vi "dotNET Compress String.vi"(8 "error in (no error)":errorcluster, 11 "String":string="<Cluster>\r\n<Name>TDC Data Cluster (XML)</Name>\r\n<NumElts>4</NumElts>\r\n<Array>\r\n<Name>Adapter Data</Name>\r\n<Dimsize>10</Dimsize>\r\n<String>\r\n<Name> </Name>\r\n<Val>SigmaQuest</Val>\r\n</String>\r\n<String>\r\n<Name> </Name>\r\n<Val>C:\\Program Files\\TMS\\TDC</Val>\r\n</String>\r\n<String>\r\n<Name> </Name>\r\n<Val>TDC Adapter XML Archive.vi</Val>\r\n</String>\r\n<String>\r\n<Name> </Name>\r\n<Val>C:\\Test Reports\\TDC XML</Val>\r\n</String>\r\n<String>\r\n<Name> </Name>\r\n<Val>ET</Val>\r\n</String>\r\n<String>\r\n<Name> </Name>\r\n<Val>OTDA</Val>\r\n</String>\r\n<String>\r\n<Name> </Name>\r\n<Val>TRUE</Val>\r\n</String>\r\n<String>\r\n<Name> </Name>\r\n<Val>D98FE819-833D-54CF-2F12-8500A4D4E1C3</Val>\r\n</String>\r\n<String>\r\n<Name> </Name>\r\n<Val></Val>\r\n</String>\r\n<String>\r\n<Name> </Name>\r\n<Val></Val>\r\n</String>\r\n</Array>\r\n<Cluster>\r\n<Name>Station Common Data</Name>\r\n<NumElts>10</NumElts>\r\n<String>\r\n<Name>Customer</Name>\r\n<Val></Val>\r\n</String>\r\n<String>\r\n<Name>Manufacturer</Name>\r\n<Val></Val>\r\n</String>\r\n<String>\r\n<Name>Process</Name>\r\n<Val></Val>\r\n</String>\r\n<String>\r\n<Name>Line</Name>\r\n<Val></Val>\r\n</String>\r\n<String>\r\n<Name>Site</Name>\r\n<Val>Sycamore-Chelmsford</Val>\r\n</String>\r\n<String>\r\n<Name>Station</Name>\r\n<Val>ATE0000003</Val>\r\n</String>\r\n<String>\r\n<Name>Operator</Name>\r\n<Val>jdaoust</Val>\r\n</String>\r\n<String>\r\n<Name>Privilege</Name>\r\n<Val>technician</Val>\r\n</String>\r\n<String>\r\n<Name>Exp1</Name>\r\n<Val></Val>\r\n</String>\r\n<String>\r\n<Name>Exp2</Name>\r\n<Val></Val>\r\n</String>\r\n</Cluster>\r\n<Cluster>\r\n<Name>Header Data</Name>\r\n<NumElts>19</NumElts>\r\n<String>\r\n<Name>SerialNumber</Name>\r\n<Val>N635017050</Val>\r\n</String>\r\n<String>\r\n<Name>ProductName</Name>\r\n<Val></Val>\r\n</String>\r\n<String>\r\n<Name>ProductNumber</Name>\r\n<Val>910244</Val>\r\n</String>\r\n<String>\r\n<Name>ProductRev</Name>\r\n<Val>AB</Val>\r\n</String>\r\n<String>\r\n<Name>FirmwareRev</Name>\r\n<Val></Val>\r\n</String>\r\n<String>\r\n<Name>CMProductName</Name>\r\n<Val></Val>\r\n</String>\r\n<String>\r\n<Name>CMProductNumber</Name>\r\n<Val>8500052410E</Val>\r\n</String>\r\n<String>\r\n<Name>CMProductRev</Name>\r\n<Val>0L1</Val>\r\n</String>\r\n<String>\r\n<Name>EventType</Name>\r\n<Val></Val>\r\n</String>\r\n<String>\r\n<Name>TPSName</Name>\r\n<Val>SN16K GSC-MC Full (Fixed Pad)</Val>\r\n</String>\r\n<String>\r\n<Name>TPSRev</Name>\r\n<Val>D</Val>\r\n</String>\r\n<String>\r\n<Name>TestStatus</Name>\r\n<Val>PASSED</Val>\r\n</String>\r\n<String>\r\n<Name>StartTime</Name>\r\n<Val>07/07/09 12:07:49</Val>\r\n</String>\r\n<String>\r\n<Name>StopTime</Name>\r\n<Val>07/07/09 12:53:15</Val>\r\n</String>\r\n<String>\r\n<Name>Duration</Name>\r\n<Val>2727</Val>\r\n</String>\r\n<String>\r\n<Name>FixtureID</Name>\r\n<Val></Val>\r\n</String>\r\n<String>\r\n<Name>LotCode</Name>\r\n<Val>HIPDB1</Val>\r\n</String>\r\n<String>\r\n<Name>Expansion1</Name>\r\n<Val></Val>\r\n</String>\r\n<String>\r\n<Name>Expansion2</Name>\r\n<Val></Val>\r\n</String>\r\n</Cluster>\r\n<Array>\r\n<Name>Data</Name>\r\n<Dimsize>11</Dimsize>\r\n<Dimsize>493</Dimsize>\r\n<String>\r\n<Name> </Name>\r\n<Val>UUT &amp; TPS Verify</Val>\r\n</String>\r\n<String>\r\n<Name> </Name>\r\n<Val>Fetch Matrix Details</Val>\r\n</String>\r\n<String>\r\n<Name> </Name>\r\n<Val>Get UUT Information</Val>\r\n</String>\r\n<String>\r\n<Name> </Name>\r\n<Val>Get UUT Information</Val>\r\n</String>\r\n<String>\r\n<Name> </Name>\r\n<Val>Log TPS P/N and Rev</Val>\r\n</String>\r\n<String>\r\n<Name> </Name>\r\n<Val>Check for Genealogy</Val>\r\n</String>\r\n<String>\r\n<Name> </Name>\r\n<Val>Skip if UUTInfoSubSequenceFile = \"Null\"</Val>\r\n</String>\r\n<String>\r\n<Name> </Name>\r\n<Val>Get UUT Genealogy Information</Val>\r\n</String>\r\n<String>\r\n<Name> </Name>\r\n<Val>TMS Common Genealogy Dialog</Val>\r\n</String>\r\n<String>\r\n<Name> </Name>\r\n<Val>Get Genealogy Information</Val>\r\n</String>\r\n<String>\r\n<Name> </Name>\r\n<Val>Power Supplies OFF</Val>\r\n</String>\r\n<String>\r\n<Name> </Name>\r\n<Val>Open VISA Sessions</Val>\r\n</String>\r\n<String>\r\n<Name> </Name>\r\n<Val>Save VXI CFG Path</Val>\r\n</String>\r\n<String>\r\n<Name> </Name>\r\n<Val>Store Paths to Directories</Val>\r\n</String>\r\n<String>\r\n<Name> </Name>\r\n<Val>Reset Arb</Val>\r\n</String>\r\n<String>\r\n<Name> </Name>\r\n<Val>Reset Mux Switching</Val>\r\n</String>\r\n<String>\r\n<Name> </Name>\r\n<Val>Store ITA Slot ID mask</Val>\r\n</String>\r\n<String>\r\n<Name> </Name>\r\n<Val>Store ITA Chassis ID mask</Val>\r\n</String>\r\n<String>\r\n<Name> </Name>\r\n<Val>Install and Connect UUT</Val>\r\n</String>\r\n<String>\r\n<Name> </Name>\r\n<Val>Insert UUT (PC Com)</Val>\r\n</String>\r\n<String>\r\n<Name> </Name>\r\n<Val>Verify Card Present</Val>\r\n</String>\r\n<String>\r\n<Name> </Name>\r\n<Val>Power UP</Val>\r\n</String>\r\n<String>\r\n<Name> </Name>\r\n<Val>Turn on 48VDC</Val>\r\n</String>\r\n<String>\r\n<Name> </Name>\r\n<Val>Turn on 3VDC</Val>\r\n</String>\r\n<String>\r\n<Name> </Name>\r\n<Val>Select 48VDC VXI Switches</Val>\r\n</String>\r\n<String>\r\n<Name> </Name>\r\n<Val>Check 48VDC Voltage</Val>\r\n</String>\r\n<String>\r\n<Name> </Name>\r\n<Val>Check 48VDC Current</Val>\r\n</String>\r\n<String>\r\n<Name> </Name>\r\n<Val>Select 3VDC VXI Switches</Val>\r\n</String>\r\n<String>\r\n<Name> </Name>\r\n<Val>Check 3VDC Voltage</Val>\r\n</String>\r\n<String>\r\n<Name> </Name>\r\n<Val>Verify UUT Bootup and Firmware</Val>\r\n</String>\r\n<String>\r\n<Name> </Name>\r\n<Val>Fetch Matrix Information if required</Val>\r\n</String>\r\n<String>\r\n<Name> </Name>\r\n<Val>Establish Communication</Val>\r\n</String>\r\n<String>\r\n<Name> </Name>\r\n<Val>Check Cable and DIP Switches</Val>\r\n</String>\r\n<String>\r\n<Name> </Name>\r\n<Val>Cycle Power if unable to Establish Communication</Val>\r\n</String>\r\n<String>\r\n<Name> </Name>\r\n<Val>Re-Establish Communication</Val>\r\n</String>\r\n<String>\r\n<Name> </Name>\r\n<Val>Fetch Versions - Flash Files</Val>\r\n</String>\r\n<String>\r\n<Name> </Name>\r\n<Val>Verify Flash Files = Required</Val>\r\n</String>\r\n<String>\r\n<Name> </Name>\r\n<Val>Get Loaded Versions using Command</Val>\r\n</String>\r\n<String>\r\n<Name> </Name>\r\n<Val>Verify Loaded = Required</Val>\r\n</String>\r\n<String>\r\n<Name> </Name>\r\n<Val>Change DIP Switches to RMM Mode</Val>\r\n</String>\r\n<String>\r\n<Name> </Name>\r\n<Val>Cycle Power 1</Val>\r\n</String>\r\n<String>\r\n<Name> </Name>\r\n<Val>Establish Communication 1</Val>\r\n</String>\r\n<String>\r\n<Name> </Name>\r\n<Val>Program BaseROM</Val>\r\n</String>\r\n<String>\r\n<Name> </Name>\r\n<Val>Cycle Power 2</Val>\r\n</String>\r\n<String>\r\n<Name> </Name>\r\n<Val>Establish Communication 2</Val>\r\n</String>\r\n<String>\r\n<Name> </Name>\r\n<Val>Program BootROM</Val>\r\n</String>\r\n<String>\r\n<Name> </Name>\r\n<Val>Program DiagROM</Val>\r\n</String>\r\n<String>\r\n<Name> </Name>\r\n<Val>Program FpgaROM</Val>\r\n</String>\r\n<String>\r\n<Name> </Name>\r\n<Val>Change DIP Switches to Diag Mode</Val>\r\n</String>\r\n<String>\r\n<Name> </Name>\r\n<Val>Cycle Power 3</Val>\r\n</String>\r\n<String>\r\n<Name> </Name>\r\n<Val>Establish Communication 3</Val>\r\n</String>\r\n<String>\r\n<Name> </Name>\r\n<Val>Verify UUT in Diag Mode</Val>\r\n</String>\r\n<String>\r\n<Name> </Name>\r\n<Val>Get Loaded Versions using Command 2</Val>\r\n</String>\r\n<String>\r\n<Name> </Name>\r\n<Val>Verify Loaded = Required 2</Val>\r\n</String>\r\n<String>\r\n<Name> </Name>\r\n<Val>Program IDPROM</Val>\r\n</String>\r\n<String>\r\n<Name> </Name>\r\n<Val>Electrical Diags</Val>\r\n</String>\r\n<String>\r\n<Name> </Name>\r\n<Val>MII Tests</Val>\r\n</String>\r\n<String>\r\n<Name> </Name>\r\n<Val>LED Test</Val>\r\n</String>\r\n<String>\r\n<Name> </Name>\r\n<Val>LED Test Retry Message</Val>\r\n</String>\r\n<String>\r\n<Name> </Name>\r\n<Val>MII0 Access Test</Val>\r\n</String>\r\n<String>\r\n<Name> </Name>\r\n<Val>MII1 Access Test</Val>\r\n</String>\r\n<String>\r\n<Name> </Name>\r\n<Val>SDRAM Tests</Val>\r\n</String>\r\n<String>\r\n<Name> </Name>\r\n<Val>FCC1 Setup for PHY Loopback</Val>\r\n</String>\r\n<String>\r\n<Name> </Name>\r\n<Val>FCC1 PHY Loopback Test</Val>\r\n</String>\r\n<String>\r\n<Name> </Name>\r\n<Val>FCC2 Setup for PHY Loopback</Val>\r\n</String>\r\n<String>\r\n<Name> </Name>\r\n<Val>FCC2 PHY Loopback Test</Val>\r\n</String>\r\n<String>\r\n<Name> </Name>\r\n<Val>Reinitialize card</Val>\r\n</String>\r\n<String>\r\n<Name> </Name>\r\n<Val>FCC1 Setup for no Loopback</Val>\r\n</String>\r\n<String>\r\n<Name> </Name>\r\n<Val>FCC2 Setup for no Loopback</Val>\r\n</String>\r\n<String>\r\n<Name> </Name>\r\n<Val>FCC1 to FCC2 Test</Val>\r\n</String>\r\n<String>\r\n<Name> </Name>\r\n<Val>FCC2 to FCC1 Test</Val>\r\n</String>\r\n<String>\r\n<Name> </Name>\r\n<Val>Cycle Reset Latch , FCC retest</Val>\r\n</String>\r\n<String>\r\n<Name> </Name>\r\n<Val>Establish Diagnostics Communication, FCC retest</Val>\r\n</String>\r\n<String>\r\n<Name> </Name>\r\n<Val>Get Temperature</Val>\r\n</String>\r\n<String>\r\n<Name> </Name>\r\n<Val>Temp Test Retry Message</Val>\r\n</String>\r\n<String>\r\n<Name> </Name>\r\n<Val>SDRAM Data Bus Test</Val>\r\n</String>\r\n<String>\r\n<Name> </Name>\r\n<Val>SDRAM Address Bus Test</Val>\r\n</String>\r\n<String>\r\n<Name> </Name>\r\n<Val>SDRAM Size Test</Val>\r\n</String>\r\n<String>\r\n<Name> </Name>\r\n<Val>FPGA Tests</Val>\r\n</String>\r\n<String>\r\n<Name> </Name>\r\n<Val>PRBS FPGA Access Test</Val>\r\n</String>\r\n<String>\r\n<Name> </Name>\r\n<Val>PRBS FPGA Interrupt Test</Val>\r\n</String>\r\n<String>\r\n<Name> </Name>\r\n<Val>EEPROM Tests</Val>\r\n</String>\r\n<String>\r\n<Name> </Name>\r\n<Val>EEPROM Single Byte Test</Val>\r\n</String>\r\n<String>\r\n<Name> </Name>\r\n<Val>GXC B EEPROM Access Test</Val>\r\n</String>\r\n<String>\r\n<Name> </Name>\r\n<Val>GXC A EEPROM Access Test</Val>\r\n</String>\r\n<String>\r\n<Name> </Name>\r\n<Val>Verify GXC B Status at Addr f303800c</Val>\r\n</String>\r\n<String>\r\n<Name> </Name>\r\n<Val>Verify GXC A Status at Addr f301800c</Val>\r\n</String>\r\n<String>\r\n<Name> </Name>\r\n<Val>CPLD Tests</Val>\r\n</String>\r\n<String>\r\n<Name> </Name>\r\n<Val>Control CPLD Version</Val>\r\n</String>\r\n<String>\r\n<Name> </Name>\r\n<Val>Control CPLD Access Test</Val>\r\n</String>\r\n<String>\r\n<Name> </Name>\r\n<Val>Timing CPLD Access Test</Val>\r\n</String>\r\n<String>\r\n<Name> </Name>\r\n<Val>Timing CPLD Interrupt Test</Val>\r\n</String>\r\n<String>\r\n<Name> </Name>\r\n<Val>GXC Tests</Val>\r\n</String>\r\n<String>\r\n<Name> </Name>\r\n<Val>GXC B Access Test</Val>\r\n</String>\r\n<String>\r\n<Name> </Name>\r\n<Val>GXC B Interrupt Test</Val>\r\n</String>\r\n<String>\r\n<Name> </Name>\r\n<Val>GXC A Access Test</Val>\r\n</String>\r\n<String>\r\n<Name> </Name>\r\n<Val>GXC A Interrupt Test</Val>\r\n</String>\r\n<String>\r\n<Name> </Name>\r\n<Val>Local Timing Tests</Val>\r\n</String>\r\n<String>\r\n<Name> </Name>\r\n<Val>Set Timing Select to Local</Val>\r\n</String>\r\n<String>\r\n<Name> </Name>\r\n<Val>Test VCXO Status</Val>\r\n</String>\r\n<String>\r\n<Name> </Name>\r\n<Val>Test SYSCLK Status</Val>\r\n</String>\r\n<String>\r\n<Name> </Name>\r\n<Val>Test PLL Status</Val>\r\n</String>\r\n<String>\r\n<Name> </Name>\r\n<Val>PLL Re-Lock Test</Val>\r\n</String>\r\n<String>\r\n<Name> </Name>\r\n<Val>PRBS Path Thru Switch</Val>\r\n</String>\r\n<String>\r\n<Name> </Name>\r\n<Val>PRBS Path Thru Switch B</Val>\r\n</String>\r\n<String>\r\n<Name> </Name>\r\n<Val>Reset Switch B, PRBS Path Test</Val>\r\n</String>\r\n<String>\r\n<Name> </Name>\r\n<Val>Setup PRBS Test Thru Switch B</Val>\r\n</String>\r\n<String>\r\n<Name> </Name>\r\n<Val>Verify PRBS Status, in Sync, SW B</Val>\r\n</String>\r\n<String>\r\n<Name> </Name>\r\n<Val>Verify PRBS Status, Zero B1 Errors, SW B</Val>\r\n</String>\r\n<String>\r\n<Name> </Name>\r\n<Val>Turn Off PRBS Generator</Val>\r\n</String>\r\n<String>\r\n<Name> </Name>\r\n<Val>Verify PRBS Status, Lost Sync, SW B</Val>\r\n</String>\r\n<String>\r\n<Name> </Name>\r\n<Val>Verify PRBS Status, Max B1 Errors, SW B</Val>\r\n</String>\r\n<String>\r\n<Name> </Name>\r\n<Val>PRBS Path Thru Switch A</Val>\r\n</String>\r\n<String>\r\n<Name> </Name>\r\n<Val>Reset Switch A, PRBS Path Test</Val>\r\n</String>\r\n<String>\r\n<Name> </Name>\r\n<Val>Setup PRBS Test Thru Switch A</Val>\r\n</String>\r\n<String>\r\n<Name> </Name>\r\n<Val>Verify PRBS Status, in Sync, SW A</Val>\r\n</String>\r\n<String>\r\n<Name> </Name>\r\n<Val>Verify PRBS Status, Zero B1 Errors, SW A</Val>\r\n</String>\r\n<String>\r\n<Name> </Name>\r\n<Val>Turn Off PRBS Generator</Val>\r\n</String>\r\n<String>\r\n<Name> </Name>\r\n<Val>Verify PRBS Status, Lost Sync, SW A</Val>\r\n</String>\r\n<String>\r\n<Name> </Name>\r\n<Val>Verify PRBS Status, Max B1 Errors, SW A</Val>\r\n</String>\r\n<String>\r\n<Name> </Name>\r\n<Val>Electrical Backplane Tests</Val>\r\n</String>\r\n<String>\r\n<Name> </Name>\r\n<Val>SMC Tests</Val>\r\n</String>\r\n<String>\r\n<Name> </Name>\r\n<Val>Enable SMC Digital IO</Val>\r\n</String>\r\n<String>\r\n<Name> </Name>\r\n<Val>Set SMC Act Inputs, 110</Val>\r\n</String>\r\n<String>\r\n<Name> </Name>\r\n<Val>Test Soft Reset A</Val>\r\n</String>\r\n<String>\r\n<Name> </Name>\r\n<Val>Test Hard Reset A</Val>\r\n</String>\r\n<String>\r\n<Name> </Name>\r\n<Val>SMC A Active Test 1</Val>\r\n</String>\r\n<String>\r\n<Name> </Name>\r\n<Val>Set SMC Act Inputs, 101</Val>\r\n</String>\r\n<String>\r\n<Name> </Name>\r\n<Val>SMC A Active Test 2</Val>\r\n</String>\r\n<String>\r\n<Name> </Name>\r\n<Val>Set SMC Act Inputs, 011</Val>\r\n</String>\r\n<String>\r\n<Name> </Name>\r\n<Val>SMC A Active Test 3</Val>\r\n</String>\r\n<String>\r\n<Name> </Name>\r\n<Val>Set SMC Act Inputs, 100</Val>\r\n</String>\r\n<String>\r\n<Name> </Name>\r\n<Val>Test Soft Reset B</Val>\r\n</String>\r\n<String>\r\n<Name> </Name>\r\n<Val>Test Hard Reset B</Val>\r\n</String>\r\n<String>\r\n<Name> </Name>\r\n<Val>SMC B Active Test 1</Val>\r\n</String>\r\n<String>\r\n<Name> </Name>\r\n<Val>Set SMC Act Inputs, 010</Val>\r\n</String>\r\n<String>\r\n<Name> </Name>\r\n<Val>SMC B Active Test 2</Val>\r\n</String>\r\n<String>\r\n<Name> </Name>\r\n<Val>Set SMC Act Inputs, 001</Val>\r\n</String>\r\n<String>\r\n<Name> </Name>\r\n<Val>SMC B Active Test 3</Val>\r\n</String>\r\n<String>\r\n<Name> </Name>\r\n<Val>Disable SMC Digital IO</Val>\r\n</String>\r\n<String>\r\n<Name> </Name>\r\n<Val>TRC Timing Tests</Val>\r\n</String>\r\n<String>\r\n<Name> </Name>\r\n<Val>Set Timing Select to Auto</Val>\r\n</String>\r\n<String>\r\n<Name> </Name>\r\n<Val>Enable TRC Digital IO</Val>\r\n</String>\r\n<String>\r\n<Name> </Name>\r\n<Val>TRC A Tests</Val>\r\n</String>\r\n<String>\r\n<Name> </Name>\r\n<Val>Set Arb to 19MHz Sys Clock A</Val>\r\n</String>\r\n<String>\r\n<Name> </Name>\r\n<Val>Test Prim Ref Clock Status Valid</Val>\r\n</String>\r\n<String>\r\n<Name> </Name>\r\n<Val>Test Sec Ref Clock Status Invalid</Val>\r\n</String>\r\n<String>\r\n<Name> </Name>\r\n<Val>Set TRC Act Inputs, 110</Val>\r\n</String>\r\n<String>\r\n<Name> </Name>\r\n<Val>TRC A Active Test 1</Val>\r\n</String>\r\n<String>\r\n<Name> </Name>\r\n<Val>Set TRC Act Inputs, 101</Val>\r\n</String>\r\n<String>\r\n<Name> </Name>\r\n<Val>TRC A Active Test 2</Val>\r\n</String>\r\n<String>\r\n<Name> </Name>\r\n<Val>Set TRC Act Inputs, 011</Val>\r\n</String>\r\n<String>\r\n<Name> </Name>\r\n<Val>TRC A Active Test 3</Val>\r\n</String>\r\n<String>\r\n<Name> </Name>\r\n<Val>TRC B Tests</Val>\r\n</String>\r\n<String>\r\n<Name> </Name>\r\n<Val>Set Arb to 19Mhz Sys Clock B</Val>\r\n</String>\r\n<String>\r\n<Name> </Name>\r\n<Val>Test Sec Ref Clock Status Valid</Val>\r\n</String>\r\n<String>\r\n<Name> </Name>\r\n<Val>Test Prim Ref Clock Status Invalid</Val>\r\n</String>\r\n<String>\r\n<Name> </Name>\r\n<Val>Set TRC Act Inputs, 100</Val>\r\n</String>\r\n<String>\r\n<Name> </Name>\r\n<Val>TRC B Active Test 1</Val>\r\n</String>\r\n<String>\r\n<Name> </Name>\r\n<Val>Set TRC Act Inputs, 010</Val>\r\n</String>\r\n<String>\r\n<Name> </Name>\r\n<Val>TRC B Active Test 2</Val>\r\n</String>\r\n<String>\r\n<Name> </Name>\r\n<Val>Set TRC Act Inputs, 001</Val>\r\n</String>\r\n<String>\r\n<Name> </Name>\r\n<Val>TRC B Active Test 3</Val>\r\n</String>\r\n<String>\r\n<Name> </Name>\r\n<Val>Fsync Tests</Val>\r\n</String>\r\n<String>\r\n<Name> </Name>\r\n<Val>Enable TRC Fsync Status Reporting</Val>\r\n</String>\r\n<String>\r\n<Name> </Name>\r\n<Val>Set TRC Act Inputs, 110</Val>\r\n</String>\r\n<String>\r\n<Name> </Name>\r\n<Val>Set Arb to 8KHz Fsync A</Val>\r\n</String>\r\n<String>\r\n<Name> </Name>\r\n<Val>Test Fsync A Status Valid</Val>\r\n</String>\r\n<String>\r\n<Name> </Name>\r\n<Val>Test Fsync B Status Invalid</Val>\r\n</String>\r\n<String>\r\n<Name> </Name>\r\n<Val>Set TRC Act Inputs, 100</Val>\r\n</String>\r\n<String>\r\n<Name> </Name>\r\n<Val>Set Arb to 8KHz Fsync B</Val>\r\n</String>\r\n<String>\r\n<Name> </Name>\r\n<Val>Test Fsync B Status Valid</Val>\r\n</String>\r\n<String>\r\n<Name> </Name>\r\n<Val>Test Fsync A Status Invalid</Val>\r\n</String>\r\n<String>\r\n<Name> </Name>\r\n<Val>Disable TRC Digital IO</Val>\r\n</String>\r\n<String>\r\n<Name> </Name>\r\n<Val>Reset Arb</Val>\r\n</String>\r\n<String>\r\n<Name> </Name>\r\n<Val>Verify TRC Active is Local</Val>\r\n</String>\r\n<String>\r\n<Name> </Name>\r\n<Val>Set Timing Select back to Local</Val>\r\n</String>\r\n<String>\r\n<Name> </Name>\r\n<Val>Chassis and Slot ID Tests</Val>\r\n</String>\r\n<String>\r\n<Name> </Name>\r\n<Val>Enable Chassis ID Digital IO</Val>\r\n</String>\r\n<String>\r\n<Name> </Name>\r\n<Val>Set Chassis ID to '55'</Val>\r\n</String>\r\n<String>\r\n<Name> </Name>\r\n<Val>Verify '55' at f100000c</Val>\r\n</String>\r\n<String>\r\n<Name> </Name>\r\n<Val>Set Chassis ID to 'AA'</Val>\r\n</String>\r\n<String>\r\n<Name> </Name>\r\n<Val>Verify 'AA' at f100000c</Val>\r\n</String>\r\n<String>\r\n<Name> </Name>\r\n<Val>Chassis ID Test from Diag Port</Val>\r\n</String>\r\n<String>\r\n<Name> </Name>\r\n<Val>Disable Chassis ID Digital IO</Val>\r\n</String>\r\n<String>\r\n<Name> </Name>\r\n<Val>Enable Slot ID Digital IO</Val>\r\n</String>\r\n<String>\r\n<Name> </Name>\r\n<Val>Slot ID Test</Val>\r\n</String>\r\n<String>\r\n<Name> </Name>\r\n<Val>Disable Slot ID Digital IO</Val>\r\n</String>\r\n<String>\r\n<Name> </Name>\r\n<Val>Card Pending Removal Test</Val>\r\n</String>\r\n<String>\r\n<Name> </Name>\r\n<Val>BP LED Test</Val>\r\n</String>\r\n<String>\r\n<Name> </Name>\r\n<Val>BP LED Test Retry Message</Val>\r\n</String>\r\n<String>\r\n<Name> </Name>\r\n<Val>Disable Digital IO</Val>\r\n</String>\r\n<String>\r\n<Name> </Name>\r\n<Val>Pull Reset Latch Down</Val>\r\n</String>\r\n<String>\r\n<Name> </Name>\r\n<Val>Verify Pending Removal BP Signal</Val>\r\n</String>\r\n<String>\r\n<Name> </Name>\r\n<Val>Return Reset Latch to Up Position</Val>\r\n</String>\r\n<String>\r\n<Name> </Name>\r\n<Val>Verify No Pending Removal BP Signal</Val>\r\n</String>\r\n<String>\r\n<Name> </Name>\r\n<Val>Disable Digital IO</Val>\r\n</String>\r\n<String>\r\n<Name> </Name>\r\n<Val>Verify Diagnostics Communication</Val>\r\n</String>\r\n<String>\r\n<Name> </Name>\r\n<Val>Optical Backplane Tests</Val>\r\n</String>\r\n<String>\r\n<Name> </Name>\r\n<Val>Install Empty Quad-pack Connector A</Val>\r\n</String>\r\n<String>\r\n<Name> </Name>\r\n<Val>Verify VCSEL Outputs, SW A Ports 0 - 31</Val>\r\n</String>\r\n<String>\r\n<Name> </Name>\r\n<Val>Install Pos 1 MT Connector</Val>\r\n</String>\r\n<String>\r\n<Name> </Name>\r\n<Val>Test Outputs from MT Postion 1</Val>\r\n</String>\r\n<String>\r\n<Name> </Name>\r\n<Val>Disable Lasers</Val>\r\n</String>\r\n<String>\r\n<Name> </Name>\r\n<Val>Delay for 1 Second Before Verifying Disable</Val>\r\n</String>\r\n<String>\r\n<Name> </Name>\r\n<Val>Verify Laser Disable</Val>\r\n</String>\r\n<String>\r\n<Name> </Name>\r\n<Val>Enable AIS-L Insertion</Val>\r\n</String>\r\n<String>\r\n<Name> </Name>\r\n<Val>Enable Lasers</Val>\r\n</String>\r\n<String>\r\n<Name> </Name>\r\n<Val>Delay for 1 Second Before Verifying Enable</Val>\r\n</String>\r\n<String>\r\n<Name> </Name>\r\n<Val>Reset Fifo</Val>\r\n</String>\r\n<String>\r\n<Name> </Name>\r\n<Val>Reset Frame</Val>\r\n</String>\r\n<String>\r\n<Name> </Name>\r\n<Val>Verify VCSEL Active</Val>\r\n</String>\r\n<String>\r\n<Name> </Name>\r\n<Val>Verify Laser Enable</Val>\r\n</String>\r\n<String>\r\n<Name> </Name>\r\n<Val>Install Pos 2 MT Connector</Val>\r\n</String>\r\n<String>\r\n<Name> </Name>\r\n<Val>Test Outputs from MT Postion 2</Val>\r\n</String>\r\n<String>\r\n<Name> </Name>\r\n<Val>Disable Lasers</Val>\r\n</String>\r\n<String>\r\n<Name> </Name>\r\n<Val>Delay for 1 Second Before Verifying Disable</Val>\r\n</String>\r\n<String>\r\n<Name> </Name>\r\n<Val>Verify Laser Disable</Val>\r\n</String>\r\n<String>\r\n<Name> </Name>\r\n<Val>Enable AIS-L Insertion</Val>\r\n</String>\r\n<String>\r\n<Name> </Name>\r\n<Val>Enable Lasers</Val>\r\n</String>\r\n<String>\r\n<Name> </Name>\r\n<Val>Delay for 1 Second Before Verifying Enable</Val>\r\n</String>\r\n<String>\r\n<Name> </Name>\r\n<Val>Reset Fifo</Val>\r\n</String>\r\n<String>\r\n<Name> </Name>\r\n<Val>Reset Frame</Val>\r\n</String>\r\n<String>\r\n<Name> </Name>\r\n<Val>Verify VCSEL Active</Val>\r\n</String>\r\n<String>\r\n<Name> </Name>\r\n<Val>Verify Laser Enable</Val>\r\n</String>\r\n<String>\r\n<Name> </Name>\r\n<Val>Install Pos 3 MT Connector</Val>\r\n</String>\r\n<String>\r\n<Name> </Name>\r\n<Val>Test Outputs from MT Postion 3</Val>\r\n</String>\r\n<String>\r\n<Name> </Name>\r\n<Val>Disable Lasers</Val>\r\n</String>\r\n<String>\r\n<Name> </Name>\r\n<Val>Delay for 1 Second Before Verifying Disable</Val>\r\n</String>\r\n<String>\r\n<Name> </Name>\r\n<Val>Verify Laser Disable</Val>\r\n</String>\r\n<String>\r\n<Name> </Name>\r\n<Val>Enable AIS-L Insertion</Val>\r\n</String>\r\n<String>\r\n<Name> </Name>\r\n<Val>Enable Lasers</Val>\r\n</String>\r\n<String>\r\n<Name> </Name>\r\n<Val>Delay for 1 Second Before Verifying Enable</Val>\r\n</String>\r\n<String>\r\n<Name> </Name>\r\n<Val>Reset Fifo</Val>\r\n</String>\r\n<String>\r\n<Name> </Name>\r\n<Val>Reset Frame</Val>\r\n</String>\r\n<String>\r\n<Name> </Name>\r\n<Val>Verify VCSEL Active</Val>\r\n</String>\r\n<String>\r\n<Name> </Name>\r\n<Val>Verify Laser Enable</Val>\r\n</String>\r\n<String>\r\n<Name> </Name>\r\n<Val>Install Pos 4 MT Connector</Val>\r\n</String>\r\n<String>\r\n<Name> </Name>\r\n<Val>Test Outputs from MT Postion 4</Val>\r\n</String>\r\n<String>\r\n<Name> </Name>\r\n<Val>Disable Lasers</Val>\r\n</String>\r\n<String>\r\n<Name> </Name>\r\n<Val>Delay for 1 Second Before Verifying Disable</Val>\r\n</String>\r\n<String>\r\n<Name> </Name>\r\n<Val>Verify Laser Disable</Val>\r\n</String>\r\n<String>\r\n<Name> </Name>\r\n<Val>Enable AIS-L Insertion</Val>\r\n</String>\r\n<String>\r\n<Name> </Name>\r\n<Val>Enable Lasers</Val>\r\n</String>\r\n<String>\r\n<Name> </Name>\r\n<Val>Delay for 1 Second Before Verifying Enable</Val>\r\n</String>\r\n<String>\r\n<Name> </Name>\r\n<Val>Reset Fifo</Val>\r\n</String>\r\n<String>\r\n<Name> </Name>\r\n<Val>Reset Frame</Val>\r\n</String>\r\n<String>\r\n<Name> </Name>\r\n<Val>Verify VCSEL Active</Val>\r\n</String>\r\n<String>\r\n<Name> </Name>\r\n<Val>Verify Laser Enable</Val>\r\n</String>\r\n<String>\r\n<Name> </Name>\r\n<Val>Install Empty Quad-pack Connector B</Val>\r\n</String>\r\n<String>\r\n<Name> </Name>\r\n<Val>Verify VCSEL Outputs, SW B Ports 0 - 31</Val>\r\n</String>\r\n<String>\r\n<Name> </Name>\r\n<Val>Install Pos 1 MT Connector</Val>\r\n</String>\r\n<String>\r\n<Name> </Name>\r\n<Val>Test Outputs from MT Postion 1</Val>\r\n</String>\r\n<String>\r\n<Name> </Name>\r\n<Val>Disable Lasers</Val>\r\n</String>\r\n<String>\r\n<Name> </Name>\r\n<Val>Delay for 1 Second Before Verifying Disable</Val>\r\n</String>\r\n<String>\r\n<Name> </Name>\r\n<Val>Verify Laser Disable</Val>\r\n</String>\r\n<String>\r\n<Name> </Name>\r\n<Val>Enable AIS-L Insertion</Val>\r\n</String>\r\n<String>\r\n<Name> </Name>\r\n<Val>Enable Lasers</Val>\r\n</String>\r\n<String>\r\n<Name> </Name>\r\n<Val>Delay for 1 Second Before Verifying Enable</Val>\r\n</String>\r\n<String>\r\n<Name> </Name>\r\n<Val>Reset Fifo</Val>\r\n</String>\r\n<String>\r\n<Name> </Name>\r\n<Val>Reset Frame</Val>\r\n</String>\r\n<String>\r\n<Name> </Name>\r\n<Val>Verify VCSEL Active</Val>\r\n</String>\r\n<String>\r\n<Name> </Name>\r\n<Val>Verify Laser Enable</Val>\r\n</String>\r\n<String>\r\n<Name> </Name>\r\n<Val>Install Pos 2 MT Connector</Val>\r\n</String>\r\n<String>\r\n<Name> </Name>\r\n<Val>Test Outputs from MT Postion 2</Val>\r\n</String>\r\n<String>\r\n<Name> </Name>\r\n<Val>Disable Lasers</Val>\r\n</String>\r\n<String>\r\n<Name> </Name>\r\n<Val>Delay for 1 Second Before Verifying Disable</Val>\r\n</String>\r\n<String>\r\n<Name> </Name>\r\n<Val>Verify Laser Disable</Val>\r\n</String>\r\n<String>\r\n<Name> </Name>\r\n<Val>Enable AIS-L Insertion</Val>\r\n</String>\r\n<String>\r\n<Name> </Name>\r\n<Val>Enable Lasers</Val>\r\n</String>\r\n<String>\r\n<Name> </Name>\r\n<Val>Delay for 1 Second Before Verifying Enable</Val>\r\n</String>\r\n<String>\r\n<Name> </Name>\r\n<Val>Reset Fifo</Val>\r\n</String>\r\n<String>\r\n<Name> </Name>\r\n<Val>Reset Frame</Val>\r\n</String>\r\n<String>\r\n<Name> </Name>\r\n<Val>Verify VCSEL Active</Val>\r\n</String>\r\n<String>\r\n<Name> </Name>\r\n<Val>Verify Laser Enable</Val>\r\n</String>\r\n<String>\r\n<Name> </Name>\r\n<Val>Install Pos 3 MT Connector</Val>\r\n</String>\r\n<String>\r\n<Name> </Name>\r\n<Val>Test Outputs from MT Postion 3</Val>\r\n</String>\r\n<String>\r\n<Name> </Name>\r\n<Val>Disable Lasers</Val>\r\n</String>\r\n<String>\r\n<Name> </Name>\r\n<Val>Delay for 1 Second Before Verifying Disable</Val>\r\n</String>\r\n<String>\r\n<Name> </Name>\r\n<Val>Verify Laser Disable</Val>\r\n</String>\r\n<String>\r\n<Name> </Name>\r\n<Val>Enable AIS-L Insertion</Val>\r\n</String>\r\n<String>\r\n<Name> </Name>\r\n<Val>Enable Lasers</Val>\r\n</String>\r\n<String>\r\n<Name> </Name>\r\n<Val>Delay for 1 Second Before Verifying Enable</Val>\r\n</String>\r\n<String>\r\n<Name> </Name>\r\n<Val>Reset Fifo</Val>\r\n</String>\r\n<String>\r\n<Name> </Name>\r\n<Val>Reset Frame</Val>\r\n</String>\r\n<String>\r\n<Name> </Name>\r\n<Val>Verify VCSEL Active</Val>\r\n</String>\r\n<String>\r\n<Name> </Name>\r\n<Val>Verify Laser Enable</Val>\r\n</String>\r\n<String>\r\n<Name> </Name>\r\n<Val>Install Pos 4 MT Connector</Val>\r\n</String>\r\n<String>\r\n<Name> </Name>\r\n<Val>Test Outputs from MT Postion 4</Val>\r\n</String>\r\n<String>\r\n<Name> </Name>\r\n<Val>Disable Lasers</Val>\r\n</String>\r\n<String>\r\n<Name> </Name>\r\n<Val>Delay for 1 Second Before Verifying Disable</Val>\r\n</String>\r\n<String>\r\n<Name> </Name>\r\n<Val>Verify Laser Disable</Val>\r\n</String>\r\n<String>\r\n<Name> </Name>\r\n<Val>Enable AIS-L Insertion</Val>\r\n</String>\r\n<String>\r\n<Name> </Name>\r\n<Val>Enable Lasers</Val>\r\n</String>\r\n<String>\r\n<Name> </Name>\r\n<Val>Delay for 1 Second Before Verifying Enable</Val>\r\n</String>\r\n<String>\r\n<Name> </Name>\r\n<Val>Reset Fifo</Val>\r\n</String>\r\n<String>\r\n<Name> </Name>\r\n<Val>Reset Frame</Val>\r\n</String>\r\n<String>\r\n<Name> </Name>\r\n<Val>Verify VCSEL Active</Val>\r\n</String>\r\n<String>\r\n<Name> </Name>\r\n<Val>Verify Laser Enable</Val>\r\n</String>\r\n<String>\r\n<Name> </Name>\r\n<Val>Install Empty Quad-pack Connector C</Val>\r\n</String>\r\n<String>\r\n<Name> </Name>\r\n<Val>Verify VCSEL Outputs, SW A Ports 32 - 63</Val>\r\n</String>\r\n<String>\r\n<Name> </Name>\r\n<Val>Install Pos 1 MT Connector</Val>\r\n</String>\r\n<String>\r\n<Name> </Name>\r\n<Val>Test Outputs from MT Postion 1</Val>\r\n</String>\r\n<String>\r\n<Name> </Name>\r\n<Val>Disable Lasers</Val>\r\n</String>\r\n<String>\r\n<Name> </Name>\r\n<Val>Delay for 1 Second Before Verifying Disable</Val>\r\n</String>\r\n<String>\r\n<Name> </Name>\r\n<Val>Verify Laser Disable</Val>\r\n</String>\r\n<String>\r\n<Name> </Name>\r\n<Val>Enable AIS-L Insertion</Val>\r\n</String>\r\n<String>\r\n<Name> </Name>\r\n<Val>Enable Lasers</Val>\r\n</String>\r\n<String>\r\n<Name> </Name>\r\n<Val>Delay for 1 Second Before Verifying Enable</Val>\r\n</String>\r\n<String>\r\n<Name> </Name>\r\n<Val>Reset Fifo</Val>\r\n</String>\r\n<String>\r\n<Name> </Name>\r\n<Val>Reset Frame</Val>\r\n</String>\r\n<String>\r\n<Name> </Name>\r\n<Val>Verify VCSEL Active</Val>\r\n</String>\r\n<String>\r\n<Name> </Name>\r\n<Val>Verify Laser Enable</Val>\r\n</String>\r\n<String>\r\n<Name> </Name>\r\n<Val>Install Pos 2 MT Connector</Val>\r\n</String>\r\n<String>\r\n<Name> </Name>\r\n<Val>Test Outputs from MT Postion 2</Val>\r\n</String>\r\n<String>\r\n<Name> </Name>\r\n<Val>Disable Lasers</Val>\r\n</String>\r\n<String>\r\n<Name> </Name>\r\n<Val>Delay for 1 Second Before Verifying Disable</Val>\r\n</String>\r\n<String>\r\n<Name> </Name>\r\n<Val>Verify Laser Disable</Val>\r\n</String>\r\n<String>\r\n<Name> </Name>\r\n<Val>Enable AIS-L Insertion</Val>\r\n</String>\r\n<String>\r\n<Name> </Name>\r\n<Val>Enable Lasers</Val>\r\n</String>\r\n<String>\r\n<Name> </Name>\r\n<Val>Delay for 1 Second Before Verifying Enable</Val>\r\n</String>\r\n<String>\r\n<Name> </Name>\r\n<Val>Reset Fifo</Val>\r\n</String>\r\n<String>\r\n<Name> </Name>\r\n<Val>Reset Frame</Val>\r\n</String>\r\n<String>\r\n<Name> </Name>\r\n<Val>Verify VCSEL Active</Val>\r\n</String>\r\n<String>\r\n<Name> </Name>\r\n<Val>Verify Laser Enable</Val>\r\n</String>\r\n<String>\r\n<Name> </Name>\r\n<Val>Install Pos 3 MT Connector</Val>\r\n</String>\r\n<String>\r\n<Name> </Name>\r\n<Val>Test Outputs from MT Postion 3</Val>\r\n</String>\r\n<String>\r\n<Name> </Name>\r\n<Val>Disable Lasers</Val>\r\n</String>\r\n<String>\r\n<Name> </Name>\r\n<Val>Delay for 1 Second Before Verifying Disable</Val>\r\n</String>\r\n<String>\r\n<Name> </Name>\r\n<Val>Verify Laser Disable</Val>\r\n</String>\r\n<String>\r\n<Name> </Name>\r\n<Val>Enable AIS-L Insertion</Val>\r\n</String>\r\n<String>\r\n<Name> </Name>\r\n<Val>Enable Lasers</Val>\r\n</String>\r\n<String>\r\n<Name> </Name>\r\n<Val>Delay for 1 Second Before Verifying Enable</Val>\r\n</String>\r\n<String>\r\n<Name> </Name>\r\n<Val>Reset Fifo</Val>\r\n</String>\r\n<String>\r\n<Name> </Name>\r\n<Val>Reset Frame</Val>\r\n</String>\r\n<String>\r\n<Name> </Name>\r\n<Val>Verify VCSEL Active</Val>\r\n</String>\r\n<String>\r\n<Name> </Name>\r\n<Val>Verify Laser Enable</Val>\r\n</String>\r\n<String>\r\n<Name> </Name>\r\n<Val>Install Pos 4 MT Connector</Val>\r\n</String>\r\n<String>\r\n<Name> </Name>\r\n<Val>Test Outputs from MT Postion 4</Val>\r\n</String>\r\n<String>\r\n<Name> </Name>\r\n<Val>Disable Lasers</Val>\r\n</String>\r\n<String>\r\n<Name> </Name>\r\n<Val>Delay for 1 Second Before Verifying Disable</Val>\r\n</String>\r\n<String>\r\n<Name> </Name>\r\n<Val>Verify Laser Disable</Val>\r\n</String>\r\n<String>\r\n<Name> </Name>\r\n<Val>Enable AIS-L Insertion</Val>\r\n</String>\r\n<String>\r\n<Name> </Name>\r\n<Val>Enable Lasers</Val>\r\n</String>\r\n<String>\r\n<Name> </Name>\r\n<Val>Delay for 1 Second Before Verifying Enable</Val>\r\n</String>\r\n<String>\r\n<Name> </Name>\r\n<Val>Reset Fifo</Val>\r\n</String>\r\n<String>\r\n<Name> </Name>\r\n<Val>Reset Frame</Val>\r\n</String>\r\n<String>\r\n<Name> </Name>\r\n<Val>Verify VCSEL Active</Val>\r\n</String>\r\n<String>\r\n<Name> </Name>\r\n<Val>Verify Laser Enable</Val>\r\n</String>\r\n<String>\r\n<Name> </Name>\r\n<Val>Install Empty Quad-pack Connector D</Val>\r\n</String>\r\n<String>\r\n<Name> </Name>\r\n<Val>Verify VCSEL Outputs, SW B Ports 32 - 63</Val>\r\n</String>\r\n<String>\r\n<Name> </Name>\r\n<Val>Install Pos 1 MT Connector</Val>\r\n</String>\r\n<String>\r\n<Name> </Name>\r\n<Val>Test Outputs from MT Postion 1</Val>\r\n</String>\r\n<String>\r\n<Name> </Name>\r\n<Val>Disable Lasers</Val>\r\n</String>\r\n<String>\r\n<Name> </Name>\r\n<Val>Delay for 1 Second Before Verifying Disable</Val>\r\n</String>\r\n<String>\r\n<Name> </Name>\r\n<Val>Verify Laser Disable</Val>\r\n</String>\r\n<String>\r\n<Name> </Name>\r\n<Val>Enable AIS-L Insertion</Val>\r\n</String>\r\n<String>\r\n<Name> </Name>\r\n<Val>Enable Lasers</Val>\r\n</String>\r\n<String>\r\n<Name> </Name>\r\n<Val>Delay for 1 Second Before Verifying Enable</Val>\r\n</String>\r\n<String>\r\n<Name> </Name>\r\n<Val>Reset Fifo</Val>\r\n</String>\r\n<String>\r\n<Name> </Name>\r\n<Val>Reset Frame</Val>\r\n</String>\r\n<String>\r\n<Name> </Name>\r\n<Val>Verify VCSEL Active</Val>\r\n</String>\r\n<String>\r\n<Name> </Name>\r\n<Val>Verify Laser Enable</Val>\r\n</String>\r\n<String>\r\n<Name> </Name>\r\n<Val>Install Pos 2 MT Connector</Val>\r\n</String>\r\n<String>\r\n<Name> </Name>\r\n<Val>Test Outputs from MT Postion 2</Val>\r\n</String>\r\n<String>\r\n<Name> </Name>\r\n<Val>Disable Lasers</Val>\r\n</String>\r\n<String>\r\n<Name> </Name>\r\n<Val>Delay for 1 Second Before Verifying Disable</Val>\r\n</String>\r\n<String>\r\n<Name> </Name>\r\n<Val>Verify Laser Disable</Val>\r\n</String>\r\n<String>\r\n<Name> </Name>\r\n<Val>Enable AIS-L Insertion</Val>\r\n</String>\r\n<String>\r\n<Name> </Name>\r\n<Val>Enable Lasers</Val>\r\n</String>\r\n<String>\r\n<Name> </Name>\r\n<Val>Delay for 1 Second Before Verifying Enable</Val>\r\n</String>\r\n<String>\r\n<Name> </Name>\r\n<Val>Reset Fifo</Val>\r\n</String>\r\n<String>\r\n<Name> </Name>\r\n<Val>Reset Frame</Val>\r\n</String>\r\n<String>\r\n<Name> </Name>\r\n<Val>Verify VCSEL Active</Val>\r\n</String>\r\n<String>\r\n<Name> </Name>\r\n<Val>Verify Laser Enable</Val>\r\n</String>\r\n<String>\r\n<Name> </Name>\r\n<Val>Install Pos 3 MT Connector</Val>\r\n</String>\r\n<String>\r\n<Name> </Name>\r\n<Val>Test Outputs from MT Postion 3</Val>\r\n</String>\r\n<String>\r\n<Name> </Name>\r\n<Val>Disable Lasers</Val>\r\n</String>\r\n<String>\r\n<Name> </Name>\r\n<Val>Delay for 1 Second Before Verifying Disable</Val>\r\n</String>\r\n<String>\r\n<Name> </Name>\r\n<Val>Verify Laser Disable</Val>\r\n</String>\r\n<String>\r\n<Name> </Name>\r\n<Val>Enable AIS-L Insertion</Val>\r\n</String>\r\n<String>\r\n<Name> </Name>\r\n<Val>Enable Lasers</Val>\r\n</String>\r\n<String>\r\n<Name> </Name>\r\n<Val>Delay for 1 Second Before Verifying Enable</Val>\r\n</String>\r\n<String>\r\n<Name> </Name>\r\n<Val>Reset Fifo</Val>\r\n</String>\r\n<String>\r\n<Name> </Name>\r\n<Val>Reset Frame</Val>\r\n</String>\r\n<String>\r\n<Name> </Name>\r\n<Val>Verify VCSEL Active</Val>\r\n</String>\r\n<String>\r\n<Name> </Name>\r\n<Val>Verify Laser Enable</Val>\r\n</String>\r\n<String>\r\n<Name> </Name>\r\n<Val>Install Pos 4 MT Connector</Val>\r\n</String>\r\n<String>\r\n<Name> </Name>\r\n<Val>Test Outputs from MT Postion 4</Val>\r\n</String>\r\n<String>\r\n<Name> </Name>\r\n<Val>Disable Lasers</Val>\r\n</String>\r\n<String>\r\n<Name> </Name>\r\n<Val>Delay for 1 Second Before Verifying Disable</Val>\r\n</String>\r\n<String>\r\n<Name> </Name>\r\n<Val>Verify Laser Disable</Val>\r\n</String>\r\n<String>\r\n<Name> </Name>\r\n<Val>Enable AIS-L Insertion</Val>\r\n</String>\r\n<String>\r\n<Name> </Name>\r\n<Val>Enable Lasers</Val>\r\n</String>\r\n<String>\r\n<Name> </Name>\r\n<Val>Delay for 1 Second Before Verifying Enable</Val>\r\n</String>\r\n<String>\r\n<Name> </Name>\r\n<Val>Reset Fifo</Val>\r\n</String>\r\n<String>\r\n<Name> </Name>\r\n<Val>Reset Frame</Val>\r\n</String>\r\n<String>\r\n<Name> </Name>\r\n<Val>Verify VCSEL Active</Val>\r\n</String>\r\n<String>\r\n<Name> </Name>\r\n<Val>Verify Laser Enable</Val>\r\n</String>\r\n<String>\r\n<Name> </Name>\r\n<Val>Install Optical Loopbacks</Val>\r\n</String>\r\n<String>\r\n<Name> </Name>\r\n<Val>Enable AIS-L Insertion</Val>\r\n</String>\r\n<String>\r\n<Name> </Name>\r\n<Val>Setup for PRBS</Val>\r\n</String>\r\n<String>\r\n<Name> </Name>\r\n<Val>Reset Switch B for PRBS Test</Val>\r\n</String>\r\n<String>\r\n<Name> </Name>\r\n<Val>Reset Switch A for PRBS Test</Val>\r\n</String>\r\n<String>\r\n<Name> </Name>\r\n<Val>Setup Logical Mapping</Val>\r\n</String>\r\n<String>\r\n<Name> </Name>\r\n<Val>Turn on PRBS</Val>\r\n</String>\r\n<String>\r\n<Name> </Name>\r\n<Val>SW B Set All Input Ports to Ref B</Val>\r\n</String>\r\n<String>\r\n<Name> </Name>\r\n<Val>SW A Set All Input Ports to Ref B</Val>\r\n</String>\r\n<String>\r\n<Name> </Name>\r\n<Val>SW B Set Input Port 64 to Ref A</Val>\r\n</String>\r\n<String>\r\n<Name> </Name>\r\n<Val>SW A Set Input Port 64 to Ref A</Val>\r\n</String>\r\n<String>\r\n<Name> </Name>\r\n<Val>SW B Broadcast PRBS Data All Ports</Val>\r\n</String>\r\n<String>\r\n<Name> </Name>\r\n<Val>SW A Broadcast PRBS Data All Ports</Val>\r\n</String>\r\n<String>\r\n<Name> </Name>\r\n<Val>Disable B1 Regeneration, SW B</Val>\r\n</String>\r\n<String>\r\n<Name> </Name>\r\n<Val>Disable B1 Regeneration, SW A</Val>\r\n</String>\r\n<String>\r\n<Name> </Name>\r\n<Val>Verify Loopbacks, SW A Ports 0 -31</Val>\r\n</String>\r\n<String>\r\n<Name> </Name>\r\n<Val>Verify Loopbacks, SW B Ports 0 -31</Val>\r\n</String>\r\n<String>\r\n<Name> </Name>\r\n<Val>Verify Loopbacks, SW A Ports 32 -63</Val>\r\n</String>\r\n<String>\r\n<Name> </Name>\r\n<Val>Verify Loopbacks, SW B Ports 32 -63</Val>\r\n</String>\r\n<String>\r\n<Name> </Name>\r\n<Val>Verify Frame Sync, Loopback</Val>\r\n</String>\r\n<String>\r\n<Name> </Name>\r\n<Val>Verify Frame Alignment, Loopback</Val>\r\n</String>\r\n<String>\r\n<Name> </Name>\r\n<Val>Clear B1 Error Registers</Val>\r\n</String>\r\n<String>\r\n<Name> </Name>\r\n<Val>Initialize PRBS Start Time</Val>\r\n</String>\r\n<String>\r\n<Name> </Name>\r\n<Val>15 Second PRBS, Loopbacks</Val>\r\n</String>\r\n<String>\r\n<Name> </Name>\r\n<Val>Verify GXC B Status at Addr f303800c</Val>\r\n</String>\r\n<String>\r\n<Name> </Name>\r\n<Val>Verify GXC A Status at Addr f301800c</Val>\r\n</String>\r\n<String>\r\n<Name> </Name>\r\n<Val>Scan Fixed Attenuator Serial Numbers</Val>\r\n</String>\r\n<String>\r\n<Name> </Name>\r\n<Val>Test Optical Shuffle Connections</Val>\r\n</String>\r\n<String>\r\n<Name> </Name>\r\n<Val>Enable B1 Regeneration, SW B</Val>\r\n</String>\r\n<String>\r\n<Name> </Name>\r\n<Val>Enable B1 Regeneration, SW A</Val>\r\n</String>\r\n<String>\r\n<Name> </Name>\r\n<Val>Reset Switch B Fifo</Val>\r\n</String>\r\n<String>\r\n<Name> </Name>\r\n<Val>Reset Switch A Fifo</Val>\r\n</String>\r\n<String>\r\n<Name> </Name>\r\n<Val>Reset Switch B Frame</Val>\r\n</String>\r\n<String>\r\n<Name> </Name>\r\n<Val>Reset Switch A Frame</Val>\r\n</String>\r\n<String>\r\n<Name> </Name>\r\n<Val>Clear B1 Error Registers</Val>\r\n</String>\r\n<String>\r\n<Name> </Name>\r\n<Val>Optical Fiber Shuffle Test</Val>\r\n</String>\r\n<String>\r\n<Name> </Name>\r\n<Val>Install Half Loopback in Quad-pack A</Val>\r\n</String>\r\n<String>\r\n<Name> </Name>\r\n<Val>Reset Switch A Fifo post Half-lpbk at Quadpack</Val>\r\n</String>\r\n<String>\r\n<Name> </Name>\r\n<Val>Reset Switch A Frame post Half-lpbk at Quadpack</Val>\r\n</String>\r\n<String>\r\n<Name> </Name>\r\n<Val>Test for Swapped MT Conns in Quadpack</Val>\r\n</String>\r\n<String>\r\n<Name> </Name>\r\n<Val>Install Half Loopback in Quad-pack B</Val>\r\n</String>\r\n<String>\r\n<Name> </Name>\r\n<Val>Reset Switch A Fifo post Half-lpbk at Quadpack</Val>\r\n</String>\r\n<String>\r\n<Name> </Name>\r\n<Val>Reset Switch A Frame post Half-lpbk at Quadpack</Val>\r\n</String>\r\n<String>\r\n<Name> </Name>\r\n<Val>Test for Swapped MT Conns in Quadpack</Val>\r\n</String>\r\n<String>\r\n<Name> </Name>\r\n<Val>Install Half Loopback in Quad-pack C</Val>\r\n</String>\r\n<String>\r\n<Name> </Name>\r\n<Val>Reset Switch A Fifo post Half-lpbk at Quadpack</Val>\r\n</String>\r\n<String>\r\n<Name> </Name>\r\n<Val>Reset Switch A Frame post Half-lpbk at Quadpack</Val>\r\n</String>\r\n<String>\r\n<Name> </Name>\r\n<Val>Test for Swapped MT Conns in Quadpack</Val>\r\n</String>\r\n<String>\r\n<Name> </Name>\r\n<Val>Install Half Loopback in Quad-pack D</Val>\r\n</String>\r\n<String>\r\n<Name> </Name>\r\n<Val>Reset Switch A Fifo post Half-lpbk at Quadpack</Val>\r\n</String>\r\n<String>\r\n<Name> </Name>\r\n<Val>Reset Switch A Frame post Half-lpbk at Quadpack</Val>\r\n</String>\r\n<String>\r\n<Name> </Name>\r\n<Val>Test for Swapped MT Conns in Quadpack</Val>\r\n</String>\r\n<String>\r\n<Name> </Name>\r\n<Val>Receive Sensitivity Tests</Val>\r\n</String>\r\n<String>\r\n<Name> </Name>\r\n<Val>Install Optical Loopbacks</Val>\r\n</String>\r\n<String>\r\n<Name> </Name>\r\n<Val>Scan Fixed Attenuator Serial Numbers</Val>\r\n</String>\r\n<String>\r\n<Name> </Name>\r\n<Val>Log Fixed Pad Serial Numbers</Val>\r\n</String>\r\n<String>\r\n<Name> </Name>\r\n<Val>Setup for PRBS</Val>\r\n</String>\r\n<String>\r\n<Name> </Name>\r\n<Val>Reset Switch B for PRBS Test</Val>\r\n</String>\r\n<String>\r\n<Name> </Name>\r\n<Val>Reset Switch A for PRBS Test</Val>\r\n</String>\r\n<String>\r\n<Name> </Name>\r\n<Val>Setup Logical Mapping</Val>\r\n</String>\r\n<String>\r\n<Name> </Name>\r\n<Val>Turn on PRBS</Val>\r\n</String>\r\n<String>\r\n<Name> </Name>\r\n<Val>SW B Set All Input Ports to Ref B</Val>\r\n</String>\r\n<String>\r\n<Name> </Name>\r\n<Val>SW A Set All Input Ports to Ref B</Val>\r\n</String>\r\n<String>\r\n<Name> </Name>\r\n<Val>SW B Set Input Port 64 to Ref A</Val>\r\n</String>\r\n<String>\r\n<Name> </Name>\r\n<Val>SW A Set Input Port 64 to Ref A</Val>\r\n</String>\r\n<String>\r\n<Name> </Name>\r\n<Val>SW B Broadcast PRBS Data All Ports</Val>\r\n</String>\r\n<String>\r\n<Name> </Name>\r\n<Val>SW A Broadcast PRBS Data All Ports</Val>\r\n</String>\r\n<String>\r\n<Name> </Name>\r\n<Val>Disable B1 Regeneration, SW B</Val>\r\n</String>\r\n<String>\r\n<Name> </Name>\r\n<Val>Disable B1 Regeneration, SW A</Val>\r\n</String>\r\n<String>\r\n<Name> </Name>\r\n<Val>Rx Sensitivity, SW A Ports 0 - 63 and SW B Ports 0-63</Val>\r\n</String>\r\n<String>\r\n<Name> </Name>\r\n<Val>Verify Loopbacks, SW A Rx Ports 0 -31</Val>\r\n</String>\r\n<String>\r\n<Name> </Name>\r\n<Val>Verify Frame Sync SW A Ports 0 - 31</Val>\r\n</String>\r\n<String>\r\n<Name> </Name>\r\n<Val>Verify Frame Align SW A Ports 0 - 31</Val>\r\n</String>\r\n<String>\r\n<Name> </Name>\r\n<Val>Verify Loopbacks, SW A Rx Ports 32 -63</Val>\r\n</String>\r\n<String>\r\n<Name> </Name>\r\n<Val>Verify Frame Sync SW A Ports 32 -63</Val>\r\n</String>\r\n<String>\r\n<Name> </Name>\r\n<Val>Verify Frame Align SW A Ports 32 -63</Val>\r\n</String>\r\n<String>\r\n<Name> </Name>\r\n<Val>Verify Loopbacks, SW B Rx Ports 0 -31</Val>\r\n</String>\r\n<String>\r\n<Name> </Name>\r\n<Val>Verify Frame Sync SW B Ports 0 - 31</Val>\r\n</String>\r\n<String>\r\n<Name> </Name>\r\n<Val>Verify Frame Align SW B Ports 0 - 31</Val>\r\n</String>\r\n<String>\r\n<Name> </Name>\r\n<Val>Verify Loopbacks, SW B Rx Ports 32 -63</Val>\r\n</String>\r\n<String>\r\n<Name> </Name>\r\n<Val>Verify Frame Sync SW B Ports 32 -63</Val>\r\n</String>\r\n<String>\r\n<Name> </Name>\r\n<Val>Verify Frame Align SW B Ports 32 -63</Val>\r\n</String>\r\n<String>\r\n<Name> </Name>\r\n<Val>Verify GXC B Status at Addr f303800c, pre-PRBS</Val>\r\n</String>\r\n<String>\r\n<Name> </Name>\r\n<Val>Verify GXC A Status at Addr f301800c, pre-PRBS</Val>\r\n</String>\r\n<String>\r\n<Name> </Name>\r\n<Val>Clear B1 Errors for SW A  &amp; SW B All Ports</Val>\r\n</String>\r\n<String>\r\n<Name> </Name>\r\n<Val>Initialize Start Time for SW A  &amp; SW B All Ports</Val>\r\n</String>\r\n<String>\r\n<Name> </Name>\r\n<Val>4 Minute PRBS B1 Test at -14dBm, SW A  &amp; SW B All Ports</Val>\r\n</String>\r\n<String>\r\n<Name> </Name>\r\n<Val>Verify GXC B Status at Addr f303800c, post PRBS</Val>\r\n</String>\r\n<String>\r\n<Name> </Name>\r\n<Val>Verify GXC A Status at Addr f301800c, post PRBS</Val>\r\n</String>\r\n<String>\r\n<Name> </Name>\r\n<Val>Close ActiveX Communication</Val>\r\n</String>\r\n<String>\r\n<Name> </Name>\r\n<Val>Power Supplies OFF</Val>\r\n</String>\r\n<String>\r\n<Name> </Name>\r\n<Val>Reset Mux Switching</Val>\r\n</String>\r\n<String>\r\n<Name> </Name>\r\n<Val>Close VISA Sessions</Val>\r\n</String>\r\n<String>\r\n<Name> </Name>\r\n<Val>Collect TDC Data</Val>\r\n</String>\r\n<String>\r\n<Name> </Name>\r\n<Val>Passed</Val>\r\n</String>\r\n<String>\r\n<Name> </Name>\r\n<Val>Passed</Val>\r\n</String>\r\n<String>\r\n<Name> </Name>\r\n<Val>Passed</Val>\r\n</String>\r\n<String>\r\n<Name> </Name>\r\n<Val>Passed</Val>\r\n</String>\r\n<String>\r\n<Name> </Name>\r\n<Val>Done</Val>\r\n</String>\r\n<String>\r\n<Name> </Name>\r\n<Val>Passed</Val>\r\n</String>\r\n<String>\r\n<Name> </Name>\r\n<Val>Skipped</Val>\r\n</String>\r\n<String>\r\n<Name> </Name>\r\n<Val>Passed</Val>\r\n</String>\r\n<String>\r\n<Name> </Name>\r\n<Val>Passed</Val>\r\n</String>\r\n<String>\r\n<Name> </Name>\r\n<Val>Passed</Val>\r\n</String>\r\n<String>\r\n<Name> </Name>\r\n<Val>Done</Val>\r\n</String>\r\n<String>\r\n<Name> </Name>\r\n<Val>Done</Val>\r\n</String>\r\n<String>\r\n<Name> </Name>\r\n<Val>Passed</Val>\r\n</String>\r\n<String>\r\n<Name> </Name>\r\n<Val>Passed</Val>\r\n</String>\r\n<String>\r\n<Name> </Name>\r\n<Val>Passed</Val>\r\n</String>\r\n<String>\r\n<Name> </Name>\r\n<Val>Passed</Val>\r\n</String>\r\n<String>\r\n<Name> </Name>\r\n<Val>Passed</Val>\r\n</String>\r\n<String>\r\n<Name> </Name>\r\n<Val>Passed</Val>\r\n</String>\r\n<String>\r\n<Name> </Name>\r\n<Val>Passed</Val>\r\n</String>\r\n<String>\r\n<Name> </Name>\r\n<Val>Passed</Val>\r\n</String>\r\n<String>\r\n<Name> </Name>\r\n<Val>Passed</Val>\r\n</String>\r\n<String>\r\n<Name> </Name>\r\n<Val>Passed</Val>\r\n</String>\r\n<String>\r\n<Name> </Name>\r\n<Val>Passed</Val>\r\n</String>\r\n<String>\r\n<Name> </Name>\r\n<Val>Passed</Val>\r\n</String>\r\n<String>\r\n<Name> </Name>\r\n<Val>Passed</Val>\r\n</String>\r\n<String>\r\n<Name> </Name>\r\n<Val>Passed</Val>\r\n</String>\r\n<String>\r\n<Name> </Name>\r\n<Val>Passed</Val>\r\n</String>\r\n<String>\r\n<Name> </Name>\r\n<Val>Passed</Val>\r\n</String>\r\n<String>\r\n<Name> </Name>\r\n<Val>Passed</Val>\r\n</String>\r\n<String>\r\n<Name> </Name>\r\n<Val>Passed</Val>\r\n</String>\r\n<String>\r\n<Name> </Name>\r\n<Val>Skipped</Val>\r\n</String>\r\n<String>\r\n<Name> </Name>\r\n<Val>Passed</Val>\r\n</String>\r\n<String>\r\n<Name> </Name>\r\n<Val>Passed</Val>\r\n</String>\r\n<String>\r\n<Name> </Name>\r\n<Val>Passed</Val>\r\n</String>\r\n<String>\r\n<Name> </Name>\r\n<Val>Passed</Val>\r\n</String>\r\n<String>\r\n<Name> </Name>\r\n<Val>Passed</Val>\r\n</String>\r\n<String>\r\n<Name> </Name>\r\n<Val>Passed</Val>\r\n</String>\r\n<String>\r\n<Name> </Name>\r\n<Val>Passed</Val>\r\n</String>\r\n<String>\r\n<Name> </Name>\r\n<Val>Done</Val>\r\n</String>\r\n<String>\r\n<Name> </Name>\r\n<Val>Skipped</Val>\r\n</String>\r\n<String>\r\n<Name> </Name>\r\n<Val>Skipped</Val>\r\n</String>\r\n<String>\r\n<Name> </Name>\r\n<Val>Skipped</Val>\r\n</String>\r\n<String>\r\n<Name> </Name>\r\n<Val>Passed</Val>\r\n</String>\r\n<String>\r\n<Name> </Name>\r\n<Val>Passed</Val>\r\n</String>\r\n<String>\r\n<Name> </Name>\r\n<Val>Passed</Val>\r\n</String>\r\n<String>\r\n<Name> </Name>\r\n<Val>Passed</Val>\r\n</String>\r\n<String>\r\n<Name> </Name>\r\n<Val>Passed</Val>\r\n</String>\r\n<String>\r\n<Name> </Name>\r\n<Val>Passed</Val>\r\n</String>\r\n<String>\r\n<Name> </Name>\r\n<Val>Passed</Val>\r\n</String>\r\n<String>\r\n<Name> </Name>\r\n<Val>Passed</Val>\r\n</String>\r\n<String>\r\n<Name> </Name>\r\n<Val>Passed</Val>\r\n</String>\r\n<String>\r\n<Name> </Name>\r\n<Val>Passed</Val>\r\n</String>\r\n<String>\r\n<Name> </Name>\r\n<Val>Passed</Val>\r\n</String>\r\n<String>\r\n<Name> </Name>\r\n<Val>Passed</Val>\r\n</String>\r\n<String>\r\n<Name> </Name>\r\n<Val>Passed</Val>\r\n</String>\r\n<String>\r\n<Name> </Name>\r\n<Val>Passed</Val>\r\n</String>\r\n<String>\r\n<Name> </Name>\r\n<Val>Passed</Val>\r\n</String>\r\n<String>\r\n<Name> </Name>\r\n<Val>Passed</Val>\r\n</String>\r\n<String>\r\n<Name> </Name>\r\n<Val>Skipped</Val>\r\n</String>\r\n<String>\r\n<Name> </Name>\r\n<Val>Passed</Val>\r\n</String>\r\n<String>\r\n<Name> </Name>\r\n<Val>Passed</Val>\r\n</String>\r\n<String>\r\n<Name> </Name>\r\n<Val>Passed</Val>\r\n</String>\r\n<String>\r\n<Name> </Name>\r\n<Val>Passed</Val>\r\n</String>\r\n<String>\r\n<Name> </Name>\r\n<Val>Passed</Val>\r\n</String>\r\n<String>\r\n<Name> </Name>\r\n<Val>Passed</Val>\r\n</String>\r\n<String>\r\n<Name> </Name>\r\n<Val>Passed</Val>\r\n</String>\r\n<String>\r\n<Name> </Name>\r\n<Val>Passed</Val>\r\n</String>\r\n<String>\r\n<Name> </Name>\r\n<Val>Passed</Val>\r\n</String>\r\n<String>\r\n<Name> </Name>\r\n<Val>Passed</Val>\r\n</String>\r\n<String>\r\n<Name> </Name>\r\n<Val>Passed</Val>\r\n</String>\r\n<String>\r\n<Name> </Name>\r\n<Val>Passed</Val>\r\n</String>\r\n<String>\r\n<Name> </Name>\r\n<Val>Skipped</Val>\r\n</String>\r\n<String>\r\n<Name> </Name>\r\n<Val>Skipped</Val>\r\n</String>\r\n<String>\r\n<Name> </Name>\r\n<Val>Passed</Val>\r\n</String>\r\n<String>\r\n<Name> </Name>\r\n<Val>Skipped</Val>\r\n</String>\r\n<String>\r\n<Name> </Name>\r\n<Val>Passed</Val>\r\n</String>\r\n<String>\r\n<Name> </Name>\r\n<Val>Passed</Val>\r\n</String>\r\n<String>\r\n<Name> </Name>\r\n<Val>Passed</Val>\r\n</String>\r\n<String>\r\n<Name> </Name>\r\n<Val>Passed</Val>\r\n</String>\r\n<String>\r\n<Name> </Name>\r\n<Val>Passed</Val>\r\n</String>\r\n<String>\r\n<Name> </Name>\r\n<Val>Passed</Val>\r\n</String>\r\n<String>\r\n<Name> </Name>\r\n<Val>Passed</Val>\r\n</String>\r\n<String>\r\n<Name> </Name>\r\n<Val>Passed</Val>\r\n</String>\r\n<String>\r\n<Name> </Name>\r\n<Val>Passed</Val>\r\n</String>\r\n<String>\r\n<Name> </Name>\r\n<Val>Passed</Val>\r\n</String>\r\n<String>\r\n<Name> </Name>\r\n<Val>Passed</Val>\r\n</String>\r\n<String>\r\n<Name> </Name>\r\n<Val>Passed</Val>\r\n</String>\r\n<String>\r\n<Name> </Name>\r\n<Val>Passed</Val>\r\n</String>\r\n<String>\r\n<Name> </Name>\r\n<Val>Passed</Val>\r\n</String>\r\n<String>\r\n<Name> </Name>\r\n<Val>Passed</Val>\r\n</String>\r\n<String>\r\n<Name> </Name>\r\n<Val>Passed</Val>\r\n</String>\r\n<String>\r\n<Name> </Name>\r\n<Val>Passed</Val>\r\n</String>\r\n<String>\r\n<Name> </Name>\r\n<Val>Passed</Val>\r\n</String>\r\n<String>\r\n<Name> </Name>\r\n<Val>Passed</Val>\r\n</String>\r\n<String>\r\n<Name> </Name>\r\n<Val>Passed</Val>\r\n</String>\r\n<String>\r\n<Name> </Name>\r\n<Val>Passed</Val>\r\n</String>\r\n<String>\r\n<Name> </Name>\r\n<Val>Passed</Val>\r\n</String>\r\n<String>\r\n<Name> </Name>\r\n<Val>Passed</Val>\r\n</String>\r\n<String>\r\n<Name> </Name>\r\n<Val>Passed</Val>\r\n</String>\r\n<String>\r\n<Name> </Name>\r\n<Val>Passed</Val>\r\n</String>\r\n<String>\r\n<Name> </Name>\r\n<Val>Passed</Val>\r\n</String>\r\n<String>\r\n<Name> </Name>\r\n<Val>Passed</Val>\r\n</String>\r\n<String>\r\n<Name> </Name>\r\n<Val>Passed</Val>\r\n</String>\r\n<String>\r\n<Name> </Name>\r\n<Val>Passed</Val>\r\n</String>\r\n<String>\r\n<Name> </Name>\r\n<Val>Passed</Val>\r\n</String>\r\n<String>\r\n<Name> </Name>\r\n<Val>Passed</Val>\r\n</String>\r\n<String>\r\n<Name> </Name>\r\n<Val>Passed</Val>\r\n</String>\r\n<String>\r\n<Name> </Name>\r\n<Val>Passed</Val>\r\n</String>\r\n<String>\r\n<Name> </Name>\r\n<Val>Passed</Val>\r\n</String>\r\n<String>\r\n<Name> </Name>\r\n<Val>Passed</Val>\r\n</String>\r\n<String>\r\n<Name> </Name>\r\n<Val>Passed</Val>\r\n</String>\r\n<String>\r\n<Name> </Name>\r\n<Val>Passed</Val>\r\n</String>\r\n<String>\r\n<Name> </Name>\r\n<Val>Passed</Val>\r\n</String>\r\n<String>\r\n<Name> </Name>\r\n<Val>Passed</Val>\r\n</String>\r\n<String>\r\n<Name> </Name>\r\n<Val>Passed</Val>\r\n</String>\r\n<String>\r\n<Name> </Name>\r\n<Val>Passed</Val>\r\n</String>\r\n<String>\r\n<Name> </Name>\r\n<Val>Passed</Val>\r\n</String>\r\n<String>\r\n<Name> </Name>\r\n<Val>Passed</Val>\r\n</String>\r\n<String>\r\n<Name> </Name>\r\n<Val>Passed</Val>\r\n</String>\r\n<String>\r\n<Name> </Name>\r\n<Val>Passed</Val>\r\n</String>\r\n<String>\r\n<Name> </Name>\r\n<Val>Passed</Val>\r\n</String>\r\n<String>\r\n<Name> </Name>\r\n<Val>Passed</Val>\r\n</String>\r\n<String>\r\n<Name> </Name>\r\n<Val>Passed</Val>\r\n</String>\r\n<String>\r\n<Name> </Name>\r\n<Val>Passed</Val>\r\n</String>\r\n<String>\r\n<Name> </Name>\r\n<Val>Passed</Val>\r\n</String>\r\n<String>\r\n<Name> </Name>\r\n<Val>Passed</Val>\r\n</String>\r\n<String>\r\n<Name> </Name>\r\n<Val>Passed</Val>\r\n</String>\r\n<String>\r\n<Name> </Name>\r\n<Val>Passed</Val>\r\n</String>\r\n<String>\r\n<Name> </Name>\r\n<Val>Passed</Val>\r\n</String>\r\n<String>\r\n<Name> </Name>\r\n<Val>Passed</Val>\r\n</String>\r\n<String>\r\n<Name> </Name>\r\n<Val>Passed</Val>\r\n</String>\r\n<String>\r\n<Name> </Name>\r\n<Val>Passed</Val>\r\n</String>\r\n<String>\r\n<Name> </Name>\r\n<Val>Passed</Val>\r\n</String>\r\n<String>\r\n<Name> </Name>\r\n<Val>Passed</Val>\r\n</String>\r\n<String>\r\n<Name> </Name>\r\n<Val>Passed</Val>\r\n</String>\r\n<String>\r\n<Name> </Name>\r\n<Val>Passed</Val>\r\n</String>\r\n<String>\r\n<Name> </Name>\r\n<Val>Passed</Val>\r\n</String>\r\n<String>\r\n<Name> </Name>\r\n<Val>Passed</Val>\r\n</String>\r\n<String>\r\n<Name> </Name>\r\n<Val>Passed</Val>\r\n</String>\r\n<String>\r\n<Name> </Name>\r\n<Val>Passed</Val>\r\n</String>\r\n<String>\r\n<Name> </Name>\r\n<Val>Passed</Val>\r\n</String>\r\n<String>\r\n<Name> </Name>\r\n<Val>Passed</Val>\r\n</String>\r\n<String>\r\n<Name> </Name>\r\n<Val>Passed</Val>\r\n</String>\r\n<String>\r\n<Name> </Name>\r\n<Val>Passed</Val>\r\n</String>\r\n<String>\r\n<Name> </Name>\r\n<Val>Passed</Val>\r\n</String>\r\n<String>\r\n<Name> </Name>\r\n<Val>Passed</Val>\r\n</String>\r\n<String>\r\n<Name> </Name>\r\n<Val>Passed</Val>\r\n</String>\r\n<String>\r\n<Name> </Name>\r\n<Val>Passed</Val>\r\n</String>\r\n<String>\r\n<Name> </Name>\r\n<Val>Passed</Val>\r\n</String>\r\n<String>\r\n<Name> </Name>\r\n<Val>Passed</Val>\r\n</String>\r\n<String>\r\n<Name> </Name>\r\n<Val>Passed</Val>\r\n</String>\r\n<String>\r\n<Name> </Name>\r\n<Val>Passed</Val>\r\n</String>\r\n<String>\r\n<Name> </Name>\r\n<Val>Passed</Val>\r\n</String>\r\n<String>\r\n<Name> </Name>\r\n<Val>Passed</Val>\r\n</String>\r\n<String>\r\n<Name> </Name>\r\n<Val>Passed</Val>\r\n</String>\r\n<String>\r\n<Name> </Name>\r\n<Val>Passed</Val>\r\n</String>\r\n<String>\r\n<Name> </Name>\r\n<Val>Passed</Val>\r\n</String>\r\n<String>\r\n<Name> </Name>\r\n<Val>Passed</Val>\r\n</String>\r\n<String>\r\n<Name> </Name>\r\n<Val>Passed</Val>\r\n</String>\r\n<String>\r\n<Name> </Name>\r\n<Val>Passed</Val>\r\n</String>\r\n<String>\r\n<Name> </Name>\r\n<Val>Passed</Val>\r\n</String>\r\n<String>\r\n<Name> </Name>\r\n<Val>Passed</Val>\r\n</String>\r\n<String>\r\n<Name> </Name>\r\n<Val>Passed</Val>\r\n</String>\r\n<String>\r\n<Name> </Name>\r\n<Val>Passed</Val>\r\n</String>\r\n<String>\r\n<Name> </Name>\r\n<Val>Passed</Val>\r\n</String>\r\n<String>\r\n<Name> </Name>\r\n<Val>Passed</Val>\r\n</String>\r\n<String>\r\n<Name> </Name>\r\n<Val>Passed</Val>\r\n</String>\r\n<String>\r\n<Name> </Name>\r\n<Val>Passed</Val>\r\n</String>\r\n<String>\r\n<Name> </Name>\r\n<Val>Passed</Val>\r\n</String>\r\n<String>\r\n<Name> </Name>\r\n<Val>Passed</Val>\r\n</String>\r\n<String>\r\n<Name> </Name>\r\n<Val>Passed</Val>\r\n</String>\r\n<String>\r\n<Name> </Name>\r\n<Val>Passed</Val>\r\n</String>\r\n<String>\r\n<Name> </Name>\r\n<Val>Passed</Val>\r\n</String>\r\n<String>\r\n<Name> </Name>\r\n<Val>Passed</Val>\r\n</String>\r\n<String>\r\n<Name> </Name>\r\n<Val>Passed</Val>\r\n</String>\r\n<String>\r\n<Name> </Name>\r\n<Val>Passed</Val>\r\n</String>\r\n<String>\r\n<Name> </Name>\r\n<Val>Passed</Val>\r\n</String>\r\n<String>\r\n<Name> </Name>\r\n<Val>Passed</Val>\r\n</String>\r\n<String>\r\n<Name> </Name>\r\n<Val>Passed</Val>\r\n</String>\r\n<String>\r\n<Name> </Name>\r\n<Val>Passed</Val>\r\n</String>\r\n<String>\r\n<Name> </Name>\r\n<Val>Passed</Val>\r\n</String>\r\n<String>\r\n<Name> </Name>\r\n<Val>Passed</Val>\r\n</String>\r\n<String>\r\n<Name> </Name>\r\n<Val>Passed</Val>\r\n</String>\r\n<String>\r\n<Name> </Name>\r\n<Val>Passed</Val>\r\n</String>\r\n<String>\r\n<Name> </Name>\r\n<Val>Passed</Val>\r\n</String>\r\n<String>\r\n<Name> </Name>\r\n<Val>Passed</Val>\r\n</String>\r\n<String>\r\n<Name> </Name>\r\n<Val>Passed</Val>\r\n</String>\r\n<String>\r\n<Name> </Name>\r\n<Val>Passed</Val>\r\n</String>\r\n<String>\r\n<Name> </Name>\r\n<Val>Passed</Val>\r\n</String>\r\n<String>\r\n<Name> </Name>\r\n<Val>Passed</Val>\r\n</String>\r\n<String>\r\n<Name> </Name>\r\n<Val>Skipped</Val>\r\n</String>\r\n<String>\r\n<Name> </Name>\r\n<Val>Passed</Val>\r\n</String>\r\n<String>\r\n<Name> </Name>\r\n<Val>Passed</Val>\r\n</String>\r\n<String>\r\n<Name> </Name>\r\n<Val>Passed</Val>\r\n</String>\r\n<String>\r\n<Name> </Name>\r\n<Val>Passed</Val>\r\n</String>\r\n<String>\r\n<Name> </Name>\r\n<Val>Passed</Val>\r\n</String>\r\n<String>\r\n<Name> </Name>\r\n<Val>Passed</Val>\r\n</String>\r\n<String>\r\n<Name> </Name>\r\n<Val>Passed</Val>\r\n</String>\r\n<String>\r\n<Name> </Name>\r\n<Val>Passed</Val>\r\n</String>\r\n<String>\r\n<Name> </Name>\r\n<Val>Passed</Val>\r\n</String>\r\n<String>\r\n<Name> </Name>\r\n<Val>Passed</Val>\r\n</String>\r\n<String>\r\n<Name> </Name>\r\n<Val>Passed</Val>\r\n</String>\r\n<String>\r\n<Name> </Name>\r\n<Val>Passed</Val>\r\n</String>\r\n<String>\r\n<Name> </Name>\r\n<Val>Passed</Val>\r\n</String>\r\n<String>\r\n<Name> </Name>\r\n<Val>Passed</Val>\r\n</String>\r\n<String>\r\n<Name> </Name>\r\n<Val>Passed</Val>\r\n</String>\r\n<String>\r\n<Name> </Name>\r\n<Val>Passed</Val>\r\n</String>\r\n<String>\r\n<Name> </Name>\r\n<Val>Passed</Val>\r\n</String>\r\n<String>\r\n<Name> </Name>\r\n<Val>Passed</Val>\r\n</String>\r\n<String>\r\n<Name> </Name>\r\n<Val>Passed</Val>\r\n</String>\r\n<String>\r\n<Name> </Name>\r\n<Val>Passed</Val>\r\n</String>\r\n<String>\r\n<Name> </Name>\r\n<Val>Passed</Val>\r\n</String>\r\n<String>\r\n<Name> </Name>\r\n<Val>Passed</Val>\r\n</String>\r\n<String>\r\n<Name> </Name>\r\n<Val>Passed</Val>\r\n</String>\r\n<String>\r\n<Name> </Name>\r\n<Val>Passed</Val>\r\n</String>\r\n<String>\r\n<Name> </Name>\r\n<Val>Passed</Val>\r\n</String>\r\n<String>\r\n<Name> </Name>\r\n<Val>Passed</Val>\r\n</String>\r\n<String>\r\n<Name> </Name>\r\n<Val>Passed</Val>\r\n</String>\r\n<String>\r\n<Name> </Name>\r\n<Val>Passed</Val>\r\n</String>\r\n<String>\r\n<Name> </Name>\r\n<Val>Passed</Val>\r\n</String>\r\n<String>\r\n<Name> </Name>\r\n<Val>Passed</Val>\r\n</String>\r\n<String>\r\n<Name> </Name>\r\n<Val>Passed</Val>\r\n</String>\r\n<String>\r\n<Name> </Name>\r\n<Val>Passed</Val>\r\n</String>\r\n<String>\r\n<Name> </Name>\r\n<Val>Passed</Val>\r\n</String>\r\n<String>\r\n<Name> </Name>\r\n<Val>Passed</Val>\r\n</String>\r\n<String>\r\n<Name> </Name>\r\n<Val>Passed</Val>\r\n</String>\r\n<String>\r\n<Name> </Name>\r\n<Val>Passed</Val>\r\n</String>\r\n<String>\r\n<Name> </Name>\r\n<Val>Passed</Val>\r\n</String>\r\n<String>\r\n<Name> </Name>\r\n<Val>Passed</Val>\r\n</String>\r\n<String>\r\n<Name> </Name>\r\n<Val>Passed</Val>\r\n</String>\r\n<String>\r\n<Name> </Name>\r\n<Val>Passed</Val>\r\n</String>\r\n<String>\r\n<Name> </Name>\r\n<Val>Passed</Val>\r\n</String>\r\n<String>\r\n<Name> </Name>\r\n<Val>Passed</Val>\r\n</String>\r\n<String>\r\n<Name> </Name>\r\n<Val>Passed</Val>\r\n</String>\r\n<String>\r\n<Name> </Name>\r\n<Val>Passed</Val>\r\n</String>\r\n<String>\r\n<Name> </Name>\r\n<Val>Passed</Val>\r\n</String>\r\n<String>\r\n<Name> </Name>\r\n<Val>Passed</Val>\r\n</String>\r\n<String>\r\n<Name> </Name>\r\n<Val>Passed</Val>\r\n</String>\r\n<String>\r\n<Name> </Name>\r\n<Val>Passed</Val>\r\n</String>\r\n<String>\r\n<Name> </Name>\r\n<Val>Passed</Val>\r\n</String>\r\n<String>\r\n<Name> </Name>\r\n<Val>Passed</Val>\r\n</String>\r\n<String>\r\n<Name> </Name>\r\n<Val>Passed</Val>\r\n</String>\r\n<String>\r\n<Name> </Name>\r\n<Val>Passed</Val>\r\n</String>\r\n<String>\r\n<Name> </Name>\r\n<Val>Passed</Val>\r\n</String>\r\n<String>\r\n<Name> </Name>\r\n<Val>Passed</Val>\r\n</String>\r\n<String>\r\n<Name> </Name>\r\n<Val>Passed</Val>\r\n</String>\r\n<String>\r\n<Name> </Name>\r\n<Val>Passed</Val>\r\n</String>\r\n<String>\r\n<Name> </Name>\r\n<Val>Passed</Val>\r\n</String>\r\n<String>\r\n<Name> </Name>\r\n<Val>Passed</Val>\r\n</String>\r\n<String>\r\n<Name> </Name>\r\n<Val>Passed</Val>\r\n</String>\r\n<String>\r\n<Name> </Name>\r\n<Val>Passed</Val>\r\n</String>\r\n<String>\r\n<Name> </Name>\r\n<Val>Passed</Val>\r\n</String>\r\n<String>\r\n<Name> </Name>\r\n<Val>Passed</Val>\r\n</String>\r\n<String>\r\n<Name> </Name>\r\n<Val>Passed</Val>\r\n</String>\r\n<String>\r\n<Name> </Name>\r\n<Val>Passed</Val>\r\n</String>\r\n<String>\r\n<Name> </Name>\r\n<Val>Passed</Val>\r\n</String>\r\n<String>\r\n<Name> </Name>\r\n<Val>Passed</Val>\r\n</String>\r\n<String>\r\n<Name> </Name>\r\n<Val>Passed</Val>\r\n</String>\r\n<String>\r\n<Name> </Name>\r\n<Val>Passed</Val>\r\n</String>\r\n<String>\r\n<Name> </Name>\r\n<Val>Passed</Val>\r\n</String>\r\n<String>\r\n<Name> </Name>\r\n<Val>Passed</Val>\r\n</String>\r\n<String>\r\n<Name> </Name>\r\n<Val>Passed</Val>\r\n</String>\r\n<String>\r\n<Name> </Name>\r\n<Val>Passed</Val>\r\n</String>\r\n<String>\r\n<Name> </Name>\r\n<Val>Passed</Val>\r\n</String>\r\n<String>\r\n<Name> </Name>\r\n<Val>Passed</Val>\r\n</String>\r\n<String>\r\n<Name> </Name>\r\n<Val>Passed</Val>\r\n</String>\r\n<String>\r\n<Name> </Name>\r\n<Val>Passed</Val>\r\n</String>\r\n<String>\r\n<Name> </Name>\r\n<Val>Passed</Val>\r\n</String>\r\n<String>\r\n<Name> </Name>\r\n<Val>Passed</Val>\r\n</String>\r\n<String>\r\n<Name> </Name>\r\n<Val>Passed</Val>\r\n</String>\r\n<String>\r\n<Name> </Name>\r\n<Val>Passed</Val>\r\n</String>\r\n<String>\r\n<Name> </Name>\r\n<Val>Passed</Val>\r\n</String>\r\n<String>\r\n<Name> </Name>\r\n<Val>Passed</Val>\r\n</String>\r\n<String>\r\n<Name> </Name>\r\n<Val>Passed</Val>\r\n</String>\r\n<String>\r\n<Name> </Name>\r\n<Val>Passed</Val>\r\n</String>\r\n<String>\r\n<Name> </Name>\r\n<Val>Passed</Val>\r\n</String>\r\n<String>\r\n<Name> </Name>\r\n<Val>Passed</Val>\r\n</String>\r\n<String>\r\n<Name> </Name>\r\n<Val>Passed</Val>\r\n</String>\r\n<String>\r\n<Name> </Name>\r\n<Val>Passed</Val>\r\n</String>\r\n<String>\r\n<Name> </Name>\r\n<Val>Passed</Val>\r\n</String>\r\n<String>\r\n<Name> </Name>\r\n<Val>Passed</Val>\r\n</String>\r\n<String>\r\n<Name> </Name>\r\n<Val>Passed</Val>\r\n</String>\r\n<String>\r\n<Name> </Name>\r\n<Val>Passed</Val>\r\n</String>\r\n<String>\r\n<Name> </Name>\r\n<Val>Passed</Val>\r\n</String>\r\n<String>\r\n<Name> </Name>\r\n<Val>Passed</Val>\r\n</String>\r\n<String>\r\n<Name> </Name>\r\n<Val>Passed</Val>\r\n</String>\r\n<String>\r\n<Name> </Name>\r\n<Val>Passed</Val>\r\n</String>\r\n<String>\r\n<Name> </Name>\r\n<Val>Passed</Val>\r\n</String>\r\n<String>\r\n<Name> </Name>\r\n<Val>Passed</Val>\r\n</String>\r\n<String>\r\n<Name> </Name>\r\n<Val>Passed</Val>\r\n</String>\r\n<String>\r\n<Name> </Name>\r\n<Val>Passed</Val>\r\n</String>\r\n<String>\r\n<Name> </Name>\r\n<Val>Passed</Val>\r\n</String>\r\n<String>\r\n<Name> </Name>\r\n<Val>Passed</Val>\r\n</String>\r\n<String>\r\n<Name> </Name>\r\n<Val>Passed</Val>\r\n</String>\r\n<String>\r\n<Name> </Name>\r\n<Val>Passed</Val>\r\n</String>\r\n<String>\r\n<Name> </Name>\r\n<Val>Passed</Val>\r\n</String>\r\n<String>\r\n<Name> </Name>\r\n<Val>Passed</Val>\r\n</String>\r\n<String>\r\n<Name> </Name>\r\n<Val>Passed</Val>\r\n</String>\r\n<String>\r\n<Name> </Name>\r\n<Val>Passed</Val>\r\n</String>\r\n<String>\r\n<Name> </Name>\r\n<Val>Passed</Val>\r\n</String>\r\n<String>\r\n<Name> </Name>\r\n<Val>Passed</Val>\r\n</String>\r\n<String>\r\n<Name> </Name>\r\n<Val>Passed</Val>\r\n</String>\r\n<String>\r\n<Name> </Name>\r\n<Val>Passed</Val>\r\n</String>\r\n<String>\r\n<Name> </Name>\r\n<Val>Passed</Val>\r\n</String>\r\n<String>\r\n<Name> </Name>\r\n<Val>Passed</Val>\r\n</String>\r\n<String>\r\n<Name> </Name>\r\n<Val>Passed</Val>\r\n</String>\r\n<String>\r\n<Name> </Name>\r\n<Val>Passed</Val>\r\n</String>\r\n<String>\r\n<Name> </Name>\r\n<Val>Passed</Val>\r\n</String>\r\n<String>\r\n<Name> </Name>\r\n<Val>Passed</Val>\r\n</String>\r\n<String>\r\n<Name> </Name>\r\n<Val>Passed</Val>\r\n</String>\r\n<String>\r\n<Name> </Name>\r\n<Val>Passed</Val>\r\n</String>\r\n<String>\r\n<Name> </Name>\r\n<Val>Passed</Val>\r\n</String>\r\n<String>\r\n<Name> </Name>\r\n<Val>Passed</Val>\r\n</String>\r\n<String>\r\n<Name> </Name>\r\n<Val>Passed</Val>\r\n</String>\r\n<String>\r\n<Name> </Name>\r\n<Val>Passed</Val>\r\n</String>\r\n<String>\r\n<Name> </Name>\r\n<Val>Passed</Val>\r\n</String>\r\n<String>\r\n<Name> </Name>\r\n<Val>Passed</Val>\r\n</String>\r\n<String>\r\n<Name> </Name>\r\n<Val>Passed</Val>\r\n</String>\r\n<String>\r\n<Name> </Name>\r\n<Val>Passed</Val>\r\n</String>\r\n<String>\r\n<Name> </Name>\r\n<Val>Passed</Val>\r\n</String>\r\n<String>\r\n<Name> </Name>\r\n<Val>Passed</Val>\r\n</String>\r\n<String>\r\n<Name> </Name>\r\n<Val>Passed</Val>\r\n</String>\r\n<String>\r\n<Name> </Name>\r\n<Val>Passed</Val>\r\n</String>\r\n<String>\r\n<Name> </Name>\r\n<Val>Passed</Val>\r\n</String>\r\n<String>\r\n<Name> </Name>\r\n<Val>Passed</Val>\r\n</String>\r\n<String>\r\n<Name> </Name>\r\n<Val>Passed</Val>\r\n</String>\r\n<String>\r\n<Name> </Name>\r\n<Val>Passed</Val>\r\n</String>\r\n<String>\r\n<Name> </Name>\r\n<Val>Passed</Val>\r\n</String>\r\n<String>\r\n<Name> </Name>\r\n<Val>Passed</Val>\r\n</String>\r\n<String>\r\n<Name> </Name>\r\n<Val>Passed</Val>\r\n</String>\r\n<String>\r\n<Name> </Name>\r\n<Val>Passed</Val>\r\n</String>\r\n<String>\r\n<Name> </Name>\r\n<Val>Passed</Val>\r\n</String>\r\n<String>\r\n<Name> </Name>\r\n<Val>Passed</Val>\r\n</String>\r\n<String>\r\n<Name> </Name>\r\n<Val>Passed</Val>\r\n</String>\r\n<String>\r\n<Name> </Name>\r\n<Val>Passed</Val>\r\n</String>\r\n<String>\r\n<Name> </Name>\r\n<Val>Passed</Val>\r\n</String>\r\n<String>\r\n<Name> </Name>\r\n<Val>Passed</Val>\r\n</String>\r\n<String>\r\n<Name> </Name>\r\n<Val>Passed</Val>\r\n</String>\r\n<String>\r\n<Name> </Name>\r\n<Val>Passed</Val>\r\n</String>\r\n<String>\r\n<Name> </Name>\r\n<Val>Passed</Val>\r\n</String>\r\n<String>\r\n<Name> </Name>\r\n<Val>Passed</Val>\r\n</String>\r\n<String>\r\n<Name> </Name>\r\n<Val>Passed</Val>\r\n</String>\r\n<String>\r\n<Name> </Name>\r\n<Val>Passed</Val>\r\n</String>\r\n<String>\r\n<Name> </Name>\r\n<Val>Passed</Val>\r\n</String>\r\n<String>\r\n<Name> </Name>\r\n<Val>Passed</Val>\r\n</String>\r\n<String>\r\n<Name> </Name>\r\n<Val>Passed</Val>\r\n</String>\r\n<String>\r\n<Name> </Name>\r\n<Val>Passed</Val>\r\n</String>\r\n<String>\r\n<Name> </Name>\r\n<Val>Passed</Val>\r\n</String>\r\n<String>\r\n<Name> </Name>\r\n<Val>Passed</Val>\r\n</String>\r\n<String>\r\n<Name> </Name>\r\n<Val>Passed</Val>\r\n</String>\r\n<String>\r\n<Name> </Name>\r\n<Val>Passed</Val>\r\n</String>\r\n<String>\r\n<Name> </Name>\r\n<Val>Passed</Val>\r\n</String>\r\n<String>\r\n<Name> </Name>\r\n<Val>Passed</Val>\r\n</String>\r\n<String>\r\n<Name> </Name>\r\n<Val>Passed</Val>\r\n</String>\r\n<String>\r\n<Name> </Name>\r\n<Val>Passed</Val>\r\n</String>\r\n<String>\r\n<Name> </Name>\r\n<Val>Passed</Val>\r\n</String>\r\n<String>\r\n<Name> </Name>\r\n<Val>Passed</Val>\r\n</String>\r\n<String>\r\n<Name> </Name>\r\n<Val>Passed</Val>\r\n</String>\r\n<String>\r\n<Name> </Name>\r\n<Val>Passed</Val>\r\n</String>\r\n<String>\r\n<Name> </Name>\r\n<Val>Passed</Val>\r\n</String>\r\n<String>\r\n<Name> </Name>\r\n<Val>Passed</Val>\r\n</String>\r\n<String>\r\n<Name> </Name>\r\n<Val>Passed</Val>\r\n</String>\r\n<String>\r\n<Name> </Name>\r\n<Val>Passed</Val>\r\n</String>\r\n<String>\r\n<Name> </Name>\r\n<Val>Passed</Val>\r\n</String>\r\n<String>\r\n<Name> </Name>\r\n<Val>Passed</Val>\r\n</String>\r\n<String>\r\n<Name> </Name>\r\n<Val>Passed</Val>\r\n</String>\r\n<String>\r\n<Name> </Name>\r\n<Val>Passed</Val>\r\n</String>\r\n<String>\r\n<Name> </Name>\r\n<Val>Passed</Val>\r\n</String>\r\n<String>\r\n<Name> </Name>\r\n<Val>Passed</Val>\r\n</String>\r\n<String>\r\n<Name> </Name>\r\n<Val>Passed</Val>\r\n</String>\r\n<String>\r\n<Name> </Name>\r\n<Val>Passed</Val>\r\n</String>\r\n<String>\r\n<Name> </Name>\r\n<Val>Passed</Val>\r\n</String>\r\n<String>\r\n<Name> </Name>\r\n<Val>Passed</Val>\r\n</String>\r\n<String>\r\n<Name> </Name>\r\n<Val>Passed</Val>\r\n</String>\r\n<String>\r\n<Name> </Name>\r\n<Val>Passed</Val>\r\n</String>\r\n<String>\r\n<Name> </Name>\r\n<Val>Passed</Val>\r\n</String>\r\n<String>\r\n<Name> </Name>\r\n<Val>Passed</Val>\r\n</String>\r\n<String>\r\n<Name> </Name>\r\n<Val>Passed</Val>\r\n</String>\r\n<String>\r\n<Name> </Name>\r\n<Val>Passed</Val>\r\n</String>\r\n<String>\r\n<Name> </Name>\r\n<Val>Passed</Val>\r\n</String>\r\n<String>\r\n<Name> </Name>\r\n<Val>Passed</Val>\r\n</String>\r\n<String>\r\n<Name> </Name>\r\n<Val>Passed</Val>\r\n</String>\r\n<String>\r\n<Name> </Name>\r\n<Val>Passed</Val>\r\n</String>\r\n<String>\r\n<Name> </Name>\r\n<Val>Passed</Val>\r\n</String>\r\n<String>\r\n<Name> </Name>\r\n<Val>Passed</Val>\r\n</String>\r\n<String>\r\n<Name> </Name>\r\n<Val>Passed</Val>\r\n</String>\r\n<String>\r\n<Name> </Name>\r\n<Val>Passed</Val>\r\n</String>\r\n<String>\r\n<Name> </Name>\r\n<Val>Passed</Val>\r\n</String>\r\n<String>\r\n<Name> </Name>\r\n<Val>Passed</Val>\r\n</String>\r\n<String>\r\n<Name> </Name>\r\n<Val>Passed</Val>\r\n</String>\r\n<String>\r\n<Name> </Name>\r\n<Val>Passed</Val>\r\n</String>\r\n<String>\r\n<Name> </Name>\r\n<Val>Passed</Val>\r\n</String>\r\n<String>\r\n<Name> </Name>\r\n<Val>Passed</Val>\r\n</String>\r\n<String>\r\n<Name> </Name>\r\n<Val>Passed</Val>\r\n</String>\r\n<String>\r\n<Name> </Name>\r\n<Val>Passed</Val>\r\n</String>\r\n<String>\r\n<Name> </Name>\r\n<Val>Passed</Val>\r\n</String>\r\n<String>\r\n<Name> </Name>\r\n<Val>Passed</Val>\r\n</String>\r\n<String>\r\n<Name> </Name>\r\n<Val>Passed</Val>\r\n</String>\r\n<String>\r\n<Name> </Name>\r\n<Val>Passed</Val>\r\n</String>\r\n<String>\r\n<Name> </Name>\r\n<Val>Passed</Val>\r\n</String>\r\n<String>\r\n<Name> </Name>\r\n<Val>Passed</Val>\r\n</String>\r\n<String>\r\n<Name> </Name>\r\n<Val>Passed</Val>\r\n</String>\r\n<String>\r\n<Name> </Name>\r\n<Val>Passed</Val>\r\n</String>\r\n<String>\r\n<Name> </Name>\r\n<Val>Passed</Val>\r\n</String>\r\n<String>\r\n<Name> </Name>\r\n<Val>Passed</Val>\r\n</String>\r\n<String>\r\n<Name> </Name>\r\n<Val>Passed</Val>\r\n</String>\r\n<String>\r\n<Name> </Name>\r\n<Val>Passed</Val>\r\n</String>\r\n<String>\r\n<Name> </Name>\r\n<Val>Passed</Val>\r\n</String>\r\n<String>\r\n<Name> </Name>\r\n<Val>Passed</Val>\r\n</String>\r\n<String>\r\n<Name> </Name>\r\n<Val>Passed</Val>\r\n</String>\r\n<String>\r\n<Name> </Name>\r\n<Val>Passed</Val>\r\n</String>\r\n<String>\r\n<Name> </Name>\r\n<Val>Passed</Val>\r\n</String>\r\n<String>\r\n<Name> </Name>\r\n<Val>Passed</Val>\r\n</String>\r\n<String>\r\n<Name> </Name>\r\n<Val>Passed</Val>\r\n</String>\r\n<String>\r\n<Name> </Name>\r\n<Val>Passed</Val>\r\n</String>\r\n<String>\r\n<Name> </Name>\r\n<Val>Passed</Val>\r\n</String>\r\n<String>\r\n<Name> </Name>\r\n<Val>Passed</Val>\r\n</String>\r\n<String>\r\n<Name> </Name>\r\n<Val>Passed</Val>\r\n</String>\r\n<String>\r\n<Name> </Name>\r\n<Val>Passed</Val>\r\n</String>\r\n<String>\r\n<Name> </Name>\r\n<Val>Passed</Val>\r\n</String>\r\n<String>\r\n<Name> </Name>\r\n<Val>Passed</Val>\r\n</String>\r\n<String>\r\n<Name> </Name>\r\n<Val>Done</Val>\r\n</String>\r\n<String>\r\n<Name> </Name>\r\n<Val>Passed</Val>\r\n</String>\r\n<String>\r\n<Name> </Name>\r\n<Val>Passed</Val>\r\n</String>\r\n<String>\r\n<Name> </Name>\r\n<Val>Passed</Val>\r\n</String>\r\n<String>\r\n<Name> </Name>\r\n<Val>Skipped</Val>\r\n</String>\r\n<String>\r\n<Name> </Name>\r\n<Val>Passed</Val>\r\n</String>\r\n<String>\r\n<Name> </Name>\r\n<Val>Passed</Val>\r\n</String>\r\n<String>\r\n<Name> </Name>\r\n<Val>Passed</Val>\r\n</String>\r\n<String>\r\n<Name> </Name>\r\n<Val>Passed</Val>\r\n</String>\r\n<String>\r\n<Name> </Name>\r\n<Val>Passed</Val>\r\n</String>\r\n<String>\r\n<Name> </Name>\r\n<Val>Passed</Val>\r\n</String>\r\n<String>\r\n<Name> </Name>\r\n<Val>Passed</Val>\r\n</String>\r\n<String>\r\n<Name> </Name>\r\n<Val>Passed</Val>\r\n</String>\r\n<String>\r\n<Name> </Name>\r\n<Val>Passed</Val>\r\n</String>\r\n<String>\r\n<Name> </Name>\r\n<Val>Passed</Val>\r\n</String>\r\n<String>\r\n<Name> </Name>\r\n<Val>Passed</Val>\r\n</String>\r\n<String>\r\n<Name> </Name>\r\n<Val>Passed</Val>\r\n</String>\r\n<String>\r\n<Name> </Name>\r\n<Val>Passed</Val>\r\n</String>\r\n<String>\r\n<Name> </Name>\r\n<Val>Passed</Val>\r\n</String>\r\n<String>\r\n<Name> </Name>\r\n<Val>Passed</Val>\r\n</String>\r\n<String>\r\n<Name> </Name>\r\n<Val>Passed</Val>\r\n</String>\r\n<String>\r\n<Name> </Name>\r\n<Val>Passed</Val>\r\n</String>\r\n<String>\r\n<Name> </Name>\r\n<Val>Passed</Val>\r\n</String>\r\n<String>\r\n<Name> </Name>\r\n<Val>Passed</Val>\r\n</String>\r\n<String>\r\n<Name> </Name>\r\n<Val>Passed</Val>\r\n</String>\r\n<String>\r\n<Name> </Name>\r\n<Val>Passed</Val>\r\n</String>\r\n<String>\r\n<Name> </Name>\r\n<Val>Passed</Val>\r\n</String>\r\n<String>\r\n<Name> </Name>\r\n<Val>Passed</Val>\r\n</String>\r\n<String>\r\n<Name> </Name>\r\n<Val>Passed</Val>\r\n</String>\r\n<String>\r\n<Name> </Name>\r\n<Val>Passed</Val>\r\n</String>\r\n<String>\r\n<Name> </Name>\r\n<Val>Passed</Val>\r\n</String>\r\n<String>\r\n<Name> </Name>\r\n<Val>Passed</Val>\r\n</String>\r\n<String>\r\n<Name> </Name>\r\n<Val>Passed</Val>\r\n</String>\r\n<String>\r\n<Name> </Name>\r\n<Val>Passed</Val>\r\n</String>\r\n<String>\r\n<Name> </Name>\r\n<Val>Passed</Val>\r\n</String>\r\n<String>\r\n<Name> </Name>\r\n<Val>Passed</Val>\r\n</String>\r\n<String>\r\n<Name> </Name>\r\n<Val>Passed</Val>\r\n</String>\r\n<String>\r\n<Name> </Name>\r\n<Val>Passed</Val>\r\n</String>\r\n<String>\r\n<Name> </Name>\r\n<Val>Passed</Val>\r\n</String>\r\n<String>\r\n<Name> </Name>\r\n<Val>Passed</Val>\r\n</String>\r\n<String>\r\n<Name> </Name>\r\n<Val>Passed</Val>\r\n</String>\r\n<String>\r\n<Name> </Name>\r\n<Val>Passed</Val>\r\n</String>\r\n<String>\r\n<Name> </Name>\r\n<Val>Passed</Val>\r\n</String>\r\n<String>\r\n<Name> </Name>\r\n<Val>Passed</Val>\r\n</String>\r\n<String>\r\n<Name> </Name>\r\n<Val>Passed</Val>\r\n</String>\r\n<String>\r\n<Name> </Name>\r\n<Val>Passed</Val>\r\n</String>\r\n<String>\r\n<Name> </Name>\r\n<Val>Passed</Val>\r\n</String>\r\n<String>\r\n<Name> </Name>\r\n<Val>Passed</Val>\r\n</String>\r\n<String>\r\n<Name> </Name>\r\n<Val>Passed</Val>\r\n</String>\r\n<String>\r\n<Name> </Name>\r\n<Val>Passed</Val>\r\n</String>\r\n<String>\r\n<Name> </Name>\r\n<Val>Passed</Val>\r\n</String>\r\n<String>\r\n<Name> </Name>\r\n<Val>Passed</Val>\r\n</String>\r\n<String>\r\n<Name> </Name>\r\n<Val>Passed</Val>\r\n</String>\r\n<String>\r\n<Name> </Name>\r\n<Val>Passed</Val>\r\n</String>\r\n<String>\r\n<Name> </Name>\r\n<Val>Passed</Val>\r\n</String>\r\n<String>\r\n<Name> </Name>\r\n<Val>Passed</Val>\r\n</String>\r\n<String>\r\n<Name> </Name>\r\n<Val>Passed</Val>\r\n</String>\r\n<String>\r\n<Name> </Name>\r\n<Val>Passed</Val>\r\n</String>\r\n<String>\r\n<Name> </Name>\r\n<Val>Passed</Val>\r\n</String>\r\n<String>\r\n<Name> </Name>\r\n<Val>Passed</Val>\r\n</String>\r\n<String>\r\n<Name> </Name>\r\n<Val>Passed</Val>\r\n</String>\r\n<String>\r\n<Name> </Name>\r\n<Val>Passed</Val>\r\n</String>\r\n<String>\r\n<Name> </Name>\r\n<Val>Passed</Val>\r\n</String>\r\n<String>\r\n<Name> </Name>\r\n<Val>Done</Val>\r\n</String>\r\n<String>\r\n<Name> </Name>\r\n<Val>Passed</Val>\r\n</String>\r\n<String>\r\n<Name> </Name>\r\n<Val>Passed</Val>\r\n</String>\r\n<String>\r\n<Name> </Name>\r\n<Val>Passed</Val>\r\n</String>\r\n<String>\r\n<Name> </Name>\r\n<Val>Done</Val>\r\n</String>\r\n<String>\r\n<Name> </Name>\r\n<Val>Done</Val>\r\n</String>\r\n<String>\r\n<Name> </Name>\r\n<Val>Passed</Val>\r\n</String>\r\n<String>\r\n<Name> </Name>\r\n<Val>Done</Val>\r\n</String>\r\n<String>\r\n<Name> </Name>\r\n<Val>Passed</Val>\r\n</String>\r\n<String>\r\n<Name> </Name>\r\n<Val>PassFailTest</Val>\r\n</String>\r\n<String>\r\n<Name> </Name>\r\n<Val>PassFailTest</Val>\r\n</String>\r\n<String>\r\n<Name> </Name>\r\n<Val>PassFailTest</Val>\r\n</String>\r\n<String>\r\n<Name> </Name>\r\n<Val>PassFailTest</Val>\r\n</String>\r\n<String>\r\n<Name> </Name>\r\n<Val>PassFailTest</Val>\r\n</String>\r\n<String>\r\n<Name> </Name>\r\n<Val>PassFailTest</Val>\r\n</String>\r\n<String>\r\n<Name> </Name>\r\n<Val>PassFailTest</Val>\r\n</String>\r\n<String>\r\n<Name> </Name>\r\n<Val>PassFailTest</Val>\r\n</String>\r\n<String>\r\n<Name> </Name>\r\n<Val>PassFailTest</Val>\r\n</String>\r\n<String>\r\n<Name> </Name>\r\n<Val>PassFailTest</Val>\r\n</String>\r\n<String>\r\n<Name> </Name>\r\n<Val>PassFailTest</Val>\r\n</String>\r\n<String>\r\n<Name> </Name>\r\n<Val>PassFailTest</Val>\r\n</String>\r\n<String>\r\n<Name> </Name>\r\n<Val>PassFailTest</Val>\r\n</String>\r\n<String>\r\n<Name> </Name>\r\n<Val>PassFailTest</Val>\r\n</String>\r\n<String>\r\n<Name> </Name>\r\n<Val>PassFailTest</Val>\r\n</String>\r\n<String>\r\n<Name> </Name>\r\n<Val>PassFailTest</Val>\r\n</String>\r\n<String>\r\n<Name> </Name>\r\n<Val>PassFailTest</Val>\r\n</String>\r\n<String>\r\n<Name> </Name>\r\n<Val>PassFailTest</Val>\r\n</String>\r\n<String>\r\n<Name> </Name>\r\n<Val>PassFailTest</Val>\r\n</String>\r\n<String>\r\n<Name> </Name>\r\n<Val>PassFailTest</Val>\r\n</String>\r\n<String>\r\n<Name> </Name>\r\n<Val>NumericLimitTest</Val>\r\n</String>\r\n<String>\r\n<Name> </Name>\r\n<Val>PassFailTest</Val>\r\n</String>\r\n<String>\r\n<Name> </Name>\r\n<Val>PassFailTest</Val>\r\n</String>\r\n<String>\r\n<Name> </Name>\r\n<Val>PassFailTest</Val>\r\n</String>\r\n<String>\r\n<Name> </Name>\r\n<Val>PassFailTest</Val>\r\n</String>\r\n<String>\r\n<Name> </Name>\r\n<Val>NumericLimitTest</Val>\r\n</String>\r\n<String>\r\n<Name> </Name>\r\n<Val>NumericLimitTest</Val>\r\n</String>\r\n<String>\r\n<Name> </Name>\r\n<Val>PassFailTest</Val>\r\n</String>\r\n<String>\r\n<Name> </Name>\r\n<Val>NumericLimitTest</Val>\r\n</String>\r\n<String>\r\n<Name> </Name>\r\n<Val>PassFailTest</Val>\r\n</String>\r\n<String>\r\n<Name> </Name>\r\n<Val>PassFailTest</Val>\r\n</String>\r\n<String>\r\n<Name> </Name>\r\n<Val>PassFailTest</Val>\r\n</String>\r\n<String>\r\n<Name> </Name>\r\n<Val>PassFailTest</Val>\r\n</String>\r\n<String>\r\n<Name> </Name>\r\n<Val>PassFailTest</Val>\r\n</String>\r\n<String>\r\n<Name> </Name>\r\n<Val>PassFailTest</Val>\r\n</String>\r\n<String>\r\n<Name> </Name>\r\n<Val>PassFailTest</Val>\r\n</String>\r\n<String>\r\n<Name> </Name>\r\n<Val>PassFailTest</Val>\r\n</String>\r\n<String>\r\n<Name> </Name>\r\n<Val>PassFailTest</Val>\r\n</String>\r\n<String>\r\n<Name> </Name>\r\n<Val>PassFailTest</Val>\r\n</String>\r\n<String>\r\n<Name> </Name>\r\n<Val>PassFailTest</Val>\r\n</String>\r\n<String>\r\n<Name> </Name>\r\n<Val>PassFailTest</Val>\r\n</String>\r\n<String>\r\n<Name> </Name>\r\n<Val>PassFailTest</Val>\r\n</String>\r\n<String>\r\n<Name> </Name>\r\n<Val>PassFailTest</Val>\r\n</String>\r\n<String>\r\n<Name> </Name>\r\n<Val>PassFailTest</Val>\r\n</String>\r\n<String>\r\n<Name> </Name>\r\n<Val>PassFailTest</Val>\r\n</String>\r\n<String>\r\n<Name> </Name>\r\n<Val>PassFailTest</Val>\r\n</String>\r\n<String>\r\n<Name> </Name>\r\n<Val>PassFailTest</Val>\r\n</String>\r\n<String>\r\n<Name> </Name>\r\n<Val>PassFailTest</Val>\r\n</String>\r\n<String>\r\n<Name> </Name>\r\n<Val>PassFailTest</Val>\r\n</String>\r\n<String>\r\n<Name> </Name>\r\n<Val>PassFailTest</Val>\r\n</String>\r\n<String>\r\n<Name> </Name>\r\n<Val>PassFailTest</Val>\r\n</String>\r\n<String>\r\n<Name> </Name>\r\n<Val>PassFailTest</Val>\r\n</String>\r\n<String>\r\n<Name> </Name>\r\n<Val>PassFailTest</Val>\r\n</String>\r\n<String>\r\n<Name> </Name>\r\n<Val>PassFailTest</Val>\r\n</String>\r\n<String>\r\n<Name> </Name>\r\n<Val>StringValueTest</Val>\r\n</String>\r\n<String>\r\n<Name> </Name>\r\n<Val>PassFailTest</Val>\r\n</String>\r\n<String>\r\n<Name> </Name>\r\n<Val>PassFailTest</Val>\r\n</String>\r\n<String>\r\n<Name> </Name>\r\n<Val>PassFailTest</Val>\r\n</String>\r\n<String>\r\n<Name> </Name>\r\n<Val>PassFailTest</Val>\r\n</String>\r\n<String>\r\n<Name> </Name>\r\n<Val>PassFailTest</Val>\r\n</String>\r\n<String>\r\n<Name> </Name>\r\n<Val>PassFailTest</Val>\r\n</String>\r\n<String>\r\n<Name> </Name>\r\n<Val>PassFailTest</Val>\r\n</String>\r\n<String>\r\n<Name> </Name>\r\n<Val>PassFailTest</Val>\r\n</String>\r\n<String>\r\n<Name> </Name>\r\n<Val>PassFailTest</Val>\r\n</String>\r\n<String>\r\n<Name> </Name>\r\n<Val>PassFailTest</Val>\r\n</String>\r\n<String>\r\n<Name> </Name>\r\n<Val>PassFailTest</Val>\r\n</String>\r\n<String>\r\n<Name> </Name>\r\n<Val>PassFailTest</Val>\r\n</String>\r\n<String>\r\n<Name> </Name>\r\n<Val>PassFailTest</Val>\r\n</String>\r\n<String>\r\n<Name> </Name>\r\n<Val>PassFailTest</Val>\r\n</String>\r\n<String>\r\n<Name> </Name>\r\n<Val>PassFailTest</Val>\r\n</String>\r\n<String>\r\n<Name> </Name>\r\n<Val>PassFailTest</Val>\r\n</String>\r\n<String>\r\n<Name> </Name>\r\n<Val>PassFailTest</Val>\r\n</String>\r\n<String>\r\n<Name> </Name>\r\n<Val>PassFailTest</Val>\r\n</String>\r\n<String>\r\n<Name> </Name>\r\n<Val>NumericLimitTest</Val>\r\n</String>\r\n<String>\r\n<Name> </Name>\r\n<Val>PassFailTest</Val>\r\n</String>\r\n<String>\r\n<Name> </Name>\r\n<Val>PassFailTest</Val>\r\n</String>\r\n<String>\r\n<Name> </Name>\r\n<Val>PassFailTest</Val>\r\n</String>\r\n<String>\r\n<Name> </Name>\r\n<Val>PassFailTest</Val>\r\n</String>\r\n<String>\r\n<Name> </Name>\r\n<Val>PassFailTest</Val>\r\n</String>\r\n<String>\r\n<Name> </Name>\r\n<Val>PassFailTest</Val>\r\n</String>\r\n<String>\r\n<Name> </Name>\r\n<Val>PassFailTest</Val>\r\n</String>\r\n<String>\r\n<Name> </Name>\r\n<Val>PassFailTest</Val>\r\n</String>\r\n<String>\r\n<Name> </Name>\r\n<Val>PassFailTest</Val>\r\n</String>\r\n<String>\r\n<Name> </Name>\r\n<Val>PassFailTest</Val>\r\n</String>\r\n<String>\r\n<Name> </Name>\r\n<Val>PassFailTest</Val>\r\n</String>\r\n<String>\r\n<Name> </Name>\r\n<Val>PassFailTest</Val>\r\n</String>\r\n<String>\r\n<Name> </Name>\r\n<Val>PassFailTest</Val>\r\n</String>\r\n<String>\r\n<Name> </Name>\r\n<Val>PassFailTest</Val>\r\n</String>\r\n<String>\r\n<Name> </Name>\r\n<Val>PassFailTest</Val>\r\n</String>\r\n<String>\r\n<Name> </Name>\r\n<Val>PassFailTest</Val>\r\n</String>\r\n<String>\r\n<Name> </Name>\r\n<Val>PassFailTest</Val>\r\n</String>\r\n<String>\r\n<Name> </Name>\r\n<Val>PassFailTest</Val>\r\n</String>\r\n<String>\r\n<Name> </Name>\r\n<Val>PassFailTest</Val>\r\n</String>\r\n<String>\r\n<Name> </Name>\r\n<Val>PassFailTest</Val>\r\n</String>\r\n<String>\r\n<Name> </Name>\r\n<Val>PassFailTest</Val>\r\n</String>\r\n<String>\r\n<Name> </Name>\r\n<Val>PassFailTest</Val>\r\n</String>\r\n<String>\r\n<Name> </Name>\r\n<Val>PassFailTest</Val>\r\n</String>\r\n<String>\r\n<Name> </Name>\r\n<Val>PassFailTest</Val>\r\n</String>\r\n<String>\r\n<Name> </Name>\r\n<Val>PassFailTest</Val>\r\n</String>\r\n<String>\r\n<Name> </Name>\r\n<Val>PassFailTest</Val>\r\n</String>\r\n<String>\r\n<Name> </Name>\r\n<Val>PassFailTest</Val>\r\n</String>\r\n<String>\r\n<Name> </Name>\r\n<Val>PassFailTest</Val>\r\n</String>\r\n<String>\r\n<Name> </Name>\r\n<Val>PassFailTest</Val>\r\n</String>\r\n<String>\r\n<Name> </Name>\r\n<Val>PassFailTest</Val>\r\n</String>\r\n<String>\r\n<Name> </Name>\r\n<Val>PassFailTest</Val>\r\n</String>\r\n<String>\r\n<Name> </Name>\r\n<Val>PassFailTest</Val>\r\n</String>\r\n<String>\r\n<Name> </Name>\r\n<Val>PassFailTest</Val>\r\n</String>\r\n<String>\r\n<Name> </Name>\r\n<Val>PassFailTest</Val>\r\n</String>\r\n<String>\r\n<Name> </Name>\r\n<Val>PassFailTest</Val>\r\n</String>\r\n<String>\r\n<Name> </Name>\r\n<Val>PassFailTest</Val>\r\n</String>\r\n<String>\r\n<Name> </Name>\r\n<Val>PassFailTest</Val>\r\n</String>\r\n<String>\r\n<Name> </Name>\r\n<Val>PassFailTest</Val>\r\n</String>\r\n<String>\r\n<Name> </Name>\r\n<Val>PassFailTest</Val>\r\n</String>\r\n<String>\r\n<Name> </Name>\r\n<Val>PassFailTest</Val>\r\n</String>\r\n<String>\r\n<Name> </Name>\r\n<Val>PassFailTest</Val>\r\n</String>\r\n<String>\r\n<Name> </Name>\r\n<Val>PassFailTest</Val>\r\n</String>\r\n<String>\r\n<Name> </Name>\r\n<Val>PassFailTest</Val>\r\n</String>\r\n<String>\r\n<Name> </Name>\r\n<Val>PassFailTest</Val>\r\n</String>\r\n<String>\r\n<Name> </Name>\r\n<Val>PassFailTest</Val>\r\n</String>\r\n<String>\r\n<Name> </Name>\r\n<Val>PassFailTest</Val>\r\n</String>\r\n<String>\r\n<Name> </Name>\r\n<Val>PassFailTest</Val>\r\n</String>\r\n<String>\r\n<Name> </Name>\r\n<Val>PassFailTest</Val>\r\n</String>\r\n<String>\r\n<Name> </Name>\r\n<Val>PassFailTest</Val>\r\n</String>\r\n<String>\r\n<Name> </Name>\r\n<Val>PassFailTest</Val>\r\n</String>\r\n<String>\r\n<Name> </Name>\r\n<Val>PassFailTest</Val>\r\n</String>\r\n<String>\r\n<Name> </Name>\r\n<Val>PassFailTest</Val>\r\n</String>\r\n<String>\r\n<Name> </Name>\r\n<Val>PassFailTest</Val>\r\n</String>\r\n<String>\r\n<Name> </Name>\r\n<Val>PassFailTest</Val>\r\n</String>\r\n<String>\r\n<Name> </Name>\r\n<Val>PassFailTest</Val>\r\n</String>\r\n<String>\r\n<Name> </Name>\r\n<Val>PassFailTest</Val>\r\n</String>\r\n<String>\r\n<Name> </Name>\r\n<Val>PassFailTest</Val>\r\n</String>\r\n<String>\r\n<Name> </Name>\r\n<Val>PassFailTest</Val>\r\n</String>\r\n<String>\r\n<Name> </Name>\r\n<Val>PassFailTest</Val>\r\n</String>\r\n<String>\r\n<Name> </Name>\r\n<Val>PassFailTest</Val>\r\n</String>\r\n<String>\r\n<Name> </Name>\r\n<Val>PassFailTest</Val>\r\n</String>\r\n<String>\r\n<Name> </Name>\r\n<Val>PassFailTest</Val>\r\n</String>\r\n<String>\r\n<Name> </Name>\r\n<Val>PassFailTest</Val>\r\n</String>\r\n<String>\r\n<Name> </Name>\r\n<Val>PassFailTest</Val>\r\n</String>\r\n<String>\r\n<Name> </Name>\r\n<Val>PassFailTest</Val>\r\n</String>\r\n<String>\r\n<Name> </Name>\r\n<Val>PassFailTest</Val>\r\n</String>\r\n<String>\r\n<Name> </Name>\r\n<Val>PassFailTest</Val>\r\n</String>\r\n<String>\r\n<Name> </Name>\r\n<Val>PassFailTest</Val>\r\n</String>\r\n<String>\r\n<Name> </Name>\r\n<Val>PassFailTest</Val>\r\n</String>\r\n<String>\r\n<Name> </Name>\r\n<Val>PassFailTest</Val>\r\n</String>\r\n<String>\r\n<Name> </Name>\r\n<Val>PassFailTest</Val>\r\n</String>\r\n<String>\r\n<Name> </Name>\r\n<Val>PassFailTest</Val>\r\n</String>\r\n<String>\r\n<Name> </Name>\r\n<Val>PassFailTest</Val>\r\n</String>\r\n<String>\r\n<Name> </Name>\r\n<Val>PassFailTest</Val>\r\n</String>\r\n<String>\r\n<Name> </Name>\r\n<Val>PassFailTest</Val>\r\n</String>\r\n<String>\r\n<Name> </Name>\r\n<Val>PassFailTest</Val>\r\n</String>\r\n<String>\r\n<Name> </Name>\r\n<Val>PassFailTest</Val>\r\n</String>\r\n<String>\r\n<Name> </Name>\r\n<Val>PassFailTest</Val>\r\n</String>\r\n<String>\r\n<Name> </Name>\r\n<Val>PassFailTest</Val>\r\n</String>\r\n<String>\r\n<Name> </Name>\r\n<Val>PassFailTest</Val>\r\n</String>\r\n<String>\r\n<Name> </Name>\r\n<Val>PassFailTest</Val>\r\n</String>\r\n<String>\r\n<Name> </Name>\r\n<Val>PassFailTest</Val>\r\n</String>\r\n<String>\r\n<Name> </Name>\r\n<Val>PassFailTest</Val>\r\n</String>\r\n<String>\r\n<Name> </Name>\r\n<Val>PassFailTest</Val>\r\n</String>\r\n<String>\r\n<Name> </Name>\r\n<Val>PassFailTest</Val>\r\n</String>\r\n<String>\r\n<Name> </Name>\r\n<Val>PassFailTest</Val>\r\n</String>\r\n<String>\r\n<Name> </Name>\r\n<Val>PassFailTest</Val>\r\n</String>\r\n<String>\r\n<Name> </Name>\r\n<Val>PassFailTest</Val>\r\n</String>\r\n<String>\r\n<Name> </Name>\r\n<Val>PassFailTest</Val>\r\n</String>\r\n<String>\r\n<Name> </Name>\r\n<Val>PassFailTest</Val>\r\n</String>\r\n<String>\r\n<Name> </Name>\r\n<Val>PassFailTest</Val>\r\n</String>\r\n<String>\r\n<Name> </Name>\r\n<Val>PassFailTest</Val>\r\n</String>\r\n<String>\r\n<Name> </Name>\r\n<Val>PassFailTest</Val>\r\n</String>\r\n<String>\r\n<Name> </Name>\r\n<Val>PassFailTest</Val>\r\n</String>\r\n<String>\r\n<Name> </Name>\r\n<Val>PassFailTest</Val>\r\n</String>\r\n<String>\r\n<Name> </Name>\r\n<Val>PassFailTest</Val>\r\n</String>\r\n<String>\r\n<Name> </Name>\r\n<Val>PassFailTest</Val>\r\n</String>\r\n<String>\r\n<Name> </Name>\r\n<Val>PassFailTest</Val>\r\n</String>\r\n<String>\r\n<Name> </Name>\r\n<Val>PassFailTest</Val>\r\n</String>\r\n<String>\r\n<Name> </Name>\r\n<Val>PassFailTest</Val>\r\n</String>\r\n<String>\r\n<Name> </Name>\r\n<Val>PassFailTest</Val>\r\n</String>\r\n<String>\r\n<Name> </Name>\r\n<Val>PassFailTest</Val>\r\n</String>\r\n<String>\r\n<Name> </Name>\r\n<Val>PassFailTest</Val>\r\n</String>\r\n<String>\r\n<Name> </Name>\r\n<Val>PassFailTest</Val>\r\n</String>\r\n<String>\r\n<Name> </Name>\r\n<Val>PassFailTest</Val>\r\n</String>\r\n<String>\r\n<Name> </Name>\r\n<Val>PassFailTest</Val>\r\n</String>\r\n<String>\r\n<Name> </Name>\r\n<Val>PassFailTest</Val>\r\n</String>\r\n<String>\r\n<Name> </Name>\r\n<Val>PassFailTest</Val>\r\n</String>\r\n<String>\r\n<Name> </Name>\r\n<Val>PassFailTest</Val>\r\n</String>\r\n<String>\r\n<Name> </Name>\r\n<Val>PassFailTest</Val>\r\n</String>\r\n<String>\r\n<Name> </Name>\r\n<Val>PassFailTest</Val>\r\n</String>\r\n<String>\r\n<Name> </Name>\r\n<Val>PassFailTest</Val>\r\n</String>\r\n<String>\r\n<Name> </Name>\r\n<Val>PassFailTest</Val>\r\n</String>\r\n<String>\r\n<Name> </Name>\r\n<Val>PassFailTest</Val>\r\n</String>\r\n<String>\r\n<Name> </Name>\r\n<Val>PassFailTest</Val>\r\n</String>\r\n<String>\r\n<Name> </Name>\r\n<Val>PassFailTest</Val>\r\n</String>\r\n<String>\r\n<Name> </Name>\r\n<Val>PassFailTest</Val>\r\n</String>\r\n<String>\r\n<Name> </Name>\r\n<Val>PassFailTest</Val>\r\n</String>\r\n<String>\r\n<Name> </Name>\r\n<Val>PassFailTest</Val>\r\n</String>\r\n<String>\r\n<Name> </Name>\r\n<Val>PassFailTest</Val>\r\n</String>\r\n<String>\r\n<Name> </Name>\r\n<Val>PassFailTest</Val>\r\n</String>\r\n<String>\r\n<Name> </Name>\r\n<Val>PassFailTest</Val>\r\n</String>\r\n<String>\r\n<Name> </Name>\r\n<Val>PassFailTest</Val>\r\n</String>\r\n<String>\r\n<Name> </Name>\r\n<Val>PassFailTest</Val>\r\n</String>\r\n<String>\r\n<Name> </Name>\r\n<Val>PassFailTest</Val>\r\n</String>\r\n<String>\r\n<Name> </Name>\r\n<Val>PassFailTest</Val>\r\n</String>\r\n<String>\r\n<Name> </Name>\r\n<Val>PassFailTest</Val>\r\n</String>\r\n<String>\r\n<Name> </Name>\r\n<Val>PassFailTest</Val>\r\n</String>\r\n<String>\r\n<Name> </Name>\r\n<Val>PassFailTest</Val>\r\n</String>\r\n<String>\r\n<Name> </Name>\r\n<Val>PassFailTest</Val>\r\n</String>\r\n<String>\r\n<Name> </Name>\r\n<Val>PassFailTest</Val>\r\n</String>\r\n<String>\r\n<Name> </Name>\r\n<Val>NumericLimitTest</Val>\r\n</String>\r\n<String>\r\n<Name> </Name>\r\n<Val>PassFailTest</Val>\r\n</String>\r\n<String>\r\n<Name> </Name>\r\n<Val>PassFailTest</Val>\r\n</String>\r\n<String>\r\n<Name> </Name>\r\n<Val>PassFailTest</Val>\r\n</String>\r\n<String>\r\n<Name> </Name>\r\n<Val>PassFailTest</Val>\r\n</String>\r\n<String>\r\n<Name> </Name>\r\n<Val>PassFailTest</Val>\r\n</String>\r\n<String>\r\n<Name> </Name>\r\n<Val>PassFailTest</Val>\r\n</String>\r\n<String>\r\n<Name> </Name>\r\n<Val>NumericLimitTest</Val>\r\n</String>\r\n<String>\r\n<Name> </Name>\r\n<Val>PassFailTest</Val>\r\n</String>\r\n<String>\r\n<Name> </Name>\r\n<Val>PassFailTest</Val>\r\n</String>\r\n<String>\r\n<Name> </Name>\r\n<Val>PassFailTest</Val>\r\n</String>\r\n<String>\r\n<Name> </Name>\r\n<Val>PassFailTest</Val>\r\n</String>\r\n<String>\r\n<Name> </Name>\r\n<Val>NumericLimitTest</Val>\r\n</String>\r\n<String>\r\n<Name> </Name>\r\n<Val>PassFailTest</Val>\r\n</String>\r\n<String>\r\n<Name> </Name>\r\n<Val>PassFailTest</Val>\r\n</String>\r\n<String>\r\n<Name> </Name>\r\n<Val>PassFailTest</Val>\r\n</String>\r\n<String>\r\n<Name> </Name>\r\n<Val>PassFailTest</Val>\r\n</String>\r\n<String>\r\n<Name> </Name>\r\n<Val>PassFailTest</Val>\r\n</String>\r\n<String>\r\n<Name> </Name>\r\n<Val>PassFailTest</Val>\r\n</String>\r\n<String>\r\n<Name> </Name>\r\n<Val>NumericLimitTest</Val>\r\n</String>\r\n<String>\r\n<Name> </Name>\r\n<Val>PassFailTest</Val>\r\n</String>\r\n<String>\r\n<Name> </Name>\r\n<Val>PassFailTest</Val>\r\n</String>\r\n<String>\r\n<Name> </Name>\r\n<Val>PassFailTest</Val>\r\n</String>\r\n<String>\r\n<Name> </Name>\r\n<Val>PassFailTest</Val>\r\n</String>\r\n<String>\r\n<Name> </Name>\r\n<Val>NumericLimitTest</Val>\r\n</String>\r\n<String>\r\n<Name> </Name>\r\n<Val>PassFailTest</Val>\r\n</String>\r\n<String>\r\n<Name> </Name>\r\n<Val>PassFailTest</Val>\r\n</String>\r\n<String>\r\n<Name> </Name>\r\n<Val>PassFailTest</Val>\r\n</String>\r\n<String>\r\n<Name> </Name>\r\n<Val>PassFailTest</Val>\r\n</String>\r\n<String>\r\n<Name> </Name>\r\n<Val>PassFailTest</Val>\r\n</String>\r\n<String>\r\n<Name> </Name>\r\n<Val>PassFailTest</Val>\r\n</String>\r\n<String>\r\n<Name> </Name>\r\n<Val>NumericLimitTest</Val>\r\n</String>\r\n<String>\r\n<Name> </Name>\r\n<Val>PassFailTest</Val>\r\n</String>\r\n<String>\r\n<Name> </Name>\r\n<Val>PassFailTest</Val>\r\n</String>\r\n<String>\r\n<Name> </Name>\r\n<Val>PassFailTest</Val>\r\n</String>\r\n<String>\r\n<Name> </Name>\r\n<Val>PassFailTest</Val>\r\n</String>\r\n<String>\r\n<Name> </Name>\r\n<Val>NumericLimitTest</Val>\r\n</String>\r\n<String>\r\n<Name> </Name>\r\n<Val>PassFailTest</Val>\r\n</String>\r\n<String>\r\n<Name> </Name>\r\n<Val>PassFailTest</Val>\r\n</String>\r\n<String>\r\n<Name> </Name>\r\n<Val>PassFailTest</Val>\r\n</String>\r\n<String>\r\n<Name> </Name>\r\n<Val>PassFailTest</Val>\r\n</String>\r\n<String>\r\n<Name> </Name>\r\n<Val>PassFailTest</Val>\r\n</String>\r\n<String>\r\n<Name> </Name>\r\n<Val>PassFailTest</Val>\r\n</String>\r\n<String>\r\n<Name> </Name>\r\n<Val>NumericLimitTest</Val>\r\n</String>\r\n<String>\r\n<Name> </Name>\r\n<Val>PassFailTest</Val>\r\n</String>\r\n<String>\r\n<Name> </Name>\r\n<Val>PassFailTest</Val>\r\n</String>\r\n<String>\r\n<Name> </Name>\r\n<Val>PassFailTest</Val>\r\n</String>\r\n<String>\r\n<Name> </Name>\r\n<Val>PassFailTest</Val>\r\n</String>\r\n<String>\r\n<Name> </Name>\r\n<Val>PassFailTest</Val>\r\n</String>\r\n<String>\r\n<Name> </Name>\r\n<Val>PassFailTest</Val>\r\n</String>\r\n<String>\r\n<Name> </Name>\r\n<Val>NumericLimitTest</Val>\r\n</String>\r\n<String>\r\n<Name> </Name>\r\n<Val>PassFailTest</Val>\r\n</String>\r\n<String>\r\n<Name> </Name>\r\n<Val>PassFailTest</Val>\r\n</String>\r\n<String>\r\n<Name> </Name>\r\n<Val>PassFailTest</Val>\r\n</String>\r\n<String>\r\n<Name> </Name>\r\n<Val>PassFailTest</Val>\r\n</String>\r\n<String>\r\n<Name> </Name>\r\n<Val>PassFailTest</Val>\r\n</String>\r\n<String>\r\n<Name> </Name>\r\n<Val>PassFailTest</Val>\r\n</String>\r\n<String>\r\n<Name> </Name>\r\n<Val>NumericLimitTest</Val>\r\n</String>\r\n<String>\r\n<Name> </Name>\r\n<Val>PassFailTest</Val>\r\n</String>\r\n<String>\r\n<Name> </Name>\r\n<Val>PassFailTest</Val>\r\n</String>\r\n<String>\r\n<Name> </Name>\r\n<Val>PassFailTest</Val>\r\n</String>\r\n<String>\r\n<Name> </Name>\r\n<Val>PassFailTest</Val>\r\n</String>\r\n<String>\r\n<Name> </Name>\r\n<Val>NumericLimitTest</Val>\r\n</String>\r\n<String>\r\n<Name> </Name>\r\n<Val>PassFailTest</Val>\r\n</String>\r\n<String>\r\n<Name> </Name>\r\n<Val>PassFailTest</Val>\r\n</String>\r\n<String>\r\n<Name> </Name>\r\n<Val>PassFailTest</Val>\r\n</String>\r\n<String>\r\n<Name> </Name>\r\n<Val>PassFailTest</Val>\r\n</String>\r\n<String>\r\n<Name> </Name>\r\n<Val>PassFailTest</Val>\r\n</String>\r\n<String>\r\n<Name> </Name>\r\n<Val>PassFailTest</Val>\r\n</String>\r\n<String>\r\n<Name> </Name>\r\n<Val>NumericLimitTest</Val>\r\n</String>\r\n<String>\r\n<Name> </Name>\r\n<Val>PassFailTest</Val>\r\n</String>\r\n<String>\r\n<Name> </Name>\r\n<Val>PassFailTest</Val>\r\n</String>\r\n<String>\r\n<Name> </Name>\r\n<Val>PassFailTest</Val>\r\n</String>\r\n<String>\r\n<Name> </Name>\r\n<Val>PassFailTest</Val>\r\n</String>\r\n<String>\r\n<Name> </Name>\r\n<Val>NumericLimitTest</Val>\r\n</String>\r\n<String>\r\n<Name> </Name>\r\n<Val>PassFailTest</Val>\r\n</String>\r\n<String>\r\n<Name> </Name>\r\n<Val>PassFailTest</Val>\r\n</String>\r\n<String>\r\n<Name> </Name>\r\n<Val>PassFailTest</Val>\r\n</String>\r\n<String>\r\n<Name> </Name>\r\n<Val>PassFailTest</Val>\r\n</String>\r\n<String>\r\n<Name> </Name>\r\n<Val>PassFailTest</Val>\r\n</String>\r\n<String>\r\n<Name> </Name>\r\n<Val>PassFailTest</Val>\r\n</String>\r\n<String>\r\n<Name> </Name>\r\n<Val>NumericLimitTest</Val>\r\n</String>\r\n<String>\r\n<Name> </Name>\r\n<Val>PassFailTest</Val>\r\n</String>\r\n<String>\r\n<Name> </Name>\r\n<Val>PassFailTest</Val>\r\n</String>\r\n<String>\r\n<Name> </Name>\r\n<Val>PassFailTest</Val>\r\n</String>\r\n<String>\r\n<Name> </Name>\r\n<Val>PassFailTest</Val>\r\n</String>\r\n<String>\r\n<Name> </Name>\r\n<Val>NumericLimitTest</Val>\r\n</String>\r\n<String>\r\n<Name> </Name>\r\n<Val>PassFailTest</Val>\r\n</String>\r\n<String>\r\n<Name> </Name>\r\n<Val>PassFailTest</Val>\r\n</String>\r\n<String>\r\n<Name> </Name>\r\n<Val>PassFailTest</Val>\r\n</String>\r\n<String>\r\n<Name> </Name>\r\n<Val>PassFailTest</Val>\r\n</String>\r\n<String>\r\n<Name> </Name>\r\n<Val>PassFailTest</Val>\r\n</String>\r\n<String>\r\n<Name> </Name>\r\n<Val>PassFailTest</Val>\r\n</String>\r\n<String>\r\n<Name> </Name>\r\n<Val>NumericLimitTest</Val>\r\n</String>\r\n<String>\r\n<Name> </Name>\r\n<Val>PassFailTest</Val>\r\n</String>\r\n<String>\r\n<Name> </Name>\r\n<Val>PassFailTest</Val>\r\n</String>\r\n<String>\r\n<Name> </Name>\r\n<Val>PassFailTest</Val>\r\n</String>\r\n<String>\r\n<Name> </Name>\r\n<Val>PassFailTest</Val>\r\n</String>\r\n<String>\r\n<Name> </Name>\r\n<Val>PassFailTest</Val>\r\n</String>\r\n<String>\r\n<Name> </Name>\r\n<Val>PassFailTest</Val>\r\n</String>\r\n<String>\r\n<Name> </Name>\r\n<Val>NumericLimitTest</Val>\r\n</String>\r\n<String>\r\n<Name> </Name>\r\n<Val>PassFailTest</Val>\r\n</String>\r\n<String>\r\n<Name> </Name>\r\n<Val>PassFailTest</Val>\r\n</String>\r\n<String>\r\n<Name> </Name>\r\n<Val>PassFailTest</Val>\r\n</String>\r\n<String>\r\n<Name> </Name>\r\n<Val>PassFailTest</Val>\r\n</String>\r\n<String>\r\n<Name> </Name>\r\n<Val>PassFailTest</Val>\r\n</String>\r\n<String>\r\n<Name> </Name>\r\n<Val>PassFailTest</Val>\r\n</String>\r\n<String>\r\n<Name> </Name>\r\n<Val>NumericLimitTest</Val>\r\n</String>\r\n<String>\r\n<Name> </Name>\r\n<Val>PassFailTest</Val>\r\n</String>\r\n<String>\r\n<Name> </Name>\r\n<Val>PassFailTest</Val>\r\n</String>\r\n<String>\r\n<Name> </Name>\r\n<Val>PassFailTest</Val>\r\n</String>\r\n<String>\r\n<Name> </Name>\r\n<Val>PassFailTest</Val>\r\n</String>\r\n<String>\r\n<Name> </Name>\r\n<Val>NumericLimitTest</Val>\r\n</String>\r\n<String>\r\n<Name> </Name>\r\n<Val>PassFailTest</Val>\r\n</String>\r\n<String>\r\n<Name> </Name>\r\n<Val>PassFailTest</Val>\r\n</String>\r\n<String>\r\n<Name> </Name>\r\n<Val>PassFailTest</Val>\r\n</String>\r\n<String>\r\n<Name> </Name>\r\n<Val>PassFailTest</Val>\r\n</String>\r\n<String>\r\n<Name> </Name>\r\n<Val>PassFailTest</Val>\r\n</String>\r\n<String>\r\n<Name> </Name>\r\n<Val>PassFailTest</Val>\r\n</String>\r\n<String>\r\n<Name> </Name>\r\n<Val>NumericLimitTest</Val>\r\n</String>\r\n<String>\r\n<Name> </Name>\r\n<Val>PassFailTest</Val>\r\n</String>\r\n<String>\r\n<Name> </Name>\r\n<Val>PassFailTest</Val>\r\n</String>\r\n<String>\r\n<Name> </Name>\r\n<Val>PassFailTest</Val>\r\n</String>\r\n<String>\r\n<Name> </Name>\r\n<Val>PassFailTest</Val>\r\n</String>\r\n<String>\r\n<Name> </Name>\r\n<Val>NumericLimitTest</Val>\r\n</String>\r\n<String>\r\n<Name> </Name>\r\n<Val>PassFailTest</Val>\r\n</String>\r\n<String>\r\n<Name> </Name>\r\n<Val>PassFailTest</Val>\r\n</String>\r\n<String>\r\n<Name> </Name>\r\n<Val>PassFailTest</Val>\r\n</String>\r\n<String>\r\n<Name> </Name>\r\n<Val>PassFailTest</Val>\r\n</String>\r\n<String>\r\n<Name> </Name>\r\n<Val>PassFailTest</Val>\r\n</String>\r\n<String>\r\n<Name> </Name>\r\n<Val>PassFailTest</Val>\r\n</String>\r\n<String>\r\n<Name> </Name>\r\n<Val>NumericLimitTest</Val>\r\n</String>\r\n<String>\r\n<Name> </Name>\r\n<Val>PassFailTest</Val>\r\n</String>\r\n<String>\r\n<Name> </Name>\r\n<Val>PassFailTest</Val>\r\n</String>\r\n<String>\r\n<Name> </Name>\r\n<Val>PassFailTest</Val>\r\n</String>\r\n<String>\r\n<Name> </Name>\r\n<Val>PassFailTest</Val>\r\n</String>\r\n<String>\r\n<Name> </Name>\r\n<Val>NumericLimitTest</Val>\r\n</String>\r\n<String>\r\n<Name> </Name>\r\n<Val>PassFailTest</Val>\r\n</String>\r\n<String>\r\n<Name> </Name>\r\n<Val>PassFailTest</Val>\r\n</String>\r\n<String>\r\n<Name> </Name>\r\n<Val>PassFailTest</Val>\r\n</String>\r\n<String>\r\n<Name> </Name>\r\n<Val>PassFailTest</Val>\r\n</String>\r\n<String>\r\n<Name> </Name>\r\n<Val>PassFailTest</Val>\r\n</String>\r\n<String>\r\n<Name> </Name>\r\n<Val>PassFailTest</Val>\r\n</String>\r\n<String>\r\n<Name> </Name>\r\n<Val>NumericLimitTest</Val>\r\n</String>\r\n<String>\r\n<Name> </Name>\r\n<Val>PassFailTest</Val>\r\n</String>\r\n<String>\r\n<Name> </Name>\r\n<Val>PassFailTest</Val>\r\n</String>\r\n<String>\r\n<Name> </Name>\r\n<Val>PassFailTest</Val>\r\n</String>\r\n<String>\r\n<Name> </Name>\r\n<Val>PassFailTest</Val>\r\n</String>\r\n<String>\r\n<Name> </Name>\r\n<Val>PassFailTest</Val>\r\n</String>\r\n<String>\r\n<Name> </Name>\r\n<Val>PassFailTest</Val>\r\n</String>\r\n<String>\r\n<Name> </Name>\r\n<Val>NumericLimitTest</Val>\r\n</String>\r\n<String>\r\n<Name> </Name>\r\n<Val>PassFailTest</Val>\r\n</String>\r\n<String>\r\n<Name> </Name>\r\n<Val>PassFailTest</Val>\r\n</String>\r\n<String>\r\n<Name> </Name>\r\n<Val>PassFailTest</Val>\r\n</String>\r\n<String>\r\n<Name> </Name>\r\n<Val>PassFailTest</Val>\r\n</String>\r\n<String>\r\n<Name> </Name>\r\n<Val>PassFailTest</Val>\r\n</String>\r\n<String>\r\n<Name> </Name>\r\n<Val>PassFailTest</Val>\r\n</String>\r\n<String>\r\n<Name> </Name>\r\n<Val>NumericLimitTest</Val>\r\n</String>\r\n<String>\r\n<Name> </Name>\r\n<Val>PassFailTest</Val>\r\n</String>\r\n<String>\r\n<Name> </Name>\r\n<Val>PassFailTest</Val>\r\n</String>\r\n<String>\r\n<Name> </Name>\r\n<Val>PassFailTest</Val>\r\n</String>\r\n<String>\r\n<Name> </Name>\r\n<Val>PassFailTest</Val>\r\n</String>\r\n<String>\r\n<Name> </Name>\r\n<Val>NumericLimitTest</Val>\r\n</String>\r\n<String>\r\n<Name> </Name>\r\n<Val>PassFailTest</Val>\r\n</String>\r\n<String>\r\n<Name> </Name>\r\n<Val>PassFailTest</Val>\r\n</String>\r\n<String>\r\n<Name> </Name>\r\n<Val>PassFailTest</Val>\r\n</String>\r\n<String>\r\n<Name> </Name>\r\n<Val>PassFailTest</Val>\r\n</String>\r\n<String>\r\n<Name> </Name>\r\n<Val>PassFailTest</Val>\r\n</String>\r\n<String>\r\n<Name> </Name>\r\n<Val>PassFailTest</Val>\r\n</String>\r\n<String>\r\n<Name> </Name>\r\n<Val>NumericLimitTest</Val>\r\n</String>\r\n<String>\r\n<Name> </Name>\r\n<Val>PassFailTest</Val>\r\n</String>\r\n<String>\r\n<Name> </Name>\r\n<Val>PassFailTest</Val>\r\n</String>\r\n<String>\r\n<Name> </Name>\r\n<Val>PassFailTest</Val>\r\n</String>\r\n<String>\r\n<Name> </Name>\r\n<Val>PassFailTest</Val>\r\n</String>\r\n<String>\r\n<Name> </Name>\r\n<Val>NumericLimitTest</Val>\r\n</String>\r\n<String>\r\n<Name> </Name>\r\n<Val>PassFailTest</Val>\r\n</String>\r\n<String>\r\n<Name> </Name>\r\n<Val>PassFailTest</Val>\r\n</String>\r\n<String>\r\n<Name> </Name>\r\n<Val>PassFailTest</Val>\r\n</String>\r\n<String>\r\n<Name> </Name>\r\n<Val>PassFailTest</Val>\r\n</String>\r\n<String>\r\n<Name> </Name>\r\n<Val>PassFailTest</Val>\r\n</String>\r\n<String>\r\n<Name> </Name>\r\n<Val>PassFailTest</Val>\r\n</String>\r\n<String>\r\n<Name> </Name>\r\n<Val>NumericLimitTest</Val>\r\n</String>\r\n<String>\r\n<Name> </Name>\r\n<Val>PassFailTest</Val>\r\n</String>\r\n<String>\r\n<Name> </Name>\r\n<Val>PassFailTest</Val>\r\n</String>\r\n<String>\r\n<Name> </Name>\r\n<Val>PassFailTest</Val>\r\n</String>\r\n<String>\r\n<Name> </Name>\r\n<Val>PassFailTest</Val>\r\n</String>\r\n<String>\r\n<Name> </Name>\r\n<Val>NumericLimitTest</Val>\r\n</String>\r\n<String>\r\n<Name> </Name>\r\n<Val>PassFailTest</Val>\r\n</String>\r\n<String>\r\n<Name> </Name>\r\n<Val>PassFailTest</Val>\r\n</String>\r\n<String>\r\n<Name> </Name>\r\n<Val>PassFailTest</Val>\r\n</String>\r\n<String>\r\n<Name> </Name>\r\n<Val>PassFailTest</Val>\r\n</String>\r\n<String>\r\n<Name> </Name>\r\n<Val>PassFailTest</Val>\r\n</String>\r\n<String>\r\n<Name> </Name>\r\n<Val>PassFailTest</Val>\r\n</String>\r\n<String>\r\n<Name> </Name>\r\n<Val>NumericLimitTest</Val>\r\n</String>\r\n<String>\r\n<Name> </Name>\r\n<Val>PassFailTest</Val>\r\n</String>\r\n<String>\r\n<Name> </Name>\r\n<Val>PassFailTest</Val>\r\n</String>\r\n<String>\r\n<Name> </Name>\r\n<Val>PassFailTest</Val>\r\n</String>\r\n<String>\r\n<Name> </Name>\r\n<Val>PassFailTest</Val>\r\n</String>\r\n<String>\r\n<Name> </Name>\r\n<Val>PassFailTest</Val>\r\n</String>\r\n<String>\r\n<Name> </Name>\r\n<Val>PassFailTest</Val>\r\n</String>\r\n<String>\r\n<Name> </Name>\r\n<Val>PassFailTest</Val>\r\n</String>\r\n<String>\r\n<Name> </Name>\r\n<Val>PassFailTest</Val>\r\n</String>\r\n<String>\r\n<Name> </Name>\r\n<Val>PassFailTest</Val>\r\n</String>\r\n<String>\r\n<Name> </Name>\r\n<Val>PassFailTest</Val>\r\n</String>\r\n<String>\r\n<Name> </Name>\r\n<Val>PassFailTest</Val>\r\n</String>\r\n<String>\r\n<Name> </Name>\r\n<Val>PassFailTest</Val>\r\n</String>\r\n<String>\r\n<Name> </Name>\r\n<Val>PassFailTest</Val>\r\n</String>\r\n<String>\r\n<Name> </Name>\r\n<Val>PassFailTest</Val>\r\n</String>\r\n<String>\r\n<Name> </Name>\r\n<Val>PassFailTest</Val>\r\n</String>\r\n<String>\r\n<Name> </Name>\r\n<Val>PassFailTest</Val>\r\n</String>\r\n<String>\r\n<Name> </Name>\r\n<Val>PassFailTest</Val>\r\n</String>\r\n<String>\r\n<Name> </Name>\r\n<Val>PassFailTest</Val>\r\n</String>\r\n<String>\r\n<Name> </Name>\r\n<Val>PassFailTest</Val>\r\n</String>\r\n<String>\r\n<Name> </Name>\r\n<Val>PassFailTest</Val>\r\n</String>\r\n<String>\r\n<Name> </Name>\r\n<Val>PassFailTest</Val>\r\n</String>\r\n<String>\r\n<Name> </Name>\r\n<Val>PassFailTest</Val>\r\n</String>\r\n<String>\r\n<Name> </Name>\r\n<Val>PassFailTest</Val>\r\n</String>\r\n<String>\r\n<Name> </Name>\r\n<Val>PassFailTest</Val>\r\n</String>\r\n<String>\r\n<Name> </Name>\r\n<Val>PassFailTest</Val>\r\n</String>\r\n<String>\r\n<Name> </Name>\r\n<Val>PassFailTest</Val>\r\n</String>\r\n<String>\r\n<Name> </Name>\r\n<Val>PassFailTest</Val>\r\n</String>\r\n<String>\r\n<Name> </Name>\r\n<Val>PassFailTest</Val>\r\n</String>\r\n<String>\r\n<Name> </Name>\r\n<Val>PassFailTest</Val>\r\n</String>\r\n<String>\r\n<Name> </Name>\r\n<Val>PassFailTest</Val>\r\n</String>\r\n<String>\r\n<Name> </Name>\r\n<Val>PassFailTest</Val>\r\n</String>\r\n<String>\r\n<Name> </Name>\r\n<Val>PassFailTest</Val>\r\n</String>\r\n<String>\r\n<Name> </Name>\r\n<Val>PassFailTest</Val>\r\n</String>\r\n<String>\r\n<Name> </Name>\r\n<Val>PassFailTest</Val>\r\n</String>\r\n<String>\r\n<Name> </Name>\r\n<Val>PassFailTest</Val>\r\n</String>\r\n<String>\r\n<Name> </Name>\r\n<Val>PassFailTest</Val>\r\n</String>\r\n<String>\r\n<Name> </Name>\r\n<Val>PassFailTest</Val>\r\n</String>\r\n<String>\r\n<Name> </Name>\r\n<Val>PassFailTest</Val>\r\n</String>\r\n<String>\r\n<Name> </Name>\r\n<Val>PassFailTest</Val>\r\n</String>\r\n<String>\r\n<Name> </Name>\r\n<Val>PassFailTest</Val>\r\n</String>\r\n<String>\r\n<Name> </Name>\r\n<Val>PassFailTest</Val>\r\n</String>\r\n<String>\r\n<Name> </Name>\r\n<Val>PassFailTest</Val>\r\n</String>\r\n<String>\r\n<Name> </Name>\r\n<Val>PassFailTest</Val>\r\n</String>\r\n<String>\r\n<Name> </Name>\r\n<Val>PassFailTest</Val>\r\n</String>\r\n<String>\r\n<Name> </Name>\r\n<Val>PassFailTest</Val>\r\n</String>\r\n<String>\r\n<Name> </Name>\r\n<Val>PassFailTest</Val>\r\n</String>\r\n<String>\r\n<Name> </Name>\r\n<Val>PassFailTest</Val>\r\n</String>\r\n<String>\r\n<Name> </Name>\r\n<Val>PassFailTest</Val>\r\n</String>\r\n<String>\r\n<Name> </Name>\r\n<Val>PassFailTest</Val>\r\n</String>\r\n<String>\r\n<Name> </Name>\r\n<Val>PassFailTest</Val>\r\n</String>\r\n<String>\r\n<Name> </Name>\r\n<Val>PassFailTest</Val>\r\n</String>\r\n<String>\r\n<Name> </Name>\r\n<Val>PassFailTest</Val>\r\n</String>\r\n<String>\r\n<Name> </Name>\r\n<Val>PassFailTest</Val>\r\n</String>\r\n<String>\r\n<Name> </Name>\r\n<Val>PassFailTest</Val>\r\n</String>\r\n<String>\r\n<Name> </Name>\r\n<Val>PassFailTest</Val>\r\n</String>\r\n<String>\r\n<Name> </Name>\r\n<Val>PassFailTest</Val>\r\n</String>\r\n<String>\r\n<Name> </Name>\r\n<Val>PassFailTest</Val>\r\n</String>\r\n<String>\r\n<Name> </Name>\r\n<Val>PassFailTest</Val>\r\n</String>\r\n<String>\r\n<Name> </Name>\r\n<Val>PassFailTest</Val>\r\n</String>\r\n<String>\r\n<Name> </Name>\r\n<Val>PassFailTest</Val>\r\n</String>\r\n<String>\r\n<Name> </Name>\r\n<Val>PassFailTest</Val>\r\n</String>\r\n<String>\r\n<Name> </Name>\r\n<Val>PassFailTest</Val>\r\n</String>\r\n<String>\r\n<Name> </Name>\r\n<Val>PassFailTest</Val>\r\n</String>\r\n<String>\r\n<Name> </Name>\r\n<Val>PassFailTest</Val>\r\n</String>\r\n<String>\r\n<Name> </Name>\r\n<Val>PassFailTest</Val>\r\n</String>\r\n<String>\r\n<Name> </Name>\r\n<Val>PassFailTest</Val>\r\n</String>\r\n<String>\r\n<Name> </Name>\r\n<Val>PassFailTest</Val>\r\n</String>\r\n<String>\r\n<Name> </Name>\r\n<Val>PassFailTest</Val>\r\n</String>\r\n<String>\r\n<Name> </Name>\r\n<Val>PassFailTest</Val>\r\n</String>\r\n<String>\r\n<Name> </Name>\r\n<Val>PassFailTest</Val>\r\n</String>\r\n<String>\r\n<Name> </Name>\r\n<Val>PassFailTest</Val>\r\n</String>\r\n<String>\r\n<Name> </Name>\r\n<Val>PassFailTest</Val>\r\n</String>\r\n<String>\r\n<Name> </Name>\r\n<Val>PassFailTest</Val>\r\n</String>\r\n<String>\r\n<Name> </Name>\r\n<Val>PassFailTest</Val>\r\n</String>\r\n<String>\r\n<Name> </Name>\r\n<Val>PassFailTest</Val>\r\n</String>\r\n<String>\r\n<Name> </Name>\r\n<Val>PassFailTest</Val>\r\n</String>\r\n<String>\r\n<Name> </Name>\r\n<Val>PassFailTest</Val>\r\n</String>\r\n<String>\r\n<Name> </Name>\r\n<Val>PassFailTest</Val>\r\n</String>\r\n<String>\r\n<Name> </Name>\r\n<Val>PassFailTest</Val>\r\n</String>\r\n<String>\r\n<Name> </Name>\r\n<Val>PassFailTest</Val>\r\n</String>\r\n<String>\r\n<Name> </Name>\r\n<Val>PassFailTest</Val>\r\n</String>\r\n<String>\r\n<Name> </Name>\r\n<Val>PassFailTest</Val>\r\n</String>\r\n<String>\r\n<Name> </Name>\r\n<Val>PassFailTest</Val>\r\n</String>\r\n<String>\r\n<Name> </Name>\r\n<Val>PassFailTest</Val>\r\n</String>\r\n<String>\r\n<Name> </Name>\r\n<Val>PassFailTest</Val>\r\n</String>\r\n<String>\r\n<Name> </Name>\r\n<Val>PassFailTest</Val>\r\n</String>\r\n<String>\r\n<Name> </Name>\r\n<Val>PassFailTest</Val>\r\n</String>\r\n<String>\r\n<Name> </Name>\r\n<Val>PassFailTest</Val>\r\n</String>\r\n<String>\r\n<Name> </Name>\r\n<Val>PassFailTest</Val>\r\n</String>\r\n<String>\r\n<Name> </Name>\r\n<Val>PassFailTest</Val>\r\n</String>\r\n<String>\r\n<Name> </Name>\r\n<Val>PassFailTest</Val>\r\n</String>\r\n<String>\r\n<Name> </Name>\r\n<Val>PassFailTest</Val>\r\n</String>\r\n<String>\r\n<Name> </Name>\r\n<Val>PassFailTest</Val>\r\n</String>\r\n<String>\r\n<Name> </Name>\r\n<Val>PassFailTest</Val>\r\n</String>\r\n<String>\r\n<Name> </Name>\r\n<Val></Val>\r\n</String>\r\n<String>\r\n<Name> </Name>\r\n<Val></Val>\r\n</String>\r\n<String>\r\n<Name> </Name>\r\n<Val></Val>\r\n</String>\r\n<String>\r\n<Name> </Name>\r\n<Val></Val>\r\n</String>\r\n<String>\r\n<Name> </Name>\r\n<Val></Val>\r\n</String>\r\n<String>\r\n<Name> </Name>\r\n<Val></Val>\r\n</String>\r\n<String>\r\n<Name> </Name>\r\n<Val></Val>\r\n</String>\r\n<String>\r\n<Name> </Name>\r\n<Val></Val>\r\n</String>\r\n<String>\r\n<Name> </Name>\r\n<Val></Val>\r\n</String>\r\n<String>\r\n<Name> </Name>\r\n<Val></Val>\r\n</String>\r\n<String>\r\n<Name> </Name>\r\n<Val></Val>\r\n</String>\r\n<String>\r\n<Name> </Name>\r\n<Val></Val>\r\n</String>\r\n<String>\r\n<Name> </Name>\r\n<Val></Val>\r\n</String>\r\n<String>\r\n<Name> </Name>\r\n<Val></Val>\r\n</String>\r\n<String>\r\n<Name> </Name>\r\n<Val></Val>\r\n</String>\r\n<String>\r\n<Name> </Name>\r\n<Val></Val>\r\n</String>\r\n<String>\r\n<Name> </Name>\r\n<Val></Val>\r\n</String>\r\n<String>\r\n<Name> </Name>\r\n<Val></Val>\r\n</String>\r\n<String>\r\n<Name> </Name>\r\n<Val></Val>\r\n</String>\r\n<String>\r\n<Name> </Name>\r\n<Val></Val>\r\n</String>\r\n<String>\r\n<Name> </Name>\r\n<Val>1.301493</Val>\r\n</String>\r\n<String>\r\n<Name> </Name>\r\n<Val></Val>\r\n</String>\r\n<String>\r\n<Name> </Name>\r\n<Val></Val>\r\n</String>\r\n<String>\r\n<Name> </Name>\r\n<Val></Val>\r\n</String>\r\n<String>\r\n<Name> </Name>\r\n<Val></Val>\r\n</String>\r\n<String>\r\n<Name> </Name>\r\n<Val>48.056165</Val>\r\n</String>\r\n<String>\r\n<Name> </Name>\r\n<Val>0.97</Val>\r\n</String>\r\n<String>\r\n<Name> </Name>\r\n<Val></Val>\r\n</String>\r\n<String>\r\n<Name> </Name>\r\n<Val>3.3032722</Val>\r\n</String>\r\n<String>\r\n<Name> </Name>\r\n<Val></Val>\r\n</String>\r\n<String>\r\n<Name> </Name>\r\n<Val></Val>\r\n</String>\r\n<String>\r\n<Name> </Name>\r\n<Val></Val>\r\n</String>\r\n<String>\r\n<Name> </Name>\r\n<Val></Val>\r\n</String>\r\n<String>\r\n<Name> </Name>\r\n<Val></Val>\r\n</String>\r\n<String>\r\n<Name> </Name>\r\n<Val></Val>\r\n</String>\r\n<String>\r\n<Name> </Name>\r\n<Val></Val>\r\n</String>\r\n<String>\r\n<Name> </Name>\r\n<Val></Val>\r\n</String>\r\n<String>\r\n<Name> </Name>\r\n<Val></Val>\r\n</String>\r\n<String>\r\n<Name> </Name>\r\n<Val></Val>\r\n</String>\r\n<String>\r\n<Name> </Name>\r\n<Val></Val>\r\n</String>\r\n<String>\r\n<Name> </Name>\r\n<Val></Val>\r\n</String>\r\n<String>\r\n<Name> </Name>\r\n<Val></Val>\r\n</String>\r\n<String>\r\n<Name> </Name>\r\n<Val></Val>\r\n</String>\r\n<String>\r\n<Name> </Name>\r\n<Val></Val>\r\n</String>\r\n<String>\r\n<Name> </Name>\r\n<Val></Val>\r\n</String>\r\n<String>\r\n<Name> </Name>\r\n<Val></Val>\r\n</String>\r\n<String>\r\n<Name> </Name>\r\n<Val></Val>\r\n</String>\r\n<String>\r\n<Name> </Name>\r\n<Val></Val>\r\n</String>\r\n<String>\r\n<Name> </Name>\r\n<Val></Val>\r\n</String>\r\n<String>\r\n<Name> </Name>\r\n<Val></Val>\r\n</String>\r\n<String>\r\n<Name> </Name>\r\n<Val></Val>\r\n</String>\r\n<String>\r\n<Name> </Name>\r\n<Val></Val>\r\n</String>\r\n<String>\r\n<Name> </Name>\r\n<Val></Val>\r\n</String>\r\n<String>\r\n<Name> </Name>\r\n<Val></Val>\r\n</String>\r\n<String>\r\n<Name> </Name>\r\n<Val>promHeader            : Sycamore Eeprom\n\r\rpromSize              : 0x80\n\r\rpromVersion           : 0x8\n\r\rserialNumber          : N635017050\n\r\rproductCode           : 910244\n\r\rissueNumber           : AB\n\r\rProduct ID            : 910244-AB\n\r\rCLEICode              : SOC2G33BAA\n\r\rmacAddress            :  \n\r\rcardType              : 0x9e\n\r\r850-Level Part Number : 8500052410E\n\r\rBOM revision          : 0L1\n\r\rChecksum              : 0x8981\n\r\rxpostFlag             : 0x 0\rxpostFailCode         : 0x 0</Val>\r\n</String>\r\n<String>\r\n<Name> </Name>\r\n<Val></Val>\r\n</String>\r\n<String>\r\n<Name> </Name>\r\n<Val></Val>\r\n</String>\r\n<String>\r\n<Name> </Name>\r\n<Val></Val>\r\n</String>\r\n<String>\r\n<Name> </Name>\r\n<Val></Val>\r\n</String>\r\n<String>\r\n<Name> </Name>\r\n<Val></Val>\r\n</String>\r\n<String>\r\n<Name> </Name>\r\n<Val></Val>\r\n</String>\r\n<String>\r\n<Name> </Name>\r\n<Val></Val>\r\n</String>\r\n<String>\r\n<Name> </Name>\r\n<Val></Val>\r\n</String>\r\n<String>\r\n<Name> </Name>\r\n<Val></Val>\r\n</String>\r\n<String>\r\n<Name> </Name>\r\n<Val></Val>\r\n</String>\r\n<String>\r\n<Name> </Name>\r\n<Val></Val>\r\n</String>\r\n<String>\r\n<Name> </Name>\r\n<Val></Val>\r\n</String>\r\n<String>\r\n<Name> </Name>\r\n<Val></Val>\r\n</String>\r\n<String>\r\n<Name> </Name>\r\n<Val></Val>\r\n</String>\r\n<String>\r\n<Name> </Name>\r\n<Val></Val>\r\n</String>\r\n<String>\r\n<Name> </Name>\r\n<Val></Val>\r\n</String>\r\n<String>\r\n<Name> </Name>\r\n<Val></Val>\r\n</String>\r\n<String>\r\n<Name> </Name>\r\n<Val></Val>\r\n</String>\r\n<String>\r\n<Name> </Name>\r\n<Val>30</Val>\r\n</String>\r\n<String>\r\n<Name> </Name>\r\n<Val></Val>\r\n</String>\r\n<String>\r\n<Name> </Name>\r\n<Val></Val>\r\n</String>\r\n<String>\r\n<Name> </Name>\r\n<Val></Val>\r\n</String>\r\n<String>\r\n<Name> </Name>\r\n<Val></Val>\r\n</String>\r\n<String>\r\n<Name> </Name>\r\n<Val></Val>\r\n</String>\r\n<String>\r\n<Name> </Name>\r\n<Val></Val>\r\n</String>\r\n<String>\r\n<Name> </Name>\r\n<Val></Val>\r\n</String>\r\n<String>\r\n<Name> </Name>\r\n<Val></Val>\r\n</String>\r\n<String>\r\n<Name> </Name>\r\n<Val></Val>\r\n</String>\r\n<String>\r\n<Name> </Name>\r\n<Val></Val>\r\n</String>\r\n<String>\r\n<Name> </Name>\r\n<Val></Val>\r\n</String>\r\n<String>\r\n<Name> </Name>\r\n<Val></Val>\r\n</String>\r\n<String>\r\n<Name> </Name>\r\n<Val></Val>\r\n</String>\r\n<String>\r\n<Name> </Name>\r\n<Val></Val>\r\n</String>\r\n<String>\r\n<Name> </Name>\r\n<Val></Val>\r\n</String>\r\n<String>\r\n<Name> </Name>\r\n<Val></Val>\r\n</String>\r\n<String>\r\n<Name> </Name>\r\n<Val></Val>\r\n</String>\r\n<String>\r\n<Name> </Name>\r\n<Val></Val>\r\n</String>\r\n<String>\r\n<Name> </Name>\r\n<Val></Val>\r\n</String>\r\n<String>\r\n<Name> </Name>\r\n<Val></Val>\r\n</String>\r\n<String>\r\n<Name> </Name>\r\n<Val></Val>\r\n</String>\r\n<String>\r\n<Name> </Name>\r\n<Val></Val>\r\n</String>\r\n<String>\r\n<Name> </Name>\r\n<Val></Val>\r\n</String>\r\n<String>\r\n<Name> </Name>\r\n<Val></Val>\r\n</String>\r\n<String>\r\n<Name> </Name>\r\n<Val></Val>\r\n</String>\r\n<String>\r\n<Name> </Name>\r\n<Val></Val>\r\n</String>\r\n<String>\r\n<Name> </Name>\r\n<Val></Val>\r\n</String>\r\n<String>\r\n<Name> </Name>\r\n<Val></Val>\r\n</String>\r\n<String>\r\n<Name> </Name>\r\n<Val></Val>\r\n</String>\r\n<String>\r\n<Name> </Name>\r\n<Val></Val>\r\n</String>\r\n<String>\r\n<Name> </Name>\r\n<Val></Val>\r\n</String>\r\n<String>\r\n<Name> </Name>\r\n<Val></Val>\r\n</String>\r\n<String>\r\n<Name> </Name>\r\n<Val></Val>\r\n</String>\r\n<String>\r\n<Name> </Name>\r\n<Val></Val>\r\n</String>\r\n<String>\r\n<Name> </Name>\r\n<Val></Val>\r\n</String>\r\n<String>\r\n<Name> </Name>\r\n<Val></Val>\r\n</String>\r\n<String>\r\n<Name> </Name>\r\n<Val></Val>\r\n</String>\r\n<String>\r\n<Name> </Name>\r\n<Val></Val>\r\n</String>\r\n<String>\r\n<Name> </Name>\r\n<Val></Val>\r\n</String>\r\n<String>\r\n<Name> </Name>\r\n<Val></Val>\r\n</String>\r\n<String>\r\n<Name> </Name>\r\n<Val></Val>\r\n</String>\r\n<String>\r\n<Name> </Name>\r\n<Val></Val>\r\n</String>\r\n<String>\r\n<Name> </Name>\r\n<Val></Val>\r\n</String>\r\n<String>\r\n<Name> </Name>\r\n<Val></Val>\r\n</String>\r\n<String>\r\n<Name> </Name>\r\n<Val></Val>\r\n</String>\r\n<String>\r\n<Name> </Name>\r\n<Val></Val>\r\n</String>\r\n<String>\r\n<Name> </Name>\r\n<Val></Val>\r\n</String>\r\n<String>\r\n<Name> </Name>\r\n<Val></Val>\r\n</String>\r\n<String>\r\n<Name> </Name>\r\n<Val></Val>\r\n</String>\r\n<String>\r\n<Name> </Name>\r\n<Val></Val>\r\n</String>\r\n<String>\r\n<Name> </Name>\r\n<Val></Val>\r\n</String>\r\n<String>\r\n<Name> </Name>\r\n<Val></Val>\r\n</String>\r\n<String>\r\n<Name> </Name>\r\n<Val></Val>\r\n</String>\r\n<String>\r\n<Name> </Name>\r\n<Val></Val>\r\n</String>\r\n<String>\r\n<Name> </Name>\r\n<Val></Val>\r\n</String>\r\n<String>\r\n<Name> </Name>\r\n<Val></Val>\r\n</String>\r\n<String>\r\n<Name> </Name>\r\n<Val></Val>\r\n</String>\r\n<String>\r\n<Name> </Name>\r\n<Val></Val>\r\n</String>\r\n<String>\r\n<Name> </Name>\r\n<Val></Val>\r\n</String>\r\n<String>\r\n<Name> </Name>\r\n<Val></Val>\r\n</String>\r\n<String>\r\n<Name> </Name>\r\n<Val></Val>\r\n</String>\r\n<String>\r\n<Name> </Name>\r\n<Val></Val>\r\n</String>\r\n<String>\r\n<Name> </Name>\r\n<Val></Val>\r\n</String>\r\n<String>\r\n<Name> </Name>\r\n<Val></Val>\r\n</String>\r\n<String>\r\n<Name> </Name>\r\n<Val></Val>\r\n</String>\r\n<String>\r\n<Name> </Name>\r\n<Val></Val>\r\n</String>\r\n<String>\r\n<Name> </Name>\r\n<Val></Val>\r\n</String>\r\n<String>\r\n<Name> </Name>\r\n<Val></Val>\r\n</String>\r\n<String>\r\n<Name> </Name>\r\n<Val></Val>\r\n</String>\r\n<String>\r\n<Name> </Name>\r\n<Val></Val>\r\n</String>\r\n<String>\r\n<Name> </Name>\r\n<Val></Val>\r\n</String>\r\n<String>\r\n<Name> </Name>\r\n<Val></Val>\r\n</String>\r\n<String>\r\n<Name> </Name>\r\n<Val></Val>\r\n</String>\r\n<String>\r\n<Name> </Name>\r\n<Val></Val>\r\n</String>\r\n<String>\r\n<Name> </Name>\r\n<Val></Val>\r\n</String>\r\n<String>\r\n<Name> </Name>\r\n<Val></Val>\r\n</String>\r\n<String>\r\n<Name> </Name>\r\n<Val></Val>\r\n</String>\r\n<String>\r\n<Name> </Name>\r\n<Val></Val>\r\n</String>\r\n<String>\r\n<Name> </Name>\r\n<Val></Val>\r\n</String>\r\n<String>\r\n<Name> </Name>\r\n<Val></Val>\r\n</String>\r\n<String>\r\n<Name> </Name>\r\n<Val></Val>\r\n</String>\r\n<String>\r\n<Name> </Name>\r\n<Val></Val>\r\n</String>\r\n<String>\r\n<Name> </Name>\r\n<Val></Val>\r\n</String>\r\n<String>\r\n<Name> </Name>\r\n<Val></Val>\r\n</String>\r\n<String>\r\n<Name> </Name>\r\n<Val></Val>\r\n</String>\r\n<String>\r\n<Name> </Name>\r\n<Val></Val>\r\n</String>\r\n<String>\r\n<Name> </Name>\r\n<Val></Val>\r\n</String>\r\n<String>\r\n<Name> </Name>\r\n<Val></Val>\r\n</String>\r\n<String>\r\n<Name> </Name>\r\n<Val></Val>\r\n</String>\r\n<String>\r\n<Name> </Name>\r\n<Val></Val>\r\n</String>\r\n<String>\r\n<Name> </Name>\r\n<Val></Val>\r\n</String>\r\n<String>\r\n<Name> </Name>\r\n<Val></Val>\r\n</String>\r\n<String>\r\n<Name> </Name>\r\n<Val></Val>\r\n</String>\r\n<String>\r\n<Name> </Name>\r\n<Val></Val>\r\n</String>\r\n<String>\r\n<Name> </Name>\r\n<Val></Val>\r\n</String>\r\n<String>\r\n<Name> </Name>\r\n<Val></Val>\r\n</String>\r\n<String>\r\n<Name> </Name>\r\n<Val></Val>\r\n</String>\r\n<String>\r\n<Name> </Name>\r\n<Val></Val>\r\n</String>\r\n<String>\r\n<Name> </Name>\r\n<Val></Val>\r\n</String>\r\n<String>\r\n<Name> </Name>\r\n<Val></Val>\r\n</String>\r\n<String>\r\n<Name> </Name>\r\n<Val></Val>\r\n</String>\r\n<String>\r\n<Name> </Name>\r\n<Val></Val>\r\n</String>\r\n<String>\r\n<Name> </Name>\r\n<Val></Val>\r\n</String>\r\n<String>\r\n<Name> </Name>\r\n<Val></Val>\r\n</String>\r\n<String>\r\n<Name> </Name>\r\n<Val></Val>\r\n</String>\r\n<String>\r\n<Name> </Name>\r\n<Val></Val>\r\n</String>\r\n<String>\r\n<Name> </Name>\r\n<Val></Val>\r\n</String>\r\n<String>\r\n<Name> </Name>\r\n<Val></Val>\r\n</String>\r\n<String>\r\n<Name> </Name>\r\n<Val></Val>\r\n</String>\r\n<String>\r\n<Name> </Name>\r\n<Val></Val>\r\n</String>\r\n<String>\r\n<Name> </Name>\r\n<Val></Val>\r\n</String>\r\n<String>\r\n<Name> </Name>\r\n<Val></Val>\r\n</String>\r\n<String>\r\n<Name> </Name>\r\n<Val></Val>\r\n</String>\r\n<String>\r\n<Name> </Name>\r\n<Val></Val>\r\n</String>\r\n<String>\r\n<Name> </Name>\r\n<Val></Val>\r\n</String>\r\n<String>\r\n<Name> </Name>\r\n<Val></Val>\r\n</String>\r\n<String>\r\n<Name> </Name>\r\n<Val></Val>\r\n</String>\r\n<String>\r\n<Name> </Name>\r\n<Val></Val>\r\n</String>\r\n<String>\r\n<Name> </Name>\r\n<Val></Val>\r\n</String>\r\n<String>\r\n<Name> </Name>\r\n<Val></Val>\r\n</String>\r\n<String>\r\n<Name> </Name>\r\n<Val></Val>\r\n</String>\r\n<String>\r\n<Name> </Name>\r\n<Val></Val>\r\n</String>\r\n<String>\r\n<Name> </Name>\r\n<Val></Val>\r\n</String>\r\n<String>\r\n<Name> </Name>\r\n<Val></Val>\r\n</String>\r\n<String>\r\n<Name> </Name>\r\n<Val></Val>\r\n</String>\r\n<String>\r\n<Name> </Name>\r\n<Val></Val>\r\n</String>\r\n<String>\r\n<Name> </Name>\r\n<Val></Val>\r\n</String>\r\n<String>\r\n<Name> </Name>\r\n<Val></Val>\r\n</String>\r\n<String>\r\n<Name> </Name>\r\n<Val></Val>\r\n</String>\r\n<String>\r\n<Name> </Name>\r\n<Val></Val>\r\n</String>\r\n<String>\r\n<Name> </Name>\r\n<Val></Val>\r\n</String>\r\n<String>\r\n<Name> </Name>\r\n<Val>-47.7708</Val>\r\n</String>\r\n<String>\r\n<Name> </Name>\r\n<Val></Val>\r\n</String>\r\n<String>\r\n<Name> </Name>\r\n<Val></Val>\r\n</String>\r\n<String>\r\n<Name> </Name>\r\n<Val></Val>\r\n</String>\r\n<String>\r\n<Name> </Name>\r\n<Val></Val>\r\n</String>\r\n<String>\r\n<Name> </Name>\r\n<Val></Val>\r\n</String>\r\n<String>\r\n<Name> </Name>\r\n<Val></Val>\r\n</String>\r\n<String>\r\n<Name> </Name>\r\n<Val>-4.54522</Val>\r\n</String>\r\n<String>\r\n<Name> </Name>\r\n<Val></Val>\r\n</String>\r\n<String>\r\n<Name> </Name>\r\n<Val></Val>\r\n</String>\r\n<String>\r\n<Name> </Name>\r\n<Val></Val>\r\n</String>\r\n<String>\r\n<Name> </Name>\r\n<Val></Val>\r\n</String>\r\n<String>\r\n<Name> </Name>\r\n<Val>-48.004</Val>\r\n</String>\r\n<String>\r\n<Name> </Name>\r\n<Val></Val>\r\n</String>\r\n<String>\r\n<Name> </Name>\r\n<Val></Val>\r\n</String>\r\n<String>\r\n<Name> </Name>\r\n<Val></Val>\r\n</String>\r\n<String>\r\n<Name> </Name>\r\n<Val></Val>\r\n</String>\r\n<String>\r\n<Name> </Name>\r\n<Val></Val>\r\n</String>\r\n<String>\r\n<Name> </Name>\r\n<Val></Val>\r\n</String>\r\n<String>\r\n<Name> </Name>\r\n<Val>-4.19756</Val>\r\n</String>\r\n<String>\r\n<Name> </Name>\r\n<Val></Val>\r\n</String>\r\n<String>\r\n<Name> </Name>\r\n<Val></Val>\r\n</String>\r\n<String>\r\n<Name> </Name>\r\n<Val></Val>\r\n</String>\r\n<String>\r\n<Name> </Name>\r\n<Val></Val>\r\n</String>\r\n<String>\r\n<Name> </Name>\r\n<Val>-66.764</Val>\r\n</String>\r\n<String>\r\n<Name> </Name>\r\n<Val></Val>\r\n</String>\r\n<String>\r\n<Name> </Name>\r\n<Val></Val>\r\n</String>\r\n<String>\r\n<Name> </Name>\r\n<Val></Val>\r\n</String>\r\n<String>\r\n<Name> </Name>\r\n<Val></Val>\r\n</String>\r\n<String>\r\n<Name> </Name>\r\n<Val></Val>\r\n</String>\r\n<String>\r\n<Name> </Name>\r\n<Val></Val>\r\n</String>\r\n<String>\r\n<Name> </Name>\r\n<Val>-3.6094</Val>\r\n</String>\r\n<String>\r\n<Name> </Name>\r\n<Val></Val>\r\n</String>\r\n<String>\r\n<Name> </Name>\r\n<Val></Val>\r\n</String>\r\n<String>\r\n<Name> </Name>\r\n<Val></Val>\r\n</String>\r\n<String>\r\n<Name> </Name>\r\n<Val></Val>\r\n</String>\r\n<String>\r\n<Name> </Name>\r\n<Val>-48.2936</Val>\r\n</String>\r\n<String>\r\n<Name> </Name>\r\n<Val></Val>\r\n</String>\r\n<String>\r\n<Name> </Name>\r\n<Val></Val>\r\n</String>\r\n<String>\r\n<Name> </Name>\r\n<Val></Val>\r\n</String>\r\n<String>\r\n<Name> </Name>\r\n<Val></Val>\r\n</String>\r\n<String>\r\n<Name> </Name>\r\n<Val></Val>\r\n</String>\r\n<String>\r\n<Name> </Name>\r\n<Val></Val>\r\n</String>\r\n<String>\r\n<Name> </Name>\r\n<Val>-5.00136</Val>\r\n</String>\r\n<String>\r\n<Name> </Name>\r\n<Val></Val>\r\n</String>\r\n<String>\r\n<Name> </Name>\r\n<Val></Val>\r\n</String>\r\n<String>\r\n<Name> </Name>\r\n<Val></Val>\r\n</String>\r\n<String>\r\n<Name> </Name>\r\n<Val></Val>\r\n</String>\r\n<String>\r\n<Name> </Name>\r\n<Val></Val>\r\n</String>\r\n<String>\r\n<Name> </Name>\r\n<Val></Val>\r\n</String>\r\n<String>\r\n<Name> </Name>\r\n<Val>-69.476</Val>\r\n</String>\r\n<String>\r\n<Name> </Name>\r\n<Val></Val>\r\n</String>\r\n<String>\r\n<Name> </Name>\r\n<Val></Val>\r\n</String>\r\n<String>\r\n<Name> </Name>\r\n<Val></Val>\r\n</String>\r\n<String>\r\n<Name> </Name>\r\n<Val></Val>\r\n</String>\r\n<String>\r\n<Name> </Name>\r\n<Val></Val>\r\n</String>\r\n<String>\r\n<Name> </Name>\r\n<Val></Val>\r\n</String>\r\n<String>\r\n<Name> </Name>\r\n<Val>-3.48634</Val>\r\n</String>\r\n<String>\r\n<Name> </Name>\r\n<Val></Val>\r\n</String>\r\n<String>\r\n<Name> </Name>\r\n<Val></Val>\r\n</String>\r\n<String>\r\n<Name> </Name>\r\n<Val></Val>\r\n</String>\r\n<String>\r\n<Name> </Name>\r\n<Val></Val>\r\n</String>\r\n<String>\r\n<Name> </Name>\r\n<Val>-60.346</Val>\r\n</String>\r\n<String>\r\n<Name> </Name>\r\n<Val></Val>\r\n</String>\r\n<String>\r\n<Name> </Name>\r\n<Val></Val>\r\n</String>\r\n<String>\r\n<Name> </Name>\r\n<Val></Val>\r\n</String>\r\n<String>\r\n<Name> </Name>\r\n<Val></Val>\r\n</String>\r\n<String>\r\n<Name> </Name>\r\n<Val></Val>\r\n</String>\r\n<String>\r\n<Name> </Name>\r\n<Val></Val>\r\n</String>\r\n<String>\r\n<Name> </Name>\r\n<Val>-3.23766</Val>\r\n</String>\r\n<String>\r\n<Name> </Name>\r\n<Val></Val>\r\n</String>\r\n<String>\r\n<Name> </Name>\r\n<Val></Val>\r\n</String>\r\n<String>\r\n<Name> </Name>\r\n<Val></Val>\r\n</String>\r\n<String>\r\n<Name> </Name>\r\n<Val></Val>\r\n</String>\r\n<String>\r\n<Name> </Name>\r\n<Val>-48.4202</Val>\r\n</String>\r\n<String>\r\n<Name> </Name>\r\n<Val></Val>\r\n</String>\r\n<String>\r\n<Name> </Name>\r\n<Val></Val>\r\n</String>\r\n<String>\r\n<Name> </Name>\r\n<Val></Val>\r\n</String>\r\n<String>\r\n<Name> </Name>\r\n<Val></Val>\r\n</String>\r\n<String>\r\n<Name> </Name>\r\n<Val></Val>\r\n</String>\r\n<String>\r\n<Name> </Name>\r\n<Val></Val>\r\n</String>\r\n<String>\r\n<Name> </Name>\r\n<Val>-4.78534</Val>\r\n</String>\r\n<String>\r\n<Name> </Name>\r\n<Val></Val>\r\n</String>\r\n<String>\r\n<Name> </Name>\r\n<Val></Val>\r\n</String>\r\n<String>\r\n<Name> </Name>\r\n<Val></Val>\r\n</String>\r\n<String>\r\n<Name> </Name>\r\n<Val></Val>\r\n</String>\r\n<String>\r\n<Name> </Name>\r\n<Val>-47.9334</Val>\r\n</String>\r\n<String>\r\n<Name> </Name>\r\n<Val></Val>\r\n</String>\r\n<String>\r\n<Name> </Name>\r\n<Val></Val>\r\n</String>\r\n<String>\r\n<Name> </Name>\r\n<Val></Val>\r\n</String>\r\n<String>\r\n<Name> </Name>\r\n<Val></Val>\r\n</String>\r\n<String>\r\n<Name> </Name>\r\n<Val></Val>\r\n</String>\r\n<String>\r\n<Name> </Name>\r\n<Val></Val>\r\n</String>\r\n<String>\r\n<Name> </Name>\r\n<Val>-3.93968</Val>\r\n</String>\r\n<String>\r\n<Name> </Name>\r\n<Val></Val>\r\n</String>\r\n<String>\r\n<Name> </Name>\r\n<Val></Val>\r\n</String>\r\n<String>\r\n<Name> </Name>\r\n<Val></Val>\r\n</String>\r\n<String>\r\n<Name> </Name>\r\n<Val></Val>\r\n</String>\r\n<String>\r\n<Name> </Name>\r\n<Val></Val>\r\n</String>\r\n<String>\r\n<Name> </Name>\r\n<Val></Val>\r\n</String>\r\n<String>\r\n<Name> </Name>\r\n<Val>-40.85416</Val>\r\n</String>\r\n<String>\r\n<Name> </Name>\r\n<Val></Val>\r\n</String>\r\n<String>\r\n<Name> </Name>\r\n<Val></Val>\r\n</String>\r\n<String>\r\n<Name> </Name>\r\n<Val></Val>\r\n</String>\r\n<String>\r\n<Name> </Name>\r\n<Val></Val>\r\n</String>\r\n<String>\r\n<Name> </Name>\r\n<Val></Val>\r\n</String>\r\n<String>\r\n<Name> </Name>\r\n<Val></Val>\r\n</String>\r\n<String>\r\n<Name> </Name>\r\n<Val>-3.99712</Val>\r\n</String>\r\n<String>\r\n<Name> </Name>\r\n<Val></Val>\r\n</String>\r\n<String>\r\n<Name> </Name>\r\n<Val></Val>\r\n</String>\r\n<String>\r\n<Name> </Name>\r\n<Val></Val>\r\n</String>\r\n<String>\r\n<Name> </Name>\r\n<Val></Val>\r\n</String>\r\n<String>\r\n<Name> </Name>\r\n<Val>-70.622</Val>\r\n</String>\r\n<String>\r\n<Name> </Name>\r\n<Val></Val>\r\n</String>\r\n<String>\r\n<Name> </Name>\r\n<Val></Val>\r\n</String>\r\n<String>\r\n<Name> </Name>\r\n<Val></Val>\r\n</String>\r\n<String>\r\n<Name> </Name>\r\n<Val></Val>\r\n</String>\r\n<String>\r\n<Name> </Name>\r\n<Val></Val>\r\n</String>\r\n<String>\r\n<Name> </Name>\r\n<Val></Val>\r\n</String>\r\n<String>\r\n<Name> </Name>\r\n<Val>-3.9661</Val>\r\n</String>\r\n<String>\r\n<Name> </Name>\r\n<Val></Val>\r\n</String>\r\n<String>\r\n<Name> </Name>\r\n<Val></Val>\r\n</String>\r\n<String>\r\n<Name> </Name>\r\n<Val></Val>\r\n</String>\r\n<String>\r\n<Name> </Name>\r\n<Val></Val>\r\n</String>\r\n<String>\r\n<Name> </Name>\r\n<Val>-47.0772</Val>\r\n</String>\r\n<String>\r\n<Name> </Name>\r\n<Val></Val>\r\n</String>\r\n<String>\r\n<Name> </Name>\r\n<Val></Val>\r\n</String>\r\n<String>\r\n<Name> </Name>\r\n<Val></Val>\r\n</String>\r\n<String>\r\n<Name> </Name>\r\n<Val></Val>\r\n</String>\r\n<String>\r\n<Name> </Name>\r\n<Val></Val>\r\n</String>\r\n<String>\r\n<Name> </Name>\r\n<Val></Val>\r\n</String>\r\n<String>\r\n<Name> </Name>\r\n<Val>-3.95874</Val>\r\n</String>\r\n<String>\r\n<Name> </Name>\r\n<Val></Val>\r\n</String>\r\n<String>\r\n<Name> </Name>\r\n<Val></Val>\r\n</String>\r\n<String>\r\n<Name> </Name>\r\n<Val></Val>\r\n</String>\r\n<String>\r\n<Name> </Name>\r\n<Val></Val>\r\n</String>\r\n<String>\r\n<Name> </Name>\r\n<Val>-49.2812</Val>\r\n</String>\r\n<String>\r\n<Name> </Name>\r\n<Val></Val>\r\n</String>\r\n<String>\r\n<Name> </Name>\r\n<Val></Val>\r\n</String>\r\n<String>\r\n<Name> </Name>\r\n<Val></Val>\r\n</String>\r\n<String>\r\n<Name> </Name>\r\n<Val></Val>\r\n</String>\r\n<String>\r\n<Name> </Name>\r\n<Val></Val>\r\n</String>\r\n<String>\r\n<Name> </Name>\r\n<Val></Val>\r\n</String>\r\n<String>\r\n<Name> </Name>\r\n<Val>-4.96502</Val>\r\n</String>\r\n<String>\r\n<Name> </Name>\r\n<Val></Val>\r\n</String>\r\n<String>\r\n<Name> </Name>\r\n<Val></Val>\r\n</String>\r\n<String>\r\n<Name> </Name>\r\n<Val></Val>\r\n</String>\r\n<String>\r\n<Name> </Name>\r\n<Val></Val>\r\n</String>\r\n<String>\r\n<Name> </Name>\r\n<Val></Val>\r\n</String>\r\n<String>\r\n<Name> </Name>\r\n<Val></Val>\r\n</String>\r\n<String>\r\n<Name> </Name>\r\n<Val>-46.3062</Val>\r\n</String>\r\n<String>\r\n<Name> </Name>\r\n<Val></Val>\r\n</String>\r\n<String>\r\n<Name> </Name>\r\n<Val></Val>\r\n</String>\r\n<String>\r\n<Name> </Name>\r\n<Val></Val>\r\n</String>\r\n<String>\r\n<Name> </Name>\r\n<Val></Val>\r\n</String>\r\n<String>\r\n<Name> </Name>\r\n<Val></Val>\r\n</String>\r\n<String>\r\n<Name> </Name>\r\n<Val></Val>\r\n</String>\r\n<String>\r\n<Name> </Name>\r\n<Val>-3.9467</Val>\r\n</String>\r\n<String>\r\n<Name> </Name>\r\n<Val></Val>\r\n</String>\r\n<String>\r\n<Name> </Name>\r\n<Val></Val>\r\n</String>\r\n<String>\r\n<Name> </Name>\r\n<Val></Val>\r\n</String>\r\n<String>\r\n<Name> </Name>\r\n<Val></Val>\r\n</String>\r\n<String>\r\n<Name> </Name>\r\n<Val>-46.2894</Val>\r\n</String>\r\n<String>\r\n<Name> </Name>\r\n<Val></Val>\r\n</String>\r\n<String>\r\n<Name> </Name>\r\n<Val></Val>\r\n</String>\r\n<String>\r\n<Name> </Name>\r\n<Val></Val>\r\n</String>\r\n<String>\r\n<Name> </Name>\r\n<Val></Val>\r\n</String>\r\n<String>\r\n<Name> </Name>\r\n<Val></Val>\r\n</String>\r\n<String>\r\n<Name> </Name>\r\n<Val></Val>\r\n</String>\r\n<String>\r\n<Name> </Name>\r\n<Val>-3.78498</Val>\r\n</String>\r\n<String>\r\n<Name> </Name>\r\n<Val></Val>\r\n</String>\r\n<String>\r\n<Name> </Name>\r\n<Val></Val>\r\n</String>\r\n<String>\r\n<Name> </Name>\r\n<Val></Val>\r\n</String>\r\n<String>\r\n<Name> </Name>\r\n<Val></Val>\r\n</String>\r\n<String>\r\n<Name> </Name>\r\n<Val>-49.828</Val>\r\n</String>\r\n<String>\r\n<Name> </Name>\r\n<Val></Val>\r\n</String>\r\n<String>\r\n<Name> </Name>\r\n<Val></Val>\r\n</String>\r\n<String>\r\n<Name> </Name>\r\n<Val></Val>\r\n</String>\r\n<String>\r\n<Name> </Name>\r\n<Val></Val>\r\n</String>\r\n<String>\r\n<Name> </Name>\r\n<Val></Val>\r\n</String>\r\n<String>\r\n<Name> </Name>\r\n<Val></Val>\r\n</String>\r\n<String>\r\n<Name> </Name>\r\n<Val>-5.02942</Val>\r\n</String>\r\n<String>\r\n<Name> </Name>\r\n<Val></Val>\r\n</String>\r\n<String>\r\n<Name> </Name>\r\n<Val></Val>\r\n</String>\r\n<String>\r\n<Name> </Name>\r\n<Val></Val>\r\n</String>\r\n<String>\r\n<Name> </Name>\r\n<Val></Val>\r\n</String>\r\n<String>\r\n<Name> </Name>\r\n<Val>-46.6118</Val>\r\n</String>\r\n<String>\r\n<Name> </Name>\r\n<Val></Val>\r\n</String>\r\n<String>\r\n<Name> </Name>\r\n<Val></Val>\r\n</String>\r\n<String>\r\n<Name> </Name>\r\n<Val></Val>\r\n</String>\r\n<String>\r\n<Name> </Name>\r\n<Val></Val>\r\n</String>\r\n<String>\r\n<Name> </Name>\r\n<Val></Val>\r\n</String>\r\n<String>\r\n<Name> </Name>\r\n<Val></Val>\r\n</String>\r\n<String>\r\n<Name> </Name>\r\n<Val>-4.24462</Val>\r\n</String>\r\n<String>\r\n<Name> </Name>\r\n<Val></Val>\r\n</String>\r\n<String>\r\n<Name> </Name>\r\n<Val></Val>\r\n</String>\r\n<String>\r\n<Name> </Name>\r\n<Val></Val>\r\n</String>\r\n<String>\r\n<Name> </Name>\r\n<Val></Val>\r\n</String>\r\n<String>\r\n<Name> </Name>\r\n<Val></Val>\r\n</String>\r\n<String>\r\n<Name> </Name>\r\n<Val></Val>\r\n</String>\r\n<String>\r\n<Name> </Name>\r\n<Val></Val>\r\n</String>\r\n<String>\r\n<Name> </Name>\r\n<Val></Val>\r\n</String>\r\n<String>\r\n<Name> </Name>\r\n<Val></Val>\r\n</String>\r\n<String>\r\n<Name> </Name>\r\n<Val></Val>\r\n</String>\r\n<String>\r\n<Name> </Name>\r\n<Val></Val>\r\n</String>\r\n<String>\r\n<Name> </Name>\r\n<Val></Val>\r\n</String>\r\n<String>\r\n<Name> </Name>\r\n<Val></Val>\r\n</String>\r\n<String>\r\n<Name> </Name>\r\n<Val></Val>\r\n</String>\r\n<String>\r\n<Name> </Name>\r\n<Val></Val>\r\n</String>\r\n<String>\r\n<Name> </Name>\r\n<Val></Val>\r\n</String>\r\n<String>\r\n<Name> </Name>\r\n<Val></Val>\r\n</String>\r\n<String>\r\n<Name> </Name>\r\n<Val></Val>\r\n</String>\r\n<String>\r\n<Name> </Name>\r\n<Val></Val>\r\n</String>\r\n<String>\r\n<Name> </Name>\r\n<Val></Val>\r\n</String>\r\n<String>\r\n<Name> </Name>\r\n<Val></Val>\r\n</String>\r\n<String>\r\n<Name> </Name>\r\n<Val></Val>\r\n</String>\r\n<String>\r\n<Name> </Name>\r\n<Val></Val>\r\n</String>\r\n<String>\r\n<Name> </Name>\r\n<Val></Val>\r\n</String>\r\n<String>\r\n<Name> </Name>\r\n<Val></Val>\r\n</String>\r\n<String>\r\n<Name> </Name>\r\n<Val></Val>\r\n</String>\r\n<String>\r\n<Name> </Name>\r\n<Val></Val>\r\n</String>\r\n<String>\r\n<Name> </Name>\r\n<Val></Val>\r\n</String>\r\n<String>\r\n<Name> </Name>\r\n<Val></Val>\r\n</String>\r\n<String>\r\n<Name> </Name>\r\n<Val></Val>\r\n</String>\r\n<String>\r\n<Name> </Name>\r\n<Val></Val>\r\n</String>\r\n<String>\r\n<Name> </Name>\r\n<Val></Val>\r\n</String>\r\n<String>\r\n<Name> </Name>\r\n<Val></Val>\r\n</String>\r\n<String>\r\n<Name> </Name>\r\n<Val></Val>\r\n</String>\r\n<String>\r\n<Name> </Name>\r\n<Val></Val>\r\n</String>\r\n<String>\r\n<Name> </Name>\r\n<Val></Val>\r\n</String>\r\n<String>\r\n<Name> </Name>\r\n<Val></Val>\r\n</String>\r\n<String>\r\n<Name> </Name>\r\n<Val></Val>\r\n</String>\r\n<String>\r\n<Name> </Name>\r\n<Val></Val>\r\n</String>\r\n<String>\r\n<Name> </Name>\r\n<Val></Val>\r\n</String>\r\n<String>\r\n<Name> </Name>\r\n<Val></Val>\r\n</String>\r\n<String>\r\n<Name> </Name>\r\n<Val></Val>\r\n</String>\r\n<String>\r\n<Name> </Name>\r\n<Val></Val>\r\n</String>\r\n<String>\r\n<Name> </Name>\r\n<Val></Val>\r\n</String>\r\n<String>\r\n<Name> </Name>\r\n<Val></Val>\r\n</String>\r\n<String>\r\n<Name> </Name>\r\n<Val></Val>\r\n</String>\r\n<String>\r\n<Name> </Name>\r\n<Val></Val>\r\n</String>\r\n<String>\r\n<Name> </Name>\r\n<Val></Val>\r\n</String>\r\n<String>\r\n<Name> </Name>\r\n<Val></Val>\r\n</String>\r\n<String>\r\n<Name> </Name>\r\n<Val></Val>\r\n</String>\r\n<String>\r\n<Name> </Name>\r\n<Val></Val>\r\n</String>\r\n<String>\r\n<Name> </Name>\r\n<Val></Val>\r\n</String>\r\n<String>\r\n<Name> </Name>\r\n<Val></Val>\r\n</String>\r\n<String>\r\n<Name> </Name>\r\n<Val></Val>\r\n</String>\r\n<String>\r\n<Name> </Name>\r\n<Val></Val>\r\n</String>\r\n<String>\r\n<Name> </Name>\r\n<Val></Val>\r\n</String>\r\n<String>\r\n<Name> </Name>\r\n<Val></Val>\r\n</String>\r\n<String>\r\n<Name> </Name>\r\n<Val></Val>\r\n</String>\r\n<String>\r\n<Name> </Name>\r\n<Val></Val>\r\n</String>\r\n<String>\r\n<Name> </Name>\r\n<Val></Val>\r\n</String>\r\n<String>\r\n<Name> </Name>\r\n<Val></Val>\r\n</String>\r\n<String>\r\n<Name> </Name>\r\n<Val></Val>\r\n</String>\r\n<String>\r\n<Name> </Name>\r\n<Val></Val>\r\n</String>\r\n<String>\r\n<Name> </Name>\r\n<Val></Val>\r\n</String>\r\n<String>\r\n<Name> </Name>\r\n<Val></Val>\r\n</String>\r\n<String>\r\n<Name> </Name>\r\n<Val></Val>\r\n</String>\r\n<String>\r\n<Name> </Name>\r\n<Val></Val>\r\n</String>\r\n<String>\r\n<Name> </Name>\r\n<Val></Val>\r\n</String>\r\n<String>\r\n<Name> </Name>\r\n<Val></Val>\r\n</String>\r\n<String>\r\n<Name> </Name>\r\n<Val></Val>\r\n</String>\r\n<String>\r\n<Name> </Name>\r\n<Val></Val>\r\n</String>\r\n<String>\r\n<Name> </Name>\r\n<Val></Val>\r\n</String>\r\n<String>\r\n<Name> </Name>\r\n<Val></Val>\r\n</String>\r\n<String>\r\n<Name> </Name>\r\n<Val></Val>\r\n</String>\r\n<String>\r\n<Name> </Name>\r\n<Val></Val>\r\n</String>\r\n<String>\r\n<Name> </Name>\r\n<Val></Val>\r\n</String>\r\n<String>\r\n<Name> </Name>\r\n<Val></Val>\r\n</String>\r\n<String>\r\n<Name> </Name>\r\n<Val></Val>\r\n</String>\r\n<String>\r\n<Name> </Name>\r\n<Val></Val>\r\n</String>\r\n<String>\r\n<Name> </Name>\r\n<Val></Val>\r\n</String>\r\n<String>\r\n<Name> </Name>\r\n<Val></Val>\r\n</String>\r\n<String>\r\n<Name> </Name>\r\n<Val></Val>\r\n</String>\r\n<String>\r\n<Name> </Name>\r\n<Val></Val>\r\n</String>\r\n<String>\r\n<Name> </Name>\r\n<Val></Val>\r\n</String>\r\n<String>\r\n<Name> </Name>\r\n<Val></Val>\r\n</String>\r\n<String>\r\n<Name> </Name>\r\n<Val></Val>\r\n</String>\r\n<String>\r\n<Name> </Name>\r\n<Val></Val>\r\n</String>\r\n<String>\r\n<Name> </Name>\r\n<Val></Val>\r\n</String>\r\n<String>\r\n<Name> </Name>\r\n<Val></Val>\r\n</String>\r\n<String>\r\n<Name> </Name>\r\n<Val></Val>\r\n</String>\r\n<String>\r\n<Name> </Name>\r\n<Val></Val>\r\n</String>\r\n<String>\r\n<Name> </Name>\r\n<Val></Val>\r\n</String>\r\n<String>\r\n<Name> </Name>\r\n<Val></Val>\r\n</String>\r\n<String>\r\n<Name> </Name>\r\n<Val></Val>\r\n</String>\r\n<String>\r\n<Name> </Name>\r\n<Val>Begin Sequence: MainSequence\n\n\r(D:\\Program Files\\TMS\\Working TPS\\MfgInfo UUT &amp; TPS Verification.seq)</Val>\r\n</String>\r\n<String>\r\n<Name> </Name>\r\n<Val></Val>\r\n</String>\r\n<String>\r\n<Name> </Name>\r\n<Val>Begin Sequence: Get UUT Information\n\n\r(D:\\Program Files\\TMS\\Working TPS\\SN16K\\SN16K Common Sequences.seq)</Val>\r\n</String>\r\n<String>\r\n<Name> </Name>\r\n<Val>**** UUT Info ****\r\n\rProduct Code :               910244\r\n\rSerial Number :           N635017050\r\n\rRevision Number :                   AB\r\n\rMAC Address :                     \r\n\rCard Type :                   9E\r\n\r850 Part Number :          8500052410E\r\n\r850 BOM Revision :                  0L1\r\n\rECI Code :               127544\rCLEI Code :           SOC2G33BAA</Val>\r\n</String>\r\n<String>\r\n<Name> </Name>\r\n<Val>TPS P/N  -   889-16032-03\n\rTPS Rev  -  D</Val>\r\n</String>\r\n<String>\r\n<Name> </Name>\r\n<Val>Begin Sequence: Check for Genealogy\n\n\r(D:\\Program Files\\TMS\\Working TPS\\MfgInfo UUT &amp; TPS Verification.seq)</Val>\r\n</String>\r\n<String>\r\n<Name> </Name>\r\n<Val></Val>\r\n</String>\r\n<String>\r\n<Name> </Name>\r\n<Val>Begin Sequence: Get UUT Genealogy Information\n\n\r(D:\\Program Files\\TMS\\Working TPS\\SN16K\\SN16K Common Sequences.seq)</Val>\r\n</String>\r\n<String>\r\n<Name> </Name>\r\n<Val>Begin Sequence: Genealogy Dialog\n\n\r(D:\\Program Files\\TMS\\Working TPS\\MfgInfo UUT &amp; TPS Verification.seq)</Val>\r\n</String>\r\n<String>\r\n<Name> </Name>\r\n<Val>GENEALOGY DATA:[ SAU1;C071911 | SAU2;C071901 | SAU3;X81639309 | SBU14;X82240260 | SBU13;C071912 | SBU12;C071909 | SAU12;C073101 | SAU13;C071903 | SAU14;X81639310 | SBU3;C071905 | SBU2;C072405 | SBU1;C072408 ]</Val>\r\n</String>\r\n<String>\r\n<Name> </Name>\r\n<Val></Val>\r\n</String>\r\n<String>\r\n<Name> </Name>\r\n<Val></Val>\r\n</String>\r\n<String>\r\n<Name> </Name>\r\n<Val></Val>\r\n</String>\r\n<String>\r\n<Name> </Name>\r\n<Val></Val>\r\n</String>\r\n<String>\r\n<Name> </Name>\r\n<Val></Val>\r\n</String>\r\n<String>\r\n<Name> </Name>\r\n<Val></Val>\r\n</String>\r\n<String>\r\n<Name> </Name>\r\n<Val></Val>\r\n</String>\r\n<String>\r\n<Name> </Name>\r\n<Val></Val>\r\n</String>\r\n<String>\r\n<Name> </Name>\r\n<Val>Begin Sequence: Install and Connect UUT\n\n\r(D:\\Program Files\\TMS\\Working TPS\\SN16K\\Gsc\\Gsc-MC\\SN16K GSC-MC Full (Fixed Pad).seq)</Val>\r\n</String>\r\n<String>\r\n<Name> </Name>\r\n<Val></Val>\r\n</String>\r\n<String>\r\n<Name> </Name>\r\n<Val></Val>\r\n</String>\r\n<String>\r\n<Name> </Name>\r\n<Val>Begin Sequence: Power UP\n\n\r(D:\\Program Files\\TMS\\Working TPS\\SN16K\\Gsc\\Gsc-MC\\SN16K GSC-MC Full (Fixed Pad).seq)</Val>\r\n</String>\r\n<String>\r\n<Name> </Name>\r\n<Val></Val>\r\n</String>\r\n<String>\r\n<Name> </Name>\r\n<Val></Val>\r\n</String>\r\n<String>\r\n<Name> </Name>\r\n<Val></Val>\r\n</String>\r\n<String>\r\n<Name> </Name>\r\n<Val></Val>\r\n</String>\r\n<String>\r\n<Name> </Name>\r\n<Val></Val>\r\n</String>\r\n<String>\r\n<Name> </Name>\r\n<Val></Val>\r\n</String>\r\n<String>\r\n<Name> </Name>\r\n<Val></Val>\r\n</String>\r\n<String>\r\n<Name> </Name>\r\n<Val>Begin Sequence: MainSequence\n\n\r(D:\\Program Files\\TMS\\Working TPS\\SN16K\\SN16K XLoad.seq)</Val>\r\n</String>\r\n<String>\r\n<Name> </Name>\r\n<Val></Val>\r\n</String>\r\n<String>\r\n<Name> </Name>\r\n<Val>Done...\r\n\r\r\n\r\r\r\n\r\r\n\rPress any key to stop auto-boot...\r\n\r 1\r 0\r\r\n\rauto-booting...\r\n\r\r\n\r\r\n\rboot device          : motfcc\r\n\runit number          : 0 \r\n\rprocessor number     : 0 \r\n\rfile name            : /home/ftp/xxx\r\n\rflags (f)            : 0x8 \r\n\rother (o)            : sycamoreLineCard\r\n\r\r\n\r\n\r\t\n\rAttached TCP/IP interface to motfcc0.\r\n\rAttaching network interface lo0... done.\r\n\r\r\n\rBooting using SN-16000 Sycamore Line Card procedure.</Val>\r\n</String>\r\n<String>\r\n<Name> </Name>\r\n<Val></Val>\r\n</String>\r\n<String>\r\n<Name> </Name>\r\n<Val></Val>\r\n</String>\r\n<String>\r\n<Name> </Name>\r\n<Val>RomMiniMon</Val>\r\n</String>\r\n<String>\r\n<Name> </Name>\r\n<Val>GSC64x2 Rev_D 300Mhz Baserom, built on 13:10:46 Mar 25 2003, build 0296.360\r\n\r8260 Build 0296.322 Thu Aug 08 19:44:24 2002\r\n\rGSC64 Build 0296.365.DG1 Fri Oct 31 18:25:01 2003\rgsc64x2Rev_D, 0296.323, 13Aug02</Val>\r\n</String>\r\n<String>\r\n<Name> </Name>\r\n<Val></Val>\r\n</String>\r\n<String>\r\n<Name> </Name>\r\n<Val>baserom:GSC64x2 Rev_D 300Mhz Baserom, built on 13:10:46 Mar 25 2003, build 0296.360\n\r\r\n\r\rbootrom:8260 Build 0493 Tue Aug 31 16:50:09 2004\n\r\r\n\r\rdiagrom:GSC64 Build 0296.365.DG1 Fri Oct 31 18:25:01 2003\n\r\r\rfpga:gsc64x2Rev_D, Release3, 10Jul03</Val>\r\n</String>\r\n<String>\r\n<Name> </Name>\r\n<Val></Val>\r\n</String>\r\n<String>\r\n<Name> </Name>\r\n<Val></Val>\r\n</String>\r\n<String>\r\n<Name> </Name>\r\n<Val></Val>\r\n</String>\r\n<String>\r\n<Name> </Name>\r\n<Val></Val>\r\n</String>\r\n<String>\r\n<Name> </Name>\r\n<Val></Val>\r\n</String>\r\n<String>\r\n<Name> </Name>\r\n<Val></Val>\r\n</String>\r\n<String>\r\n<Name> </Name>\r\n<Val>RomMiniMon</Val>\r\n</String>\r\n<String>\r\n<Name> </Name>\r\n<Val></Val>\r\n</String>\r\n<String>\r\n<Name> </Name>\r\n<Val></Val>\r\n</String>\r\n<String>\r\n<Name> </Name>\r\n<Val></Val>\r\n</String>\r\n<String>\r\n<Name> </Name>\r\n<Val></Val>\r\n</String>\r\n<String>\r\n<Name> </Name>\r\n<Val></Val>\r\n</String>\r\n<String>\r\n<Name> </Name>\r\n<Val>Diag</Val>\r\n</String>\r\n<String>\r\n<Name> </Name>\r\n<Val></Val>\r\n</String>\r\n<String>\r\n<Name> </Name>\r\n<Val>BaseRom : GSC64x2 Rev_D 300Mhz Baserom, built on 13:10:46 Mar 25 2003, build 0296.360\n\r\r\n\r\rBootRom : 8260 Build 0296.322 Thu Aug 08 19:44:24 2002\n\r\r\n\r\rDiagRom : GSC64 Build 0296.365.DG1 Fri Oct 31 18:25:01 2003\n\r\r\rFpga : gsc64x2Rev_D, 0296.323, 13Aug02</Val>\r\n</String>\r\n<String>\r\n<Name> </Name>\r\n<Val></Val>\r\n</String>\r\n<String>\r\n<Name> </Name>\r\n<Val></Val>\r\n</String>\r\n<String>\r\n<Name> </Name>\r\n<Val>Begin Sequence: Electrical Diags\n\n\r(D:\\Program Files\\TMS\\Working TPS\\SN16K\\Gsc\\Gsc-MC\\SN16K GSC-MC Full (Fixed Pad).seq)</Val>\r\n</String>\r\n<String>\r\n<Name> </Name>\r\n<Val>Begin Sequence: LED Test\n\n\r(D:\\Program Files\\TMS\\Working TPS\\SN16K\\Gsc\\Gsc-MC\\SN16K GSC-MC Full (Fixed Pad).seq)</Val>\r\n</String>\r\n<String>\r\n<Name> </Name>\r\n<Val></Val>\r\n</String>\r\n<String>\r\n<Name> </Name>\r\n<Val></Val>\r\n</String>\r\n<String>\r\n<Name> </Name>\r\n<Val></Val>\r\n</String>\r\n<String>\r\n<Name> </Name>\r\n<Val></Val>\r\n</String>\r\n<String>\r\n<Name> </Name>\r\n<Val>Begin Sequence: FCC Tests\n\n\r(D:\\Program Files\\TMS\\Working TPS\\SN16K\\Gsc\\Gsc-MC\\SN16K GSC-MC Full (Fixed Pad).seq)</Val>\r\n</String>\r\n<String>\r\n<Name> </Name>\r\n<Val></Val>\r\n</String>\r\n<String>\r\n<Name> </Name>\r\n<Val></Val>\r\n</String>\r\n<String>\r\n<Name> </Name>\r\n<Val></Val>\r\n</String>\r\n<String>\r\n<Name> </Name>\r\n<Val></Val>\r\n</String>\r\n<String>\r\n<Name> </Name>\r\n<Val>f2..f1..f0..ef..ee..ed..ec..eb..ea..e9..e8..e7..e6..PASS -- 'initbrd' passed '1' time(s)</Val>\r\n</String>\r\n<String>\r\n<Name> </Name>\r\n<Val></Val>\r\n</String>\r\n<String>\r\n<Name> </Name>\r\n<Val></Val>\r\n</String>\r\n<String>\r\n<Name> </Name>\r\n<Val></Val>\r\n</String>\r\n<String>\r\n<Name> </Name>\r\n<Val></Val>\r\n</String>\r\n<String>\r\n<Name> </Name>\r\n<Val></Val>\r\n</String>\r\n<String>\r\n<Name> </Name>\r\n<Val></Val>\r\n</String>\r\n<String>\r\n<Name> </Name>\r\n<Val></Val>\r\n</String>\r\n<String>\r\n<Name> </Name>\r\n<Val></Val>\r\n</String>\r\n<String>\r\n<Name> </Name>\r\n<Val></Val>\r\n</String>\r\n<String>\r\n<Name> </Name>\r\n<Val></Val>\r\n</String>\r\n<String>\r\n<Name> </Name>\r\n<Val></Val>\r\n</String>\r\n<String>\r\n<Name> </Name>\r\n<Val>Begin Sequence: FPGA Tests\n\n\r(D:\\Program Files\\TMS\\Working TPS\\SN16K\\Gsc\\Gsc-MC\\SN16K GSC-MC Full (Fixed Pad).seq)</Val>\r\n</String>\r\n<String>\r\n<Name> </Name>\r\n<Val></Val>\r\n</String>\r\n<String>\r\n<Name> </Name>\r\n<Val></Val>\r\n</String>\r\n<String>\r\n<Name> </Name>\r\n<Val>Begin Sequence: EEPROM Tests\n\n\r(D:\\Program Files\\TMS\\Working TPS\\SN16K\\Gsc\\Gsc-MC\\SN16K GSC-MC Full (Fixed Pad).seq)</Val>\r\n</String>\r\n<String>\r\n<Name> </Name>\r\n<Val></Val>\r\n</String>\r\n<String>\r\n<Name> </Name>\r\n<Val></Val>\r\n</String>\r\n<String>\r\n<Name> </Name>\r\n<Val></Val>\r\n</String>\r\n<String>\r\n<Name> </Name>\r\n<Val></Val>\r\n</String>\r\n<String>\r\n<Name> </Name>\r\n<Val></Val>\r\n</String>\r\n<String>\r\n<Name> </Name>\r\n<Val>Begin Sequence: CPLD Tests\n\n\r(D:\\Program Files\\TMS\\Working TPS\\SN16K\\Gsc\\Gsc-MC\\SN16K GSC-MC Full (Fixed Pad).seq)</Val>\r\n</String>\r\n<String>\r\n<Name> </Name>\r\n<Val>Control CPLD, Rev : 4 (0x4)\rPASS -- 'crev' passed '1' time(s)</Val>\r\n</String>\r\n<String>\r\n<Name> </Name>\r\n<Val></Val>\r\n</String>\r\n<String>\r\n<Name> </Name>\r\n<Val></Val>\r\n</String>\r\n<String>\r\n<Name> </Name>\r\n<Val></Val>\r\n</String>\r\n<String>\r\n<Name> </Name>\r\n<Val>Begin Sequence: GXC Tests\n\n\r(D:\\Program Files\\TMS\\Working TPS\\SN16K\\Gsc\\Gsc-MC\\SN16K GSC-MC Full (Fixed Pad).seq)</Val>\r\n</String>\r\n<String>\r\n<Name> </Name>\r\n<Val>GXC B (revision 32) is alive.\rPASS -- 'gxcalive' passed '1' time(s)</Val>\r\n</String>\r\n<String>\r\n<Name> </Name>\r\n<Val></Val>\r\n</String>\r\n<String>\r\n<Name> </Name>\r\n<Val>GXC A (revision 32) is alive.\rPASS -- 'gxcalive' passed '1' time(s)</Val>\r\n</String>\r\n<String>\r\n<Name> </Name>\r\n<Val></Val>\r\n</String>\r\n<String>\r\n<Name> </Name>\r\n<Val>Begin Sequence: Local Timing Tests\n\n\r(D:\\Program Files\\TMS\\Working TPS\\SN16K\\Gsc\\Gsc-MC\\SN16K GSC-MC Full (Fixed Pad).seq)</Val>\r\n</String>\r\n<String>\r\n<Name> </Name>\r\n<Val></Val>\r\n</String>\r\n<String>\r\n<Name> </Name>\r\n<Val></Val>\r\n</String>\r\n<String>\r\n<Name> </Name>\r\n<Val></Val>\r\n</String>\r\n<String>\r\n<Name> </Name>\r\n<Val></Val>\r\n</String>\r\n<String>\r\n<Name> </Name>\r\n<Val></Val>\r\n</String>\r\n<String>\r\n<Name> </Name>\r\n<Val>Begin Sequence: PRBS Path Thru Switch Tests\n\n\r(D:\\Program Files\\TMS\\Working TPS\\SN16K\\Gsc\\Gsc-MC\\SN16K GSC-MC Full (Fixed Pad).seq)</Val>\r\n</String>\r\n<String>\r\n<Name> </Name>\r\n<Val>Begin Sequence: PRBS Path Thru Switch B\n\n\r(D:\\Program Files\\TMS\\Working TPS\\SN16K\\Gsc\\Gsc-MC\\SN16K GSC-MC Full (Fixed Pad).seq)</Val>\r\n</String>\r\n<String>\r\n<Name> </Name>\r\n<Val></Val>\r\n</String>\r\n<String>\r\n<Name> </Name>\r\n<Val></Val>\r\n</String>\r\n<String>\r\n<Name> </Name>\r\n<Val></Val>\r\n</String>\r\n<String>\r\n<Name> </Name>\r\n<Val></Val>\r\n</String>\r\n<String>\r\n<Name> </Name>\r\n<Val></Val>\r\n</String>\r\n<String>\r\n<Name> </Name>\r\n<Val></Val>\r\n</String>\r\n<String>\r\n<Name> </Name>\r\n<Val></Val>\r\n</String>\r\n<String>\r\n<Name> </Name>\r\n<Val>Begin Sequence: PRBS Path Thru Switch A\n\n\r(D:\\Program Files\\TMS\\Working TPS\\SN16K\\Gsc\\Gsc-MC\\SN16K GSC-MC Full (Fixed Pad).seq)</Val>\r\n</String>\r\n<String>\r\n<Name> </Name>\r\n<Val></Val>\r\n</String>\r\n<String>\r\n<Name> </Name>\r\n<Val></Val>\r\n</String>\r\n<String>\r\n<Name> </Name>\r\n<Val></Val>\r\n</String>\r\n<String>\r\n<Name> </Name>\r\n<Val></Val>\r\n</String>\r\n<String>\r\n<Name> </Name>\r\n<Val></Val>\r\n</String>\r\n<String>\r\n<Name> </Name>\r\n<Val></Val>\r\n</String>\r\n<String>\r\n<Name> </Name>\r\n<Val></Val>\r\n</String>\r\n<String>\r\n<Name> </Name>\r\n<Val>Begin Sequence: Electrical Backplane Tests\n\n\r(D:\\Program Files\\TMS\\Working TPS\\SN16K\\Gsc\\Gsc-MC\\SN16K GSC-MC Full (Fixed Pad).seq)</Val>\r\n</String>\r\n<String>\r\n<Name> </Name>\r\n<Val>Begin Sequence: SMC Tests\n\n\r(D:\\Program Files\\TMS\\Working TPS\\SN16K\\Gsc\\Gsc-MC\\SN16K GSC-MC Full (Fixed Pad).seq)</Val>\r\n</String>\r\n<String>\r\n<Name> </Name>\r\n<Val></Val>\r\n</String>\r\n<String>\r\n<Name> </Name>\r\n<Val></Val>\r\n</String>\r\n<String>\r\n<Name> </Name>\r\n<Val></Val>\r\n</String>\r\n<String>\r\n<Name> </Name>\r\n<Val></Val>\r\n</String>\r\n<String>\r\n<Name> </Name>\r\n<Val></Val>\r\n</String>\r\n<String>\r\n<Name> </Name>\r\n<Val></Val>\r\n</String>\r\n<String>\r\n<Name> </Name>\r\n<Val></Val>\r\n</String>\r\n<String>\r\n<Name> </Name>\r\n<Val></Val>\r\n</String>\r\n<String>\r\n<Name> </Name>\r\n<Val></Val>\r\n</String>\r\n<String>\r\n<Name> </Name>\r\n<Val></Val>\r\n</String>\r\n<String>\r\n<Name> </Name>\r\n<Val></Val>\r\n</String>\r\n<String>\r\n<Name> </Name>\r\n<Val></Val>\r\n</String>\r\n<String>\r\n<Name> </Name>\r\n<Val></Val>\r\n</String>\r\n<String>\r\n<Name> </Name>\r\n<Val></Val>\r\n</String>\r\n<String>\r\n<Name> </Name>\r\n<Val></Val>\r\n</String>\r\n<String>\r\n<Name> </Name>\r\n<Val></Val>\r\n</String>\r\n<String>\r\n<Name> </Name>\r\n<Val></Val>\r\n</String>\r\n<String>\r\n<Name> </Name>\r\n<Val></Val>\r\n</String>\r\n<String>\r\n<Name> </Name>\r\n<Val>Begin Sequence: TRC Timing Tests\n\n\r(D:\\Program Files\\TMS\\Working TPS\\SN16K\\Gsc\\Gsc-MC\\SN16K GSC-MC Full (Fixed Pad).seq)</Val>\r\n</String>\r\n<String>\r\n<Name> </Name>\r\n<Val></Val>\r\n</String>\r\n<String>\r\n<Name> </Name>\r\n<Val></Val>\r\n</String>\r\n<String>\r\n<Name> </Name>\r\n<Val>Begin Sequence: TRC A Tests\n\n\r(D:\\Program Files\\TMS\\Working TPS\\SN16K\\Gsc\\Gsc-MC\\SN16K GSC-MC Full (Fixed Pad).seq)</Val>\r\n</String>\r\n<String>\r\n<Name> </Name>\r\n<Val></Val>\r\n</String>\r\n<String>\r\n<Name> </Name>\r\n<Val></Val>\r\n</String>\r\n<String>\r\n<Name> </Name>\r\n<Val></Val>\r\n</String>\r\n<String>\r\n<Name> </Name>\r\n<Val></Val>\r\n</String>\r\n<String>\r\n<Name> </Name>\r\n<Val></Val>\r\n</String>\r\n<String>\r\n<Name> </Name>\r\n<Val></Val>\r\n</String>\r\n<String>\r\n<Name> </Name>\r\n<Val></Val>\r\n</String>\r\n<String>\r\n<Name> </Name>\r\n<Val></Val>\r\n</String>\r\n<String>\r\n<Name> </Name>\r\n<Val></Val>\r\n</String>\r\n<String>\r\n<Name> </Name>\r\n<Val>Begin Sequence: TRC B Tests\n\n\r(D:\\Program Files\\TMS\\Working TPS\\SN16K\\Gsc\\Gsc-MC\\SN16K GSC-MC Full (Fixed Pad).seq)</Val>\r\n</String>\r\n<String>\r\n<Name> </Name>\r\n<Val></Val>\r\n</String>\r\n<String>\r\n<Name> </Name>\r\n<Val></Val>\r\n</String>\r\n<String>\r\n<Name> </Name>\r\n<Val></Val>\r\n</String>\r\n<String>\r\n<Name> </Name>\r\n<Val></Val>\r\n</String>\r\n<String>\r\n<Name> </Name>\r\n<Val></Val>\r\n</String>\r\n<String>\r\n<Name> </Name>\r\n<Val></Val>\r\n</String>\r\n<String>\r\n<Name> </Name>\r\n<Val></Val>\r\n</String>\r\n<String>\r\n<Name> </Name>\r\n<Val></Val>\r\n</String>\r\n<String>\r\n<Name> </Name>\r\n<Val></Val>\r\n</String>\r\n<String>\r\n<Name> </Name>\r\n<Val>Begin Sequence: Fsync Tests\n\n\r(D:\\Program Files\\TMS\\Working TPS\\SN16K\\Gsc\\Gsc-MC\\SN16K GSC-MC Full (Fixed Pad).seq)</Val>\r\n</String>\r\n<String>\r\n<Name> </Name>\r\n<Val></Val>\r\n</String>\r\n<String>\r\n<Name> </Name>\r\n<Val></Val>\r\n</String>\r\n<String>\r\n<Name> </Name>\r\n<Val></Val>\r\n</String>\r\n<String>\r\n<Name> </Name>\r\n<Val></Val>\r\n</String>\r\n<String>\r\n<Name> </Name>\r\n<Val></Val>\r\n</String>\r\n<String>\r\n<Name> </Name>\r\n<Val></Val>\r\n</String>\r\n<String>\r\n<Name> </Name>\r\n<Val></Val>\r\n</String>\r\n<String>\r\n<Name> </Name>\r\n<Val></Val>\r\n</String>\r\n<String>\r\n<Name> </Name>\r\n<Val></Val>\r\n</String>\r\n<String>\r\n<Name> </Name>\r\n<Val></Val>\r\n</String>\r\n<String>\r\n<Name> </Name>\r\n<Val></Val>\r\n</String>\r\n<String>\r\n<Name> </Name>\r\n<Val></Val>\r\n</String>\r\n<String>\r\n<Name> </Name>\r\n<Val></Val>\r\n</String>\r\n<String>\r\n<Name> </Name>\r\n<Val>Begin Sequence: Chassis and Slot ID Tests\n\n\r(D:\\Program Files\\TMS\\Working TPS\\SN16K\\Gsc\\Gsc-MC\\SN16K GSC-MC Full (Fixed Pad).seq)</Val>\r\n</String>\r\n<String>\r\n<Name> </Name>\r\n<Val></Val>\r\n</String>\r\n<String>\r\n<Name> </Name>\r\n<Val></Val>\r\n</String>\r\n<String>\r\n<Name> </Name>\r\n<Val></Val>\r\n</String>\r\n<String>\r\n<Name> </Name>\r\n<Val></Val>\r\n</String>\r\n<String>\r\n<Name> </Name>\r\n<Val></Val>\r\n</String>\r\n<String>\r\n<Name> </Name>\r\n<Val></Val>\r\n</String>\r\n<String>\r\n<Name> </Name>\r\n<Val></Val>\r\n</String>\r\n<String>\r\n<Name> </Name>\r\n<Val></Val>\r\n</String>\r\n<String>\r\n<Name> </Name>\r\n<Val></Val>\r\n</String>\r\n<String>\r\n<Name> </Name>\r\n<Val></Val>\r\n</String>\r\n<String>\r\n<Name> </Name>\r\n<Val>Begin Sequence: BP LED Test\n\n\r(D:\\Program Files\\TMS\\Working TPS\\SN16K\\Gsc\\Gsc-MC\\SN16K GSC-MC Full (Fixed Pad).seq)</Val>\r\n</String>\r\n<String>\r\n<Name> </Name>\r\n<Val></Val>\r\n</String>\r\n<String>\r\n<Name> </Name>\r\n<Val></Val>\r\n</String>\r\n<String>\r\n<Name> </Name>\r\n<Val></Val>\r\n</String>\r\n<String>\r\n<Name> </Name>\r\n<Val></Val>\r\n</String>\r\n<String>\r\n<Name> </Name>\r\n<Val></Val>\r\n</String>\r\n<String>\r\n<Name> </Name>\r\n<Val></Val>\r\n</String>\r\n<String>\r\n<Name> </Name>\r\n<Val></Val>\r\n</String>\r\n<String>\r\n<Name> </Name>\r\n<Val></Val>\r\n</String>\r\n<String>\r\n<Name> </Name>\r\n<Val></Val>\r\n</String>\r\n<String>\r\n<Name> </Name>\r\n<Val>Begin Sequence: Optical Backplane Tests\n\n\r(D:\\Program Files\\TMS\\Working TPS\\SN16K\\Gsc\\Gsc-MC\\SN16K GSC-MC Full (Fixed Pad).seq)</Val>\r\n</String>\r\n<String>\r\n<Name> </Name>\r\n<Val></Val>\r\n</String>\r\n<String>\r\n<Name> </Name>\r\n<Val>Begin Sequence: Verify VCSEL Outputs\n\n\r(D:\\Program Files\\TMS\\Working TPS\\SN16K\\Gsc\\Gsc-MC\\SN16K GSC-MC Full (Fixed Pad).seq)</Val>\r\n</String>\r\n<String>\r\n<Name> </Name>\r\n<Val></Val>\r\n</String>\r\n<String>\r\n<Name> </Name>\r\n<Val>Begin Sequence: Test Outputs from One MT\n\n\r(D:\\Program Files\\TMS\\Working TPS\\SN16K\\Gsc\\Gsc-MC\\SN16K GSC-MC Full (Fixed Pad).seq)</Val>\r\n</String>\r\n<String>\r\n<Name> </Name>\r\n<Val></Val>\r\n</String>\r\n<String>\r\n<Name> </Name>\r\n<Val></Val>\r\n</String>\r\n<String>\r\n<Name> </Name>\r\n<Val>Quadpack 1, MT  1, OPM channel index    0</Val>\r\n</String>\r\n<String>\r\n<Name> </Name>\r\n<Val></Val>\r\n</String>\r\n<String>\r\n<Name> </Name>\r\n<Val></Val>\r\n</String>\r\n<String>\r\n<Name> </Name>\r\n<Val></Val>\r\n</String>\r\n<String>\r\n<Name> </Name>\r\n<Val></Val>\r\n</String>\r\n<String>\r\n<Name> </Name>\r\n<Val></Val>\r\n</String>\r\n<String>\r\n<Name> </Name>\r\n<Val></Val>\r\n</String>\r\n<String>\r\n<Name> </Name>\r\n<Val>Quadpack 1, MT  1, OPM channel index    0</Val>\r\n</String>\r\n<String>\r\n<Name> </Name>\r\n<Val></Val>\r\n</String>\r\n<String>\r\n<Name> </Name>\r\n<Val>Begin Sequence: Test Outputs from One MT\n\n\r(D:\\Program Files\\TMS\\Working TPS\\SN16K\\Gsc\\Gsc-MC\\SN16K GSC-MC Full (Fixed Pad).seq)</Val>\r\n</String>\r\n<String>\r\n<Name> </Name>\r\n<Val></Val>\r\n</String>\r\n<String>\r\n<Name> </Name>\r\n<Val></Val>\r\n</String>\r\n<String>\r\n<Name> </Name>\r\n<Val>Quadpack 1, MT  2, OPM channel index    0</Val>\r\n</String>\r\n<String>\r\n<Name> </Name>\r\n<Val></Val>\r\n</String>\r\n<String>\r\n<Name> </Name>\r\n<Val></Val>\r\n</String>\r\n<String>\r\n<Name> </Name>\r\n<Val></Val>\r\n</String>\r\n<String>\r\n<Name> </Name>\r\n<Val></Val>\r\n</String>\r\n<String>\r\n<Name> </Name>\r\n<Val></Val>\r\n</String>\r\n<String>\r\n<Name> </Name>\r\n<Val></Val>\r\n</String>\r\n<String>\r\n<Name> </Name>\r\n<Val>Quadpack 1, MT  2, OPM channel index    0</Val>\r\n</String>\r\n<String>\r\n<Name> </Name>\r\n<Val></Val>\r\n</String>\r\n<String>\r\n<Name> </Name>\r\n<Val>Begin Sequence: Test Outputs from One MT\n\n\r(D:\\Program Files\\TMS\\Working TPS\\SN16K\\Gsc\\Gsc-MC\\SN16K GSC-MC Full (Fixed Pad).seq)</Val>\r\n</String>\r\n<String>\r\n<Name> </Name>\r\n<Val></Val>\r\n</String>\r\n<String>\r\n<Name> </Name>\r\n<Val></Val>\r\n</String>\r\n<String>\r\n<Name> </Name>\r\n<Val>Quadpack 1, MT  3, OPM channel index    0</Val>\r\n</String>\r\n<String>\r\n<Name> </Name>\r\n<Val></Val>\r\n</String>\r\n<String>\r\n<Name> </Name>\r\n<Val></Val>\r\n</String>\r\n<String>\r\n<Name> </Name>\r\n<Val></Val>\r\n</String>\r\n<String>\r\n<Name> </Name>\r\n<Val></Val>\r\n</String>\r\n<String>\r\n<Name> </Name>\r\n<Val></Val>\r\n</String>\r\n<String>\r\n<Name> </Name>\r\n<Val></Val>\r\n</String>\r\n<String>\r\n<Name> </Name>\r\n<Val>Quadpack 1, MT  3, OPM channel index    0</Val>\r\n</String>\r\n<String>\r\n<Name> </Name>\r\n<Val></Val>\r\n</String>\r\n<String>\r\n<Name> </Name>\r\n<Val>Begin Sequence: Test Outputs from One MT\n\n\r(D:\\Program Files\\TMS\\Working TPS\\SN16K\\Gsc\\Gsc-MC\\SN16K GSC-MC Full (Fixed Pad).seq)</Val>\r\n</String>\r\n<String>\r\n<Name> </Name>\r\n<Val></Val>\r\n</String>\r\n<String>\r\n<Name> </Name>\r\n<Val></Val>\r\n</String>\r\n<String>\r\n<Name> </Name>\r\n<Val>Quadpack 1, MT  4, OPM channel index    0</Val>\r\n</String>\r\n<String>\r\n<Name> </Name>\r\n<Val></Val>\r\n</String>\r\n<String>\r\n<Name> </Name>\r\n<Val></Val>\r\n</String>\r\n<String>\r\n<Name> </Name>\r\n<Val></Val>\r\n</String>\r\n<String>\r\n<Name> </Name>\r\n<Val></Val>\r\n</String>\r\n<String>\r\n<Name> </Name>\r\n<Val></Val>\r\n</String>\r\n<String>\r\n<Name> </Name>\r\n<Val></Val>\r\n</String>\r\n<String>\r\n<Name> </Name>\r\n<Val>Quadpack 1, MT  4, OPM channel index    0</Val>\r\n</String>\r\n<String>\r\n<Name> </Name>\r\n<Val></Val>\r\n</String>\r\n<String>\r\n<Name> </Name>\r\n<Val>Begin Sequence: Verify VCSEL Outputs\n\n\r(D:\\Program Files\\TMS\\Working TPS\\SN16K\\Gsc\\Gsc-MC\\SN16K GSC-MC Full (Fixed Pad).seq)</Val>\r\n</String>\r\n<String>\r\n<Name> </Name>\r\n<Val></Val>\r\n</String>\r\n<String>\r\n<Name> </Name>\r\n<Val>Begin Sequence: Test Outputs from One MT\n\n\r(D:\\Program Files\\TMS\\Working TPS\\SN16K\\Gsc\\Gsc-MC\\SN16K GSC-MC Full (Fixed Pad).seq)</Val>\r\n</String>\r\n<String>\r\n<Name> </Name>\r\n<Val></Val>\r\n</String>\r\n<String>\r\n<Name> </Name>\r\n<Val></Val>\r\n</String>\r\n<String>\r\n<Name> </Name>\r\n<Val>Quadpack 2, MT  1, OPM channel index    0</Val>\r\n</String>\r\n<String>\r\n<Name> </Name>\r\n<Val></Val>\r\n</String>\r\n<String>\r\n<Name> </Name>\r\n<Val></Val>\r\n</String>\r\n<String>\r\n<Name> </Name>\r\n<Val></Val>\r\n</String>\r\n<String>\r\n<Name> </Name>\r\n<Val></Val>\r\n</String>\r\n<String>\r\n<Name> </Name>\r\n<Val></Val>\r\n</String>\r\n<String>\r\n<Name> </Name>\r\n<Val></Val>\r\n</String>\r\n<String>\r\n<Name> </Name>\r\n<Val>Quadpack 2, MT  1, OPM channel index    0</Val>\r\n</String>\r\n<String>\r\n<Name> </Name>\r\n<Val></Val>\r\n</String>\r\n<String>\r\n<Name> </Name>\r\n<Val>Begin Sequence: Test Outputs from One MT\n\n\r(D:\\Program Files\\TMS\\Working TPS\\SN16K\\Gsc\\Gsc-MC\\SN16K GSC-MC Full (Fixed Pad).seq)</Val>\r\n</String>\r\n<String>\r\n<Name> </Name>\r\n<Val></Val>\r\n</String>\r\n<String>\r\n<Name> </Name>\r\n<Val></Val>\r\n</String>\r\n<String>\r\n<Name> </Name>\r\n<Val>Quadpack 2, MT  2, OPM channel index    0</Val>\r\n</String>\r\n<String>\r\n<Name> </Name>\r\n<Val></Val>\r\n</String>\r\n<String>\r\n<Name> </Name>\r\n<Val></Val>\r\n</String>\r\n<String>\r\n<Name> </Name>\r\n<Val></Val>\r\n</String>\r\n<String>\r\n<Name> </Name>\r\n<Val></Val>\r\n</String>\r\n<String>\r\n<Name> </Name>\r\n<Val></Val>\r\n</String>\r\n<String>\r\n<Name> </Name>\r\n<Val></Val>\r\n</String>\r\n<String>\r\n<Name> </Name>\r\n<Val>Quadpack 2, MT  2, OPM channel index    0</Val>\r\n</String>\r\n<String>\r\n<Name> </Name>\r\n<Val></Val>\r\n</String>\r\n<String>\r\n<Name> </Name>\r\n<Val>Begin Sequence: Test Outputs from One MT\n\n\r(D:\\Program Files\\TMS\\Working TPS\\SN16K\\Gsc\\Gsc-MC\\SN16K GSC-MC Full (Fixed Pad).seq)</Val>\r\n</String>\r\n<String>\r\n<Name> </Name>\r\n<Val></Val>\r\n</String>\r\n<String>\r\n<Name> </Name>\r\n<Val></Val>\r\n</String>\r\n<String>\r\n<Name> </Name>\r\n<Val>Quadpack 2, MT  3, OPM channel index    0</Val>\r\n</String>\r\n<String>\r\n<Name> </Name>\r\n<Val></Val>\r\n</String>\r\n<String>\r\n<Name> </Name>\r\n<Val></Val>\r\n</String>\r\n<String>\r\n<Name> </Name>\r\n<Val></Val>\r\n</String>\r\n<String>\r\n<Name> </Name>\r\n<Val></Val>\r\n</String>\r\n<String>\r\n<Name> </Name>\r\n<Val></Val>\r\n</String>\r\n<String>\r\n<Name> </Name>\r\n<Val></Val>\r\n</String>\r\n<String>\r\n<Name> </Name>\r\n<Val>Quadpack 2, MT  3, OPM channel index    0</Val>\r\n</String>\r\n<String>\r\n<Name> </Name>\r\n<Val></Val>\r\n</String>\r\n<String>\r\n<Name> </Name>\r\n<Val>Begin Sequence: Test Outputs from One MT\n\n\r(D:\\Program Files\\TMS\\Working TPS\\SN16K\\Gsc\\Gsc-MC\\SN16K GSC-MC Full (Fixed Pad).seq)</Val>\r\n</String>\r\n<String>\r\n<Name> </Name>\r\n<Val></Val>\r\n</String>\r\n<String>\r\n<Name> </Name>\r\n<Val></Val>\r\n</String>\r\n<String>\r\n<Name> </Name>\r\n<Val>Quadpack 2, MT  4, OPM channel index    0</Val>\r\n</String>\r\n<String>\r\n<Name> </Name>\r\n<Val></Val>\r\n</String>\r\n<String>\r\n<Name> </Name>\r\n<Val></Val>\r\n</String>\r\n<String>\r\n<Name> </Name>\r\n<Val></Val>\r\n</String>\r\n<String>\r\n<Name> </Name>\r\n<Val></Val>\r\n</String>\r\n<String>\r\n<Name> </Name>\r\n<Val></Val>\r\n</String>\r\n<String>\r\n<Name> </Name>\r\n<Val></Val>\r\n</String>\r\n<String>\r\n<Name> </Name>\r\n<Val>Quadpack 2, MT  4, OPM channel index    0</Val>\r\n</String>\r\n<String>\r\n<Name> </Name>\r\n<Val></Val>\r\n</String>\r\n<String>\r\n<Name> </Name>\r\n<Val>Begin Sequence: Verify VCSEL Outputs\n\n\r(D:\\Program Files\\TMS\\Working TPS\\SN16K\\Gsc\\Gsc-MC\\SN16K GSC-MC Full (Fixed Pad).seq)</Val>\r\n</String>\r\n<String>\r\n<Name> </Name>\r\n<Val></Val>\r\n</String>\r\n<String>\r\n<Name> </Name>\r\n<Val>Begin Sequence: Test Outputs from One MT\n\n\r(D:\\Program Files\\TMS\\Working TPS\\SN16K\\Gsc\\Gsc-MC\\SN16K GSC-MC Full (Fixed Pad).seq)</Val>\r\n</String>\r\n<String>\r\n<Name> </Name>\r\n<Val></Val>\r\n</String>\r\n<String>\r\n<Name> </Name>\r\n<Val></Val>\r\n</String>\r\n<String>\r\n<Name> </Name>\r\n<Val>Quadpack 3, MT  1, OPM channel index    0</Val>\r\n</String>\r\n<String>\r\n<Name> </Name>\r\n<Val></Val>\r\n</String>\r\n<String>\r\n<Name> </Name>\r\n<Val></Val>\r\n</String>\r\n<String>\r\n<Name> </Name>\r\n<Val></Val>\r\n</String>\r\n<String>\r\n<Name> </Name>\r\n<Val></Val>\r\n</String>\r\n<String>\r\n<Name> </Name>\r\n<Val></Val>\r\n</String>\r\n<String>\r\n<Name> </Name>\r\n<Val></Val>\r\n</String>\r\n<String>\r\n<Name> </Name>\r\n<Val>Quadpack 3, MT  1, OPM channel index    0</Val>\r\n</String>\r\n<String>\r\n<Name> </Name>\r\n<Val></Val>\r\n</String>\r\n<String>\r\n<Name> </Name>\r\n<Val>Begin Sequence: Test Outputs from One MT\n\n\r(D:\\Program Files\\TMS\\Working TPS\\SN16K\\Gsc\\Gsc-MC\\SN16K GSC-MC Full (Fixed Pad).seq)</Val>\r\n</String>\r\n<String>\r\n<Name> </Name>\r\n<Val></Val>\r\n</String>\r\n<String>\r\n<Name> </Name>\r\n<Val></Val>\r\n</String>\r\n<String>\r\n<Name> </Name>\r\n<Val>Quadpack 3, MT  2, OPM channel index    0</Val>\r\n</String>\r\n<String>\r\n<Name> </Name>\r\n<Val></Val>\r\n</String>\r\n<String>\r\n<Name> </Name>\r\n<Val></Val>\r\n</String>\r\n<String>\r\n<Name> </Name>\r\n<Val></Val>\r\n</String>\r\n<String>\r\n<Name> </Name>\r\n<Val></Val>\r\n</String>\r\n<String>\r\n<Name> </Name>\r\n<Val></Val>\r\n</String>\r\n<String>\r\n<Name> </Name>\r\n<Val></Val>\r\n</String>\r\n<String>\r\n<Name> </Name>\r\n<Val>Quadpack 3, MT  2, OPM channel index    0</Val>\r\n</String>\r\n<String>\r\n<Name> </Name>\r\n<Val></Val>\r\n</String>\r\n<String>\r\n<Name> </Name>\r\n<Val>Begin Sequence: Test Outputs from One MT\n\n\r(D:\\Program Files\\TMS\\Working TPS\\SN16K\\Gsc\\Gsc-MC\\SN16K GSC-MC Full (Fixed Pad).seq)</Val>\r\n</String>\r\n<String>\r\n<Name> </Name>\r\n<Val></Val>\r\n</String>\r\n<String>\r\n<Name> </Name>\r\n<Val></Val>\r\n</String>\r\n<String>\r\n<Name> </Name>\r\n<Val>Quadpack 3, MT  3, OPM channel index    0</Val>\r\n</String>\r\n<String>\r\n<Name> </Name>\r\n<Val></Val>\r\n</String>\r\n<String>\r\n<Name> </Name>\r\n<Val></Val>\r\n</String>\r\n<String>\r\n<Name> </Name>\r\n<Val></Val>\r\n</String>\r\n<String>\r\n<Name> </Name>\r\n<Val></Val>\r\n</String>\r\n<String>\r\n<Name> </Name>\r\n<Val></Val>\r\n</String>\r\n<String>\r\n<Name> </Name>\r\n<Val></Val>\r\n</String>\r\n<String>\r\n<Name> </Name>\r\n<Val>Quadpack 3, MT  3, OPM channel index    0</Val>\r\n</String>\r\n<String>\r\n<Name> </Name>\r\n<Val></Val>\r\n</String>\r\n<String>\r\n<Name> </Name>\r\n<Val>Begin Sequence: Test Outputs from One MT\n\n\r(D:\\Program Files\\TMS\\Working TPS\\SN16K\\Gsc\\Gsc-MC\\SN16K GSC-MC Full (Fixed Pad).seq)</Val>\r\n</String>\r\n<String>\r\n<Name> </Name>\r\n<Val></Val>\r\n</String>\r\n<String>\r\n<Name> </Name>\r\n<Val></Val>\r\n</String>\r\n<String>\r\n<Name> </Name>\r\n<Val>Quadpack 3, MT  4, OPM channel index    0</Val>\r\n</String>\r\n<String>\r\n<Name> </Name>\r\n<Val></Val>\r\n</String>\r\n<String>\r\n<Name> </Name>\r\n<Val></Val>\r\n</String>\r\n<String>\r\n<Name> </Name>\r\n<Val></Val>\r\n</String>\r\n<String>\r\n<Name> </Name>\r\n<Val></Val>\r\n</String>\r\n<String>\r\n<Name> </Name>\r\n<Val></Val>\r\n</String>\r\n<String>\r\n<Name> </Name>\r\n<Val></Val>\r\n</String>\r\n<String>\r\n<Name> </Name>\r\n<Val>Quadpack 3, MT  4, OPM channel index    0</Val>\r\n</String>\r\n<String>\r\n<Name> </Name>\r\n<Val></Val>\r\n</String>\r\n<String>\r\n<Name> </Name>\r\n<Val>Begin Sequence: Verify VCSEL Outputs\n\n\r(D:\\Program Files\\TMS\\Working TPS\\SN16K\\Gsc\\Gsc-MC\\SN16K GSC-MC Full (Fixed Pad).seq)</Val>\r\n</String>\r\n<String>\r\n<Name> </Name>\r\n<Val></Val>\r\n</String>\r\n<String>\r\n<Name> </Name>\r\n<Val>Begin Sequence: Test Outputs from One MT\n\n\r(D:\\Program Files\\TMS\\Working TPS\\SN16K\\Gsc\\Gsc-MC\\SN16K GSC-MC Full (Fixed Pad).seq)</Val>\r\n</String>\r\n<String>\r\n<Name> </Name>\r\n<Val></Val>\r\n</String>\r\n<String>\r\n<Name> </Name>\r\n<Val></Val>\r\n</String>\r\n<String>\r\n<Name> </Name>\r\n<Val>Quadpack 4, MT  1, OPM channel index    0</Val>\r\n</String>\r\n<String>\r\n<Name> </Name>\r\n<Val></Val>\r\n</String>\r\n<String>\r\n<Name> </Name>\r\n<Val></Val>\r\n</String>\r\n<String>\r\n<Name> </Name>\r\n<Val></Val>\r\n</String>\r\n<String>\r\n<Name> </Name>\r\n<Val></Val>\r\n</String>\r\n<String>\r\n<Name> </Name>\r\n<Val></Val>\r\n</String>\r\n<String>\r\n<Name> </Name>\r\n<Val></Val>\r\n</String>\r\n<String>\r\n<Name> </Name>\r\n<Val>Quadpack 4, MT  1, OPM channel index    0</Val>\r\n</String>\r\n<String>\r\n<Name> </Name>\r\n<Val></Val>\r\n</String>\r\n<String>\r\n<Name> </Name>\r\n<Val>Begin Sequence: Test Outputs from One MT\n\n\r(D:\\Program Files\\TMS\\Working TPS\\SN16K\\Gsc\\Gsc-MC\\SN16K GSC-MC Full (Fixed Pad).seq)</Val>\r\n</String>\r\n<String>\r\n<Name> </Name>\r\n<Val></Val>\r\n</String>\r\n<String>\r\n<Name> </Name>\r\n<Val></Val>\r\n</String>\r\n<String>\r\n<Name> </Name>\r\n<Val>Quadpack 4, MT  2, OPM channel index    0</Val>\r\n</String>\r\n<String>\r\n<Name> </Name>\r\n<Val></Val>\r\n</String>\r\n<String>\r\n<Name> </Name>\r\n<Val></Val>\r\n</String>\r\n<String>\r\n<Name> </Name>\r\n<Val></Val>\r\n</String>\r\n<String>\r\n<Name> </Name>\r\n<Val></Val>\r\n</String>\r\n<String>\r\n<Name> </Name>\r\n<Val></Val>\r\n</String>\r\n<String>\r\n<Name> </Name>\r\n<Val></Val>\r\n</String>\r\n<String>\r\n<Name> </Name>\r\n<Val>Quadpack 4, MT  2, OPM channel index    0</Val>\r\n</String>\r\n<String>\r\n<Name> </Name>\r\n<Val></Val>\r\n</String>\r\n<String>\r\n<Name> </Name>\r\n<Val>Begin Sequence: Test Outputs from One MT\n\n\r(D:\\Program Files\\TMS\\Working TPS\\SN16K\\Gsc\\Gsc-MC\\SN16K GSC-MC Full (Fixed Pad).seq)</Val>\r\n</String>\r\n<String>\r\n<Name> </Name>\r\n<Val></Val>\r\n</String>\r\n<String>\r\n<Name> </Name>\r\n<Val></Val>\r\n</String>\r\n<String>\r\n<Name> </Name>\r\n<Val>Quadpack 4, MT  3, OPM channel index    0</Val>\r\n</String>\r\n<String>\r\n<Name> </Name>\r\n<Val></Val>\r\n</String>\r\n<String>\r\n<Name> </Name>\r\n<Val></Val>\r\n</String>\r\n<String>\r\n<Name> </Name>\r\n<Val></Val>\r\n</String>\r\n<String>\r\n<Name> </Name>\r\n<Val></Val>\r\n</String>\r\n<String>\r\n<Name> </Name>\r\n<Val></Val>\r\n</String>\r\n<String>\r\n<Name> </Name>\r\n<Val></Val>\r\n</String>\r\n<String>\r\n<Name> </Name>\r\n<Val>Quadpack 4, MT  3, OPM channel index    0</Val>\r\n</String>\r\n<String>\r\n<Name> </Name>\r\n<Val></Val>\r\n</String>\r\n<String>\r\n<Name> </Name>\r\n<Val>Begin Sequence: Test Outputs from One MT\n\n\r(D:\\Program Files\\TMS\\Working TPS\\SN16K\\Gsc\\Gsc-MC\\SN16K GSC-MC Full (Fixed Pad).seq)</Val>\r\n</String>\r\n<String>\r\n<Name> </Name>\r\n<Val></Val>\r\n</String>\r\n<String>\r\n<Name> </Name>\r\n<Val></Val>\r\n</String>\r\n<String>\r\n<Name> </Name>\r\n<Val>Quadpack 4, MT  4, OPM channel index    0</Val>\r\n</String>\r\n<String>\r\n<Name> </Name>\r\n<Val></Val>\r\n</String>\r\n<String>\r\n<Name> </Name>\r\n<Val></Val>\r\n</String>\r\n<String>\r\n<Name> </Name>\r\n<Val></Val>\r\n</String>\r\n<String>\r\n<Name> </Name>\r\n<Val></Val>\r\n</String>\r\n<String>\r\n<Name> </Name>\r\n<Val></Val>\r\n</String>\r\n<String>\r\n<Name> </Name>\r\n<Val></Val>\r\n</String>\r\n<String>\r\n<Name> </Name>\r\n<Val>Quadpack 4, MT  4, OPM channel index    0</Val>\r\n</String>\r\n<String>\r\n<Name> </Name>\r\n<Val></Val>\r\n</String>\r\n<String>\r\n<Name> </Name>\r\n<Val></Val>\r\n</String>\r\n<String>\r\n<Name> </Name>\r\n<Val>Begin Sequence: Setup for PRBS\n\n\r(D:\\Program Files\\TMS\\Working TPS\\SN16K\\Gsc\\Gsc-MC\\SN16K GSC-MC Full (Fixed Pad).seq)</Val>\r\n</String>\r\n<String>\r\n<Name> </Name>\r\n<Val></Val>\r\n</String>\r\n<String>\r\n<Name> </Name>\r\n<Val></Val>\r\n</String>\r\n<String>\r\n<Name> </Name>\r\n<Val></Val>\r\n</String>\r\n<String>\r\n<Name> </Name>\r\n<Val></Val>\r\n</String>\r\n<String>\r\n<Name> </Name>\r\n<Val></Val>\r\n</String>\r\n<String>\r\n<Name> </Name>\r\n<Val></Val>\r\n</String>\r\n<String>\r\n<Name> </Name>\r\n<Val></Val>\r\n</String>\r\n<String>\r\n<Name> </Name>\r\n<Val></Val>\r\n</String>\r\n<String>\r\n<Name> </Name>\r\n<Val></Val>\r\n</String>\r\n<String>\r\n<Name> </Name>\r\n<Val></Val>\r\n</String>\r\n<String>\r\n<Name> </Name>\r\n<Val></Val>\r\n</String>\r\n<String>\r\n<Name> </Name>\r\n<Val></Val>\r\n</String>\r\n<String>\r\n<Name> </Name>\r\n<Val></Val>\r\n</String>\r\n<String>\r\n<Name> </Name>\r\n<Val></Val>\r\n</String>\r\n<String>\r\n<Name> </Name>\r\n<Val></Val>\r\n</String>\r\n<String>\r\n<Name> </Name>\r\n<Val></Val>\r\n</String>\r\n<String>\r\n<Name> </Name>\r\n<Val></Val>\r\n</String>\r\n<String>\r\n<Name> </Name>\r\n<Val></Val>\r\n</String>\r\n<String>\r\n<Name> </Name>\r\n<Val></Val>\r\n</String>\r\n<String>\r\n<Name> </Name>\r\n<Val></Val>\r\n</String>\r\n<String>\r\n<Name> </Name>\r\n<Val></Val>\r\n</String>\r\n<String>\r\n<Name> </Name>\r\n<Val></Val>\r\n</String>\r\n<String>\r\n<Name> </Name>\r\n<Val></Val>\r\n</String>\r\n<String>\r\n<Name> </Name>\r\n<Val></Val>\r\n</String>\r\n<String>\r\n<Name> </Name>\r\n<Val>Begin Sequence: Test Optical Shuffle Connections\n\n\r(D:\\Program Files\\TMS\\Working TPS\\SN16K\\Gsc\\Gsc-MC\\SN16K GSC-MC Full (Fixed Pad).seq)</Val>\r\n</String>\r\n<String>\r\n<Name> </Name>\r\n<Val></Val>\r\n</String>\r\n<String>\r\n<Name> </Name>\r\n<Val></Val>\r\n</String>\r\n<String>\r\n<Name> </Name>\r\n<Val></Val>\r\n</String>\r\n<String>\r\n<Name> </Name>\r\n<Val></Val>\r\n</String>\r\n<String>\r\n<Name> </Name>\r\n<Val></Val>\r\n</String>\r\n<String>\r\n<Name> </Name>\r\n<Val></Val>\r\n</String>\r\n<String>\r\n<Name> </Name>\r\n<Val></Val>\r\n</String>\r\n<String>\r\n<Name> </Name>\r\n<Val></Val>\r\n</String>\r\n<String>\r\n<Name> </Name>\r\n<Val></Val>\r\n</String>\r\n<String>\r\n<Name> </Name>\r\n<Val>Quadpack A</Val>\r\n</String>\r\n<String>\r\n<Name> </Name>\r\n<Val>Quadpack A</Val>\r\n</String>\r\n<String>\r\n<Name> </Name>\r\n<Val>Quadpack A</Val>\r\n</String>\r\n<String>\r\n<Name> </Name>\r\n<Val></Val>\r\n</String>\r\n<String>\r\n<Name> </Name>\r\n<Val>Quadpack B</Val>\r\n</String>\r\n<String>\r\n<Name> </Name>\r\n<Val>Quadpack B</Val>\r\n</String>\r\n<String>\r\n<Name> </Name>\r\n<Val>Quadpack B</Val>\r\n</String>\r\n<String>\r\n<Name> </Name>\r\n<Val></Val>\r\n</String>\r\n<String>\r\n<Name> </Name>\r\n<Val>Quadpack C</Val>\r\n</String>\r\n<String>\r\n<Name> </Name>\r\n<Val>Quadpack C</Val>\r\n</String>\r\n<String>\r\n<Name> </Name>\r\n<Val>Quadpack C</Val>\r\n</String>\r\n<String>\r\n<Name> </Name>\r\n<Val></Val>\r\n</String>\r\n<String>\r\n<Name> </Name>\r\n<Val>Quadpack D</Val>\r\n</String>\r\n<String>\r\n<Name> </Name>\r\n<Val>Quadpack D</Val>\r\n</String>\r\n<String>\r\n<Name> </Name>\r\n<Val>Quadpack D</Val>\r\n</String>\r\n<String>\r\n<Name> </Name>\r\n<Val>Begin Sequence: Receive Sensitivity Tests\n\n\r(D:\\Program Files\\TMS\\Working TPS\\SN16K\\Gsc\\Gsc-MC\\SN16K GSC-MC Full (Fixed Pad).seq)</Val>\r\n</String>\r\n<String>\r\n<Name> </Name>\r\n<Val></Val>\r\n</String>\r\n<String>\r\n<Name> </Name>\r\n<Val>Begin Sequence: Scan Fixed Pad Serial Numbers\n\n\r(D:\\Program Files\\TMS\\Working TPS\\SN16K\\SN16K Common Sequences.seq)</Val>\r\n</String>\r\n<String>\r\n<Name> </Name>\r\n<Val>Quadpack A     MT1-2:    4304-2468\n\rQuadpack A     MT3-4:    2804-2417\n\rQuadpack B     MT1-2:    4304-2443\n\rQuadpack B     MT3-4:    4304-2435\n\rQuadpack C     MT1-2:    2205-1249\n\rQuadpack C     MT3-4:    2205-1247\n\rQuadpack D     MT1-2:    4304-2460\n\rQuadpack D     MT3-4:    4304-2437</Val>\r\n</String>\r\n<String>\r\n<Name> </Name>\r\n<Val>Begin Sequence: Setup for PRBS\n\n\r(D:\\Program Files\\TMS\\Working TPS\\SN16K\\Gsc\\Gsc-MC\\SN16K GSC-MC Full (Fixed Pad).seq)</Val>\r\n</String>\r\n<String>\r\n<Name> </Name>\r\n<Val></Val>\r\n</String>\r\n<String>\r\n<Name> </Name>\r\n<Val></Val>\r\n</String>\r\n<String>\r\n<Name> </Name>\r\n<Val></Val>\r\n</String>\r\n<String>\r\n<Name> </Name>\r\n<Val></Val>\r\n</String>\r\n<String>\r\n<Name> </Name>\r\n<Val></Val>\r\n</String>\r\n<String>\r\n<Name> </Name>\r\n<Val></Val>\r\n</String>\r\n<String>\r\n<Name> </Name>\r\n<Val></Val>\r\n</String>\r\n<String>\r\n<Name> </Name>\r\n<Val></Val>\r\n</String>\r\n<String>\r\n<Name> </Name>\r\n<Val></Val>\r\n</String>\r\n<String>\r\n<Name> </Name>\r\n<Val></Val>\r\n</String>\r\n<String>\r\n<Name> </Name>\r\n<Val></Val>\r\n</String>\r\n<String>\r\n<Name> </Name>\r\n<Val></Val>\r\n</String>\r\n<String>\r\n<Name> </Name>\r\n<Val>Begin Sequence: Rx Sensitivity, SW A Ports 0 - 63 and SW B Ports 0 - 63\n\n\r(D:\\Program Files\\TMS\\Working TPS\\SN16K\\Gsc\\Gsc-MC\\SN16K GSC-MC Full (Fixed Pad).seq)</Val>\r\n</String>\r\n<String>\r\n<Name> </Name>\r\n<Val></Val>\r\n</String>\r\n<String>\r\n<Name> </Name>\r\n<Val></Val>\r\n</String>\r\n<String>\r\n<Name> </Name>\r\n<Val></Val>\r\n</String>\r\n<String>\r\n<Name> </Name>\r\n<Val></Val>\r\n</String>\r\n<String>\r\n<Name> </Name>\r\n<Val></Val>\r\n</String>\r\n<String>\r\n<Name> </Name>\r\n<Val></Val>\r\n</String>\r\n<String>\r\n<Name> </Name>\r\n<Val></Val>\r\n</String>\r\n<String>\r\n<Name> </Name>\r\n<Val></Val>\r\n</String>\r\n<String>\r\n<Name> </Name>\r\n<Val></Val>\r\n</String>\r\n<String>\r\n<Name> </Name>\r\n<Val></Val>\r\n</String>\r\n<String>\r\n<Name> </Name>\r\n<Val></Val>\r\n</String>\r\n<String>\r\n<Name> </Name>\r\n<Val></Val>\r\n</String>\r\n<String>\r\n<Name> </Name>\r\n<Val></Val>\r\n</String>\r\n<String>\r\n<Name> </Name>\r\n<Val></Val>\r\n</String>\r\n<String>\r\n<Name> </Name>\r\n<Val></Val>\r\n</String>\r\n<String>\r\n<Name> </Name>\r\n<Val></Val>\r\n</String>\r\n<String>\r\n<Name> </Name>\r\n<Val></Val>\r\n</String>\r\n<String>\r\n<Name> </Name>\r\n<Val></Val>\r\n</String>\r\n<String>\r\n<Name> </Name>\r\n<Val></Val>\r\n</String>\r\n<String>\r\n<Name> </Name>\r\n<Val></Val>\r\n</String>\r\n<String>\r\n<Name> </Name>\r\n<Val></Val>\r\n</String>\r\n<String>\r\n<Name> </Name>\r\n<Val></Val>\r\n</String>\r\n<String>\r\n<Name> </Name>\r\n<Val></Val>\r\n</String>\r\n<String>\r\n<Name> </Name>\r\n<Val></Val>\r\n</String>\r\n<String>\r\n<Name> </Name>\r\n<Val></Val>\r\n</String>\r\n<String>\r\n<Name> </Name>\r\n<Val></Val>\r\n</String>\r\n<String>\r\n<Name> </Name>\r\n<Val></Val>\r\n</String>\r\n<String>\r\n<Name> </Name>\r\n<Val></Val>\r\n</String>\r\n<String>\r\n<Name> </Name>\r\n<Val></Val>\r\n</String>\r\n<String>\r\n<Name> </Name>\r\n<Val></Val>\r\n</String>\r\n<String>\r\n<Name> </Name>\r\n<Val></Val>\r\n</String>\r\n<String>\r\n<Name> </Name>\r\n<Val></Val>\r\n</String>\r\n<String>\r\n<Name> </Name>\r\n<Val></Val>\r\n</String>\r\n<String>\r\n<Name> </Name>\r\n<Val></Val>\r\n</String>\r\n<String>\r\n<Name> </Name>\r\n<Val></Val>\r\n</String>\r\n<String>\r\n<Name> </Name>\r\n<Val></Val>\r\n</String>\r\n<String>\r\n<Name> </Name>\r\n<Val></Val>\r\n</String>\r\n<String>\r\n<Name> </Name>\r\n<Val></Val>\r\n</String>\r\n<String>\r\n<Name> </Name>\r\n<Val></Val>\r\n</String>\r\n<String>\r\n<Name> </Name>\r\n<Val></Val>\r\n</String>\r\n<String>\r\n<Name> </Name>\r\n<Val></Val>\r\n</String>\r\n<String>\r\n<Name> </Name>\r\n<Val></Val>\r\n</String>\r\n<String>\r\n<Name> </Name>\r\n<Val></Val>\r\n</String>\r\n<String>\r\n<Name> </Name>\r\n<Val></Val>\r\n</String>\r\n<String>\r\n<Name> </Name>\r\n<Val></Val>\r\n</String>\r\n<String>\r\n<Name> </Name>\r\n<Val></Val>\r\n</String>\r\n<String>\r\n<Name> </Name>\r\n<Val></Val>\r\n</String>\r\n<String>\r\n<Name> </Name>\r\n<Val></Val>\r\n</String>\r\n<String>\r\n<Name> </Name>\r\n<Val></Val>\r\n</String>\r\n<String>\r\n<Name> </Name>\r\n<Val></Val>\r\n</String>\r\n<String>\r\n<Name> </Name>\r\n<Val></Val>\r\n</String>\r\n<String>\r\n<Name> </Name>\r\n<Val></Val>\r\n</String>\r\n<String>\r\n<Name> </Name>\r\n<Val></Val>\r\n</String>\r\n<String>\r\n<Name> </Name>\r\n<Val></Val>\r\n</String>\r\n<String>\r\n<Name> </Name>\r\n<Val></Val>\r\n</String>\r\n<String>\r\n<Name> </Name>\r\n<Val></Val>\r\n</String>\r\n<String>\r\n<Name> </Name>\r\n<Val></Val>\r\n</String>\r\n<String>\r\n<Name> </Name>\r\n<Val></Val>\r\n</String>\r\n<String>\r\n<Name> </Name>\r\n<Val></Val>\r\n</String>\r\n<String>\r\n<Name> </Name>\r\n<Val></Val>\r\n</String>\r\n<String>\r\n<Name> </Name>\r\n<Val></Val>\r\n</String>\r\n<String>\r\n<Name> </Name>\r\n<Val></Val>\r\n</String>\r\n<String>\r\n<Name> </Name>\r\n<Val></Val>\r\n</String>\r\n<String>\r\n<Name> </Name>\r\n<Val></Val>\r\n</String>\r\n<String>\r\n<Name> </Name>\r\n<Val></Val>\r\n</String>\r\n<String>\r\n<Name> </Name>\r\n<Val></Val>\r\n</String>\r\n<String>\r\n<Name> </Name>\r\n<Val></Val>\r\n</String>\r\n<String>\r\n<Name> </Name>\r\n<Val></Val>\r\n</String>\r\n<String>\r\n<Name> </Name>\r\n<Val></Val>\r\n</String>\r\n<String>\r\n<Name> </Name>\r\n<Val></Val>\r\n</String>\r\n<String>\r\n<Name> </Name>\r\n<Val></Val>\r\n</String>\r\n<String>\r\n<Name> </Name>\r\n<Val></Val>\r\n</String>\r\n<String>\r\n<Name> </Name>\r\n<Val></Val>\r\n</String>\r\n<String>\r\n<Name> </Name>\r\n<Val></Val>\r\n</String>\r\n<String>\r\n<Name> </Name>\r\n<Val></Val>\r\n</String>\r\n<String>\r\n<Name> </Name>\r\n<Val></Val>\r\n</String>\r\n<String>\r\n<Name> </Name>\r\n<Val></Val>\r\n</String>\r\n<String>\r\n<Name> </Name>\r\n<Val></Val>\r\n</String>\r\n<String>\r\n<Name> </Name>\r\n<Val></Val>\r\n</String>\r\n<String>\r\n<Name> </Name>\r\n<Val></Val>\r\n</String>\r\n<String>\r\n<Name> </Name>\r\n<Val></Val>\r\n</String>\r\n<String>\r\n<Name> </Name>\r\n<Val></Val>\r\n</String>\r\n<String>\r\n<Name> </Name>\r\n<Val></Val>\r\n</String>\r\n<String>\r\n<Name> </Name>\r\n<Val></Val>\r\n</String>\r\n<String>\r\n<Name> </Name>\r\n<Val></Val>\r\n</String>\r\n<String>\r\n<Name> </Name>\r\n<Val></Val>\r\n</String>\r\n<String>\r\n<Name> </Name>\r\n<Val></Val>\r\n</String>\r\n<String>\r\n<Name> </Name>\r\n<Val></Val>\r\n</String>\r\n<String>\r\n<Name> </Name>\r\n<Val></Val>\r\n</String>\r\n<String>\r\n<Name> </Name>\r\n<Val></Val>\r\n</String>\r\n<String>\r\n<Name> </Name>\r\n<Val></Val>\r\n</String>\r\n<String>\r\n<Name> </Name>\r\n<Val></Val>\r\n</String>\r\n<String>\r\n<Name> </Name>\r\n<Val></Val>\r\n</String>\r\n<String>\r\n<Name> </Name>\r\n<Val></Val>\r\n</String>\r\n<String>\r\n<Name> </Name>\r\n<Val></Val>\r\n</String>\r\n<String>\r\n<Name> </Name>\r\n<Val></Val>\r\n</String>\r\n<String>\r\n<Name> </Name>\r\n<Val></Val>\r\n</String>\r\n<String>\r\n<Name> </Name>\r\n<Val></Val>\r\n</String>\r\n<String>\r\n<Name> </Name>\r\n<Val></Val>\r\n</String>\r\n<String>\r\n<Name> </Name>\r\n<Val></Val>\r\n</String>\r\n<String>\r\n<Name> </Name>\r\n<Val></Val>\r\n</String>\r\n<String>\r\n<Name> </Name>\r\n<Val></Val>\r\n</String>\r\n<String>\r\n<Name> </Name>\r\n<Val></Val>\r\n</String>\r\n<String>\r\n<Name> </Name>\r\n<Val></Val>\r\n</String>\r\n<String>\r\n<Name> </Name>\r\n<Val></Val>\r\n</String>\r\n<String>\r\n<Name> </Name>\r\n<Val></Val>\r\n</String>\r\n<String>\r\n<Name> </Name>\r\n<Val></Val>\r\n</String>\r\n<String>\r\n<Name> </Name>\r\n<Val></Val>\r\n</String>\r\n<String>\r\n<Name> </Name>\r\n<Val></Val>\r\n</String>\r\n<String>\r\n<Name> </Name>\r\n<Val></Val>\r\n</String>\r\n<String>\r\n<Name> </Name>\r\n<Val></Val>\r\n</String>\r\n<String>\r\n<Name> </Name>\r\n<Val></Val>\r\n</String>\r\n<String>\r\n<Name> </Name>\r\n<Val></Val>\r\n</String>\r\n<String>\r\n<Name> </Name>\r\n<Val></Val>\r\n</String>\r\n<String>\r\n<Name> </Name>\r\n<Val></Val>\r\n</String>\r\n<String>\r\n<Name> </Name>\r\n<Val></Val>\r\n</String>\r\n<String>\r\n<Name> </Name>\r\n<Val></Val>\r\n</String>\r\n<String>\r\n<Name> </Name>\r\n<Val></Val>\r\n</String>\r\n<String>\r\n<Name> </Name>\r\n<Val></Val>\r\n</String>\r\n<String>\r\n<Name> </Name>\r\n<Val></Val>\r\n</String>\r\n<String>\r\n<Name> </Name>\r\n<Val></Val>\r\n</String>\r\n<String>\r\n<Name> </Name>\r\n<Val></Val>\r\n</String>\r\n<String>\r\n<Name> </Name>\r\n<Val></Val>\r\n</String>\r\n<String>\r\n<Name> </Name>\r\n<Val></Val>\r\n</String>\r\n<String>\r\n<Name> </Name>\r\n<Val></Val>\r\n</String>\r\n<String>\r\n<Name> </Name>\r\n<Val></Val>\r\n</String>\r\n<String>\r\n<Name> </Name>\r\n<Val></Val>\r\n</String>\r\n<String>\r\n<Name> </Name>\r\n<Val></Val>\r\n</String>\r\n<String>\r\n<Name> </Name>\r\n<Val></Val>\r\n</String>\r\n<String>\r\n<Name> </Name>\r\n<Val></Val>\r\n</String>\r\n<String>\r\n<Name> </Name>\r\n<Val></Val>\r\n</String>\r\n<String>\r\n<Name> </Name>\r\n<Val></Val>\r\n</String>\r\n<String>\r\n<Name> </Name>\r\n<Val></Val>\r\n</String>\r\n<String>\r\n<Name> </Name>\r\n<Val></Val>\r\n</String>\r\n<String>\r\n<Name> </Name>\r\n<Val></Val>\r\n</String>\r\n<String>\r\n<Name> </Name>\r\n<Val></Val>\r\n</String>\r\n<String>\r\n<Name> </Name>\r\n<Val></Val>\r\n</String>\r\n<String>\r\n<Name> </Name>\r\n<Val></Val>\r\n</String>\r\n<String>\r\n<Name> </Name>\r\n<Val></Val>\r\n</String>\r\n<String>\r\n<Name> </Name>\r\n<Val></Val>\r\n</String>\r\n<String>\r\n<Name> </Name>\r\n<Val></Val>\r\n</String>\r\n<String>\r\n<Name> </Name>\r\n<Val></Val>\r\n</String>\r\n<String>\r\n<Name> </Name>\r\n<Val></Val>\r\n</String>\r\n<String>\r\n<Name> </Name>\r\n<Val></Val>\r\n</String>\r\n<String>\r\n<Name> </Name>\r\n<Val></Val>\r\n</String>\r\n<String>\r\n<Name> </Name>\r\n<Val></Val>\r\n</String>\r\n<String>\r\n<Name> </Name>\r\n<Val></Val>\r\n</String>\r\n<String>\r\n<Name> </Name>\r\n<Val></Val>\r\n</String>\r\n<String>\r\n<Name> </Name>\r\n<Val></Val>\r\n</String>\r\n<String>\r\n<Name> </Name>\r\n<Val></Val>\r\n</String>\r\n<String>\r\n<Name> </Name>\r\n<Val></Val>\r\n</String>\r\n<String>\r\n<Name> </Name>\r\n<Val></Val>\r\n</String>\r\n<String>\r\n<Name> </Name>\r\n<Val></Val>\r\n</String>\r\n<String>\r\n<Name> </Name>\r\n<Val></Val>\r\n</String>\r\n<String>\r\n<Name> </Name>\r\n<Val></Val>\r\n</String>\r\n<String>\r\n<Name> </Name>\r\n<Val></Val>\r\n</String>\r\n<String>\r\n<Name> </Name>\r\n<Val></Val>\r\n</String>\r\n<String>\r\n<Name> </Name>\r\n<Val></Val>\r\n</String>\r\n<String>\r\n<Name> </Name>\r\n<Val></Val>\r\n</String>\r\n<String>\r\n<Name> </Name>\r\n<Val></Val>\r\n</String>\r\n<String>\r\n<Name> </Name>\r\n<Val></Val>\r\n</String>\r\n<String>\r\n<Name> </Name>\r\n<Val></Val>\r\n</String>\r\n<String>\r\n<Name> </Name>\r\n<Val></Val>\r\n</String>\r\n<String>\r\n<Name> </Name>\r\n<Val></Val>\r\n</String>\r\n<String>\r\n<Name> </Name>\r\n<Val></Val>\r\n</String>\r\n<String>\r\n<Name> </Name>\r\n<Val></Val>\r\n</String>\r\n<String>\r\n<Name> </Name>\r\n<Val></Val>\r\n</String>\r\n<String>\r\n<Name> </Name>\r\n<Val></Val>\r\n</String>\r\n<String>\r\n<Name> </Name>\r\n<Val></Val>\r\n</String>\r\n<String>\r\n<Name> </Name>\r\n<Val></Val>\r\n</String>\r\n<String>\r\n<Name> </Name>\r\n<Val></Val>\r\n</String>\r\n<String>\r\n<Name> </Name>\r\n<Val></Val>\r\n</String>\r\n<String>\r\n<Name> </Name>\r\n<Val></Val>\r\n</String>\r\n<String>\r\n<Name> </Name>\r\n<Val></Val>\r\n</String>\r\n<String>\r\n<Name> </Name>\r\n<Val></Val>\r\n</String>\r\n<String>\r\n<Name> </Name>\r\n<Val></Val>\r\n</String>\r\n<String>\r\n<Name> </Name>\r\n<Val></Val>\r\n</String>\r\n<String>\r\n<Name> </Name>\r\n<Val></Val>\r\n</String>\r\n<String>\r\n<Name> </Name>\r\n<Val></Val>\r\n</String>\r\n<String>\r\n<Name> </Name>\r\n<Val></Val>\r\n</String>\r\n<String>\r\n<Name> </Name>\r\n<Val></Val>\r\n</String>\r\n<String>\r\n<Name> </Name>\r\n<Val></Val>\r\n</String>\r\n<String>\r\n<Name> </Name>\r\n<Val></Val>\r\n</String>\r\n<String>\r\n<Name> </Name>\r\n<Val></Val>\r\n</String>\r\n<String>\r\n<Name> </Name>\r\n<Val></Val>\r\n</String>\r\n<String>\r\n<Name> </Name>\r\n<Val></Val>\r\n</String>\r\n<String>\r\n<Name> </Name>\r\n<Val></Val>\r\n</String>\r\n<String>\r\n<Name> </Name>\r\n<Val></Val>\r\n</String>\r\n<String>\r\n<Name> </Name>\r\n<Val></Val>\r\n</String>\r\n<String>\r\n<Name> </Name>\r\n<Val></Val>\r\n</String>\r\n<String>\r\n<Name> </Name>\r\n<Val></Val>\r\n</String>\r\n<String>\r\n<Name> </Name>\r\n<Val></Val>\r\n</String>\r\n<String>\r\n<Name> </Name>\r\n<Val></Val>\r\n</String>\r\n<String>\r\n<Name> </Name>\r\n<Val></Val>\r\n</String>\r\n<String>\r\n<Name> </Name>\r\n<Val></Val>\r\n</String>\r\n<String>\r\n<Name> </Name>\r\n<Val></Val>\r\n</String>\r\n<String>\r\n<Name> </Name>\r\n<Val></Val>\r\n</String>\r\n<String>\r\n<Name> </Name>\r\n<Val></Val>\r\n</String>\r\n<String>\r\n<Name> </Name>\r\n<Val></Val>\r\n</String>\r\n<String>\r\n<Name> </Name>\r\n<Val></Val>\r\n</String>\r\n<String>\r\n<Name> </Name>\r\n<Val></Val>\r\n</String>\r\n<String>\r\n<Name> </Name>\r\n<Val></Val>\r\n</String>\r\n<String>\r\n<Name> </Name>\r\n<Val></Val>\r\n</String>\r\n<String>\r\n<Name> </Name>\r\n<Val></Val>\r\n</String>\r\n<String>\r\n<Name> </Name>\r\n<Val></Val>\r\n</String>\r\n<String>\r\n<Name> </Name>\r\n<Val></Val>\r\n</String>\r\n<String>\r\n<Name> </Name>\r\n<Val></Val>\r\n</String>\r\n<String>\r\n<Name> </Name>\r\n<Val></Val>\r\n</String>\r\n<String>\r\n<Name> </Name>\r\n<Val></Val>\r\n</String>\r\n<String>\r\n<Name> </Name>\r\n<Val></Val>\r\n</String>\r\n<String>\r\n<Name> </Name>\r\n<Val></Val>\r\n</String>\r\n<String>\r\n<Name> </Name>\r\n<Val></Val>\r\n</String>\r\n<String>\r\n<Name> </Name>\r\n<Val></Val>\r\n</String>\r\n<String>\r\n<Name> </Name>\r\n<Val></Val>\r\n</String>\r\n<String>\r\n<Name> </Name>\r\n<Val></Val>\r\n</String>\r\n<String>\r\n<Name> </Name>\r\n<Val></Val>\r\n</String>\r\n<String>\r\n<Name> </Name>\r\n<Val></Val>\r\n</String>\r\n<String>\r\n<Name> </Name>\r\n<Val></Val>\r\n</String>\r\n<String>\r\n<Name> </Name>\r\n<Val></Val>\r\n</String>\r\n<String>\r\n<Name> </Name>\r\n<Val></Val>\r\n</String>\r\n<String>\r\n<Name> </Name>\r\n<Val></Val>\r\n</String>\r\n<String>\r\n<Name> </Name>\r\n<Val></Val>\r\n</String>\r\n<String>\r\n<Name> </Name>\r\n<Val></Val>\r\n</String>\r\n<String>\r\n<Name> </Name>\r\n<Val></Val>\r\n</String>\r\n<String>\r\n<Name> </Name>\r\n<Val></Val>\r\n</String>\r\n<String>\r\n<Name> </Name>\r\n<Val></Val>\r\n</String>\r\n<String>\r\n<Name> </Name>\r\n<Val></Val>\r\n</String>\r\n<String>\r\n<Name> </Name>\r\n<Val></Val>\r\n</String>\r\n<String>\r\n<Name> </Name>\r\n<Val></Val>\r\n</String>\r\n<String>\r\n<Name> </Name>\r\n<Val></Val>\r\n</String>\r\n<String>\r\n<Name> </Name>\r\n<Val></Val>\r\n</String>\r\n<String>\r\n<Name> </Name>\r\n<Val></Val>\r\n</String>\r\n<String>\r\n<Name> </Name>\r\n<Val></Val>\r\n</String>\r\n<String>\r\n<Name> </Name>\r\n<Val></Val>\r\n</String>\r\n<String>\r\n<Name> </Name>\r\n<Val></Val>\r\n</String>\r\n<String>\r\n<Name> </Name>\r\n<Val></Val>\r\n</String>\r\n<String>\r\n<Name> </Name>\r\n<Val></Val>\r\n</String>\r\n<String>\r\n<Name> </Name>\r\n<Val></Val>\r\n</String>\r\n<String>\r\n<Name> </Name>\r\n<Val></Val>\r\n</String>\r\n<String>\r\n<Name> </Name>\r\n<Val></Val>\r\n</String>\r\n<String>\r\n<Name> </Name>\r\n<Val></Val>\r\n</String>\r\n<String>\r\n<Name> </Name>\r\n<Val></Val>\r\n</String>\r\n<String>\r\n<Name> </Name>\r\n<Val></Val>\r\n</String>\r\n<String>\r\n<Name> </Name>\r\n<Val></Val>\r\n</String>\r\n<String>\r\n<Name> </Name>\r\n<Val></Val>\r\n</String>\r\n<String>\r\n<Name> </Name>\r\n<Val></Val>\r\n</String>\r\n<String>\r\n<Name> </Name>\r\n<Val></Val>\r\n</String>\r\n<String>\r\n<Name> </Name>\r\n<Val></Val>\r\n</String>\r\n<String>\r\n<Name> </Name>\r\n<Val></Val>\r\n</String>\r\n<String>\r\n<Name> </Name>\r\n<Val></Val>\r\n</String>\r\n<String>\r\n<Name> </Name>\r\n<Val></Val>\r\n</String>\r\n<String>\r\n<Name> </Name>\r\n<Val></Val>\r\n</String>\r\n<String>\r\n<Name> </Name>\r\n<Val></Val>\r\n</String>\r\n<String>\r\n<Name> </Name>\r\n<Val></Val>\r\n</String>\r\n<String>\r\n<Name> </Name>\r\n<Val></Val>\r\n</String>\r\n<String>\r\n<Name> </Name>\r\n<Val></Val>\r\n</String>\r\n<String>\r\n<Name> </Name>\r\n<Val></Val>\r\n</String>\r\n<String>\r\n<Name> </Name>\r\n<Val></Val>\r\n</String>\r\n<String>\r\n<Name> </Name>\r\n<Val></Val>\r\n</String>\r\n<String>\r\n<Name> </Name>\r\n<Val></Val>\r\n</String>\r\n<String>\r\n<Name> </Name>\r\n<Val></Val>\r\n</String>\r\n<String>\r\n<Name> </Name>\r\n<Val></Val>\r\n</String>\r\n<String>\r\n<Name> </Name>\r\n<Val></Val>\r\n</String>\r\n<String>\r\n<Name> </Name>\r\n<Val></Val>\r\n</String>\r\n<String>\r\n<Name> </Name>\r\n<Val></Val>\r\n</String>\r\n<String>\r\n<Name> </Name>\r\n<Val></Val>\r\n</String>\r\n<String>\r\n<Name> </Name>\r\n<Val></Val>\r\n</String>\r\n<String>\r\n<Name> </Name>\r\n<Val></Val>\r\n</String>\r\n<String>\r\n<Name> </Name>\r\n<Val></Val>\r\n</String>\r\n<String>\r\n<Name> </Name>\r\n<Val></Val>\r\n</String>\r\n<String>\r\n<Name> </Name>\r\n<Val></Val>\r\n</String>\r\n<String>\r\n<Name> </Name>\r\n<Val></Val>\r\n</String>\r\n<String>\r\n<Name> </Name>\r\n<Val></Val>\r\n</String>\r\n<String>\r\n<Name> </Name>\r\n<Val></Val>\r\n</String>\r\n<String>\r\n<Name> </Name>\r\n<Val></Val>\r\n</String>\r\n<String>\r\n<Name> </Name>\r\n<Val></Val>\r\n</String>\r\n<String>\r\n<Name> </Name>\r\n<Val></Val>\r\n</String>\r\n<String>\r\n<Name> </Name>\r\n<Val></Val>\r\n</String>\r\n<String>\r\n<Name> </Name>\r\n<Val></Val>\r\n</String>\r\n<String>\r\n<Name> </Name>\r\n<Val></Val>\r\n</String>\r\n<String>\r\n<Name> </Name>\r\n<Val></Val>\r\n</String>\r\n<String>\r\n<Name> </Name>\r\n<Val></Val>\r\n</String>\r\n<String>\r\n<Name> </Name>\r\n<Val></Val>\r\n</String>\r\n<String>\r\n<Name> </Name>\r\n<Val></Val>\r\n</String>\r\n<String>\r\n<Name> </Name>\r\n<Val></Val>\r\n</String>\r\n<String>\r\n<Name> </Name>\r\n<Val></Val>\r\n</String>\r\n<String>\r\n<Name> </Name>\r\n<Val></Val>\r\n</String>\r\n<String>\r\n<Name> </Name>\r\n<Val></Val>\r\n</String>\r\n<String>\r\n<Name> </Name>\r\n<Val></Val>\r\n</String>\r\n<String>\r\n<Name> </Name>\r\n<Val></Val>\r\n</String>\r\n<String>\r\n<Name> </Name>\r\n<Val></Val>\r\n</String>\r\n<String>\r\n<Name> </Name>\r\n<Val></Val>\r\n</String>\r\n<String>\r\n<Name> </Name>\r\n<Val></Val>\r\n</String>\r\n<String>\r\n<Name> </Name>\r\n<Val></Val>\r\n</String>\r\n<String>\r\n<Name> </Name>\r\n<Val></Val>\r\n</String>\r\n<String>\r\n<Name> </Name>\r\n<Val></Val>\r\n</String>\r\n<String>\r\n<Name> </Name>\r\n<Val></Val>\r\n</String>\r\n<String>\r\n<Name> </Name>\r\n<Val></Val>\r\n</String>\r\n<String>\r\n<Name> </Name>\r\n<Val></Val>\r\n</String>\r\n<String>\r\n<Name> </Name>\r\n<Val></Val>\r\n</String>\r\n<String>\r\n<Name> </Name>\r\n<Val></Val>\r\n</String>\r\n<String>\r\n<Name> </Name>\r\n<Val></Val>\r\n</String>\r\n<String>\r\n<Name> </Name>\r\n<Val></Val>\r\n</String>\r\n<String>\r\n<Name> </Name>\r\n<Val></Val>\r\n</String>\r\n<String>\r\n<Name> </Name>\r\n<Val></Val>\r\n</String>\r\n<String>\r\n<Name> </Name>\r\n<Val></Val>\r\n</String>\r\n<String>\r\n<Name> </Name>\r\n<Val></Val>\r\n</String>\r\n<String>\r\n<Name> </Name>\r\n<Val></Val>\r\n</String>\r\n<String>\r\n<Name> </Name>\r\n<Val></Val>\r\n</String>\r\n<String>\r\n<Name> </Name>\r\n<Val></Val>\r\n</String>\r\n<String>\r\n<Name> </Name>\r\n<Val></Val>\r\n</String>\r\n<String>\r\n<Name> </Name>\r\n<Val></Val>\r\n</String>\r\n<String>\r\n<Name> </Name>\r\n<Val></Val>\r\n</String>\r\n<String>\r\n<Name> </Name>\r\n<Val></Val>\r\n</String>\r\n<String>\r\n<Name> </Name>\r\n<Val></Val>\r\n</String>\r\n<String>\r\n<Name> </Name>\r\n<Val></Val>\r\n</String>\r\n<String>\r\n<Name> </Name>\r\n<Val></Val>\r\n</String>\r\n<String>\r\n<Name> </Name>\r\n<Val></Val>\r\n</String>\r\n<String>\r\n<Name> </Name>\r\n<Val></Val>\r\n</String>\r\n<String>\r\n<Name> </Name>\r\n<Val></Val>\r\n</String>\r\n<String>\r\n<Name> </Name>\r\n<Val></Val>\r\n</String>\r\n<String>\r\n<Name> </Name>\r\n<Val></Val>\r\n</String>\r\n<String>\r\n<Name> </Name>\r\n<Val></Val>\r\n</String>\r\n<String>\r\n<Name> </Name>\r\n<Val></Val>\r\n</String>\r\n<String>\r\n<Name> </Name>\r\n<Val></Val>\r\n</String>\r\n<String>\r\n<Name> </Name>\r\n<Val></Val>\r\n</String>\r\n<String>\r\n<Name> </Name>\r\n<Val></Val>\r\n</String>\r\n<String>\r\n<Name> </Name>\r\n<Val></Val>\r\n</String>\r\n<String>\r\n<Name> </Name>\r\n<Val></Val>\r\n</String>\r\n<String>\r\n<Name> </Name>\r\n<Val></Val>\r\n</String>\r\n<String>\r\n<Name> </Name>\r\n<Val></Val>\r\n</String>\r\n<String>\r\n<Name> </Name>\r\n<Val></Val>\r\n</String>\r\n<String>\r\n<Name> </Name>\r\n<Val></Val>\r\n</String>\r\n<String>\r\n<Name> </Name>\r\n<Val></Val>\r\n</String>\r\n<String>\r\n<Name> </Name>\r\n<Val></Val>\r\n</String>\r\n<String>\r\n<Name> </Name>\r\n<Val></Val>\r\n</String>\r\n<String>\r\n<Name> </Name>\r\n<Val></Val>\r\n</String>\r\n<String>\r\n<Name> </Name>\r\n<Val></Val>\r\n</String>\r\n<String>\r\n<Name> </Name>\r\n<Val></Val>\r\n</String>\r\n<String>\r\n<Name> </Name>\r\n<Val></Val>\r\n</String>\r\n<String>\r\n<Name> </Name>\r\n<Val></Val>\r\n</String>\r\n<String>\r\n<Name> </Name>\r\n<Val></Val>\r\n</String>\r\n<String>\r\n<Name> </Name>\r\n<Val></Val>\r\n</String>\r\n<String>\r\n<Name> </Name>\r\n<Val></Val>\r\n</String>\r\n<String>\r\n<Name> </Name>\r\n<Val></Val>\r\n</String>\r\n<String>\r\n<Name> </Name>\r\n<Val></Val>\r\n</String>\r\n<String>\r\n<Name> </Name>\r\n<Val></Val>\r\n</String>\r\n<String>\r\n<Name> </Name>\r\n<Val></Val>\r\n</String>\r\n<String>\r\n<Name> </Name>\r\n<Val></Val>\r\n</String>\r\n<String>\r\n<Name> </Name>\r\n<Val></Val>\r\n</String>\r\n<String>\r\n<Name> </Name>\r\n<Val></Val>\r\n</String>\r\n<String>\r\n<Name> </Name>\r\n<Val></Val>\r\n</String>\r\n<String>\r\n<Name> </Name>\r\n<Val></Val>\r\n</String>\r\n<String>\r\n<Name> </Name>\r\n<Val></Val>\r\n</String>\r\n<String>\r\n<Name> </Name>\r\n<Val></Val>\r\n</String>\r\n<String>\r\n<Name> </Name>\r\n<Val></Val>\r\n</String>\r\n<String>\r\n<Name> </Name>\r\n<Val></Val>\r\n</String>\r\n<String>\r\n<Name> </Name>\r\n<Val></Val>\r\n</String>\r\n<String>\r\n<Name> </Name>\r\n<Val></Val>\r\n</String>\r\n<String>\r\n<Name> </Name>\r\n<Val></Val>\r\n</String>\r\n<String>\r\n<Name> </Name>\r\n<Val></Val>\r\n</String>\r\n<String>\r\n<Name> </Name>\r\n<Val></Val>\r\n</String>\r\n<String>\r\n<Name> </Name>\r\n<Val></Val>\r\n</String>\r\n<String>\r\n<Name> </Name>\r\n<Val></Val>\r\n</String>\r\n<String>\r\n<Name> </Name>\r\n<Val></Val>\r\n</String>\r\n<String>\r\n<Name> </Name>\r\n<Val></Val>\r\n</String>\r\n<String>\r\n<Name> </Name>\r\n<Val></Val>\r\n</String>\r\n<String>\r\n<Name> </Name>\r\n<Val></Val>\r\n</String>\r\n<String>\r\n<Name> </Name>\r\n<Val></Val>\r\n</String>\r\n<String>\r\n<Name> </Name>\r\n<Val></Val>\r\n</String>\r\n<String>\r\n<Name> </Name>\r\n<Val></Val>\r\n</String>\r\n<String>\r\n<Name> </Name>\r\n<Val></Val>\r\n</String>\r\n<String>\r\n<Name> </Name>\r\n<Val></Val>\r\n</String>\r\n<String>\r\n<Name> </Name>\r\n<Val></Val>\r\n</String>\r\n<String>\r\n<Name> </Name>\r\n<Val></Val>\r\n</String>\r\n<String>\r\n<Name> </Name>\r\n<Val></Val>\r\n</String>\r\n<String>\r\n<Name> </Name>\r\n<Val></Val>\r\n</String>\r\n<String>\r\n<Name> </Name>\r\n<Val></Val>\r\n</String>\r\n<String>\r\n<Name> </Name>\r\n<Val></Val>\r\n</String>\r\n<String>\r\n<Name> </Name>\r\n<Val></Val>\r\n</String>\r\n<String>\r\n<Name> </Name>\r\n<Val></Val>\r\n</String>\r\n<String>\r\n<Name> </Name>\r\n<Val></Val>\r\n</String>\r\n<String>\r\n<Name> </Name>\r\n<Val></Val>\r\n</String>\r\n<String>\r\n<Name> </Name>\r\n<Val></Val>\r\n</String>\r\n<String>\r\n<Name> </Name>\r\n<Val></Val>\r\n</String>\r\n<String>\r\n<Name> </Name>\r\n<Val></Val>\r\n</String>\r\n<String>\r\n<Name> </Name>\r\n<Val></Val>\r\n</String>\r\n<String>\r\n<Name> </Name>\r\n<Val></Val>\r\n</String>\r\n<String>\r\n<Name> </Name>\r\n<Val></Val>\r\n</String>\r\n<String>\r\n<Name> </Name>\r\n<Val></Val>\r\n</String>\r\n<String>\r\n<Name> </Name>\r\n<Val></Val>\r\n</String>\r\n<String>\r\n<Name> </Name>\r\n<Val></Val>\r\n</String>\r\n<String>\r\n<Name> </Name>\r\n<Val></Val>\r\n</String>\r\n<String>\r\n<Name> </Name>\r\n<Val></Val>\r\n</String>\r\n<String>\r\n<Name> </Name>\r\n<Val></Val>\r\n</String>\r\n<String>\r\n<Name> </Name>\r\n<Val></Val>\r\n</String>\r\n<String>\r\n<Name> </Name>\r\n<Val></Val>\r\n</String>\r\n<String>\r\n<Name> </Name>\r\n<Val></Val>\r\n</String>\r\n<String>\r\n<Name> </Name>\r\n<Val></Val>\r\n</String>\r\n<String>\r\n<Name> </Name>\r\n<Val></Val>\r\n</String>\r\n<String>\r\n<Name> </Name>\r\n<Val></Val>\r\n</String>\r\n<String>\r\n<Name> </Name>\r\n<Val></Val>\r\n</String>\r\n<String>\r\n<Name> </Name>\r\n<Val></Val>\r\n</String>\r\n<String>\r\n<Name> </Name>\r\n<Val></Val>\r\n</String>\r\n<String>\r\n<Name> </Name>\r\n<Val></Val>\r\n</String>\r\n<String>\r\n<Name> </Name>\r\n<Val></Val>\r\n</String>\r\n<String>\r\n<Name> </Name>\r\n<Val></Val>\r\n</String>\r\n<String>\r\n<Name> </Name>\r\n<Val></Val>\r\n</String>\r\n<String>\r\n<Name> </Name>\r\n<Val></Val>\r\n</String>\r\n<String>\r\n<Name> </Name>\r\n<Val></Val>\r\n</String>\r\n<String>\r\n<Name> </Name>\r\n<Val></Val>\r\n</String>\r\n<String>\r\n<Name> </Name>\r\n<Val></Val>\r\n</String>\r\n<String>\r\n<Name> </Name>\r\n<Val></Val>\r\n</String>\r\n<String>\r\n<Name> </Name>\r\n<Val></Val>\r\n</String>\r\n<String>\r\n<Name> </Name>\r\n<Val></Val>\r\n</String>\r\n<String>\r\n<Name> </Name>\r\n<Val></Val>\r\n</String>\r\n<String>\r\n<Name> </Name>\r\n<Val></Val>\r\n</String>\r\n<String>\r\n<Name> </Name>\r\n<Val></Val>\r\n</String>\r\n<String>\r\n<Name> </Name>\r\n<Val></Val>\r\n</String>\r\n<String>\r\n<Name> </Name>\r\n<Val></Val>\r\n</String>\r\n<String>\r\n<Name> </Name>\r\n<Val></Val>\r\n</String>\r\n<String>\r\n<Name> </Name>\r\n<Val></Val>\r\n</String>\r\n<String>\r\n<Name> </Name>\r\n<Val></Val>\r\n</String>\r\n<String>\r\n<Name> </Name>\r\n<Val></Val>\r\n</String>\r\n<String>\r\n<Name> </Name>\r\n<Val></Val>\r\n</String>\r\n<String>\r\n<Name> </Name>\r\n<Val></Val>\r\n</String>\r\n<String>\r\n<Name> </Name>\r\n<Val></Val>\r\n</String>\r\n<String>\r\n<Name> </Name>\r\n<Val></Val>\r\n</String>\r\n<String>\r\n<Name> </Name>\r\n<Val></Val>\r\n</String>\r\n<String>\r\n<Name> </Name>\r\n<Val></Val>\r\n</String>\r\n<String>\r\n<Name> </Name>\r\n<Val></Val>\r\n</String>\r\n<String>\r\n<Name> </Name>\r\n<Val></Val>\r\n</String>\r\n<String>\r\n<Name> </Name>\r\n<Val></Val>\r\n</String>\r\n<String>\r\n<Name> </Name>\r\n<Val></Val>\r\n</String>\r\n<String>\r\n<Name> </Name>\r\n<Val></Val>\r\n</String>\r\n<String>\r\n<Name> </Name>\r\n<Val></Val>\r\n</String>\r\n<String>\r\n<Name> </Name>\r\n<Val></Val>\r\n</String>\r\n<String>\r\n<Name> </Name>\r\n<Val></Val>\r\n</String>\r\n<String>\r\n<Name> </Name>\r\n<Val></Val>\r\n</String>\r\n<String>\r\n<Name> </Name>\r\n<Val></Val>\r\n</String>\r\n<String>\r\n<Name> </Name>\r\n<Val></Val>\r\n</String>\r\n<String>\r\n<Name> </Name>\r\n<Val></Val>\r\n</String>\r\n<String>\r\n<Name> </Name>\r\n<Val></Val>\r\n</String>\r\n<String>\r\n<Name> </Name>\r\n<Val></Val>\r\n</String>\r\n<String>\r\n<Name> </Name>\r\n<Val></Val>\r\n</String>\r\n<String>\r\n<Name> </Name>\r\n<Val></Val>\r\n</String>\r\n<String>\r\n<Name> </Name>\r\n<Val></Val>\r\n</String>\r\n<String>\r\n<Name> </Name>\r\n<Val></Val>\r\n</String>\r\n<String>\r\n<Name> </Name>\r\n<Val></Val>\r\n</String>\r\n<String>\r\n<Name> </Name>\r\n<Val></Val>\r\n</String>\r\n<String>\r\n<Name> </Name>\r\n<Val></Val>\r\n</String>\r\n<String>\r\n<Name> </Name>\r\n<Val></Val>\r\n</String>\r\n<String>\r\n<Name> </Name>\r\n<Val></Val>\r\n</String>\r\n<String>\r\n<Name> </Name>\r\n<Val></Val>\r\n</String>\r\n<String>\r\n<Name> </Name>\r\n<Val></Val>\r\n</String>\r\n<String>\r\n<Name> </Name>\r\n<Val></Val>\r\n</String>\r\n<String>\r\n<Name> </Name>\r\n<Val></Val>\r\n</String>\r\n<String>\r\n<Name> </Name>\r\n<Val></Val>\r\n</String>\r\n<String>\r\n<Name> </Name>\r\n<Val></Val>\r\n</String>\r\n<String>\r\n<Name> </Name>\r\n<Val></Val>\r\n</String>\r\n<String>\r\n<Name> </Name>\r\n<Val></Val>\r\n</String>\r\n<String>\r\n<Name> </Name>\r\n<Val></Val>\r\n</String>\r\n<String>\r\n<Name> </Name>\r\n<Val></Val>\r\n</String>\r\n<String>\r\n<Name> </Name>\r\n<Val></Val>\r\n</String>\r\n<String>\r\n<Name> </Name>\r\n<Val></Val>\r\n</String>\r\n<String>\r\n<Name> </Name>\r\n<Val></Val>\r\n</String>\r\n<String>\r\n<Name> </Name>\r\n<Val></Val>\r\n</String>\r\n<String>\r\n<Name> </Name>\r\n<Val></Val>\r\n</String>\r\n<String>\r\n<Name> </Name>\r\n<Val></Val>\r\n</String>\r\n<String>\r\n<Name> </Name>\r\n<Val></Val>\r\n</String>\r\n<String>\r\n<Name> </Name>\r\n<Val></Val>\r\n</String>\r\n<String>\r\n<Name> </Name>\r\n<Val></Val>\r\n</String>\r\n<String>\r\n<Name> </Name>\r\n<Val></Val>\r\n</String>\r\n<String>\r\n<Name> </Name>\r\n<Val></Val>\r\n</String>\r\n<String>\r\n<Name> </Name>\r\n<Val></Val>\r\n</String>\r\n<String>\r\n<Name> </Name>\r\n<Val></Val>\r\n</String>\r\n<String>\r\n<Name> </Name>\r\n<Val></Val>\r\n</String>\r\n<String>\r\n<Name> </Name>\r\n<Val></Val>\r\n</String>\r\n<String>\r\n<Name> </Name>\r\n<Val></Val>\r\n</String>\r\n<String>\r\n<Name> </Name>\r\n<Val></Val>\r\n</String>\r\n<String>\r\n<Name> </Name>\r\n<Val></Val>\r\n</String>\r\n<String>\r\n<Name> </Name>\r\n<Val></Val>\r\n</String>\r\n<String>\r\n<Name> </Name>\r\n<Val></Val>\r\n</String>\r\n<String>\r\n<Name> </Name>\r\n<Val></Val>\r\n</String>\r\n<String>\r\n<Name> </Name>\r\n<Val></Val>\r\n</String>\r\n<String>\r\n<Name> </Name>\r\n<Val></Val>\r\n</String>\r\n<String>\r\n<Name> </Name>\r\n<Val></Val>\r\n</String>\r\n<String>\r\n<Name> </Name>\r\n<Val></Val>\r\n</String>\r\n<String>\r\n<Name> </Name>\r\n<Val></Val>\r\n</String>\r\n<String>\r\n<Name> </Name>\r\n<Val></Val>\r\n</String>\r\n<String>\r\n<Name> </Name>\r\n<Val></Val>\r\n</String>\r\n<String>\r\n<Name> </Name>\r\n<Val></Val>\r\n</String>\r\n<String>\r\n<Name> </Name>\r\n<Val></Val>\r\n</String>\r\n<String>\r\n<Name> </Name>\r\n<Val></Val>\r\n</String>\r\n<String>\r\n<Name> </Name>\r\n<Val></Val>\r\n</String>\r\n<String>\r\n<Name> </Name>\r\n<Val></Val>\r\n</String>\r\n<String>\r\n<Name> </Name>\r\n<Val></Val>\r\n</String>\r\n<String>\r\n<Name> </Name>\r\n<Val></Val>\r\n</String>\r\n<String>\r\n<Name> </Name>\r\n<Val></Val>\r\n</String>\r\n<String>\r\n<Name> </Name>\r\n<Val></Val>\r\n</String>\r\n<String>\r\n<Name> </Name>\r\n<Val></Val>\r\n</String>\r\n<String>\r\n<Name> </Name>\r\n<Val></Val>\r\n</String>\r\n<String>\r\n<Name> </Name>\r\n<Val></Val>\r\n</String>\r\n<String>\r\n<Name> </Name>\r\n<Val></Val>\r\n</String>\r\n<String>\r\n<Name> </Name>\r\n<Val></Val>\r\n</String>\r\n<String>\r\n<Name> </Name>\r\n<Val></Val>\r\n</String>\r\n<String>\r\n<Name> </Name>\r\n<Val></Val>\r\n</String>\r\n<String>\r\n<Name> </Name>\r\n<Val></Val>\r\n</String>\r\n<String>\r\n<Name> </Name>\r\n<Val></Val>\r\n</String>\r\n<String>\r\n<Name> </Name>\r\n<Val></Val>\r\n</String>\r\n<String>\r\n<Name> </Name>\r\n<Val></Val>\r\n</String>\r\n<String>\r\n<Name> </Name>\r\n<Val></Val>\r\n</String>\r\n<String>\r\n<Name> </Name>\r\n<Val></Val>\r\n</String>\r\n<String>\r\n<Name> </Name>\r\n<Val></Val>\r\n</String>\r\n<String>\r\n<Name> </Name>\r\n<Val></Val>\r\n</String>\r\n<String>\r\n<Name> </Name>\r\n<Val></Val>\r\n</String>\r\n<String>\r\n<Name> </Name>\r\n<Val></Val>\r\n</String>\r\n<String>\r\n<Name> </Name>\r\n<Val></Val>\r\n</String>\r\n<String>\r\n<Name> </Name>\r\n<Val></Val>\r\n</String>\r\n<String>\r\n<Name> </Name>\r\n<Val></Val>\r\n</String>\r\n<String>\r\n<Name> </Name>\r\n<Val></Val>\r\n</String>\r\n<String>\r\n<Name> </Name>\r\n<Val></Val>\r\n</String>\r\n<String>\r\n<Name> </Name>\r\n<Val></Val>\r\n</String>\r\n<String>\r\n<Name> </Name>\r\n<Val></Val>\r\n</String>\r\n<String>\r\n<Name> </Name>\r\n<Val></Val>\r\n</String>\r\n<String>\r\n<Name> </Name>\r\n<Val></Val>\r\n</String>\r\n<String>\r\n<Name> </Name>\r\n<Val></Val>\r\n</String>\r\n<String>\r\n<Name> </Name>\r\n<Val></Val>\r\n</String>\r\n<String>\r\n<Name> </Name>\r\n<Val></Val>\r\n</String>\r\n<String>\r\n<Name> </Name>\r\n<Val></Val>\r\n</String>\r\n<String>\r\n<Name> </Name>\r\n<Val></Val>\r\n</String>\r\n<String>\r\n<Name> </Name>\r\n<Val></Val>\r\n</String>\r\n<String>\r\n<Name> </Name>\r\n<Val></Val>\r\n</String>\r\n<String>\r\n<Name> </Name>\r\n<Val></Val>\r\n</String>\r\n<String>\r\n<Name> </Name>\r\n<Val></Val>\r\n</String>\r\n<String>\r\n<Name> </Name>\r\n<Val></Val>\r\n</String>\r\n<String>\r\n<Name> </Name>\r\n<Val></Val>\r\n</String>\r\n<String>\r\n<Name> </Name>\r\n<Val>LT</Val>\r\n</String>\r\n<String>\r\n<Name> </Name>\r\n<Val></Val>\r\n</String>\r\n<String>\r\n<Name> </Name>\r\n<Val></Val>\r\n</String>\r\n<String>\r\n<Name> </Name>\r\n<Val></Val>\r\n</String>\r\n<String>\r\n<Name> </Name>\r\n<Val></Val>\r\n</String>\r\n<String>\r\n<Name> </Name>\r\n<Val>GELE</Val>\r\n</String>\r\n<String>\r\n<Name> </Name>\r\n<Val>GELE</Val>\r\n</String>\r\n<String>\r\n<Name> </Name>\r\n<Val></Val>\r\n</String>\r\n<String>\r\n<Name> </Name>\r\n<Val>GELE</Val>\r\n</String>\r\n<String>\r\n<Name> </Name>\r\n<Val></Val>\r\n</String>\r\n<String>\r\n<Name> </Name>\r\n<Val></Val>\r\n</String>\r\n<String>\r\n<Name> </Name>\r\n<Val></Val>\r\n</String>\r\n<String>\r\n<Name> </Name>\r\n<Val></Val>\r\n</String>\r\n<String>\r\n<Name> </Name>\r\n<Val></Val>\r\n</String>\r\n<String>\r\n<Name> </Name>\r\n<Val></Val>\r\n</String>\r\n<String>\r\n<Name> </Name>\r\n<Val></Val>\r\n</String>\r\n<String>\r\n<Name> </Name>\r\n<Val></Val>\r\n</String>\r\n<String>\r\n<Name> </Name>\r\n<Val></Val>\r\n</String>\r\n<String>\r\n<Name> </Name>\r\n<Val></Val>\r\n</String>\r\n<String>\r\n<Name> </Name>\r\n<Val></Val>\r\n</String>\r\n<String>\r\n<Name> </Name>\r\n<Val></Val>\r\n</String>\r\n<String>\r\n<Name> </Name>\r\n<Val></Val>\r\n</String>\r\n<String>\r\n<Name> </Name>\r\n<Val></Val>\r\n</String>\r\n<String>\r\n<Name> </Name>\r\n<Val></Val>\r\n</String>\r\n<String>\r\n<Name> </Name>\r\n<Val></Val>\r\n</String>\r\n<String>\r\n<Name> </Name>\r\n<Val></Val>\r\n</String>\r\n<String>\r\n<Name> </Name>\r\n<Val></Val>\r\n</String>\r\n<String>\r\n<Name> </Name>\r\n<Val></Val>\r\n</String>\r\n<String>\r\n<Name> </Name>\r\n<Val></Val>\r\n</String>\r\n<String>\r\n<Name> </Name>\r\n<Val></Val>\r\n</String>\r\n<String>\r\n<Name> </Name>\r\n<Val></Val>\r\n</String>\r\n<String>\r\n<Name> </Name>\r\n<Val></Val>\r\n</String>\r\n<String>\r\n<Name> </Name>\r\n<Val></Val>\r\n</String>\r\n<String>\r\n<Name> </Name>\r\n<Val></Val>\r\n</String>\r\n<String>\r\n<Name> </Name>\r\n<Val></Val>\r\n</String>\r\n<String>\r\n<Name> </Name>\r\n<Val></Val>\r\n</String>\r\n<String>\r\n<Name> </Name>\r\n<Val></Val>\r\n</String>\r\n<String>\r\n<Name> </Name>\r\n<Val></Val>\r\n</String>\r\n<String>\r\n<Name> </Name>\r\n<Val></Val>\r\n</String>\r\n<String>\r\n<Name> </Name>\r\n<Val></Val>\r\n</String>\r\n<String>\r\n<Name> </Name>\r\n<Val></Val>\r\n</String>\r\n<String>\r\n<Name> </Name>\r\n<Val></Val>\r\n</String>\r\n<String>\r\n<Name> </Name>\r\n<Val></Val>\r\n</String>\r\n<String>\r\n<Name> </Name>\r\n<Val></Val>\r\n</String>\r\n<String>\r\n<Name> </Name>\r\n<Val></Val>\r\n</String>\r\n<String>\r\n<Name> </Name>\r\n<Val></Val>\r\n</String>\r\n<String>\r\n<Name> </Name>\r\n<Val></Val>\r\n</String>\r\n<String>\r\n<Name> </Name>\r\n<Val></Val>\r\n</String>\r\n<String>\r\n<Name> </Name>\r\n<Val></Val>\r\n</String>\r\n<String>\r\n<Name> </Name>\r\n<Val></Val>\r\n</String>\r\n<String>\r\n<Name> </Name>\r\n<Val></Val>\r\n</String>\r\n<String>\r\n<Name> </Name>\r\n<Val></Val>\r\n</String>\r\n<String>\r\n<Name> </Name>\r\n<Val></Val>\r\n</String>\r\n<String>\r\n<Name> </Name>\r\n<Val>GELE</Val>\r\n</String>\r\n<String>\r\n<Name> </Name>\r\n<Val></Val>\r\n</String>\r\n<String>\r\n<Name> </Name>\r\n<Val></Val>\r\n</String>\r\n<String>\r\n<Name> </Name>\r\n<Val></Val>\r\n</String>\r\n<String>\r\n<Name> </Name>\r\n<Val></Val>\r\n</String>\r\n<String>\r\n<Name> </Name>\r\n<Val></Val>\r\n</String>\r\n<String>\r\n<Name> </Name>\r\n<Val></Val>\r\n</String>\r\n<String>\r\n<Name> </Name>\r\n<Val></Val>\r\n</String>\r\n<String>\r\n<Name> </Name>\r\n<Val></Val>\r\n</String>\r\n<String>\r\n<Name> </Name>\r\n<Val></Val>\r\n</String>\r\n<String>\r\n<Name> </Name>\r\n<Val></Val>\r\n</String>\r\n<String>\r\n<Name> </Name>\r\n<Val></Val>\r\n</String>\r\n<String>\r\n<Name> </Name>\r\n<Val></Val>\r\n</String>\r\n<String>\r\n<Name> </Name>\r\n<Val></Val>\r\n</String>\r\n<String>\r\n<Name> </Name>\r\n<Val></Val>\r\n</String>\r\n<String>\r\n<Name> </Name>\r\n<Val></Val>\r\n</String>\r\n<String>\r\n<Name> </Name>\r\n<Val></Val>\r\n</String>\r\n<String>\r\n<Name> </Name>\r\n<Val></Val>\r\n</String>\r\n<String>\r\n<Name> </Name>\r\n<Val></Val>\r\n</String>\r\n<String>\r\n<Name> </Name>\r\n<Val></Val>\r\n</String>\r\n<String>\r\n<Name> </Name>\r\n<Val></Val>\r\n</String>\r\n<String>\r\n<Name> </Name>\r\n<Val></Val>\r\n</String>\r\n<String>\r\n<Name> </Name>\r\n<Val></Val>\r\n</String>\r\n<String>\r\n<Name> </Name>\r\n<Val></Val>\r\n</String>\r\n<String>\r\n<Name> </Name>\r\n<Val></Val>\r\n</String>\r\n<String>\r\n<Name> </Name>\r\n<Val></Val>\r\n</String>\r\n<String>\r\n<Name> </Name>\r\n<Val></Val>\r\n</String>\r\n<String>\r\n<Name> </Name>\r\n<Val></Val>\r\n</String>\r\n<String>\r\n<Name> </Name>\r\n<Val></Val>\r\n</String>\r\n<String>\r\n<Name> </Name>\r\n<Val></Val>\r\n</String>\r\n<String>\r\n<Name> </Name>\r\n<Val></Val>\r\n</String>\r\n<String>\r\n<Name> </Name>\r\n<Val></Val>\r\n</String>\r\n<String>\r\n<Name> </Name>\r\n<Val></Val>\r\n</String>\r\n<String>\r\n<Name> </Name>\r\n<Val></Val>\r\n</String>\r\n<String>\r\n<Name> </Name>\r\n<Val></Val>\r\n</String>\r\n<String>\r\n<Name> </Name>\r\n<Val></Val>\r\n</String>\r\n<String>\r\n<Name> </Name>\r\n<Val></Val>\r\n</String>\r\n<String>\r\n<Name> </Name>\r\n<Val></Val>\r\n</String>\r\n<String>\r\n<Name> </Name>\r\n<Val></Val>\r\n</String>\r\n<String>\r\n<Name> </Name>\r\n<Val></Val>\r\n</String>\r\n<String>\r\n<Name> </Name>\r\n<Val></Val>\r\n</String>\r\n<String>\r\n<Name> </Name>\r\n<Val></Val>\r\n</String>\r\n<String>\r\n<Name> </Name>\r\n<Val></Val>\r\n</String>\r\n<String>\r\n<Name> </Name>\r\n<Val></Val>\r\n</String>\r\n<String>\r\n<Name> </Name>\r\n<Val></Val>\r\n</String>\r\n<String>\r\n<Name> </Name>\r\n<Val></Val>\r\n</String>\r\n<String>\r\n<Name> </Name>\r\n<Val></Val>\r\n</String>\r\n<String>\r\n<Name> </Name>\r\n<Val></Val>\r\n</String>\r\n<String>\r\n<Name> </Name>\r\n<Val></Val>\r\n</String>\r\n<String>\r\n<Name> </Name>\r\n<Val></Val>\r\n</String>\r\n<String>\r\n<Name> </Name>\r\n<Val></Val>\r\n</String>\r\n<String>\r\n<Name> </Name>\r\n<Val></Val>\r\n</String>\r\n<String>\r\n<Name> </Name>\r\n<Val></Val>\r\n</String>\r\n<String>\r\n<Name> </Name>\r\n<Val></Val>\r\n</String>\r\n<String>\r\n<Name> </Name>\r\n<Val></Val>\r\n</String>\r\n<String>\r\n<Name> </Name>\r\n<Val></Val>\r\n</String>\r\n<String>\r\n<Name> </Name>\r\n<Val></Val>\r\n</String>\r\n<String>\r\n<Name> </Name>\r\n<Val></Val>\r\n</String>\r\n<String>\r\n<Name> </Name>\r\n<Val></Val>\r\n</String>\r\n<String>\r\n<Name> </Name>\r\n<Val></Val>\r\n</String>\r\n<String>\r\n<Name> </Name>\r\n<Val></Val>\r\n</String>\r\n<String>\r\n<Name> </Name>\r\n<Val></Val>\r\n</String>\r\n<String>\r\n<Name> </Name>\r\n<Val></Val>\r\n</String>\r\n<String>\r\n<Name> </Name>\r\n<Val></Val>\r\n</String>\r\n<String>\r\n<Name> </Name>\r\n<Val></Val>\r\n</String>\r\n<String>\r\n<Name> </Name>\r\n<Val></Val>\r\n</String>\r\n<String>\r\n<Name> </Name>\r\n<Val></Val>\r\n</String>\r\n<String>\r\n<Name> </Name>\r\n<Val></Val>\r\n</String>\r\n<String>\r\n<Name> </Name>\r\n<Val></Val>\r\n</String>\r\n<String>\r\n<Name> </Name>\r\n<Val></Val>\r\n</String>\r\n<String>\r\n<Name> </Name>\r\n<Val></Val>\r\n</String>\r\n<String>\r\n<Name> </Name>\r\n<Val></Val>\r\n</String>\r\n<String>\r\n<Name> </Name>\r\n<Val></Val>\r\n</String>\r\n<String>\r\n<Name> </Name>\r\n<Val></Val>\r\n</String>\r\n<String>\r\n<Name> </Name>\r\n<Val></Val>\r\n</String>\r\n<String>\r\n<Name> </Name>\r\n<Val></Val>\r\n</String>\r\n<String>\r\n<Name> </Name>\r\n<Val></Val>\r\n</String>\r\n<String>\r\n<Name> </Name>\r\n<Val></Val>\r\n</String>\r\n<String>\r\n<Name> </Name>\r\n<Val></Val>\r\n</String>\r\n<String>\r\n<Name> </Name>\r\n<Val></Val>\r\n</String>\r\n<String>\r\n<Name> </Name>\r\n<Val></Val>\r\n</String>\r\n<String>\r\n<Name> </Name>\r\n<Val></Val>\r\n</String>\r\n<String>\r\n<Name> </Name>\r\n<Val></Val>\r\n</String>\r\n<String>\r\n<Name> </Name>\r\n<Val></Val>\r\n</String>\r\n<String>\r\n<Name> </Name>\r\n<Val></Val>\r\n</String>\r\n<String>\r\n<Name> </Name>\r\n<Val></Val>\r\n</String>\r\n<String>\r\n<Name> </Name>\r\n<Val></Val>\r\n</String>\r\n<String>\r\n<Name> </Name>\r\n<Val></Val>\r\n</String>\r\n<String>\r\n<Name> </Name>\r\n<Val></Val>\r\n</String>\r\n<String>\r\n<Name> </Name>\r\n<Val></Val>\r\n</String>\r\n<String>\r\n<Name> </Name>\r\n<Val></Val>\r\n</String>\r\n<String>\r\n<Name> </Name>\r\n<Val></Val>\r\n</String>\r\n<String>\r\n<Name> </Name>\r\n<Val></Val>\r\n</String>\r\n<String>\r\n<Name> </Name>\r\n<Val></Val>\r\n</String>\r\n<String>\r\n<Name> </Name>\r\n<Val></Val>\r\n</String>\r\n<String>\r\n<Name> </Name>\r\n<Val></Val>\r\n</String>\r\n<String>\r\n<Name> </Name>\r\n<Val></Val>\r\n</String>\r\n<String>\r\n<Name> </Name>\r\n<Val></Val>\r\n</String>\r\n<String>\r\n<Name> </Name>\r\n<Val></Val>\r\n</String>\r\n<String>\r\n<Name> </Name>\r\n<Val></Val>\r\n</String>\r\n<String>\r\n<Name> </Name>\r\n<Val></Val>\r\n</String>\r\n<String>\r\n<Name> </Name>\r\n<Val></Val>\r\n</String>\r\n<String>\r\n<Name> </Name>\r\n<Val></Val>\r\n</String>\r\n<String>\r\n<Name> </Name>\r\n<Val></Val>\r\n</String>\r\n<String>\r\n<Name> </Name>\r\n<Val></Val>\r\n</String>\r\n<String>\r\n<Name> </Name>\r\n<Val></Val>\r\n</String>\r\n<String>\r\n<Name> </Name>\r\n<Val></Val>\r\n</String>\r\n<String>\r\n<Name> </Name>\r\n<Val></Val>\r\n</String>\r\n<String>\r\n<Name> </Name>\r\n<Val></Val>\r\n</String>\r\n<String>\r\n<Name> </Name>\r\n<Val></Val>\r\n</String>\r\n<String>\r\n<Name> </Name>\r\n<Val></Val>\r\n</String>\r\n<String>\r\n<Name> </Name>\r\n<Val></Val>\r\n</String>\r\n<String>\r\n<Name> </Name>\r\n<Val></Val>\r\n</String>\r\n<String>\r\n<Name> </Name>\r\n<Val></Val>\r\n</String>\r\n<String>\r\n<Name> </Name>\r\n<Val></Val>\r\n</String>\r\n<String>\r\n<Name> </Name>\r\n<Val></Val>\r\n</String>\r\n<String>\r\n<Name> </Name>\r\n<Val></Val>\r\n</String>\r\n<String>\r\n<Name> </Name>\r\n<Val></Val>\r\n</String>\r\n<String>\r\n<Name> </Name>\r\n<Val></Val>\r\n</String>\r\n<String>\r\n<Name> </Name>\r\n<Val></Val>\r\n</String>\r\n<String>\r\n<Name> </Name>\r\n<Val></Val>\r\n</String>\r\n<String>\r\n<Name> </Name>\r\n<Val></Val>\r\n</String>\r\n<String>\r\n<Name> </Name>\r\n<Val></Val>\r\n</String>\r\n<String>\r\n<Name> </Name>\r\n<Val></Val>\r\n</String>\r\n<String>\r\n<Name> </Name>\r\n<Val></Val>\r\n</String>\r\n<String>\r\n<Name> </Name>\r\n<Val></Val>\r\n</String>\r\n<String>\r\n<Name> </Name>\r\n<Val></Val>\r\n</String>\r\n<String>\r\n<Name> </Name>\r\n<Val></Val>\r\n</String>\r\n<String>\r\n<Name> </Name>\r\n<Val></Val>\r\n</String>\r\n<String>\r\n<Name> </Name>\r\n<Val></Val>\r\n</String>\r\n<String>\r\n<Name> </Name>\r\n<Val></Val>\r\n</String>\r\n<String>\r\n<Name> </Name>\r\n<Val></Val>\r\n</String>\r\n<String>\r\n<Name> </Name>\r\n<Val>LT</Val>\r\n</String>\r\n<String>\r\n<Name> </Name>\r\n<Val></Val>\r\n</String>\r\n<String>\r\n<Name> </Name>\r\n<Val></Val>\r\n</String>\r\n<String>\r\n<Name> </Name>\r\n<Val></Val>\r\n</String>\r\n<String>\r\n<Name> </Name>\r\n<Val></Val>\r\n</String>\r\n<String>\r\n<Name> </Name>\r\n<Val></Val>\r\n</String>\r\n<String>\r\n<Name> </Name>\r\n<Val></Val>\r\n</String>\r\n<String>\r\n<Name> </Name>\r\n<Val>GT</Val>\r\n</String>\r\n<String>\r\n<Name> </Name>\r\n<Val></Val>\r\n</String>\r\n<String>\r\n<Name> </Name>\r\n<Val></Val>\r\n</String>\r\n<String>\r\n<Name> </Name>\r\n<Val></Val>\r\n</String>\r\n<String>\r\n<Name> </Name>\r\n<Val></Val>\r\n</String>\r\n<String>\r\n<Name> </Name>\r\n<Val>LT</Val>\r\n</String>\r\n<String>\r\n<Name> </Name>\r\n<Val></Val>\r\n</String>\r\n<String>\r\n<Name> </Name>\r\n<Val></Val>\r\n</String>\r\n<String>\r\n<Name> </Name>\r\n<Val></Val>\r\n</String>\r\n<String>\r\n<Name> </Name>\r\n<Val></Val>\r\n</String>\r\n<String>\r\n<Name> </Name>\r\n<Val></Val>\r\n</String>\r\n<String>\r\n<Name> </Name>\r\n<Val></Val>\r\n</String>\r\n<String>\r\n<Name> </Name>\r\n<Val>GT</Val>\r\n</String>\r\n<String>\r\n<Name> </Name>\r\n<Val></Val>\r\n</String>\r\n<String>\r\n<Name> </Name>\r\n<Val></Val>\r\n</String>\r\n<String>\r\n<Name> </Name>\r\n<Val></Val>\r\n</String>\r\n<String>\r\n<Name> </Name>\r\n<Val></Val>\r\n</String>\r\n<String>\r\n<Name> </Name>\r\n<Val>LT</Val>\r\n</String>\r\n<String>\r\n<Name> </Name>\r\n<Val></Val>\r\n</String>\r\n<String>\r\n<Name> </Name>\r\n<Val></Val>\r\n</String>\r\n<String>\r\n<Name> </Name>\r\n<Val></Val>\r\n</String>\r\n<String>\r\n<Name> </Name>\r\n<Val></Val>\r\n</String>\r\n<String>\r\n<Name> </Name>\r\n<Val></Val>\r\n</String>\r\n<String>\r\n<Name> </Name>\r\n<Val></Val>\r\n</String>\r\n<String>\r\n<Name> </Name>\r\n<Val>GT</Val>\r\n</String>\r\n<String>\r\n<Name> </Name>\r\n<Val></Val>\r\n</String>\r\n<String>\r\n<Name> </Name>\r\n<Val></Val>\r\n</String>\r\n<String>\r\n<Name> </Name>\r\n<Val></Val>\r\n</String>\r\n<String>\r\n<Name> </Name>\r\n<Val></Val>\r\n</String>\r\n<String>\r\n<Name> </Name>\r\n<Val>LT</Val>\r\n</String>\r\n<String>\r\n<Name> </Name>\r\n<Val></Val>\r\n</String>\r\n<String>\r\n<Name> </Name>\r\n<Val></Val>\r\n</String>\r\n<String>\r\n<Name> </Name>\r\n<Val></Val>\r\n</String>\r\n<String>\r\n<Name> </Name>\r\n<Val></Val>\r\n</String>\r\n<String>\r\n<Name> </Name>\r\n<Val></Val>\r\n</String>\r\n<String>\r\n<Name> </Name>\r\n<Val></Val>\r\n</String>\r\n<String>\r\n<Name> </Name>\r\n<Val>GT</Val>\r\n</String>\r\n<String>\r\n<Name> </Name>\r\n<Val></Val>\r\n</String>\r\n<String>\r\n<Name> </Name>\r\n<Val></Val>\r\n</String>\r\n<String>\r\n<Name> </Name>\r\n<Val></Val>\r\n</String>\r\n<String>\r\n<Name> </Name>\r\n<Val></Val>\r\n</String>\r\n<String>\r\n<Name> </Name>\r\n<Val></Val>\r\n</String>\r\n<String>\r\n<Name> </Name>\r\n<Val></Val>\r\n</String>\r\n<String>\r\n<Name> </Name>\r\n<Val>LT</Val>\r\n</String>\r\n<String>\r\n<Name> </Name>\r\n<Val></Val>\r\n</String>\r\n<String>\r\n<Name> </Name>\r\n<Val></Val>\r\n</String>\r\n<String>\r\n<Name> </Name>\r\n<Val></Val>\r\n</String>\r\n<String>\r\n<Name> </Name>\r\n<Val></Val>\r\n</String>\r\n<String>\r\n<Name> </Name>\r\n<Val></Val>\r\n</String>\r\n<String>\r\n<Name> </Name>\r\n<Val></Val>\r\n</String>\r\n<String>\r\n<Name> </Name>\r\n<Val>GT</Val>\r\n</String>\r\n<String>\r\n<Name> </Name>\r\n<Val></Val>\r\n</String>\r\n<String>\r\n<Name> </Name>\r\n<Val></Val>\r\n</String>\r\n<String>\r\n<Name> </Name>\r\n<Val></Val>\r\n</String>\r\n<String>\r\n<Name> </Name>\r\n<Val></Val>\r\n</String>\r\n<String>\r\n<Name> </Name>\r\n<Val>LT</Val>\r\n</String>\r\n<String>\r\n<Name> </Name>\r\n<Val></Val>\r\n</String>\r\n<String>\r\n<Name> </Name>\r\n<Val></Val>\r\n</String>\r\n<String>\r\n<Name> </Name>\r\n<Val></Val>\r\n</String>\r\n<String>\r\n<Name> </Name>\r\n<Val></Val>\r\n</String>\r\n<String>\r\n<Name> </Name>\r\n<Val></Val>\r\n</String>\r\n<String>\r\n<Name> </Name>\r\n<Val></Val>\r\n</String>\r\n<String>\r\n<Name> </Name>\r\n<Val>GT</Val>\r\n</String>\r\n<String>\r\n<Name> </Name>\r\n<Val></Val>\r\n</String>\r\n<String>\r\n<Name> </Name>\r\n<Val></Val>\r\n</String>\r\n<String>\r\n<Name> </Name>\r\n<Val></Val>\r\n</String>\r\n<String>\r\n<Name> </Name>\r\n<Val></Val>\r\n</String>\r\n<String>\r\n<Name> </Name>\r\n<Val>LT</Val>\r\n</String>\r\n<String>\r\n<Name> </Name>\r\n<Val></Val>\r\n</String>\r\n<String>\r\n<Name> </Name>\r\n<Val></Val>\r\n</String>\r\n<String>\r\n<Name> </Name>\r\n<Val></Val>\r\n</String>\r\n<String>\r\n<Name> </Name>\r\n<Val></Val>\r\n</String>\r\n<String>\r\n<Name> </Name>\r\n<Val></Val>\r\n</String>\r\n<String>\r\n<Name> </Name>\r\n<Val></Val>\r\n</String>\r\n<String>\r\n<Name> </Name>\r\n<Val>GT</Val>\r\n</String>\r\n<String>\r\n<Name> </Name>\r\n<Val></Val>\r\n</String>\r\n<String>\r\n<Name> </Name>\r\n<Val></Val>\r\n</String>\r\n<String>\r\n<Name> </Name>\r\n<Val></Val>\r\n</String>\r\n<String>\r\n<Name> </Name>\r\n<Val></Val>\r\n</String>\r\n<String>\r\n<Name> </Name>\r\n<Val>LT</Val>\r\n</String>\r\n<String>\r\n<Name> </Name>\r\n<Val></Val>\r\n</String>\r\n<String>\r\n<Name> </Name>\r\n<Val></Val>\r\n</String>\r\n<String>\r\n<Name> </Name>\r\n<Val></Val>\r\n</String>\r\n<String>\r\n<Name> </Name>\r\n<Val></Val>\r\n</String>\r\n<String>\r\n<Name> </Name>\r\n<Val></Val>\r\n</String>\r\n<String>\r\n<Name> </Name>\r\n<Val></Val>\r\n</String>\r\n<String>\r\n<Name> </Name>\r\n<Val>GT</Val>\r\n</String>\r\n<String>\r\n<Name> </Name>\r\n<Val></Val>\r\n</String>\r\n<String>\r\n<Name> </Name>\r\n<Val></Val>\r\n</String>\r\n<String>\r\n<Name> </Name>\r\n<Val></Val>\r\n</String>\r\n<String>\r\n<Name> </Name>\r\n<Val></Val>\r\n</String>\r\n<String>\r\n<Name> </Name>\r\n<Val></Val>\r\n</String>\r\n<String>\r\n<Name> </Name>\r\n<Val></Val>\r\n</String>\r\n<String>\r\n<Name> </Name>\r\n<Val>LT</Val>\r\n</String>\r\n<String>\r\n<Name> </Name>\r\n<Val></Val>\r\n</String>\r\n<String>\r\n<Name> </Name>\r\n<Val></Val>\r\n</String>\r\n<String>\r\n<Name> </Name>\r\n<Val></Val>\r\n</String>\r\n<String>\r\n<Name> </Name>\r\n<Val></Val>\r\n</String>\r\n<String>\r\n<Name> </Name>\r\n<Val></Val>\r\n</String>\r\n<String>\r\n<Name> </Name>\r\n<Val></Val>\r\n</String>\r\n<String>\r\n<Name> </Name>\r\n<Val>GT</Val>\r\n</String>\r\n<String>\r\n<Name> </Name>\r\n<Val></Val>\r\n</String>\r\n<String>\r\n<Name> </Name>\r\n<Val></Val>\r\n</String>\r\n<String>\r\n<Name> </Name>\r\n<Val></Val>\r\n</String>\r\n<String>\r\n<Name> </Name>\r\n<Val></Val>\r\n</String>\r\n<String>\r\n<Name> </Name>\r\n<Val>LT</Val>\r\n</String>\r\n<String>\r\n<Name> </Name>\r\n<Val></Val>\r\n</String>\r\n<String>\r\n<Name> </Name>\r\n<Val></Val>\r\n</String>\r\n<String>\r\n<Name> </Name>\r\n<Val></Val>\r\n</String>\r\n<String>\r\n<Name> </Name>\r\n<Val></Val>\r\n</String>\r\n<String>\r\n<Name> </Name>\r\n<Val></Val>\r\n</String>\r\n<String>\r\n<Name> </Name>\r\n<Val></Val>\r\n</String>\r\n<String>\r\n<Name> </Name>\r\n<Val>GT</Val>\r\n</String>\r\n<String>\r\n<Name> </Name>\r\n<Val></Val>\r\n</String>\r\n<String>\r\n<Name> </Name>\r\n<Val></Val>\r\n</String>\r\n<String>\r\n<Name> </Name>\r\n<Val></Val>\r\n</String>\r\n<String>\r\n<Name> </Name>\r\n<Val></Val>\r\n</String>\r\n<String>\r\n<Name> </Name>\r\n<Val>LT</Val>\r\n</String>\r\n<String>\r\n<Name> </Name>\r\n<Val></Val>\r\n</String>\r\n<String>\r\n<Name> </Name>\r\n<Val></Val>\r\n</String>\r\n<String>\r\n<Name> </Name>\r\n<Val></Val>\r\n</String>\r\n<String>\r\n<Name> </Name>\r\n<Val></Val>\r\n</String>\r\n<String>\r\n<Name> </Name>\r\n<Val></Val>\r\n</String>\r\n<String>\r\n<Name> </Name>\r\n<Val></Val>\r\n</String>\r\n<String>\r\n<Name> </Name>\r\n<Val>GT</Val>\r\n</String>\r\n<String>\r\n<Name> </Name>\r\n<Val></Val>\r\n</String>\r\n<String>\r\n<Name> </Name>\r\n<Val></Val>\r\n</String>\r\n<String>\r\n<Name> </Name>\r\n<Val></Val>\r\n</String>\r\n<String>\r\n<Name> </Name>\r\n<Val></Val>\r\n</String>\r\n<String>\r\n<Name> </Name>\r\n<Val>LT</Val>\r\n</String>\r\n<String>\r\n<Name> </Name>\r\n<Val></Val>\r\n</String>\r\n<String>\r\n<Name> </Name>\r\n<Val></Val>\r\n</String>\r\n<String>\r\n<Name> </Name>\r\n<Val></Val>\r\n</String>\r\n<String>\r\n<Name> </Name>\r\n<Val></Val>\r\n</String>\r\n<String>\r\n<Name> </Name>\r\n<Val></Val>\r\n</String>\r\n<String>\r\n<Name> </Name>\r\n<Val></Val>\r\n</String>\r\n<String>\r\n<Name> </Name>\r\n<Val>GT</Val>\r\n</String>\r\n<String>\r\n<Name> </Name>\r\n<Val></Val>\r\n</String>\r\n<String>\r\n<Name> </Name>\r\n<Val></Val>\r\n</String>\r\n<String>\r\n<Name> </Name>\r\n<Val></Val>\r\n</String>\r\n<String>\r\n<Name> </Name>\r\n<Val></Val>\r\n</String>\r\n<String>\r\n<Name> </Name>\r\n<Val></Val>\r\n</String>\r\n<String>\r\n<Name> </Name>\r\n<Val></Val>\r\n</String>\r\n<String>\r\n<Name> </Name>\r\n<Val>LT</Val>\r\n</String>\r\n<String>\r\n<Name> </Name>\r\n<Val></Val>\r\n</String>\r\n<String>\r\n<Name> </Name>\r\n<Val></Val>\r\n</String>\r\n<String>\r\n<Name> </Name>\r\n<Val></Val>\r\n</String>\r\n<String>\r\n<Name> </Name>\r\n<Val></Val>\r\n</String>\r\n<String>\r\n<Name> </Name>\r\n<Val></Val>\r\n</String>\r\n<String>\r\n<Name> </Name>\r\n<Val></Val>\r\n</String>\r\n<String>\r\n<Name> </Name>\r\n<Val>GT</Val>\r\n</String>\r\n<String>\r\n<Name> </Name>\r\n<Val></Val>\r\n</String>\r\n<String>\r\n<Name> </Name>\r\n<Val></Val>\r\n</String>\r\n<String>\r\n<Name> </Name>\r\n<Val></Val>\r\n</String>\r\n<String>\r\n<Name> </Name>\r\n<Val></Val>\r\n</String>\r\n<String>\r\n<Name> </Name>\r\n<Val>LT</Val>\r\n</String>\r\n<String>\r\n<Name> </Name>\r\n<Val></Val>\r\n</String>\r\n<String>\r\n<Name> </Name>\r\n<Val></Val>\r\n</String>\r\n<String>\r\n<Name> </Name>\r\n<Val></Val>\r\n</String>\r\n<String>\r\n<Name> </Name>\r\n<Val></Val>\r\n</String>\r\n<String>\r\n<Name> </Name>\r\n<Val></Val>\r\n</String>\r\n<String>\r\n<Name> </Name>\r\n<Val></Val>\r\n</String>\r\n<String>\r\n<Name> </Name>\r\n<Val>GT</Val>\r\n</String>\r\n<String>\r\n<Name> </Name>\r\n<Val></Val>\r\n</String>\r\n<String>\r\n<Name> </Name>\r\n<Val></Val>\r\n</String>\r\n<String>\r\n<Name> </Name>\r\n<Val></Val>\r\n</String>\r\n<String>\r\n<Name> </Name>\r\n<Val></Val>\r\n</String>\r\n<String>\r\n<Name> </Name>\r\n<Val>LT</Val>\r\n</String>\r\n<String>\r\n<Name> </Name>\r\n<Val></Val>\r\n</String>\r\n<String>\r\n<Name> </Name>\r\n<Val></Val>\r\n</String>\r\n<String>\r\n<Name> </Name>\r\n<Val></Val>\r\n</String>\r\n<String>\r\n<Name> </Name>\r\n<Val></Val>\r\n</String>\r\n<String>\r\n<Name> </Name>\r\n<Val></Val>\r\n</String>\r\n<String>\r\n<Name> </Name>\r\n<Val></Val>\r\n</String>\r\n<String>\r\n<Name> </Name>\r\n<Val>GT</Val>\r\n</String>\r\n<String>\r\n<Name> </Name>\r\n<Val></Val>\r\n</String>\r\n<String>\r\n<Name> </Name>\r\n<Val></Val>\r\n</String>\r\n<String>\r\n<Name> </Name>\r\n<Val></Val>\r\n</String>\r\n<String>\r\n<Name> </Name>\r\n<Val></Val>\r\n</String>\r\n<String>\r\n<Name> </Name>\r\n<Val>LT</Val>\r\n</String>\r\n<String>\r\n<Name> </Name>\r\n<Val></Val>\r\n</String>\r\n<String>\r\n<Name> </Name>\r\n<Val></Val>\r\n</String>\r\n<String>\r\n<Name> </Name>\r\n<Val></Val>\r\n</String>\r\n<String>\r\n<Name> </Name>\r\n<Val></Val>\r\n</String>\r\n<String>\r\n<Name> </Name>\r\n<Val></Val>\r\n</String>\r\n<String>\r\n<Name> </Name>\r\n<Val></Val>\r\n</String>\r\n<String>\r\n<Name> </Name>\r\n<Val>GT</Val>\r\n</String>\r\n<String>\r\n<Name> </Name>\r\n<Val></Val>\r\n</String>\r\n<String>\r\n<Name> </Name>\r\n<Val></Val>\r\n</String>\r\n<String>\r\n<Name> </Name>\r\n<Val></Val>\r\n</String>\r\n<String>\r\n<Name> </Name>\r\n<Val></Val>\r\n</String>\r\n<String>\r\n<Name> </Name>\r\n<Val></Val>\r\n</String>\r\n<String>\r\n<Name> </Name>\r\n<Val></Val>\r\n</String>\r\n<String>\r\n<Name> </Name>\r\n<Val></Val>\r\n</String>\r\n<String>\r\n<Name> </Name>\r\n<Val></Val>\r\n</String>\r\n<String>\r\n<Name> </Name>\r\n<Val></Val>\r\n</String>\r\n<String>\r\n<Name> </Name>\r\n<Val></Val>\r\n</String>\r\n<String>\r\n<Name> </Name>\r\n<Val></Val>\r\n</String>\r\n<String>\r\n<Name> </Name>\r\n<Val></Val>\r\n</String>\r\n<String>\r\n<Name> </Name>\r\n<Val></Val>\r\n</String>\r\n<String>\r\n<Name> </Name>\r\n<Val></Val>\r\n</String>\r\n<String>\r\n<Name> </Name>\r\n<Val></Val>\r\n</String>\r\n<String>\r\n<Name> </Name>\r\n<Val></Val>\r\n</String>\r\n<String>\r\n<Name> </Name>\r\n<Val></Val>\r\n</String>\r\n<String>\r\n<Name> </Name>\r\n<Val></Val>\r\n</String>\r\n<String>\r\n<Name> </Name>\r\n<Val></Val>\r\n</String>\r\n<String>\r\n<Name> </Name>\r\n<Val></Val>\r\n</String>\r\n<String>\r\n<Name> </Name>\r\n<Val></Val>\r\n</String>\r\n<String>\r\n<Name> </Name>\r\n<Val></Val>\r\n</String>\r\n<String>\r\n<Name> </Name>\r\n<Val></Val>\r\n</String>\r\n<String>\r\n<Name> </Name>\r\n<Val></Val>\r\n</String>\r\n<String>\r\n<Name> </Name>\r\n<Val></Val>\r\n</String>\r\n<String>\r\n<Name> </Name>\r\n<Val></Val>\r\n</String>\r\n<String>\r\n<Name> </Name>\r\n<Val></Val>\r\n</String>\r\n<String>\r\n<Name> </Name>\r\n<Val></Val>\r\n</String>\r\n<String>\r\n<Name> </Name>\r\n<Val></Val>\r\n</String>\r\n<String>\r\n<Name> </Name>\r\n<Val></Val>\r\n</String>\r\n<String>\r\n<Name> </Name>\r\n<Val></Val>\r\n</String>\r\n<String>\r\n<Name> </Name>\r\n<Val></Val>\r\n</String>\r\n<String>\r\n<Name> </Name>\r\n<Val></Val>\r\n</String>\r\n<String>\r\n<Name> </Name>\r\n<Val></Val>\r\n</String>\r\n<String>\r\n<Name> </Name>\r\n<Val></Val>\r\n</String>\r\n<String>\r\n<Name> </Name>\r\n<Val></Val>\r\n</String>\r\n<String>\r\n<Name> </Name>\r\n<Val></Val>\r\n</String>\r\n<String>\r\n<Name> </Name>\r\n<Val></Val>\r\n</String>\r\n<String>\r\n<Name> </Name>\r\n<Val></Val>\r\n</String>\r\n<String>\r\n<Name> </Name>\r\n<Val></Val>\r\n</String>\r\n<String>\r\n<Name> </Name>\r\n<Val></Val>\r\n</String>\r\n<String>\r\n<Name> </Name>\r\n<Val></Val>\r\n</String>\r\n<String>\r\n<Name> </Name>\r\n<Val></Val>\r\n</String>\r\n<String>\r\n<Name> </Name>\r\n<Val></Val>\r\n</String>\r\n<String>\r\n<Name> </Name>\r\n<Val></Val>\r\n</String>\r\n<String>\r\n<Name> </Name>\r\n<Val></Val>\r\n</String>\r\n<String>\r\n<Name> </Name>\r\n<Val></Val>\r\n</String>\r\n<String>\r\n<Name> </Name>\r\n<Val></Val>\r\n</String>\r\n<String>\r\n<Name> </Name>\r\n<Val></Val>\r\n</String>\r\n<String>\r\n<Name> </Name>\r\n<Val></Val>\r\n</String>\r\n<String>\r\n<Name> </Name>\r\n<Val></Val>\r\n</String>\r\n<String>\r\n<Name> </Name>\r\n<Val></Val>\r\n</String>\r\n<String>\r\n<Name> </Name>\r\n<Val></Val>\r\n</String>\r\n<String>\r\n<Name> </Name>\r\n<Val></Val>\r\n</String>\r\n<String>\r\n<Name> </Name>\r\n<Val></Val>\r\n</String>\r\n<String>\r\n<Name> </Name>\r\n<Val></Val>\r\n</String>\r\n<String>\r\n<Name> </Name>\r\n<Val></Val>\r\n</String>\r\n<String>\r\n<Name> </Name>\r\n<Val></Val>\r\n</String>\r\n<String>\r\n<Name> </Name>\r\n<Val></Val>\r\n</String>\r\n<String>\r\n<Name> </Name>\r\n<Val></Val>\r\n</String>\r\n<String>\r\n<Name> </Name>\r\n<Val></Val>\r\n</String>\r\n<String>\r\n<Name> </Name>\r\n<Val></Val>\r\n</String>\r\n<String>\r\n<Name> </Name>\r\n<Val></Val>\r\n</String>\r\n<String>\r\n<Name> </Name>\r\n<Val></Val>\r\n</String>\r\n<String>\r\n<Name> </Name>\r\n<Val></Val>\r\n</String>\r\n<String>\r\n<Name> </Name>\r\n<Val></Val>\r\n</String>\r\n<String>\r\n<Name> </Name>\r\n<Val></Val>\r\n</String>\r\n<String>\r\n<Name> </Name>\r\n<Val></Val>\r\n</String>\r\n<String>\r\n<Name> </Name>\r\n<Val></Val>\r\n</String>\r\n<String>\r\n<Name> </Name>\r\n<Val></Val>\r\n</String>\r\n<String>\r\n<Name> </Name>\r\n<Val></Val>\r\n</String>\r\n<String>\r\n<Name> </Name>\r\n<Val></Val>\r\n</String>\r\n<String>\r\n<Name> </Name>\r\n<Val></Val>\r\n</String>\r\n<String>\r\n<Name> </Name>\r\n<Val></Val>\r\n</String>\r\n<String>\r\n<Name> </Name>\r\n<Val></Val>\r\n</String>\r\n<String>\r\n<Name> </Name>\r\n<Val></Val>\r\n</String>\r\n<String>\r\n<Name> </Name>\r\n<Val></Val>\r\n</String>\r\n<String>\r\n<Name> </Name>\r\n<Val></Val>\r\n</String>\r\n<String>\r\n<Name> </Name>\r\n<Val></Val>\r\n</String>\r\n<String>\r\n<Name> </Name>\r\n<Val></Val>\r\n</String>\r\n<String>\r\n<Name> </Name>\r\n<Val></Val>\r\n</String>\r\n<String>\r\n<Name> </Name>\r\n<Val></Val>\r\n</String>\r\n<String>\r\n<Name> </Name>\r\n<Val></Val>\r\n</String>\r\n<String>\r\n<Name> </Name>\r\n<Val></Val>\r\n</String>\r\n<String>\r\n<Name> </Name>\r\n<Val></Val>\r\n</String>\r\n<String>\r\n<Name> </Name>\r\n<Val></Val>\r\n</String>\r\n<String>\r\n<Name> </Name>\r\n<Val></Val>\r\n</String>\r\n<String>\r\n<Name> </Name>\r\n<Val></Val>\r\n</String>\r\n<String>\r\n<Name> </Name>\r\n<Val></Val>\r\n</String>\r\n<String>\r\n<Name> </Name>\r\n<Val></Val>\r\n</String>\r\n<String>\r\n<Name> </Name>\r\n<Val></Val>\r\n</String>\r\n<String>\r\n<Name> </Name>\r\n<Val></Val>\r\n</String>\r\n<String>\r\n<Name> </Name>\r\n<Val></Val>\r\n</String>\r\n<String>\r\n<Name> </Name>\r\n<Val></Val>\r\n</String>\r\n<String>\r\n<Name> </Name>\r\n<Val></Val>\r\n</String>\r\n<String>\r\n<Name> </Name>\r\n<Val></Val>\r\n</String>\r\n<String>\r\n<Name> </Name>\r\n<Val></Val>\r\n</String>\r\n<String>\r\n<Name> </Name>\r\n<Val></Val>\r\n</String>\r\n<String>\r\n<Name> </Name>\r\n<Val></Val>\r\n</String>\r\n<String>\r\n<Name> </Name>\r\n<Val></Val>\r\n</String>\r\n<String>\r\n<Name> </Name>\r\n<Val></Val>\r\n</String>\r\n<String>\r\n<Name> </Name>\r\n<Val></Val>\r\n</String>\r\n<String>\r\n<Name> </Name>\r\n<Val></Val>\r\n</String>\r\n<String>\r\n<Name> </Name>\r\n<Val></Val>\r\n</String>\r\n<String>\r\n<Name> </Name>\r\n<Val></Val>\r\n</String>\r\n<String>\r\n<Name> </Name>\r\n<Val></Val>\r\n</String>\r\n<String>\r\n<Name> </Name>\r\n<Val></Val>\r\n</String>\r\n<String>\r\n<Name> </Name>\r\n<Val></Val>\r\n</String>\r\n<String>\r\n<Name> </Name>\r\n<Val></Val>\r\n</String>\r\n<String>\r\n<Name> </Name>\r\n<Val></Val>\r\n</String>\r\n<String>\r\n<Name> </Name>\r\n<Val></Val>\r\n</String>\r\n<String>\r\n<Name> </Name>\r\n<Val></Val>\r\n</String>\r\n<String>\r\n<Name> </Name>\r\n<Val></Val>\r\n</String>\r\n<String>\r\n<Name> </Name>\r\n<Val></Val>\r\n</String>\r\n<String>\r\n<Name> </Name>\r\n<Val></Val>\r\n</String>\r\n<String>\r\n<Name> </Name>\r\n<Val></Val>\r\n</String>\r\n<String>\r\n<Name> </Name>\r\n<Val></Val>\r\n</String>\r\n<String>\r\n<Name> </Name>\r\n<Val></Val>\r\n</String>\r\n<String>\r\n<Name> </Name>\r\n<Val></Val>\r\n</String>\r\n<String>\r\n<Name> </Name>\r\n<Val>49</Val>\r\n</String>\r\n<String>\r\n<Name> </Name>\r\n<Val>3.75</Val>\r\n</String>\r\n<String>\r\n<Name> </Name>\r\n<Val></Val>\r\n</String>\r\n<String>\r\n<Name> </Name>\r\n<Val>3.4</Val>\r\n</String>\r\n<String>\r\n<Name> </Name>\r\n<Val></Val>\r\n</String>\r\n<String>\r\n<Name> </Name>\r\n<Val></Val>\r\n</String>\r\n<String>\r\n<Name> </Name>\r\n<Val></Val>\r\n</String>\r\n<String>\r\n<Name> </Name>\r\n<Val></Val>\r\n</String>\r\n<String>\r\n<Name> </Name>\r\n<Val></Val>\r\n</String>\r\n<String>\r\n<Name> </Name>\r\n<Val></Val>\r\n</String>\r\n<String>\r\n<Name> </Name>\r\n<Val></Val>\r\n</String>\r\n<String>\r\n<Name> </Name>\r\n<Val></Val>\r\n</String>\r\n<String>\r\n<Name> </Name>\r\n<Val></Val>\r\n</String>\r\n<String>\r\n<Name> </Name>\r\n<Val></Val>\r\n</String>\r\n<String>\r\n<Name> </Name>\r\n<Val></Val>\r\n</String>\r\n<String>\r\n<Name> </Name>\r\n<Val></Val>\r\n</String>\r\n<String>\r\n<Name> </Name>\r\n<Val></Val>\r\n</String>\r\n<String>\r\n<Name> </Name>\r\n<Val></Val>\r\n</String>\r\n<String>\r\n<Name> </Name>\r\n<Val></Val>\r\n</String>\r\n<String>\r\n<Name> </Name>\r\n<Val></Val>\r\n</String>\r\n<String>\r\n<Name> </Name>\r\n<Val></Val>\r\n</String>\r\n<String>\r\n<Name> </Name>\r\n<Val></Val>\r\n</String>\r\n<String>\r\n<Name> </Name>\r\n<Val></Val>\r\n</String>\r\n<String>\r\n<Name> </Name>\r\n<Val></Val>\r\n</String>\r\n<String>\r\n<Name> </Name>\r\n<Val></Val>\r\n</String>\r\n<String>\r\n<Name> </Name>\r\n<Val></Val>\r\n</String>\r\n<String>\r\n<Name> </Name>\r\n<Val></Val>\r\n</String>\r\n<String>\r\n<Name> </Name>\r\n<Val></Val>\r\n</String>\r\n<String>\r\n<Name> </Name>\r\n<Val></Val>\r\n</String>\r\n<String>\r\n<Name> </Name>\r\n<Val></Val>\r\n</String>\r\n<String>\r\n<Name> </Name>\r\n<Val></Val>\r\n</String>\r\n<String>\r\n<Name> </Name>\r\n<Val></Val>\r\n</String>\r\n<String>\r\n<Name> </Name>\r\n<Val></Val>\r\n</String>\r\n<String>\r\n<Name> </Name>\r\n<Val></Val>\r\n</String>\r\n<String>\r\n<Name> </Name>\r\n<Val></Val>\r\n</String>\r\n<String>\r\n<Name> </Name>\r\n<Val></Val>\r\n</String>\r\n<String>\r\n<Name> </Name>\r\n<Val></Val>\r\n</String>\r\n<String>\r\n<Name> </Name>\r\n<Val></Val>\r\n</String>\r\n<String>\r\n<Name> </Name>\r\n<Val></Val>\r\n</String>\r\n<String>\r\n<Name> </Name>\r\n<Val></Val>\r\n</String>\r\n<String>\r\n<Name> </Name>\r\n<Val></Val>\r\n</String>\r\n<String>\r\n<Name> </Name>\r\n<Val></Val>\r\n</String>\r\n<String>\r\n<Name> </Name>\r\n<Val></Val>\r\n</String>\r\n<String>\r\n<Name> </Name>\r\n<Val></Val>\r\n</String>\r\n<String>\r\n<Name> </Name>\r\n<Val></Val>\r\n</String>\r\n<String>\r\n<Name> </Name>\r\n<Val></Val>\r\n</String>\r\n<String>\r\n<Name> </Name>\r\n<Val></Val>\r\n</String>\r\n<String>\r\n<Name> </Name>\r\n<Val></Val>\r\n</String>\r\n<String>\r\n<Name> </Name>\r\n<Val>50</Val>\r\n</String>\r\n<String>\r\n<Name> </Name>\r\n<Val></Val>\r\n</String>\r\n<String>\r\n<Name> </Name>\r\n<Val></Val>\r\n</String>\r\n<String>\r\n<Name> </Name>\r\n<Val></Val>\r\n</String>\r\n<String>\r\n<Name> </Name>\r\n<Val></Val>\r\n</String>\r\n<String>\r\n<Name> </Name>\r\n<Val></Val>\r\n</String>\r\n<String>\r\n<Name> </Name>\r\n<Val></Val>\r\n</String>\r\n<String>\r\n<Name> </Name>\r\n<Val></Val>\r\n</String>\r\n<String>\r\n<Name> </Name>\r\n<Val></Val>\r\n</String>\r\n<String>\r\n<Name> </Name>\r\n<Val></Val>\r\n</String>\r\n<String>\r\n<Name> </Name>\r\n<Val></Val>\r\n</String>\r\n<String>\r\n<Name> </Name>\r\n<Val></Val>\r\n</String>\r\n<String>\r\n<Name> </Name>\r\n<Val></Val>\r\n</String>\r\n<String>\r\n<Name> </Name>\r\n<Val></Val>\r\n</String>\r\n<String>\r\n<Name> </Name>\r\n<Val></Val>\r\n</String>\r\n<String>\r\n<Name> </Name>\r\n<Val></Val>\r\n</String>\r\n<String>\r\n<Name> </Name>\r\n<Val></Val>\r\n</String>\r\n<String>\r\n<Name> </Name>\r\n<Val></Val>\r\n</String>\r\n<String>\r\n<Name> </Name>\r\n<Val></Val>\r\n</String>\r\n<String>\r\n<Name> </Name>\r\n<Val></Val>\r\n</String>\r\n<String>\r\n<Name> </Name>\r\n<Val></Val>\r\n</String>\r\n<String>\r\n<Name> </Name>\r\n<Val></Val>\r\n</String>\r\n<String>\r\n<Name> </Name>\r\n<Val></Val>\r\n</String>\r\n<String>\r\n<Name> </Name>\r\n<Val></Val>\r\n</String>\r\n<String>\r\n<Name> </Name>\r\n<Val></Val>\r\n</String>\r\n<String>\r\n<Name> </Name>\r\n<Val></Val>\r\n</String>\r\n<String>\r\n<Name> </Name>\r\n<Val></Val>\r\n</String>\r\n<String>\r\n<Name> </Name>\r\n<Val></Val>\r\n</String>\r\n<String>\r\n<Name> </Name>\r\n<Val></Val>\r\n</String>\r\n<String>\r\n<Name> </Name>\r\n<Val></Val>\r\n</String>\r\n<String>\r\n<Name> </Name>\r\n<Val></Val>\r\n</String>\r\n<String>\r\n<Name> </Name>\r\n<Val></Val>\r\n</String>\r\n<String>\r\n<Name> </Name>\r\n<Val></Val>\r\n</String>\r\n<String>\r\n<Name> </Name>\r\n<Val></Val>\r\n</String>\r\n<String>\r\n<Name> </Name>\r\n<Val></Val>\r\n</String>\r\n<String>\r\n<Name> </Name>\r\n<Val></Val>\r\n</String>\r\n<String>\r\n<Name> </Name>\r\n<Val></Val>\r\n</String>\r\n<String>\r\n<Name> </Name>\r\n<Val></Val>\r\n</String>\r\n<String>\r\n<Name> </Name>\r\n<Val></Val>\r\n</String>\r\n<String>\r\n<Name> </Name>\r\n<Val></Val>\r\n</String>\r\n<String>\r\n<Name> </Name>\r\n<Val></Val>\r\n</String>\r\n<String>\r\n<Name> </Name>\r\n<Val></Val>\r\n</String>\r\n<String>\r\n<Name> </Name>\r\n<Val></Val>\r\n</String>\r\n<String>\r\n<Name> </Name>\r\n<Val></Val>\r\n</String>\r\n<String>\r\n<Name> </Name>\r\n<Val></Val>\r\n</String>\r\n<String>\r\n<Name> </Name>\r\n<Val></Val>\r\n</String>\r\n<String>\r\n<Name> </Name>\r\n<Val></Val>\r\n</String>\r\n<String>\r\n<Name> </Name>\r\n<Val></Val>\r\n</String>\r\n<String>\r\n<Name> </Name>\r\n<Val></Val>\r\n</String>\r\n<String>\r\n<Name> </Name>\r\n<Val></Val>\r\n</String>\r\n<String>\r\n<Name> </Name>\r\n<Val></Val>\r\n</String>\r\n<String>\r\n<Name> </Name>\r\n<Val></Val>\r\n</String>\r\n<String>\r\n<Name> </Name>\r\n<Val></Val>\r\n</String>\r\n<String>\r\n<Name> </Name>\r\n<Val></Val>\r\n</String>\r\n<String>\r\n<Name> </Name>\r\n<Val></Val>\r\n</String>\r\n<String>\r\n<Name> </Name>\r\n<Val></Val>\r\n</String>\r\n<String>\r\n<Name> </Name>\r\n<Val></Val>\r\n</String>\r\n<String>\r\n<Name> </Name>\r\n<Val></Val>\r\n</String>\r\n<String>\r\n<Name> </Name>\r\n<Val></Val>\r\n</String>\r\n<String>\r\n<Name> </Name>\r\n<Val></Val>\r\n</String>\r\n<String>\r\n<Name> </Name>\r\n<Val></Val>\r\n</String>\r\n<String>\r\n<Name> </Name>\r\n<Val></Val>\r\n</String>\r\n<String>\r\n<Name> </Name>\r\n<Val></Val>\r\n</String>\r\n<String>\r\n<Name> </Name>\r\n<Val></Val>\r\n</String>\r\n<String>\r\n<Name> </Name>\r\n<Val></Val>\r\n</String>\r\n<String>\r\n<Name> </Name>\r\n<Val></Val>\r\n</String>\r\n<String>\r\n<Name> </Name>\r\n<Val></Val>\r\n</String>\r\n<String>\r\n<Name> </Name>\r\n<Val></Val>\r\n</String>\r\n<String>\r\n<Name> </Name>\r\n<Val></Val>\r\n</String>\r\n<String>\r\n<Name> </Name>\r\n<Val></Val>\r\n</String>\r\n<String>\r\n<Name> </Name>\r\n<Val></Val>\r\n</String>\r\n<String>\r\n<Name> </Name>\r\n<Val></Val>\r\n</String>\r\n<String>\r\n<Name> </Name>\r\n<Val></Val>\r\n</String>\r\n<String>\r\n<Name> </Name>\r\n<Val></Val>\r\n</String>\r\n<String>\r\n<Name> </Name>\r\n<Val></Val>\r\n</String>\r\n<String>\r\n<Name> </Name>\r\n<Val></Val>\r\n</String>\r\n<String>\r\n<Name> </Name>\r\n<Val></Val>\r\n</String>\r\n<String>\r\n<Name> </Name>\r\n<Val></Val>\r\n</String>\r\n<String>\r\n<Name> </Name>\r\n<Val></Val>\r\n</String>\r\n<String>\r\n<Name> </Name>\r\n<Val></Val>\r\n</String>\r\n<String>\r\n<Name> </Name>\r\n<Val></Val>\r\n</String>\r\n<String>\r\n<Name> </Name>\r\n<Val></Val>\r\n</String>\r\n<String>\r\n<Name> </Name>\r\n<Val></Val>\r\n</String>\r\n<String>\r\n<Name> </Name>\r\n<Val></Val>\r\n</String>\r\n<String>\r\n<Name> </Name>\r\n<Val></Val>\r\n</String>\r\n<String>\r\n<Name> </Name>\r\n<Val></Val>\r\n</String>\r\n<String>\r\n<Name> </Name>\r\n<Val></Val>\r\n</String>\r\n<String>\r\n<Name> </Name>\r\n<Val></Val>\r\n</String>\r\n<String>\r\n<Name> </Name>\r\n<Val></Val>\r\n</String>\r\n<String>\r\n<Name> </Name>\r\n<Val></Val>\r\n</String>\r\n<String>\r\n<Name> </Name>\r\n<Val></Val>\r\n</String>\r\n<String>\r\n<Name> </Name>\r\n<Val></Val>\r\n</String>\r\n<String>\r\n<Name> </Name>\r\n<Val></Val>\r\n</String>\r\n<String>\r\n<Name> </Name>\r\n<Val></Val>\r\n</String>\r\n<String>\r\n<Name> </Name>\r\n<Val></Val>\r\n</String>\r\n<String>\r\n<Name> </Name>\r\n<Val></Val>\r\n</String>\r\n<String>\r\n<Name> </Name>\r\n<Val></Val>\r\n</String>\r\n<String>\r\n<Name> </Name>\r\n<Val></Val>\r\n</String>\r\n<String>\r\n<Name> </Name>\r\n<Val></Val>\r\n</String>\r\n<String>\r\n<Name> </Name>\r\n<Val></Val>\r\n</String>\r\n<String>\r\n<Name> </Name>\r\n<Val></Val>\r\n</String>\r\n<String>\r\n<Name> </Name>\r\n<Val></Val>\r\n</String>\r\n<String>\r\n<Name> </Name>\r\n<Val></Val>\r\n</String>\r\n<String>\r\n<Name> </Name>\r\n<Val></Val>\r\n</String>\r\n<String>\r\n<Name> </Name>\r\n<Val></Val>\r\n</String>\r\n<String>\r\n<Name> </Name>\r\n<Val></Val>\r\n</String>\r\n<String>\r\n<Name> </Name>\r\n<Val></Val>\r\n</String>\r\n<String>\r\n<Name> </Name>\r\n<Val></Val>\r\n</String>\r\n<String>\r\n<Name> </Name>\r\n<Val></Val>\r\n</String>\r\n<String>\r\n<Name> </Name>\r\n<Val></Val>\r\n</String>\r\n<String>\r\n<Name> </Name>\r\n<Val></Val>\r\n</String>\r\n<String>\r\n<Name> </Name>\r\n<Val></Val>\r\n</String>\r\n<String>\r\n<Name> </Name>\r\n<Val></Val>\r\n</String>\r\n<String>\r\n<Name> </Name>\r\n<Val></Val>\r\n</String>\r\n<String>\r\n<Name> </Name>\r\n<Val></Val>\r\n</String>\r\n<String>\r\n<Name> </Name>\r\n<Val></Val>\r\n</String>\r\n<String>\r\n<Name> </Name>\r\n<Val></Val>\r\n</String>\r\n<String>\r\n<Name> </Name>\r\n<Val></Val>\r\n</String>\r\n<String>\r\n<Name> </Name>\r\n<Val></Val>\r\n</String>\r\n<String>\r\n<Name> </Name>\r\n<Val></Val>\r\n</String>\r\n<String>\r\n<Name> </Name>\r\n<Val></Val>\r\n</String>\r\n<String>\r\n<Name> </Name>\r\n<Val></Val>\r\n</String>\r\n<String>\r\n<Name> </Name>\r\n<Val></Val>\r\n</String>\r\n<String>\r\n<Name> </Name>\r\n<Val></Val>\r\n</String>\r\n<String>\r\n<Name> </Name>\r\n<Val></Val>\r\n</String>\r\n<String>\r\n<Name> </Name>\r\n<Val></Val>\r\n</String>\r\n<String>\r\n<Name> </Name>\r\n<Val></Val>\r\n</String>\r\n<String>\r\n<Name> </Name>\r\n<Val></Val>\r\n</String>\r\n<String>\r\n<Name> </Name>\r\n<Val></Val>\r\n</String>\r\n<String>\r\n<Name> </Name>\r\n<Val></Val>\r\n</String>\r\n<String>\r\n<Name> </Name>\r\n<Val></Val>\r\n</String>\r\n<String>\r\n<Name> </Name>\r\n<Val></Val>\r\n</String>\r\n<String>\r\n<Name> </Name>\r\n<Val></Val>\r\n</String>\r\n<String>\r\n<Name> </Name>\r\n<Val></Val>\r\n</String>\r\n<String>\r\n<Name> </Name>\r\n<Val></Val>\r\n</String>\r\n<String>\r\n<Name> </Name>\r\n<Val></Val>\r\n</String>\r\n<String>\r\n<Name> </Name>\r\n<Val></Val>\r\n</String>\r\n<String>\r\n<Name> </Name>\r\n<Val></Val>\r\n</String>\r\n<String>\r\n<Name> </Name>\r\n<Val></Val>\r\n</String>\r\n<String>\r\n<Name> </Name>\r\n<Val>-6.75</Val>\r\n</String>\r\n<String>\r\n<Name> </Name>\r\n<Val></Val>\r\n</String>\r\n<String>\r\n<Name> </Name>\r\n<Val></Val>\r\n</String>\r\n<String>\r\n<Name> </Name>\r\n<Val></Val>\r\n</String>\r\n<String>\r\n<Name> </Name>\r\n<Val></Val>\r\n</String>\r\n<String>\r\n<Name> </Name>\r\n<Val></Val>\r\n</String>\r\n<String>\r\n<Name> </Name>\r\n<Val></Val>\r\n</String>\r\n<String>\r\n<Name> </Name>\r\n<Val></Val>\r\n</String>\r\n<String>\r\n<Name> </Name>\r\n<Val></Val>\r\n</String>\r\n<String>\r\n<Name> </Name>\r\n<Val></Val>\r\n</String>\r\n<String>\r\n<Name> </Name>\r\n<Val></Val>\r\n</String>\r\n<String>\r\n<Name> </Name>\r\n<Val></Val>\r\n</String>\r\n<String>\r\n<Name> </Name>\r\n<Val>-6.75</Val>\r\n</String>\r\n<String>\r\n<Name> </Name>\r\n<Val></Val>\r\n</String>\r\n<String>\r\n<Name> </Name>\r\n<Val></Val>\r\n</String>\r\n<String>\r\n<Name> </Name>\r\n<Val></Val>\r\n</String>\r\n<String>\r\n<Name> </Name>\r\n<Val></Val>\r\n</String>\r\n<String>\r\n<Name> </Name>\r\n<Val></Val>\r\n</String>\r\n<String>\r\n<Name> </Name>\r\n<Val></Val>\r\n</String>\r\n<String>\r\n<Name> </Name>\r\n<Val></Val>\r\n</String>\r\n<String>\r\n<Name> </Name>\r\n<Val></Val>\r\n</String>\r\n<String>\r\n<Name> </Name>\r\n<Val></Val>\r\n</String>\r\n<String>\r\n<Name> </Name>\r\n<Val></Val>\r\n</String>\r\n<String>\r\n<Name> </Name>\r\n<Val></Val>\r\n</String>\r\n<String>\r\n<Name> </Name>\r\n<Val>-6.75</Val>\r\n</String>\r\n<String>\r\n<Name> </Name>\r\n<Val></Val>\r\n</String>\r\n<String>\r\n<Name> </Name>\r\n<Val></Val>\r\n</String>\r\n<String>\r\n<Name> </Name>\r\n<Val></Val>\r\n</String>\r\n<String>\r\n<Name> </Name>\r\n<Val></Val>\r\n</String>\r\n<String>\r\n<Name> </Name>\r\n<Val></Val>\r\n</String>\r\n<String>\r\n<Name> </Name>\r\n<Val></Val>\r\n</String>\r\n<String>\r\n<Name> </Name>\r\n<Val></Val>\r\n</String>\r\n<String>\r\n<Name> </Name>\r\n<Val></Val>\r\n</String>\r\n<String>\r\n<Name> </Name>\r\n<Val></Val>\r\n</String>\r\n<String>\r\n<Name> </Name>\r\n<Val></Val>\r\n</String>\r\n<String>\r\n<Name> </Name>\r\n<Val></Val>\r\n</String>\r\n<String>\r\n<Name> </Name>\r\n<Val>-6.75</Val>\r\n</String>\r\n<String>\r\n<Name> </Name>\r\n<Val></Val>\r\n</String>\r\n<String>\r\n<Name> </Name>\r\n<Val></Val>\r\n</String>\r\n<String>\r\n<Name> </Name>\r\n<Val></Val>\r\n</String>\r\n<String>\r\n<Name> </Name>\r\n<Val></Val>\r\n</String>\r\n<String>\r\n<Name> </Name>\r\n<Val></Val>\r\n</String>\r\n<String>\r\n<Name> </Name>\r\n<Val></Val>\r\n</String>\r\n<String>\r\n<Name> </Name>\r\n<Val></Val>\r\n</String>\r\n<String>\r\n<Name> </Name>\r\n<Val></Val>\r\n</String>\r\n<String>\r\n<Name> </Name>\r\n<Val></Val>\r\n</String>\r\n<String>\r\n<Name> </Name>\r\n<Val></Val>\r\n</String>\r\n<String>\r\n<Name> </Name>\r\n<Val></Val>\r\n</String>\r\n<String>\r\n<Name> </Name>\r\n<Val></Val>\r\n</String>\r\n<String>\r\n<Name> </Name>\r\n<Val></Val>\r\n</String>\r\n<String>\r\n<Name> </Name>\r\n<Val>-6.75</Val>\r\n</String>\r\n<String>\r\n<Name> </Name>\r\n<Val></Val>\r\n</String>\r\n<String>\r\n<Name> </Name>\r\n<Val></Val>\r\n</String>\r\n<String>\r\n<Name> </Name>\r\n<Val></Val>\r\n</String>\r\n<String>\r\n<Name> </Name>\r\n<Val></Val>\r\n</String>\r\n<String>\r\n<Name> </Name>\r\n<Val></Val>\r\n</String>\r\n<String>\r\n<Name> </Name>\r\n<Val></Val>\r\n</String>\r\n<String>\r\n<Name> </Name>\r\n<Val></Val>\r\n</String>\r\n<String>\r\n<Name> </Name>\r\n<Val></Val>\r\n</String>\r\n<String>\r\n<Name> </Name>\r\n<Val></Val>\r\n</String>\r\n<String>\r\n<Name> </Name>\r\n<Val></Val>\r\n</String>\r\n<String>\r\n<Name> </Name>\r\n<Val></Val>\r\n</String>\r\n<String>\r\n<Name> </Name>\r\n<Val>-6.75</Val>\r\n</String>\r\n<String>\r\n<Name> </Name>\r\n<Val></Val>\r\n</String>\r\n<String>\r\n<Name> </Name>\r\n<Val></Val>\r\n</String>\r\n<String>\r\n<Name> </Name>\r\n<Val></Val>\r\n</String>\r\n<String>\r\n<Name> </Name>\r\n<Val></Val>\r\n</String>\r\n<String>\r\n<Name> </Name>\r\n<Val></Val>\r\n</String>\r\n<String>\r\n<Name> </Name>\r\n<Val></Val>\r\n</String>\r\n<String>\r\n<Name> </Name>\r\n<Val></Val>\r\n</String>\r\n<String>\r\n<Name> </Name>\r\n<Val></Val>\r\n</String>\r\n<String>\r\n<Name> </Name>\r\n<Val></Val>\r\n</String>\r\n<String>\r\n<Name> </Name>\r\n<Val></Val>\r\n</String>\r\n<String>\r\n<Name> </Name>\r\n<Val></Val>\r\n</String>\r\n<String>\r\n<Name> </Name>\r\n<Val>-6.75</Val>\r\n</String>\r\n<String>\r\n<Name> </Name>\r\n<Val></Val>\r\n</String>\r\n<String>\r\n<Name> </Name>\r\n<Val></Val>\r\n</String>\r\n<String>\r\n<Name> </Name>\r\n<Val></Val>\r\n</String>\r\n<String>\r\n<Name> </Name>\r\n<Val></Val>\r\n</String>\r\n<String>\r\n<Name> </Name>\r\n<Val></Val>\r\n</String>\r\n<String>\r\n<Name> </Name>\r\n<Val></Val>\r\n</String>\r\n<String>\r\n<Name> </Name>\r\n<Val></Val>\r\n</String>\r\n<String>\r\n<Name> </Name>\r\n<Val></Val>\r\n</String>\r\n<String>\r\n<Name> </Name>\r\n<Val></Val>\r\n</String>\r\n<String>\r\n<Name> </Name>\r\n<Val></Val>\r\n</String>\r\n<String>\r\n<Name> </Name>\r\n<Val></Val>\r\n</String>\r\n<String>\r\n<Name> </Name>\r\n<Val>-6.75</Val>\r\n</String>\r\n<String>\r\n<Name> </Name>\r\n<Val></Val>\r\n</String>\r\n<String>\r\n<Name> </Name>\r\n<Val></Val>\r\n</String>\r\n<String>\r\n<Name> </Name>\r\n<Val></Val>\r\n</String>\r\n<String>\r\n<Name> </Name>\r\n<Val></Val>\r\n</String>\r\n<String>\r\n<Name> </Name>\r\n<Val></Val>\r\n</String>\r\n<String>\r\n<Name> </Name>\r\n<Val></Val>\r\n</String>\r\n<String>\r\n<Name> </Name>\r\n<Val></Val>\r\n</String>\r\n<String>\r\n<Name> </Name>\r\n<Val></Val>\r\n</String>\r\n<String>\r\n<Name> </Name>\r\n<Val></Val>\r\n</String>\r\n<String>\r\n<Name> </Name>\r\n<Val></Val>\r\n</String>\r\n<String>\r\n<Name> </Name>\r\n<Val></Val>\r\n</String>\r\n<String>\r\n<Name> </Name>\r\n<Val></Val>\r\n</String>\r\n<String>\r\n<Name> </Name>\r\n<Val></Val>\r\n</String>\r\n<String>\r\n<Name> </Name>\r\n<Val>-6.75</Val>\r\n</String>\r\n<String>\r\n<Name> </Name>\r\n<Val></Val>\r\n</String>\r\n<String>\r\n<Name> </Name>\r\n<Val></Val>\r\n</String>\r\n<String>\r\n<Name> </Name>\r\n<Val></Val>\r\n</String>\r\n<String>\r\n<Name> </Name>\r\n<Val></Val>\r\n</String>\r\n<String>\r\n<Name> </Name>\r\n<Val></Val>\r\n</String>\r\n<String>\r\n<Name> </Name>\r\n<Val></Val>\r\n</String>\r\n<String>\r\n<Name> </Name>\r\n<Val></Val>\r\n</String>\r\n<String>\r\n<Name> </Name>\r\n<Val></Val>\r\n</String>\r\n<String>\r\n<Name> </Name>\r\n<Val></Val>\r\n</String>\r\n<String>\r\n<Name> </Name>\r\n<Val></Val>\r\n</String>\r\n<String>\r\n<Name> </Name>\r\n<Val></Val>\r\n</String>\r\n<String>\r\n<Name> </Name>\r\n<Val>-6.75</Val>\r\n</String>\r\n<String>\r\n<Name> </Name>\r\n<Val></Val>\r\n</String>\r\n<String>\r\n<Name> </Name>\r\n<Val></Val>\r\n</String>\r\n<String>\r\n<Name> </Name>\r\n<Val></Val>\r\n</String>\r\n<String>\r\n<Name> </Name>\r\n<Val></Val>\r\n</String>\r\n<String>\r\n<Name> </Name>\r\n<Val></Val>\r\n</String>\r\n<String>\r\n<Name> </Name>\r\n<Val></Val>\r\n</String>\r\n<String>\r\n<Name> </Name>\r\n<Val></Val>\r\n</String>\r\n<String>\r\n<Name> </Name>\r\n<Val></Val>\r\n</String>\r\n<String>\r\n<Name> </Name>\r\n<Val></Val>\r\n</String>\r\n<String>\r\n<Name> </Name>\r\n<Val></Val>\r\n</String>\r\n<String>\r\n<Name> </Name>\r\n<Val></Val>\r\n</String>\r\n<String>\r\n<Name> </Name>\r\n<Val>-6.75</Val>\r\n</String>\r\n<String>\r\n<Name> </Name>\r\n<Val></Val>\r\n</String>\r\n<String>\r\n<Name> </Name>\r\n<Val></Val>\r\n</String>\r\n<String>\r\n<Name> </Name>\r\n<Val></Val>\r\n</String>\r\n<String>\r\n<Name> </Name>\r\n<Val></Val>\r\n</String>\r\n<String>\r\n<Name> </Name>\r\n<Val></Val>\r\n</String>\r\n<String>\r\n<Name> </Name>\r\n<Val></Val>\r\n</String>\r\n<String>\r\n<Name> </Name>\r\n<Val></Val>\r\n</String>\r\n<String>\r\n<Name> </Name>\r\n<Val></Val>\r\n</String>\r\n<String>\r\n<Name> </Name>\r\n<Val></Val>\r\n</String>\r\n<String>\r\n<Name> </Name>\r\n<Val></Val>\r\n</String>\r\n<String>\r\n<Name> </Name>\r\n<Val></Val>\r\n</String>\r\n<String>\r\n<Name> </Name>\r\n<Val>-6.75</Val>\r\n</String>\r\n<String>\r\n<Name> </Name>\r\n<Val></Val>\r\n</String>\r\n<String>\r\n<Name> </Name>\r\n<Val></Val>\r\n</String>\r\n<String>\r\n<Name> </Name>\r\n<Val></Val>\r\n</String>\r\n<String>\r\n<Name> </Name>\r\n<Val></Val>\r\n</String>\r\n<String>\r\n<Name> </Name>\r\n<Val></Val>\r\n</String>\r\n<String>\r\n<Name> </Name>\r\n<Val></Val>\r\n</String>\r\n<String>\r\n<Name> </Name>\r\n<Val></Val>\r\n</String>\r\n<String>\r\n<Name> </Name>\r\n<Val></Val>\r\n</String>\r\n<String>\r\n<Name> </Name>\r\n<Val></Val>\r\n</String>\r\n<String>\r\n<Name> </Name>\r\n<Val></Val>\r\n</String>\r\n<String>\r\n<Name> </Name>\r\n<Val></Val>\r\n</String>\r\n<String>\r\n<Name> </Name>\r\n<Val></Val>\r\n</String>\r\n<String>\r\n<Name> </Name>\r\n<Val></Val>\r\n</String>\r\n<String>\r\n<Name> </Name>\r\n<Val>-6.75</Val>\r\n</String>\r\n<String>\r\n<Name> </Name>\r\n<Val></Val>\r\n</String>\r\n<String>\r\n<Name> </Name>\r\n<Val></Val>\r\n</String>\r\n<String>\r\n<Name> </Name>\r\n<Val></Val>\r\n</String>\r\n<String>\r\n<Name> </Name>\r\n<Val></Val>\r\n</String>\r\n<String>\r\n<Name> </Name>\r\n<Val></Val>\r\n</String>\r\n<String>\r\n<Name> </Name>\r\n<Val></Val>\r\n</String>\r\n<String>\r\n<Name> </Name>\r\n<Val></Val>\r\n</String>\r\n<String>\r\n<Name> </Name>\r\n<Val></Val>\r\n</String>\r\n<String>\r\n<Name> </Name>\r\n<Val></Val>\r\n</String>\r\n<String>\r\n<Name> </Name>\r\n<Val></Val>\r\n</String>\r\n<String>\r\n<Name> </Name>\r\n<Val></Val>\r\n</String>\r\n<String>\r\n<Name> </Name>\r\n<Val>-6.75</Val>\r\n</String>\r\n<String>\r\n<Name> </Name>\r\n<Val></Val>\r\n</String>\r\n<String>\r\n<Name> </Name>\r\n<Val></Val>\r\n</String>\r\n<String>\r\n<Name> </Name>\r\n<Val></Val>\r\n</String>\r\n<String>\r\n<Name> </Name>\r\n<Val></Val>\r\n</String>\r\n<String>\r\n<Name> </Name>\r\n<Val></Val>\r\n</String>\r\n<String>\r\n<Name> </Name>\r\n<Val></Val>\r\n</String>\r\n<String>\r\n<Name> </Name>\r\n<Val></Val>\r\n</String>\r\n<String>\r\n<Name> </Name>\r\n<Val></Val>\r\n</String>\r\n<String>\r\n<Name> </Name>\r\n<Val></Val>\r\n</String>\r\n<String>\r\n<Name> </Name>\r\n<Val></Val>\r\n</String>\r\n<String>\r\n<Name> </Name>\r\n<Val></Val>\r\n</String>\r\n<String>\r\n<Name> </Name>\r\n<Val>-6.75</Val>\r\n</String>\r\n<String>\r\n<Name> </Name>\r\n<Val></Val>\r\n</String>\r\n<String>\r\n<Name> </Name>\r\n<Val></Val>\r\n</String>\r\n<String>\r\n<Name> </Name>\r\n<Val></Val>\r\n</String>\r\n<String>\r\n<Name> </Name>\r\n<Val></Val>\r\n</String>\r\n<String>\r\n<Name> </Name>\r\n<Val></Val>\r\n</String>\r\n<String>\r\n<Name> </Name>\r\n<Val></Val>\r\n</String>\r\n<String>\r\n<Name> </Name>\r\n<Val></Val>\r\n</String>\r\n<String>\r\n<Name> </Name>\r\n<Val></Val>\r\n</String>\r\n<String>\r\n<Name> </Name>\r\n<Val></Val>\r\n</String>\r\n<String>\r\n<Name> </Name>\r\n<Val></Val>\r\n</String>\r\n<String>\r\n<Name> </Name>\r\n<Val></Val>\r\n</String>\r\n<String>\r\n<Name> </Name>\r\n<Val>-6.75</Val>\r\n</String>\r\n<String>\r\n<Name> </Name>\r\n<Val></Val>\r\n</String>\r\n<String>\r\n<Name> </Name>\r\n<Val></Val>\r\n</String>\r\n<String>\r\n<Name> </Name>\r\n<Val></Val>\r\n</String>\r\n<String>\r\n<Name> </Name>\r\n<Val></Val>\r\n</String>\r\n<String>\r\n<Name> </Name>\r\n<Val></Val>\r\n</String>\r\n<String>\r\n<Name> </Name>\r\n<Val></Val>\r\n</String>\r\n<String>\r\n<Name> </Name>\r\n<Val></Val>\r\n</String>\r\n<String>\r\n<Name> </Name>\r\n<Val></Val>\r\n</String>\r\n<String>\r\n<Name> </Name>\r\n<Val></Val>\r\n</String>\r\n<String>\r\n<Name> </Name>\r\n<Val></Val>\r\n</String>\r\n<String>\r\n<Name> </Name>\r\n<Val></Val>\r\n</String>\r\n<String>\r\n<Name> </Name>\r\n<Val></Val>\r\n</String>\r\n<String>\r\n<Name> </Name>\r\n<Val></Val>\r\n</String>\r\n<String>\r\n<Name> </Name>\r\n<Val></Val>\r\n</String>\r\n<String>\r\n<Name> </Name>\r\n<Val></Val>\r\n</String>\r\n<String>\r\n<Name> </Name>\r\n<Val></Val>\r\n</String>\r\n<String>\r\n<Name> </Name>\r\n<Val></Val>\r\n</String>\r\n<String>\r\n<Name> </Name>\r\n<Val></Val>\r\n</String>\r\n<String>\r\n<Name> </Name>\r\n<Val></Val>\r\n</String>\r\n<String>\r\n<Name> </Name>\r\n<Val></Val>\r\n</String>\r\n<String>\r\n<Name> </Name>\r\n<Val></Val>\r\n</String>\r\n<String>\r\n<Name> </Name>\r\n<Val></Val>\r\n</String>\r\n<String>\r\n<Name> </Name>\r\n<Val></Val>\r\n</String>\r\n<String>\r\n<Name> </Name>\r\n<Val></Val>\r\n</String>\r\n<String>\r\n<Name> </Name>\r\n<Val></Val>\r\n</String>\r\n<String>\r\n<Name> </Name>\r\n<Val></Val>\r\n</String>\r\n<String>\r\n<Name> </Name>\r\n<Val></Val>\r\n</String>\r\n<String>\r\n<Name> </Name>\r\n<Val></Val>\r\n</String>\r\n<String>\r\n<Name> </Name>\r\n<Val></Val>\r\n</String>\r\n<String>\r\n<Name> </Name>\r\n<Val></Val>\r\n</String>\r\n<String>\r\n<Name> </Name>\r\n<Val></Val>\r\n</String>\r\n<String>\r\n<Name> </Name>\r\n<Val></Val>\r\n</String>\r\n<String>\r\n<Name> </Name>\r\n<Val></Val>\r\n</String>\r\n<String>\r\n<Name> </Name>\r\n<Val></Val>\r\n</String>\r\n<String>\r\n<Name> </Name>\r\n<Val></Val>\r\n</String>\r\n<String>\r\n<Name> </Name>\r\n<Val></Val>\r\n</String>\r\n<String>\r\n<Name> </Name>\r\n<Val></Val>\r\n</String>\r\n<String>\r\n<Name> </Name>\r\n<Val></Val>\r\n</String>\r\n<String>\r\n<Name> </Name>\r\n<Val></Val>\r\n</String>\r\n<String>\r\n<Name> </Name>\r\n<Val></Val>\r\n</String>\r\n<String>\r\n<Name> </Name>\r\n<Val></Val>\r\n</String>\r\n<String>\r\n<Name> </Name>\r\n<Val></Val>\r\n</String>\r\n<String>\r\n<Name> </Name>\r\n<Val></Val>\r\n</String>\r\n<String>\r\n<Name> </Name>\r\n<Val></Val>\r\n</String>\r\n<String>\r\n<Name> </Name>\r\n<Val></Val>\r\n</String>\r\n<String>\r\n<Name> </Name>\r\n<Val></Val>\r\n</String>\r\n<String>\r\n<Name> </Name>\r\n<Val></Val>\r\n</String>\r\n<String>\r\n<Name> </Name>\r\n<Val></Val>\r\n</String>\r\n<String>\r\n<Name> </Name>\r\n<Val></Val>\r\n</String>\r\n<String>\r\n<Name> </Name>\r\n<Val></Val>\r\n</String>\r\n<String>\r\n<Name> </Name>\r\n<Val></Val>\r\n</String>\r\n<String>\r\n<Name> </Name>\r\n<Val></Val>\r\n</String>\r\n<String>\r\n<Name> </Name>\r\n<Val></Val>\r\n</String>\r\n<String>\r\n<Name> </Name>\r\n<Val></Val>\r\n</String>\r\n<String>\r\n<Name> </Name>\r\n<Val></Val>\r\n</String>\r\n<String>\r\n<Name> </Name>\r\n<Val></Val>\r\n</String>\r\n<String>\r\n<Name> </Name>\r\n<Val></Val>\r\n</String>\r\n<String>\r\n<Name> </Name>\r\n<Val></Val>\r\n</String>\r\n<String>\r\n<Name> </Name>\r\n<Val></Val>\r\n</String>\r\n<String>\r\n<Name> </Name>\r\n<Val></Val>\r\n</String>\r\n<String>\r\n<Name> </Name>\r\n<Val></Val>\r\n</String>\r\n<String>\r\n<Name> </Name>\r\n<Val></Val>\r\n</String>\r\n<String>\r\n<Name> </Name>\r\n<Val></Val>\r\n</String>\r\n<String>\r\n<Name> </Name>\r\n<Val></Val>\r\n</String>\r\n<String>\r\n<Name> </Name>\r\n<Val></Val>\r\n</String>\r\n<String>\r\n<Name> </Name>\r\n<Val></Val>\r\n</String>\r\n<String>\r\n<Name> </Name>\r\n<Val></Val>\r\n</String>\r\n<String>\r\n<Name> </Name>\r\n<Val></Val>\r\n</String>\r\n<String>\r\n<Name> </Name>\r\n<Val></Val>\r\n</String>\r\n<String>\r\n<Name> </Name>\r\n<Val></Val>\r\n</String>\r\n<String>\r\n<Name> </Name>\r\n<Val></Val>\r\n</String>\r\n<String>\r\n<Name> </Name>\r\n<Val></Val>\r\n</String>\r\n<String>\r\n<Name> </Name>\r\n<Val></Val>\r\n</String>\r\n<String>\r\n<Name> </Name>\r\n<Val></Val>\r\n</String>\r\n<String>\r\n<Name> </Name>\r\n<Val></Val>\r\n</String>\r\n<String>\r\n<Name> </Name>\r\n<Val></Val>\r\n</String>\r\n<String>\r\n<Name> </Name>\r\n<Val></Val>\r\n</String>\r\n<String>\r\n<Name> </Name>\r\n<Val></Val>\r\n</String>\r\n<String>\r\n<Name> </Name>\r\n<Val></Val>\r\n</String>\r\n<String>\r\n<Name> </Name>\r\n<Val></Val>\r\n</String>\r\n<String>\r\n<Name> </Name>\r\n<Val></Val>\r\n</String>\r\n<String>\r\n<Name> </Name>\r\n<Val></Val>\r\n</String>\r\n<String>\r\n<Name> </Name>\r\n<Val></Val>\r\n</String>\r\n<String>\r\n<Name> </Name>\r\n<Val></Val>\r\n</String>\r\n<String>\r\n<Name> </Name>\r\n<Val></Val>\r\n</String>\r\n<String>\r\n<Name> </Name>\r\n<Val></Val>\r\n</String>\r\n<String>\r\n<Name> </Name>\r\n<Val></Val>\r\n</String>\r\n<String>\r\n<Name> </Name>\r\n<Val></Val>\r\n</String>\r\n<String>\r\n<Name> </Name>\r\n<Val></Val>\r\n</String>\r\n<String>\r\n<Name> </Name>\r\n<Val></Val>\r\n</String>\r\n<String>\r\n<Name> </Name>\r\n<Val></Val>\r\n</String>\r\n<String>\r\n<Name> </Name>\r\n<Val></Val>\r\n</String>\r\n<String>\r\n<Name> </Name>\r\n<Val></Val>\r\n</String>\r\n<String>\r\n<Name> </Name>\r\n<Val></Val>\r\n</String>\r\n<String>\r\n<Name> </Name>\r\n<Val></Val>\r\n</String>\r\n<String>\r\n<Name> </Name>\r\n<Val></Val>\r\n</String>\r\n<String>\r\n<Name> </Name>\r\n<Val></Val>\r\n</String>\r\n<String>\r\n<Name> </Name>\r\n<Val></Val>\r\n</String>\r\n<String>\r\n<Name> </Name>\r\n<Val></Val>\r\n</String>\r\n<String>\r\n<Name> </Name>\r\n<Val></Val>\r\n</String>\r\n<String>\r\n<Name> </Name>\r\n<Val></Val>\r\n</String>\r\n<String>\r\n<Name> </Name>\r\n<Val></Val>\r\n</String>\r\n<String>\r\n<Name> </Name>\r\n<Val></Val>\r\n</String>\r\n<String>\r\n<Name> </Name>\r\n<Val></Val>\r\n</String>\r\n<String>\r\n<Name> </Name>\r\n<Val></Val>\r\n</String>\r\n<String>\r\n<Name> </Name>\r\n<Val></Val>\r\n</String>\r\n<String>\r\n<Name> </Name>\r\n<Val></Val>\r\n</String>\r\n<String>\r\n<Name> </Name>\r\n<Val></Val>\r\n</String>\r\n<String>\r\n<Name> </Name>\r\n<Val></Val>\r\n</String>\r\n<String>\r\n<Name> </Name>\r\n<Val></Val>\r\n</String>\r\n<String>\r\n<Name> </Name>\r\n<Val></Val>\r\n</String>\r\n<String>\r\n<Name> </Name>\r\n<Val></Val>\r\n</String>\r\n<String>\r\n<Name> </Name>\r\n<Val></Val>\r\n</String>\r\n<String>\r\n<Name> </Name>\r\n<Val></Val>\r\n</String>\r\n<String>\r\n<Name> </Name>\r\n<Val>240</Val>\r\n</String>\r\n<String>\r\n<Name> </Name>\r\n<Val></Val>\r\n</String>\r\n<String>\r\n<Name> </Name>\r\n<Val></Val>\r\n</String>\r\n<String>\r\n<Name> </Name>\r\n<Val></Val>\r\n</String>\r\n<String>\r\n<Name> </Name>\r\n<Val></Val>\r\n</String>\r\n<String>\r\n<Name> </Name>\r\n<Val>47</Val>\r\n</String>\r\n<String>\r\n<Name> </Name>\r\n<Val>0.4</Val>\r\n</String>\r\n<String>\r\n<Name> </Name>\r\n<Val></Val>\r\n</String>\r\n<String>\r\n<Name> </Name>\r\n<Val>3.2</Val>\r\n</String>\r\n<String>\r\n<Name> </Name>\r\n<Val></Val>\r\n</String>\r\n<String>\r\n<Name> </Name>\r\n<Val></Val>\r\n</String>\r\n<String>\r\n<Name> </Name>\r\n<Val></Val>\r\n</String>\r\n<String>\r\n<Name> </Name>\r\n<Val></Val>\r\n</String>\r\n<String>\r\n<Name> </Name>\r\n<Val></Val>\r\n</String>\r\n<String>\r\n<Name> </Name>\r\n<Val></Val>\r\n</String>\r\n<String>\r\n<Name> </Name>\r\n<Val></Val>\r\n</String>\r\n<String>\r\n<Name> </Name>\r\n<Val></Val>\r\n</String>\r\n<String>\r\n<Name> </Name>\r\n<Val></Val>\r\n</String>\r\n<String>\r\n<Name> </Name>\r\n<Val></Val>\r\n</String>\r\n<String>\r\n<Name> </Name>\r\n<Val></Val>\r\n</String>\r\n<String>\r\n<Name> </Name>\r\n<Val></Val>\r\n</String>\r\n<String>\r\n<Name> </Name>\r\n<Val></Val>\r\n</String>\r\n<String>\r\n<Name> </Name>\r\n<Val></Val>\r\n</String>\r\n<String>\r\n<Name> </Name>\r\n<Val></Val>\r\n</String>\r\n<String>\r\n<Name> </Name>\r\n<Val></Val>\r\n</String>\r\n<String>\r\n<Name> </Name>\r\n<Val></Val>\r\n</String>\r\n<String>\r\n<Name> </Name>\r\n<Val></Val>\r\n</String>\r\n<String>\r\n<Name> </Name>\r\n<Val></Val>\r\n</String>\r\n<String>\r\n<Name> </Name>\r\n<Val></Val>\r\n</String>\r\n<String>\r\n<Name> </Name>\r\n<Val></Val>\r\n</String>\r\n<String>\r\n<Name> </Name>\r\n<Val></Val>\r\n</String>\r\n<String>\r\n<Name> </Name>\r\n<Val></Val>\r\n</String>\r\n<String>\r\n<Name> </Name>\r\n<Val></Val>\r\n</String>\r\n<String>\r\n<Name> </Name>\r\n<Val></Val>\r\n</String>\r\n<String>\r\n<Name> </Name>\r\n<Val></Val>\r\n</String>\r\n<String>\r\n<Name> </Name>\r\n<Val></Val>\r\n</String>\r\n<String>\r\n<Name> </Name>\r\n<Val></Val>\r\n</String>\r\n<String>\r\n<Name> </Name>\r\n<Val></Val>\r\n</String>\r\n<String>\r\n<Name> </Name>\r\n<Val></Val>\r\n</String>\r\n<String>\r\n<Name> </Name>\r\n<Val></Val>\r\n</String>\r\n<String>\r\n<Name> </Name>\r\n<Val></Val>\r\n</String>\r\n<String>\r\n<Name> </Name>\r\n<Val></Val>\r\n</String>\r\n<String>\r\n<Name> </Name>\r\n<Val></Val>\r\n</String>\r\n<String>\r\n<Name> </Name>\r\n<Val></Val>\r\n</String>\r\n<String>\r\n<Name> </Name>\r\n<Val></Val>\r\n</String>\r\n<String>\r\n<Name> </Name>\r\n<Val></Val>\r\n</String>\r\n<String>\r\n<Name> </Name>\r\n<Val></Val>\r\n</String>\r\n<String>\r\n<Name> </Name>\r\n<Val></Val>\r\n</String>\r\n<String>\r\n<Name> </Name>\r\n<Val></Val>\r\n</String>\r\n<String>\r\n<Name> </Name>\r\n<Val></Val>\r\n</String>\r\n<String>\r\n<Name> </Name>\r\n<Val></Val>\r\n</String>\r\n<String>\r\n<Name> </Name>\r\n<Val></Val>\r\n</String>\r\n<String>\r\n<Name> </Name>\r\n<Val></Val>\r\n</String>\r\n<String>\r\n<Name> </Name>\r\n<Val>20</Val>\r\n</String>\r\n<String>\r\n<Name> </Name>\r\n<Val></Val>\r\n</String>\r\n<String>\r\n<Name> </Name>\r\n<Val></Val>\r\n</String>\r\n<String>\r\n<Name> </Name>\r\n<Val></Val>\r\n</String>\r\n<String>\r\n<Name> </Name>\r\n<Val></Val>\r\n</String>\r\n<String>\r\n<Name> </Name>\r\n<Val></Val>\r\n</String>\r\n<String>\r\n<Name> </Name>\r\n<Val></Val>\r\n</String>\r\n<String>\r\n<Name> </Name>\r\n<Val></Val>\r\n</String>\r\n<String>\r\n<Name> </Name>\r\n<Val></Val>\r\n</String>\r\n<String>\r\n<Name> </Name>\r\n<Val></Val>\r\n</String>\r\n<String>\r\n<Name> </Name>\r\n<Val></Val>\r\n</String>\r\n<String>\r\n<Name> </Name>\r\n<Val></Val>\r\n</String>\r\n<String>\r\n<Name> </Name>\r\n<Val></Val>\r\n</String>\r\n<String>\r\n<Name> </Name>\r\n<Val></Val>\r\n</String>\r\n<String>\r\n<Name> </Name>\r\n<Val></Val>\r\n</String>\r\n<String>\r\n<Name> </Name>\r\n<Val></Val>\r\n</String>\r\n<String>\r\n<Name> </Name>\r\n<Val></Val>\r\n</String>\r\n<String>\r\n<Name> </Name>\r\n<Val></Val>\r\n</String>\r\n<String>\r\n<Name> </Name>\r\n<Val></Val>\r\n</String>\r\n<String>\r\n<Name> </Name>\r\n<Val></Val>\r\n</String>\r\n<String>\r\n<Name> </Name>\r\n<Val></Val>\r\n</String>\r\n<String>\r\n<Name> </Name>\r\n<Val></Val>\r\n</String>\r\n<String>\r\n<Name> </Name>\r\n<Val></Val>\r\n</String>\r\n<String>\r\n<Name> </Name>\r\n<Val></Val>\r\n</String>\r\n<String>\r\n<Name> </Name>\r\n<Val></Val>\r\n</String>\r\n<String>\r\n<Name> </Name>\r\n<Val></Val>\r\n</String>\r\n<String>\r\n<Name> </Name>\r\n<Val></Val>\r\n</String>\r\n<String>\r\n<Name> </Name>\r\n<Val></Val>\r\n</String>\r\n<String>\r\n<Name> </Name>\r\n<Val></Val>\r\n</String>\r\n<String>\r\n<Name> </Name>\r\n<Val></Val>\r\n</String>\r\n<String>\r\n<Name> </Name>\r\n<Val></Val>\r\n</String>\r\n<String>\r\n<Name> </Name>\r\n<Val></Val>\r\n</String>\r\n<String>\r\n<Name> </Name>\r\n<Val></Val>\r\n</String>\r\n<String>\r\n<Name> </Name>\r\n<Val></Val>\r\n</String>\r\n<String>\r\n<Name> </Name>\r\n<Val></Val>\r\n</String>\r\n<String>\r\n<Name> </Name>\r\n<Val></Val>\r\n</String>\r\n<String>\r\n<Name> </Name>\r\n<Val></Val>\r\n</String>\r\n<String>\r\n<Name> </Name>\r\n<Val></Val>\r\n</String>\r\n<String>\r\n<Name> </Name>\r\n<Val></Val>\r\n</String>\r\n<String>\r\n<Name> </Name>\r\n<Val></Val>\r\n</String>\r\n<String>\r\n<Name> </Name>\r\n<Val></Val>\r\n</String>\r\n<String>\r\n<Name> </Name>\r\n<Val></Val>\r\n</String>\r\n<String>\r\n<Name> </Name>\r\n<Val></Val>\r\n</String>\r\n<String>\r\n<Name> </Name>\r\n<Val></Val>\r\n</String>\r\n<String>\r\n<Name> </Name>\r\n<Val></Val>\r\n</String>\r\n<String>\r\n<Name> </Name>\r\n<Val></Val>\r\n</String>\r\n<String>\r\n<Name> </Name>\r\n<Val></Val>\r\n</String>\r\n<String>\r\n<Name> </Name>\r\n<Val></Val>\r\n</String>\r\n<String>\r\n<Name> </Name>\r\n<Val></Val>\r\n</String>\r\n<String>\r\n<Name> </Name>\r\n<Val></Val>\r\n</String>\r\n<String>\r\n<Name> </Name>\r\n<Val></Val>\r\n</String>\r\n<String>\r\n<Name> </Name>\r\n<Val></Val>\r\n</String>\r\n<String>\r\n<Name> </Name>\r\n<Val></Val>\r\n</String>\r\n<String>\r\n<Name> </Name>\r\n<Val></Val>\r\n</String>\r\n<String>\r\n<Name> </Name>\r\n<Val></Val>\r\n</String>\r\n<String>\r\n<Name> </Name>\r\n<Val></Val>\r\n</String>\r\n<String>\r\n<Name> </Name>\r\n<Val></Val>\r\n</String>\r\n<String>\r\n<Name> </Name>\r\n<Val></Val>\r\n</String>\r\n<String>\r\n<Name> </Name>\r\n<Val></Val>\r\n</String>\r\n<String>\r\n<Name> </Name>\r\n<Val></Val>\r\n</String>\r\n<String>\r\n<Name> </Name>\r\n<Val></Val>\r\n</String>\r\n<String>\r\n<Name> </Name>\r\n<Val></Val>\r\n</String>\r\n<String>\r\n<Name> </Name>\r\n<Val></Val>\r\n</String>\r\n<String>\r\n<Name> </Name>\r\n<Val></Val>\r\n</String>\r\n<String>\r\n<Name> </Name>\r\n<Val></Val>\r\n</String>\r\n<String>\r\n<Name> </Name>\r\n<Val></Val>\r\n</String>\r\n<String>\r\n<Name> </Name>\r\n<Val></Val>\r\n</String>\r\n<String>\r\n<Name> </Name>\r\n<Val></Val>\r\n</String>\r\n<String>\r\n<Name> </Name>\r\n<Val></Val>\r\n</String>\r\n<String>\r\n<Name> </Name>\r\n<Val></Val>\r\n</String>\r\n<String>\r\n<Name> </Name>\r\n<Val></Val>\r\n</String>\r\n<String>\r\n<Name> </Name>\r\n<Val></Val>\r\n</String>\r\n<String>\r\n<Name> </Name>\r\n<Val></Val>\r\n</String>\r\n<String>\r\n<Name> </Name>\r\n<Val></Val>\r\n</String>\r\n<String>\r\n<Name> </Name>\r\n<Val></Val>\r\n</String>\r\n<String>\r\n<Name> </Name>\r\n<Val></Val>\r\n</String>\r\n<String>\r\n<Name> </Name>\r\n<Val></Val>\r\n</String>\r\n<String>\r\n<Name> </Name>\r\n<Val></Val>\r\n</String>\r\n<String>\r\n<Name> </Name>\r\n<Val></Val>\r\n</String>\r\n<String>\r\n<Name> </Name>\r\n<Val></Val>\r\n</String>\r\n<String>\r\n<Name> </Name>\r\n<Val></Val>\r\n</String>\r\n<String>\r\n<Name> </Name>\r\n<Val></Val>\r\n</String>\r\n<String>\r\n<Name> </Name>\r\n<Val></Val>\r\n</String>\r\n<String>\r\n<Name> </Name>\r\n<Val></Val>\r\n</String>\r\n<String>\r\n<Name> </Name>\r\n<Val></Val>\r\n</String>\r\n<String>\r\n<Name> </Name>\r\n<Val></Val>\r\n</String>\r\n<String>\r\n<Name> </Name>\r\n<Val></Val>\r\n</String>\r\n<String>\r\n<Name> </Name>\r\n<Val></Val>\r\n</String>\r\n<String>\r\n<Name> </Name>\r\n<Val></Val>\r\n</String>\r\n<String>\r\n<Name> </Name>\r\n<Val></Val>\r\n</String>\r\n<String>\r\n<Name> </Name>\r\n<Val></Val>\r\n</String>\r\n<String>\r\n<Name> </Name>\r\n<Val></Val>\r\n</String>\r\n<String>\r\n<Name> </Name>\r\n<Val></Val>\r\n</String>\r\n<String>\r\n<Name> </Name>\r\n<Val></Val>\r\n</String>\r\n<String>\r\n<Name> </Name>\r\n<Val></Val>\r\n</String>\r\n<String>\r\n<Name> </Name>\r\n<Val></Val>\r\n</String>\r\n<String>\r\n<Name> </Name>\r\n<Val></Val>\r\n</String>\r\n<String>\r\n<Name> </Name>\r\n<Val></Val>\r\n</String>\r\n<String>\r\n<Name> </Name>\r\n<Val></Val>\r\n</String>\r\n<String>\r\n<Name> </Name>\r\n<Val></Val>\r\n</String>\r\n<String>\r\n<Name> </Name>\r\n<Val></Val>\r\n</String>\r\n<String>\r\n<Name> </Name>\r\n<Val></Val>\r\n</String>\r\n<String>\r\n<Name> </Name>\r\n<Val></Val>\r\n</String>\r\n<String>\r\n<Name> </Name>\r\n<Val></Val>\r\n</String>\r\n<String>\r\n<Name> </Name>\r\n<Val></Val>\r\n</String>\r\n<String>\r\n<Name> </Name>\r\n<Val></Val>\r\n</String>\r\n<String>\r\n<Name> </Name>\r\n<Val></Val>\r\n</String>\r\n<String>\r\n<Name> </Name>\r\n<Val></Val>\r\n</String>\r\n<String>\r\n<Name> </Name>\r\n<Val></Val>\r\n</String>\r\n<String>\r\n<Name> </Name>\r\n<Val></Val>\r\n</String>\r\n<String>\r\n<Name> </Name>\r\n<Val></Val>\r\n</String>\r\n<String>\r\n<Name> </Name>\r\n<Val></Val>\r\n</String>\r\n<String>\r\n<Name> </Name>\r\n<Val></Val>\r\n</String>\r\n<String>\r\n<Name> </Name>\r\n<Val></Val>\r\n</String>\r\n<String>\r\n<Name> </Name>\r\n<Val></Val>\r\n</String>\r\n<String>\r\n<Name> </Name>\r\n<Val></Val>\r\n</String>\r\n<String>\r\n<Name> </Name>\r\n<Val></Val>\r\n</String>\r\n<String>\r\n<Name> </Name>\r\n<Val></Val>\r\n</String>\r\n<String>\r\n<Name> </Name>\r\n<Val></Val>\r\n</String>\r\n<String>\r\n<Name> </Name>\r\n<Val></Val>\r\n</String>\r\n<String>\r\n<Name> </Name>\r\n<Val></Val>\r\n</String>\r\n<String>\r\n<Name> </Name>\r\n<Val></Val>\r\n</String>\r\n<String>\r\n<Name> </Name>\r\n<Val></Val>\r\n</String>\r\n<String>\r\n<Name> </Name>\r\n<Val></Val>\r\n</String>\r\n<String>\r\n<Name> </Name>\r\n<Val></Val>\r\n</String>\r\n<String>\r\n<Name> </Name>\r\n<Val></Val>\r\n</String>\r\n<String>\r\n<Name> </Name>\r\n<Val></Val>\r\n</String>\r\n<String>\r\n<Name> </Name>\r\n<Val></Val>\r\n</String>\r\n<String>\r\n<Name> </Name>\r\n<Val></Val>\r\n</String>\r\n<String>\r\n<Name> </Name>\r\n<Val></Val>\r\n</String>\r\n<String>\r\n<Name> </Name>\r\n<Val></Val>\r\n</String>\r\n<String>\r\n<Name> </Name>\r\n<Val></Val>\r\n</String>\r\n<String>\r\n<Name> </Name>\r\n<Val>-20</Val>\r\n</String>\r\n<String>\r\n<Name> </Name>\r\n<Val></Val>\r\n</String>\r\n<String>\r\n<Name> </Name>\r\n<Val></Val>\r\n</String>\r\n<String>\r\n<Name> </Name>\r\n<Val></Val>\r\n</String>\r\n<String>\r\n<Name> </Name>\r\n<Val></Val>\r\n</String>\r\n<String>\r\n<Name> </Name>\r\n<Val></Val>\r\n</String>\r\n<String>\r\n<Name> </Name>\r\n<Val></Val>\r\n</String>\r\n<String>\r\n<Name> </Name>\r\n<Val></Val>\r\n</String>\r\n<String>\r\n<Name> </Name>\r\n<Val></Val>\r\n</String>\r\n<String>\r\n<Name> </Name>\r\n<Val></Val>\r\n</String>\r\n<String>\r\n<Name> </Name>\r\n<Val></Val>\r\n</String>\r\n<String>\r\n<Name> </Name>\r\n<Val></Val>\r\n</String>\r\n<String>\r\n<Name> </Name>\r\n<Val>-20</Val>\r\n</String>\r\n<String>\r\n<Name> </Name>\r\n<Val></Val>\r\n</String>\r\n<String>\r\n<Name> </Name>\r\n<Val></Val>\r\n</String>\r\n<String>\r\n<Name> </Name>\r\n<Val></Val>\r\n</String>\r\n<String>\r\n<Name> </Name>\r\n<Val></Val>\r\n</String>\r\n<String>\r\n<Name> </Name>\r\n<Val></Val>\r\n</String>\r\n<String>\r\n<Name> </Name>\r\n<Val></Val>\r\n</String>\r\n<String>\r\n<Name> </Name>\r\n<Val></Val>\r\n</String>\r\n<String>\r\n<Name> </Name>\r\n<Val></Val>\r\n</String>\r\n<String>\r\n<Name> </Name>\r\n<Val></Val>\r\n</String>\r\n<String>\r\n<Name> </Name>\r\n<Val></Val>\r\n</String>\r\n<String>\r\n<Name> </Name>\r\n<Val></Val>\r\n</String>\r\n<String>\r\n<Name> </Name>\r\n<Val>-20</Val>\r\n</String>\r\n<String>\r\n<Name> </Name>\r\n<Val></Val>\r\n</String>\r\n<String>\r\n<Name> </Name>\r\n<Val></Val>\r\n</String>\r\n<String>\r\n<Name> </Name>\r\n<Val></Val>\r\n</String>\r\n<String>\r\n<Name> </Name>\r\n<Val></Val>\r\n</String>\r\n<String>\r\n<Name> </Name>\r\n<Val></Val>\r\n</String>\r\n<String>\r\n<Name> </Name>\r\n<Val></Val>\r\n</String>\r\n<String>\r\n<Name> </Name>\r\n<Val></Val>\r\n</String>\r\n<String>\r\n<Name> </Name>\r\n<Val></Val>\r\n</String>\r\n<String>\r\n<Name> </Name>\r\n<Val></Val>\r\n</String>\r\n<String>\r\n<Name> </Name>\r\n<Val></Val>\r\n</String>\r\n<String>\r\n<Name> </Name>\r\n<Val></Val>\r\n</String>\r\n<String>\r\n<Name> </Name>\r\n<Val>-20</Val>\r\n</String>\r\n<String>\r\n<Name> </Name>\r\n<Val></Val>\r\n</String>\r\n<String>\r\n<Name> </Name>\r\n<Val></Val>\r\n</String>\r\n<String>\r\n<Name> </Name>\r\n<Val></Val>\r\n</String>\r\n<String>\r\n<Name> </Name>\r\n<Val></Val>\r\n</String>\r\n<String>\r\n<Name> </Name>\r\n<Val></Val>\r\n</String>\r\n<String>\r\n<Name> </Name>\r\n<Val></Val>\r\n</String>\r\n<String>\r\n<Name> </Name>\r\n<Val></Val>\r\n</String>\r\n<String>\r\n<Name> </Name>\r\n<Val></Val>\r\n</String>\r\n<String>\r\n<Name> </Name>\r\n<Val></Val>\r\n</String>\r\n<String>\r\n<Name> </Name>\r\n<Val></Val>\r\n</String>\r\n<String>\r\n<Name> </Name>\r\n<Val></Val>\r\n</String>\r\n<String>\r\n<Name> </Name>\r\n<Val></Val>\r\n</String>\r\n<String>\r\n<Name> </Name>\r\n<Val></Val>\r\n</String>\r\n<String>\r\n<Name> </Name>\r\n<Val>-20</Val>\r\n</String>\r\n<String>\r\n<Name> </Name>\r\n<Val></Val>\r\n</String>\r\n<String>\r\n<Name> </Name>\r\n<Val></Val>\r\n</String>\r\n<String>\r\n<Name> </Name>\r\n<Val></Val>\r\n</String>\r\n<String>\r\n<Name> </Name>\r\n<Val></Val>\r\n</String>\r\n<String>\r\n<Name> </Name>\r\n<Val></Val>\r\n</String>\r\n<String>\r\n<Name> </Name>\r\n<Val></Val>\r\n</String>\r\n<String>\r\n<Name> </Name>\r\n<Val></Val>\r\n</String>\r\n<String>\r\n<Name> </Name>\r\n<Val></Val>\r\n</String>\r\n<String>\r\n<Name> </Name>\r\n<Val></Val>\r\n</String>\r\n<String>\r\n<Name> </Name>\r\n<Val></Val>\r\n</String>\r\n<String>\r\n<Name> </Name>\r\n<Val></Val>\r\n</String>\r\n<String>\r\n<Name> </Name>\r\n<Val>-20</Val>\r\n</String>\r\n<String>\r\n<Name> </Name>\r\n<Val></Val>\r\n</String>\r\n<String>\r\n<Name> </Name>\r\n<Val></Val>\r\n</String>\r\n<String>\r\n<Name> </Name>\r\n<Val></Val>\r\n</String>\r\n<String>\r\n<Name> </Name>\r\n<Val></Val>\r\n</String>\r\n<String>\r\n<Name> </Name>\r\n<Val></Val>\r\n</String>\r\n<String>\r\n<Name> </Name>\r\n<Val></Val>\r\n</String>\r\n<String>\r\n<Name> </Name>\r\n<Val></Val>\r\n</String>\r\n<String>\r\n<Name> </Name>\r\n<Val></Val>\r\n</String>\r\n<String>\r\n<Name> </Name>\r\n<Val></Val>\r\n</String>\r\n<String>\r\n<Name> </Name>\r\n<Val></Val>\r\n</String>\r\n<String>\r\n<Name> </Name>\r\n<Val></Val>\r\n</String>\r\n<String>\r\n<Name> </Name>\r\n<Val>-20</Val>\r\n</String>\r\n<String>\r\n<Name> </Name>\r\n<Val></Val>\r\n</String>\r\n<String>\r\n<Name> </Name>\r\n<Val></Val>\r\n</String>\r\n<String>\r\n<Name> </Name>\r\n<Val></Val>\r\n</String>\r\n<String>\r\n<Name> </Name>\r\n<Val></Val>\r\n</String>\r\n<String>\r\n<Name> </Name>\r\n<Val></Val>\r\n</String>\r\n<String>\r\n<Name> </Name>\r\n<Val></Val>\r\n</String>\r\n<String>\r\n<Name> </Name>\r\n<Val></Val>\r\n</String>\r\n<String>\r\n<Name> </Name>\r\n<Val></Val>\r\n</String>\r\n<String>\r\n<Name> </Name>\r\n<Val></Val>\r\n</String>\r\n<String>\r\n<Name> </Name>\r\n<Val></Val>\r\n</String>\r\n<String>\r\n<Name> </Name>\r\n<Val></Val>\r\n</String>\r\n<String>\r\n<Name> </Name>\r\n<Val>-20</Val>\r\n</String>\r\n<String>\r\n<Name> </Name>\r\n<Val></Val>\r\n</String>\r\n<String>\r\n<Name> </Name>\r\n<Val></Val>\r\n</String>\r\n<String>\r\n<Name> </Name>\r\n<Val></Val>\r\n</String>\r\n<String>\r\n<Name> </Name>\r\n<Val></Val>\r\n</String>\r\n<String>\r\n<Name> </Name>\r\n<Val></Val>\r\n</String>\r\n<String>\r\n<Name> </Name>\r\n<Val></Val>\r\n</String>\r\n<String>\r\n<Name> </Name>\r\n<Val></Val>\r\n</String>\r\n<String>\r\n<Name> </Name>\r\n<Val></Val>\r\n</String>\r\n<String>\r\n<Name> </Name>\r\n<Val></Val>\r\n</String>\r\n<String>\r\n<Name> </Name>\r\n<Val></Val>\r\n</String>\r\n<String>\r\n<Name> </Name>\r\n<Val></Val>\r\n</String>\r\n<String>\r\n<Name> </Name>\r\n<Val></Val>\r\n</String>\r\n<String>\r\n<Name> </Name>\r\n<Val></Val>\r\n</String>\r\n<String>\r\n<Name> </Name>\r\n<Val>-20</Val>\r\n</String>\r\n<String>\r\n<Name> </Name>\r\n<Val></Val>\r\n</String>\r\n<String>\r\n<Name> </Name>\r\n<Val></Val>\r\n</String>\r\n<String>\r\n<Name> </Name>\r\n<Val></Val>\r\n</String>\r\n<String>\r\n<Name> </Name>\r\n<Val></Val>\r\n</String>\r\n<String>\r\n<Name> </Name>\r\n<Val></Val>\r\n</String>\r\n<String>\r\n<Name> </Name>\r\n<Val></Val>\r\n</String>\r\n<String>\r\n<Name> </Name>\r\n<Val></Val>\r\n</String>\r\n<String>\r\n<Name> </Name>\r\n<Val></Val>\r\n</String>\r\n<String>\r\n<Name> </Name>\r\n<Val></Val>\r\n</String>\r\n<String>\r\n<Name> </Name>\r\n<Val></Val>\r\n</String>\r\n<String>\r\n<Name> </Name>\r\n<Val></Val>\r\n</String>\r\n<String>\r\n<Name> </Name>\r\n<Val>-20</Val>\r\n</String>\r\n<String>\r\n<Name> </Name>\r\n<Val></Val>\r\n</String>\r\n<String>\r\n<Name> </Name>\r\n<Val></Val>\r\n</String>\r\n<String>\r\n<Name> </Name>\r\n<Val></Val>\r\n</String>\r\n<String>\r\n<Name> </Name>\r\n<Val></Val>\r\n</String>\r\n<String>\r\n<Name> </Name>\r\n<Val></Val>\r\n</String>\r\n<String>\r\n<Name> </Name>\r\n<Val></Val>\r\n</String>\r\n<String>\r\n<Name> </Name>\r\n<Val></Val>\r\n</String>\r\n<String>\r\n<Name> </Name>\r\n<Val></Val>\r\n</String>\r\n<String>\r\n<Name> </Name>\r\n<Val></Val>\r\n</String>\r\n<String>\r\n<Name> </Name>\r\n<Val></Val>\r\n</String>\r\n<String>\r\n<Name> </Name>\r\n<Val></Val>\r\n</String>\r\n<String>\r\n<Name> </Name>\r\n<Val>-20</Val>\r\n</String>\r\n<String>\r\n<Name> </Name>\r\n<Val></Val>\r\n</String>\r\n<String>\r\n<Name> </Name>\r\n<Val></Val>\r\n</String>\r\n<String>\r\n<Name> </Name>\r\n<Val></Val>\r\n</String>\r\n<String>\r\n<Name> </Name>\r\n<Val></Val>\r\n</String>\r\n<String>\r\n<Name> </Name>\r\n<Val></Val>\r\n</String>\r\n<String>\r\n<Name> </Name>\r\n<Val></Val>\r\n</String>\r\n<String>\r\n<Name> </Name>\r\n<Val></Val>\r\n</String>\r\n<String>\r\n<Name> </Name>\r\n<Val></Val>\r\n</String>\r\n<String>\r\n<Name> </Name>\r\n<Val></Val>\r\n</String>\r\n<String>\r\n<Name> </Name>\r\n<Val></Val>\r\n</String>\r\n<String>\r\n<Name> </Name>\r\n<Val></Val>\r\n</String>\r\n<String>\r\n<Name> </Name>\r\n<Val>-20</Val>\r\n</String>\r\n<String>\r\n<Name> </Name>\r\n<Val></Val>\r\n</String>\r\n<String>\r\n<Name> </Name>\r\n<Val></Val>\r\n</String>\r\n<String>\r\n<Name> </Name>\r\n<Val></Val>\r\n</String>\r\n<String>\r\n<Name> </Name>\r\n<Val></Val>\r\n</String>\r\n<String>\r\n<Name> </Name>\r\n<Val></Val>\r\n</String>\r\n<String>\r\n<Name> </Name>\r\n<Val></Val>\r\n</String>\r\n<String>\r\n<Name> </Name>\r\n<Val></Val>\r\n</String>\r\n<String>\r\n<Name> </Name>\r\n<Val></Val>\r\n</String>\r\n<String>\r\n<Name> </Name>\r\n<Val></Val>\r\n</String>\r\n<String>\r\n<Name> </Name>\r\n<Val></Val>\r\n</String>\r\n<String>\r\n<Name> </Name>\r\n<Val></Val>\r\n</String>\r\n<String>\r\n<Name> </Name>\r\n<Val></Val>\r\n</String>\r\n<String>\r\n<Name> </Name>\r\n<Val></Val>\r\n</String>\r\n<String>\r\n<Name> </Name>\r\n<Val>-20</Val>\r\n</String>\r\n<String>\r\n<Name> </Name>\r\n<Val></Val>\r\n</String>\r\n<String>\r\n<Name> </Name>\r\n<Val></Val>\r\n</String>\r\n<String>\r\n<Name> </Name>\r\n<Val></Val>\r\n</String>\r\n<String>\r\n<Name> </Name>\r\n<Val></Val>\r\n</String>\r\n<String>\r\n<Name> </Name>\r\n<Val></Val>\r\n</String>\r\n<String>\r\n<Name> </Name>\r\n<Val></Val>\r\n</String>\r\n<String>\r\n<Name> </Name>\r\n<Val></Val>\r\n</String>\r\n<String>\r\n<Name> </Name>\r\n<Val></Val>\r\n</String>\r\n<String>\r\n<Name> </Name>\r\n<Val></Val>\r\n</String>\r\n<String>\r\n<Name> </Name>\r\n<Val></Val>\r\n</String>\r\n<String>\r\n<Name> </Name>\r\n<Val></Val>\r\n</String>\r\n<String>\r\n<Name> </Name>\r\n<Val>-20</Val>\r\n</String>\r\n<String>\r\n<Name> </Name>\r\n<Val></Val>\r\n</String>\r\n<String>\r\n<Name> </Name>\r\n<Val></Val>\r\n</String>\r\n<String>\r\n<Name> </Name>\r\n<Val></Val>\r\n</String>\r\n<String>\r\n<Name> </Name>\r\n<Val></Val>\r\n</String>\r\n<String>\r\n<Name> </Name>\r\n<Val></Val>\r\n</String>\r\n<String>\r\n<Name> </Name>\r\n<Val></Val>\r\n</String>\r\n<String>\r\n<Name> </Name>\r\n<Val></Val>\r\n</String>\r\n<String>\r\n<Name> </Name>\r\n<Val></Val>\r\n</String>\r\n<String>\r\n<Name> </Name>\r\n<Val></Val>\r\n</String>\r\n<String>\r\n<Name> </Name>\r\n<Val></Val>\r\n</String>\r\n<String>\r\n<Name> </Name>\r\n<Val></Val>\r\n</String>\r\n<String>\r\n<Name> </Name>\r\n<Val>-20</Val>\r\n</String>\r\n<String>\r\n<Name> </Name>\r\n<Val></Val>\r\n</String>\r\n<String>\r\n<Name> </Name>\r\n<Val></Val>\r\n</String>\r\n<String>\r\n<Name> </Name>\r\n<Val></Val>\r\n</String>\r\n<String>\r\n<Name> </Name>\r\n<Val></Val>\r\n</String>\r\n<String>\r\n<Name> </Name>\r\n<Val></Val>\r\n</String>\r\n<String>\r\n<Name> </Name>\r\n<Val></Val>\r\n</String>\r\n<String>\r\n<Name> </Name>\r\n<Val></Val>\r\n</String>\r\n<String>\r\n<Name> </Name>\r\n<Val></Val>\r\n</String>\r\n<String>\r\n<Name> </Name>\r\n<Val></Val>\r\n</String>\r\n<String>\r\n<Name> </Name>\r\n<Val></Val>\r\n</String>\r\n<String>\r\n<Name> </Name>\r\n<Val></Val>\r\n</String>\r\n<String>\r\n<Name> </Name>\r\n<Val>-20</Val>\r\n</String>\r\n<String>\r\n<Name> </Name>\r\n<Val></Val>\r\n</String>\r\n<String>\r\n<Name> </Name>\r\n<Val></Val>\r\n</String>\r\n<String>\r\n<Name> </Name>\r\n<Val></Val>\r\n</String>\r\n<String>\r\n<Name> </Name>\r\n<Val></Val>\r\n</String>\r\n<String>\r\n<Name> </Name>\r\n<Val></Val>\r\n</String>\r\n<String>\r\n<Name> </Name>\r\n<Val></Val>\r\n</String>\r\n<String>\r\n<Name> </Name>\r\n<Val></Val>\r\n</String>\r\n<String>\r\n<Name> </Name>\r\n<Val></Val>\r\n</String>\r\n<String>\r\n<Name> </Name>\r\n<Val></Val>\r\n</String>\r\n<String>\r\n<Name> </Name>\r\n<Val></Val>\r\n</String>\r\n<String>\r\n<Name> </Name>\r\n<Val></Val>\r\n</String>\r\n<String>\r\n<Name> </Name>\r\n<Val></Val>\r\n</String>\r\n<String>\r\n<Name> </Name>\r\n<Val></Val>\r\n</String>\r\n<String>\r\n<Name> </Name>\r\n<Val></Val>\r\n</String>\r\n<String>\r\n<Name> </Name>\r\n<Val></Val>\r\n</String>\r\n<String>\r\n<Name> </Name>\r\n<Val></Val>\r\n</String>\r\n<String>\r\n<Name> </Name>\r\n<Val></Val>\r\n</String>\r\n<String>\r\n<Name> </Name>\r\n<Val></Val>\r\n</String>\r\n<String>\r\n<Name> </Name>\r\n<Val></Val>\r\n</String>\r\n<String>\r\n<Name> </Name>\r\n<Val></Val>\r\n</String>\r\n<String>\r\n<Name> </Name>\r\n<Val></Val>\r\n</String>\r\n<String>\r\n<Name> </Name>\r\n<Val></Val>\r\n</String>\r\n<String>\r\n<Name> </Name>\r\n<Val></Val>\r\n</String>\r\n<String>\r\n<Name> </Name>\r\n<Val></Val>\r\n</String>\r\n<String>\r\n<Name> </Name>\r\n<Val></Val>\r\n</String>\r\n<String>\r\n<Name> </Name>\r\n<Val></Val>\r\n</String>\r\n<String>\r\n<Name> </Name>\r\n<Val></Val>\r\n</String>\r\n<String>\r\n<Name> </Name>\r\n<Val></Val>\r\n</String>\r\n<String>\r\n<Name> </Name>\r\n<Val></Val>\r\n</String>\r\n<String>\r\n<Name> </Name>\r\n<Val></Val>\r\n</String>\r\n<String>\r\n<Name> </Name>\r\n<Val></Val>\r\n</String>\r\n<String>\r\n<Name> </Name>\r\n<Val></Val>\r\n</String>\r\n<String>\r\n<Name> </Name>\r\n<Val></Val>\r\n</String>\r\n<String>\r\n<Name> </Name>\r\n<Val></Val>\r\n</String>\r\n<String>\r\n<Name> </Name>\r\n<Val></Val>\r\n</String>\r\n<String>\r\n<Name> </Name>\r\n<Val></Val>\r\n</String>\r\n<String>\r\n<Name> </Name>\r\n<Val></Val>\r\n</String>\r\n<String>\r\n<Name> </Name>\r\n<Val></Val>\r\n</String>\r\n<String>\r\n<Name> </Name>\r\n<Val></Val>\r\n</String>\r\n<String>\r\n<Name> </Name>\r\n<Val></Val>\r\n</String>\r\n<String>\r\n<Name> </Name>\r\n<Val></Val>\r\n</String>\r\n<String>\r\n<Name> </Name>\r\n<Val></Val>\r\n</String>\r\n<String>\r\n<Name> </Name>\r\n<Val></Val>\r\n</String>\r\n<String>\r\n<Name> </Name>\r\n<Val></Val>\r\n</String>\r\n<String>\r\n<Name> </Name>\r\n<Val></Val>\r\n</String>\r\n<String>\r\n<Name> </Name>\r\n<Val></Val>\r\n</String>\r\n<String>\r\n<Name> </Name>\r\n<Val></Val>\r\n</String>\r\n<String>\r\n<Name> </Name>\r\n<Val></Val>\r\n</String>\r\n<String>\r\n<Name> </Name>\r\n<Val></Val>\r\n</String>\r\n<String>\r\n<Name> </Name>\r\n<Val></Val>\r\n</String>\r\n<String>\r\n<Name> </Name>\r\n<Val></Val>\r\n</String>\r\n<String>\r\n<Name> </Name>\r\n<Val></Val>\r\n</String>\r\n<String>\r\n<Name> </Name>\r\n<Val></Val>\r\n</String>\r\n<String>\r\n<Name> </Name>\r\n<Val></Val>\r\n</String>\r\n<String>\r\n<Name> </Name>\r\n<Val></Val>\r\n</String>\r\n<String>\r\n<Name> </Name>\r\n<Val></Val>\r\n</String>\r\n<String>\r\n<Name> </Name>\r\n<Val></Val>\r\n</String>\r\n<String>\r\n<Name> </Name>\r\n<Val></Val>\r\n</String>\r\n<String>\r\n<Name> </Name>\r\n<Val></Val>\r\n</String>\r\n<String>\r\n<Name> </Name>\r\n<Val></Val>\r\n</String>\r\n<String>\r\n<Name> </Name>\r\n<Val></Val>\r\n</String>\r\n<String>\r\n<Name> </Name>\r\n<Val></Val>\r\n</String>\r\n<String>\r\n<Name> </Name>\r\n<Val></Val>\r\n</String>\r\n<String>\r\n<Name> </Name>\r\n<Val></Val>\r\n</String>\r\n<String>\r\n<Name> </Name>\r\n<Val></Val>\r\n</String>\r\n<String>\r\n<Name> </Name>\r\n<Val></Val>\r\n</String>\r\n<String>\r\n<Name> </Name>\r\n<Val></Val>\r\n</String>\r\n<String>\r\n<Name> </Name>\r\n<Val></Val>\r\n</String>\r\n<String>\r\n<Name> </Name>\r\n<Val></Val>\r\n</String>\r\n<String>\r\n<Name> </Name>\r\n<Val></Val>\r\n</String>\r\n<String>\r\n<Name> </Name>\r\n<Val></Val>\r\n</String>\r\n<String>\r\n<Name> </Name>\r\n<Val></Val>\r\n</String>\r\n<String>\r\n<Name> </Name>\r\n<Val></Val>\r\n</String>\r\n<String>\r\n<Name> </Name>\r\n<Val></Val>\r\n</String>\r\n<String>\r\n<Name> </Name>\r\n<Val></Val>\r\n</String>\r\n<String>\r\n<Name> </Name>\r\n<Val></Val>\r\n</String>\r\n<String>\r\n<Name> </Name>\r\n<Val></Val>\r\n</String>\r\n<String>\r\n<Name> </Name>\r\n<Val></Val>\r\n</String>\r\n<String>\r\n<Name> </Name>\r\n<Val></Val>\r\n</String>\r\n<String>\r\n<Name> </Name>\r\n<Val></Val>\r\n</String>\r\n<String>\r\n<Name> </Name>\r\n<Val></Val>\r\n</String>\r\n<String>\r\n<Name> </Name>\r\n<Val></Val>\r\n</String>\r\n<String>\r\n<Name> </Name>\r\n<Val></Val>\r\n</String>\r\n<String>\r\n<Name> </Name>\r\n<Val></Val>\r\n</String>\r\n<String>\r\n<Name> </Name>\r\n<Val></Val>\r\n</String>\r\n<String>\r\n<Name> </Name>\r\n<Val></Val>\r\n</String>\r\n<String>\r\n<Name> </Name>\r\n<Val></Val>\r\n</String>\r\n<String>\r\n<Name> </Name>\r\n<Val></Val>\r\n</String>\r\n<String>\r\n<Name> </Name>\r\n<Val></Val>\r\n</String>\r\n<String>\r\n<Name> </Name>\r\n<Val></Val>\r\n</String>\r\n<String>\r\n<Name> </Name>\r\n<Val></Val>\r\n</String>\r\n<String>\r\n<Name> </Name>\r\n<Val></Val>\r\n</String>\r\n<String>\r\n<Name> </Name>\r\n<Val></Val>\r\n</String>\r\n<String>\r\n<Name> </Name>\r\n<Val></Val>\r\n</String>\r\n<String>\r\n<Name> </Name>\r\n<Val></Val>\r\n</String>\r\n<String>\r\n<Name> </Name>\r\n<Val></Val>\r\n</String>\r\n<String>\r\n<Name> </Name>\r\n<Val></Val>\r\n</String>\r\n<String>\r\n<Name> </Name>\r\n<Val></Val>\r\n</String>\r\n<String>\r\n<Name> </Name>\r\n<Val></Val>\r\n</String>\r\n<String>\r\n<Name> </Name>\r\n<Val></Val>\r\n</String>\r\n<String>\r\n<Name> </Name>\r\n<Val></Val>\r\n</String>\r\n<String>\r\n<Name> </Name>\r\n<Val></Val>\r\n</String>\r\n<String>\r\n<Name> </Name>\r\n<Val></Val>\r\n</String>\r\n<String>\r\n<Name> </Name>\r\n<Val></Val>\r\n</String>\r\n<String>\r\n<Name> </Name>\r\n<Val></Val>\r\n</String>\r\n<String>\r\n<Name> </Name>\r\n<Val></Val>\r\n</String>\r\n<String>\r\n<Name> </Name>\r\n<Val></Val>\r\n</String>\r\n<String>\r\n<Name> </Name>\r\n<Val></Val>\r\n</String>\r\n<String>\r\n<Name> </Name>\r\n<Val></Val>\r\n</String>\r\n<String>\r\n<Name> </Name>\r\n<Val></Val>\r\n</String>\r\n<String>\r\n<Name> </Name>\r\n<Val></Val>\r\n</String>\r\n<String>\r\n<Name> </Name>\r\n<Val></Val>\r\n</String>\r\n<String>\r\n<Name> </Name>\r\n<Val></Val>\r\n</String>\r\n<String>\r\n<Name> </Name>\r\n<Val></Val>\r\n</String>\r\n<String>\r\n<Name> </Name>\r\n<Val></Val>\r\n</String>\r\n<String>\r\n<Name> </Name>\r\n<Val></Val>\r\n</String>\r\n<String>\r\n<Name> </Name>\r\n<Val></Val>\r\n</String>\r\n<String>\r\n<Name> </Name>\r\n<Val></Val>\r\n</String>\r\n<String>\r\n<Name> </Name>\r\n<Val></Val>\r\n</String>\r\n<String>\r\n<Name> </Name>\r\n<Val></Val>\r\n</String>\r\n<String>\r\n<Name> </Name>\r\n<Val></Val>\r\n</String>\r\n<String>\r\n<Name> </Name>\r\n<Val></Val>\r\n</String>\r\n<String>\r\n<Name> </Name>\r\n<Val></Val>\r\n</String>\r\n<String>\r\n<Name> </Name>\r\n<Val></Val>\r\n</String>\r\n<String>\r\n<Name> </Name>\r\n<Val></Val>\r\n</String>\r\n<String>\r\n<Name> </Name>\r\n<Val></Val>\r\n</String>\r\n<String>\r\n<Name> </Name>\r\n<Val></Val>\r\n</String>\r\n<String>\r\n<Name> </Name>\r\n<Val></Val>\r\n</String>\r\n<String>\r\n<Name> </Name>\r\n<Val></Val>\r\n</String>\r\n<String>\r\n<Name> </Name>\r\n<Val></Val>\r\n</String>\r\n<String>\r\n<Name> </Name>\r\n<Val></Val>\r\n</String>\r\n<String>\r\n<Name> </Name>\r\n<Val></Val>\r\n</String>\r\n<String>\r\n<Name> </Name>\r\n<Val></Val>\r\n</String>\r\n<String>\r\n<Name> </Name>\r\n<Val></Val>\r\n</String>\r\n<String>\r\n<Name> </Name>\r\n<Val></Val>\r\n</String>\r\n<String>\r\n<Name> </Name>\r\n<Val></Val>\r\n</String>\r\n<String>\r\n<Name> </Name>\r\n<Val></Val>\r\n</String>\r\n<String>\r\n<Name> </Name>\r\n<Val></Val>\r\n</String>\r\n<String>\r\n<Name> </Name>\r\n<Val></Val>\r\n</String>\r\n<String>\r\n<Name> </Name>\r\n<Val></Val>\r\n</String>\r\n<String>\r\n<Name> </Name>\r\n<Val></Val>\r\n</String>\r\n<String>\r\n<Name> </Name>\r\n<Val></Val>\r\n</String>\r\n<String>\r\n<Name> </Name>\r\n<Val></Val>\r\n</String>\r\n<String>\r\n<Name> </Name>\r\n<Val></Val>\r\n</String>\r\n<String>\r\n<Name> </Name>\r\n<Val></Val>\r\n</String>\r\n<String>\r\n<Name> </Name>\r\n<Val></Val>\r\n</String>\r\n<String>\r\n<Name> </Name>\r\n<Val></Val>\r\n</String>\r\n<String>\r\n<Name> </Name>\r\n<Val></Val>\r\n</String>\r\n<String>\r\n<Name> </Name>\r\n<Val></Val>\r\n</String>\r\n<String>\r\n<Name> </Name>\r\n<Val></Val>\r\n</String>\r\n<String>\r\n<Name> </Name>\r\n<Val></Val>\r\n</String>\r\n<String>\r\n<Name> </Name>\r\n<Val></Val>\r\n</String>\r\n<String>\r\n<Name> </Name>\r\n<Val></Val>\r\n</String>\r\n<String>\r\n<Name> </Name>\r\n<Val></Val>\r\n</String>\r\n<String>\r\n<Name> </Name>\r\n<Val></Val>\r\n</String>\r\n<String>\r\n<Name> </Name>\r\n<Val></Val>\r\n</String>\r\n<String>\r\n<Name> </Name>\r\n<Val></Val>\r\n</String>\r\n<String>\r\n<Name> </Name>\r\n<Val></Val>\r\n</String>\r\n<String>\r\n<Name> </Name>\r\n<Val></Val>\r\n</String>\r\n<String>\r\n<Name> </Name>\r\n<Val></Val>\r\n</String>\r\n<String>\r\n<Name> </Name>\r\n<Val></Val>\r\n</String>\r\n<String>\r\n<Name> </Name>\r\n<Val></Val>\r\n</String>\r\n<String>\r\n<Name> </Name>\r\n<Val></Val>\r\n</String>\r\n<String>\r\n<Name> </Name>\r\n<Val></Val>\r\n</String>\r\n<String>\r\n<Name> </Name>\r\n<Val></Val>\r\n</String>\r\n<String>\r\n<Name> </Name>\r\n<Val></Val>\r\n</String>\r\n<String>\r\n<Name> </Name>\r\n<Val></Val>\r\n</String>\r\n<String>\r\n<Name> </Name>\r\n<Val></Val>\r\n</String>\r\n<String>\r\n<Name> </Name>\r\n<Val></Val>\r\n</String>\r\n<String>\r\n<Name> </Name>\r\n<Val></Val>\r\n</String>\r\n<String>\r\n<Name> </Name>\r\n<Val></Val>\r\n</String>\r\n<String>\r\n<Name> </Name>\r\n<Val></Val>\r\n</String>\r\n<String>\r\n<Name> </Name>\r\n<Val></Val>\r\n</String>\r\n<String>\r\n<Name> </Name>\r\n<Val></Val>\r\n</String>\r\n<String>\r\n<Name> </Name>\r\n<Val></Val>\r\n</String>\r\n<String>\r\n<Name> </Name>\r\n<Val></Val>\r\n</String>\r\n<String>\r\n<Name> </Name>\r\n<Val></Val>\r\n</String>\r\n<String>\r\n<Name> </Name>\r\n<Val></Val>\r\n</String>\r\n<String>\r\n<Name> </Name>\r\n<Val></Val>\r\n</String>\r\n<String>\r\n<Name> </Name>\r\n<Val></Val>\r\n</String>\r\n<String>\r\n<Name> </Name>\r\n<Val></Val>\r\n</String>\r\n<String>\r\n<Name> </Name>\r\n<Val></Val>\r\n</String>\r\n<String>\r\n<Name> </Name>\r\n<Val></Val>\r\n</String>\r\n<String>\r\n<Name> </Name>\r\n<Val></Val>\r\n</String>\r\n<String>\r\n<Name> </Name>\r\n<Val></Val>\r\n</String>\r\n<String>\r\n<Name> </Name>\r\n<Val></Val>\r\n</String>\r\n<String>\r\n<Name> </Name>\r\n<Val></Val>\r\n</String>\r\n<String>\r\n<Name> </Name>\r\n<Val></Val>\r\n</String>\r\n<String>\r\n<Name> </Name>\r\n<Val></Val>\r\n</String>\r\n<String>\r\n<Name> </Name>\r\n<Val></Val>\r\n</String>\r\n<String>\r\n<Name> </Name>\r\n<Val></Val>\r\n</String>\r\n<String>\r\n<Name> </Name>\r\n<Val></Val>\r\n</String>\r\n<String>\r\n<Name> </Name>\r\n<Val></Val>\r\n</String>\r\n<String>\r\n<Name> </Name>\r\n<Val></Val>\r\n</String>\r\n<String>\r\n<Name> </Name>\r\n<Val></Val>\r\n</String>\r\n<String>\r\n<Name> </Name>\r\n<Val></Val>\r\n</String>\r\n<String>\r\n<Name> </Name>\r\n<Val></Val>\r\n</String>\r\n<String>\r\n<Name> </Name>\r\n<Val></Val>\r\n</String>\r\n<String>\r\n<Name> </Name>\r\n<Val></Val>\r\n</String>\r\n<String>\r\n<Name> </Name>\r\n<Val></Val>\r\n</String>\r\n<String>\r\n<Name> </Name>\r\n<Val></Val>\r\n</String>\r\n<String>\r\n<Name> </Name>\r\n<Val></Val>\r\n</String>\r\n<String>\r\n<Name> </Name>\r\n<Val></Val>\r\n</String>\r\n<String>\r\n<Name> </Name>\r\n<Val></Val>\r\n</String>\r\n<String>\r\n<Name> </Name>\r\n<Val></Val>\r\n</String>\r\n<String>\r\n<Name> </Name>\r\n<Val></Val>\r\n</String>\r\n<String>\r\n<Name> </Name>\r\n<Val></Val>\r\n</String>\r\n<String>\r\n<Name> </Name>\r\n<Val></Val>\r\n</String>\r\n<String>\r\n<Name> </Name>\r\n<Val></Val>\r\n</String>\r\n<String>\r\n<Name> </Name>\r\n<Val></Val>\r\n</String>\r\n<String>\r\n<Name> </Name>\r\n<Val></Val>\r\n</String>\r\n<String>\r\n<Name> </Name>\r\n<Val></Val>\r\n</String>\r\n<String>\r\n<Name> </Name>\r\n<Val></Val>\r\n</String>\r\n<String>\r\n<Name> </Name>\r\n<Val></Val>\r\n</String>\r\n<String>\r\n<Name> </Name>\r\n<Val></Val>\r\n</String>\r\n<String>\r\n<Name> </Name>\r\n<Val></Val>\r\n</String>\r\n<String>\r\n<Name> </Name>\r\n<Val></Val>\r\n</String>\r\n<String>\r\n<Name> </Name>\r\n<Val></Val>\r\n</String>\r\n<String>\r\n<Name> </Name>\r\n<Val></Val>\r\n</String>\r\n<String>\r\n<Name> </Name>\r\n<Val></Val>\r\n</String>\r\n<String>\r\n<Name> </Name>\r\n<Val></Val>\r\n</String>\r\n<String>\r\n<Name> </Name>\r\n<Val></Val>\r\n</String>\r\n<String>\r\n<Name> </Name>\r\n<Val></Val>\r\n</String>\r\n<String>\r\n<Name> </Name>\r\n<Val></Val>\r\n</String>\r\n<String>\r\n<Name> </Name>\r\n<Val></Val>\r\n</String>\r\n<String>\r\n<Name> </Name>\r\n<Val></Val>\r\n</String>\r\n<String>\r\n<Name> </Name>\r\n<Val></Val>\r\n</String>\r\n<String>\r\n<Name> </Name>\r\n<Val></Val>\r\n</String>\r\n<String>\r\n<Name> </Name>\r\n<Val></Val>\r\n</String>\r\n<String>\r\n<Name> </Name>\r\n<Val></Val>\r\n</String>\r\n<String>\r\n<Name> </Name>\r\n<Val></Val>\r\n</String>\r\n<String>\r\n<Name> </Name>\r\n<Val></Val>\r\n</String>\r\n<String>\r\n<Name> </Name>\r\n<Val></Val>\r\n</String>\r\n<String>\r\n<Name> </Name>\r\n<Val></Val>\r\n</String>\r\n<String>\r\n<Name> </Name>\r\n<Val></Val>\r\n</String>\r\n<String>\r\n<Name> </Name>\r\n<Val></Val>\r\n</String>\r\n<String>\r\n<Name> </Name>\r\n<Val></Val>\r\n</String>\r\n<String>\r\n<Name> </Name>\r\n<Val></Val>\r\n</String>\r\n<String>\r\n<Name> </Name>\r\n<Val></Val>\r\n</String>\r\n<String>\r\n<Name> </Name>\r\n<Val></Val>\r\n</String>\r\n<String>\r\n<Name> </Name>\r\n<Val></Val>\r\n</String>\r\n<String>\r\n<Name> </Name>\r\n<Val></Val>\r\n</String>\r\n<String>\r\n<Name> </Name>\r\n<Val></Val>\r\n</String>\r\n<String>\r\n<Name> </Name>\r\n<Val></Val>\r\n</String>\r\n<String>\r\n<Name> </Name>\r\n<Val></Val>\r\n</String>\r\n<String>\r\n<Name> </Name>\r\n<Val></Val>\r\n</String>\r\n<String>\r\n<Name> </Name>\r\n<Val></Val>\r\n</String>\r\n<String>\r\n<Name> </Name>\r\n<Val></Val>\r\n</String>\r\n<String>\r\n<Name> </Name>\r\n<Val></Val>\r\n</String>\r\n<String>\r\n<Name> </Name>\r\n<Val></Val>\r\n</String>\r\n<String>\r\n<Name> </Name>\r\n<Val></Val>\r\n</String>\r\n<String>\r\n<Name> </Name>\r\n<Val></Val>\r\n</String>\r\n<String>\r\n<Name> </Name>\r\n<Val></Val>\r\n</String>\r\n<String>\r\n<Name> </Name>\r\n<Val></Val>\r\n</String>\r\n<String>\r\n<Name> </Name>\r\n<Val></Val>\r\n</String>\r\n<String>\r\n<Name> </Name>\r\n<Val></Val>\r\n</String>\r\n<String>\r\n<Name> </Name>\r\n<Val></Val>\r\n</String>\r\n<String>\r\n<Name> </Name>\r\n<Val></Val>\r\n</String>\r\n<String>\r\n<Name> </Name>\r\n<Val></Val>\r\n</String>\r\n<String>\r\n<Name> </Name>\r\n<Val></Val>\r\n</String>\r\n<String>\r\n<Name> </Name>\r\n<Val></Val>\r\n</String>\r\n<String>\r\n<Name> </Name>\r\n<Val></Val>\r\n</String>\r\n<String>\r\n<Name> </Name>\r\n<Val></Val>\r\n</String>\r\n<String>\r\n<Name> </Name>\r\n<Val></Val>\r\n</String>\r\n<String>\r\n<Name> </Name>\r\n<Val></Val>\r\n</String>\r\n<String>\r\n<Name> </Name>\r\n<Val></Val>\r\n</String>\r\n<String>\r\n<Name> </Name>\r\n<Val></Val>\r\n</String>\r\n<String>\r\n<Name> </Name>\r\n<Val></Val>\r\n</String>\r\n<String>\r\n<Name> </Name>\r\n<Val></Val>\r\n</String>\r\n<String>\r\n<Name> </Name>\r\n<Val></Val>\r\n</String>\r\n<String>\r\n<Name> </Name>\r\n<Val></Val>\r\n</String>\r\n<String>\r\n<Name> </Name>\r\n<Val></Val>\r\n</String>\r\n<String>\r\n<Name> </Name>\r\n<Val></Val>\r\n</String>\r\n<String>\r\n<Name> </Name>\r\n<Val></Val>\r\n</String>\r\n<String>\r\n<Name> </Name>\r\n<Val></Val>\r\n</String>\r\n<String>\r\n<Name> </Name>\r\n<Val></Val>\r\n</String>\r\n<String>\r\n<Name> </Name>\r\n<Val></Val>\r\n</String>\r\n<String>\r\n<Name> </Name>\r\n<Val></Val>\r\n</String>\r\n<String>\r\n<Name> </Name>\r\n<Val></Val>\r\n</String>\r\n<String>\r\n<Name> </Name>\r\n<Val></Val>\r\n</String>\r\n<String>\r\n<Name> </Name>\r\n<Val></Val>\r\n</String>\r\n<String>\r\n<Name> </Name>\r\n<Val></Val>\r\n</String>\r\n<String>\r\n<Name> </Name>\r\n<Val></Val>\r\n</String>\r\n<String>\r\n<Name> </Name>\r\n<Val></Val>\r\n</String>\r\n<String>\r\n<Name> </Name>\r\n<Val></Val>\r\n</String>\r\n<String>\r\n<Name> </Name>\r\n<Val></Val>\r\n</String>\r\n<String>\r\n<Name> </Name>\r\n<Val></Val>\r\n</String>\r\n<String>\r\n<Name> </Name>\r\n<Val></Val>\r\n</String>\r\n<String>\r\n<Name> </Name>\r\n<Val></Val>\r\n</String>\r\n<String>\r\n<Name> </Name>\r\n<Val></Val>\r\n</String>\r\n<String>\r\n<Name> </Name>\r\n<Val></Val>\r\n</String>\r\n<String>\r\n<Name> </Name>\r\n<Val></Val>\r\n</String>\r\n<String>\r\n<Name> </Name>\r\n<Val></Val>\r\n</String>\r\n<String>\r\n<Name> </Name>\r\n<Val></Val>\r\n</String>\r\n<String>\r\n<Name> </Name>\r\n<Val></Val>\r\n</String>\r\n<String>\r\n<Name> </Name>\r\n<Val></Val>\r\n</String>\r\n<String>\r\n<Name> </Name>\r\n<Val></Val>\r\n</String>\r\n<String>\r\n<Name> </Name>\r\n<Val></Val>\r\n</String>\r\n<String>\r\n<Name> </Name>\r\n<Val></Val>\r\n</String>\r\n<String>\r\n<Name> </Name>\r\n<Val></Val>\r\n</String>\r\n<String>\r\n<Name> </Name>\r\n<Val></Val>\r\n</String>\r\n<String>\r\n<Name> </Name>\r\n<Val></Val>\r\n</String>\r\n<String>\r\n<Name> </Name>\r\n<Val></Val>\r\n</String>\r\n<String>\r\n<Name> </Name>\r\n<Val></Val>\r\n</String>\r\n<String>\r\n<Name> </Name>\r\n<Val></Val>\r\n</String>\r\n<String>\r\n<Name> </Name>\r\n<Val></Val>\r\n</String>\r\n<String>\r\n<Name> </Name>\r\n<Val></Val>\r\n</String>\r\n<String>\r\n<Name> </Name>\r\n<Val></Val>\r\n</String>\r\n<String>\r\n<Name> </Name>\r\n<Val></Val>\r\n</String>\r\n<String>\r\n<Name> </Name>\r\n<Val></Val>\r\n</String>\r\n<String>\r\n<Name> </Name>\r\n<Val></Val>\r\n</String>\r\n<String>\r\n<Name> </Name>\r\n<Val></Val>\r\n</String>\r\n<String>\r\n<Name> </Name>\r\n<Val></Val>\r\n</String>\r\n<String>\r\n<Name> </Name>\r\n<Val></Val>\r\n</String>\r\n<String>\r\n<Name> </Name>\r\n<Val></Val>\r\n</String>\r\n<String>\r\n<Name> </Name>\r\n<Val></Val>\r\n</String>\r\n<String>\r\n<Name> </Name>\r\n<Val></Val>\r\n</String>\r\n<String>\r\n<Name> </Name>\r\n<Val></Val>\r\n</String>\r\n<String>\r\n<Name> </Name>\r\n<Val></Val>\r\n</String>\r\n<String>\r\n<Name> </Name>\r\n<Val></Val>\r\n</String>\r\n<String>\r\n<Name> </Name>\r\n<Val></Val>\r\n</String>\r\n<String>\r\n<Name> </Name>\r\n<Val></Val>\r\n</String>\r\n<String>\r\n<Name> </Name>\r\n<Val></Val>\r\n</String>\r\n<String>\r\n<Name> </Name>\r\n<Val></Val>\r\n</String>\r\n<String>\r\n<Name> </Name>\r\n<Val></Val>\r\n</String>\r\n<String>\r\n<Name> </Name>\r\n<Val></Val>\r\n</String>\r\n<String>\r\n<Name> </Name>\r\n<Val></Val>\r\n</String>\r\n<String>\r\n<Name> </Name>\r\n<Val></Val>\r\n</String>\r\n<String>\r\n<Name> </Name>\r\n<Val></Val>\r\n</String>\r\n<String>\r\n<Name> </Name>\r\n<Val></Val>\r\n</String>\r\n<String>\r\n<Name> </Name>\r\n<Val></Val>\r\n</String>\r\n<String>\r\n<Name> </Name>\r\n<Val></Val>\r\n</String>\r\n<String>\r\n<Name> </Name>\r\n<Val></Val>\r\n</String>\r\n<String>\r\n<Name> </Name>\r\n<Val></Val>\r\n</String>\r\n<String>\r\n<Name> </Name>\r\n<Val></Val>\r\n</String>\r\n<String>\r\n<Name> </Name>\r\n<Val></Val>\r\n</String>\r\n<String>\r\n<Name> </Name>\r\n<Val></Val>\r\n</String>\r\n<String>\r\n<Name> </Name>\r\n<Val></Val>\r\n</String>\r\n<String>\r\n<Name> </Name>\r\n<Val></Val>\r\n</String>\r\n<String>\r\n<Name> </Name>\r\n<Val></Val>\r\n</String>\r\n<String>\r\n<Name> </Name>\r\n<Val></Val>\r\n</String>\r\n<String>\r\n<Name> </Name>\r\n<Val></Val>\r\n</String>\r\n<String>\r\n<Name> </Name>\r\n<Val></Val>\r\n</String>\r\n<String>\r\n<Name> </Name>\r\n<Val></Val>\r\n</String>\r\n<String>\r\n<Name> </Name>\r\n<Val></Val>\r\n</String>\r\n<String>\r\n<Name> </Name>\r\n<Val></Val>\r\n</String>\r\n<String>\r\n<Name> </Name>\r\n<Val></Val>\r\n</String>\r\n<String>\r\n<Name> </Name>\r\n<Val></Val>\r\n</String>\r\n<String>\r\n<Name> </Name>\r\n<Val></Val>\r\n</String>\r\n<String>\r\n<Name> </Name>\r\n<Val></Val>\r\n</String>\r\n<String>\r\n<Name> </Name>\r\n<Val></Val>\r\n</String>\r\n<String>\r\n<Name> </Name>\r\n<Val></Val>\r\n</String>\r\n<String>\r\n<Name> </Name>\r\n<Val></Val>\r\n</String>\r\n<String>\r\n<Name> </Name>\r\n<Val></Val>\r\n</String>\r\n<String>\r\n<Name> </Name>\r\n<Val></Val>\r\n</String>\r\n<String>\r\n<Name> </Name>\r\n<Val></Val>\r\n</String>\r\n<String>\r\n<Name> </Name>\r\n<Val></Val>\r\n</String>\r\n<String>\r\n<Name> </Name>\r\n<Val></Val>\r\n</String>\r\n<String>\r\n<Name> </Name>\r\n<Val></Val>\r\n</String>\r\n<String>\r\n<Name> </Name>\r\n<Val></Val>\r\n</String>\r\n<String>\r\n<Name> </Name>\r\n<Val></Val>\r\n</String>\r\n<String>\r\n<Name> </Name>\r\n<Val></Val>\r\n</String>\r\n<String>\r\n<Name> </Name>\r\n<Val></Val>\r\n</String>\r\n<String>\r\n<Name> </Name>\r\n<Val></Val>\r\n</String>\r\n<String>\r\n<Name> </Name>\r\n<Val></Val>\r\n</String>\r\n<String>\r\n<Name> </Name>\r\n<Val></Val>\r\n</String>\r\n<String>\r\n<Name> </Name>\r\n<Val></Val>\r\n</String>\r\n<String>\r\n<Name> </Name>\r\n<Val></Val>\r\n</String>\r\n<String>\r\n<Name> </Name>\r\n<Val></Val>\r\n</String>\r\n<String>\r\n<Name> </Name>\r\n<Val></Val>\r\n</String>\r\n<String>\r\n<Name> </Name>\r\n<Val></Val>\r\n</String>\r\n<String>\r\n<Name> </Name>\r\n<Val></Val>\r\n</String>\r\n<String>\r\n<Name> </Name>\r\n<Val></Val>\r\n</String>\r\n<String>\r\n<Name> </Name>\r\n<Val></Val>\r\n</String>\r\n<String>\r\n<Name> </Name>\r\n<Val></Val>\r\n</String>\r\n<String>\r\n<Name> </Name>\r\n<Val></Val>\r\n</String>\r\n<String>\r\n<Name> </Name>\r\n<Val></Val>\r\n</String>\r\n<String>\r\n<Name> </Name>\r\n<Val></Val>\r\n</String>\r\n<String>\r\n<Name> </Name>\r\n<Val></Val>\r\n</String>\r\n<String>\r\n<Name> </Name>\r\n<Val></Val>\r\n</String>\r\n<String>\r\n<Name> </Name>\r\n<Val></Val>\r\n</String>\r\n<String>\r\n<Name> </Name>\r\n<Val></Val>\r\n</String>\r\n<String>\r\n<Name> </Name>\r\n<Val></Val>\r\n</String>\r\n<String>\r\n<Name> </Name>\r\n<Val></Val>\r\n</String>\r\n<String>\r\n<Name> </Name>\r\n<Val></Val>\r\n</String>\r\n<String>\r\n<Name> </Name>\r\n<Val></Val>\r\n</String>\r\n<String>\r\n<Name> </Name>\r\n<Val></Val>\r\n</String>\r\n<String>\r\n<Name> </Name>\r\n<Val></Val>\r\n</String>\r\n<String>\r\n<Name> </Name>\r\n<Val></Val>\r\n</String>\r\n<String>\r\n<Name> </Name>\r\n<Val></Val>\r\n</String>\r\n<String>\r\n<Name> </Name>\r\n<Val></Val>\r\n</String>\r\n<String>\r\n<Name> </Name>\r\n<Val></Val>\r\n</String>\r\n<String>\r\n<Name> </Name>\r\n<Val></Val>\r\n</String>\r\n<String>\r\n<Name> </Name>\r\n<Val></Val>\r\n</String>\r\n<String>\r\n<Name> </Name>\r\n<Val></Val>\r\n</String>\r\n<String>\r\n<Name> </Name>\r\n<Val></Val>\r\n</String>\r\n<String>\r\n<Name> </Name>\r\n<Val></Val>\r\n</String>\r\n<String>\r\n<Name> </Name>\r\n<Val></Val>\r\n</String>\r\n<String>\r\n<Name> </Name>\r\n<Val></Val>\r\n</String>\r\n<String>\r\n<Name> </Name>\r\n<Val></Val>\r\n</String>\r\n<String>\r\n<Name> </Name>\r\n<Val></Val>\r\n</String>\r\n<String>\r\n<Name> </Name>\r\n<Val></Val>\r\n</String>\r\n<String>\r\n<Name> </Name>\r\n<Val></Val>\r\n</String>\r\n<String>\r\n<Name> </Name>\r\n<Val></Val>\r\n</String>\r\n<String>\r\n<Name> </Name>\r\n<Val></Val>\r\n</String>\r\n<String>\r\n<Name> </Name>\r\n<Val></Val>\r\n</String>\r\n<String>\r\n<Name> </Name>\r\n<Val></Val>\r\n</String>\r\n<String>\r\n<Name> </Name>\r\n<Val></Val>\r\n</String>\r\n<String>\r\n<Name> </Name>\r\n<Val></Val>\r\n</String>\r\n<String>\r\n<Name> </Name>\r\n<Val></Val>\r\n</String>\r\n<String>\r\n<Name> </Name>\r\n<Val></Val>\r\n</String>\r\n<String>\r\n<Name> </Name>\r\n<Val></Val>\r\n</String>\r\n<String>\r\n<Name> </Name>\r\n<Val></Val>\r\n</String>\r\n<String>\r\n<Name> </Name>\r\n<Val></Val>\r\n</String>\r\n<String>\r\n<Name> </Name>\r\n<Val></Val>\r\n</String>\r\n<String>\r\n<Name> </Name>\r\n<Val></Val>\r\n</String>\r\n<String>\r\n<Name> </Name>\r\n<Val></Val>\r\n</String>\r\n<String>\r\n<Name> </Name>\r\n<Val></Val>\r\n</String>\r\n<String>\r\n<Name> </Name>\r\n<Val></Val>\r\n</String>\r\n<String>\r\n<Name> </Name>\r\n<Val></Val>\r\n</String>\r\n<String>\r\n<Name> </Name>\r\n<Val></Val>\r\n</String>\r\n<String>\r\n<Name> </Name>\r\n<Val></Val>\r\n</String>\r\n<String>\r\n<Name> </Name>\r\n<Val></Val>\r\n</String>\r\n<String>\r\n<Name> </Name>\r\n<Val></Val>\r\n</String>\r\n<String>\r\n<Name> </Name>\r\n<Val></Val>\r\n</String>\r\n<String>\r\n<Name> </Name>\r\n<Val></Val>\r\n</String>\r\n<String>\r\n<Name> </Name>\r\n<Val></Val>\r\n</String>\r\n<String>\r\n<Name> </Name>\r\n<Val></Val>\r\n</String>\r\n<String>\r\n<Name> </Name>\r\n<Val></Val>\r\n</String>\r\n<String>\r\n<Name> </Name>\r\n<Val></Val>\r\n</String>\r\n<String>\r\n<Name> </Name>\r\n<Val></Val>\r\n</String>\r\n<String>\r\n<Name> </Name>\r\n<Val></Val>\r\n</String>\r\n<String>\r\n<Name> </Name>\r\n<Val></Val>\r\n</String>\r\n<String>\r\n<Name> </Name>\r\n<Val></Val>\r\n</String>\r\n<String>\r\n<Name> </Name>\r\n<Val></Val>\r\n</String>\r\n<String>\r\n<Name> </Name>\r\n<Val></Val>\r\n</String>\r\n<String>\r\n<Name> </Name>\r\n<Val></Val>\r\n</String>\r\n<String>\r\n<Name> </Name>\r\n<Val></Val>\r\n</String>\r\n<String>\r\n<Name> </Name>\r\n<Val></Val>\r\n</String>\r\n<String>\r\n<Name> </Name>\r\n<Val></Val>\r\n</String>\r\n<String>\r\n<Name> </Name>\r\n<Val></Val>\r\n</String>\r\n<String>\r\n<Name> </Name>\r\n<Val></Val>\r\n</String>\r\n<String>\r\n<Name> </Name>\r\n<Val></Val>\r\n</String>\r\n<String>\r\n<Name> </Name>\r\n<Val></Val>\r\n</String>\r\n<String>\r\n<Name> </Name>\r\n<Val></Val>\r\n</String>\r\n<String>\r\n<Name> </Name>\r\n<Val></Val>\r\n</String>\r\n<String>\r\n<Name> </Name>\r\n<Val></Val>\r\n</String>\r\n<String>\r\n<Name> </Name>\r\n<Val></Val>\r\n</String>\r\n<String>\r\n<Name> </Name>\r\n<Val></Val>\r\n</String>\r\n<String>\r\n<Name> </Name>\r\n<Val></Val>\r\n</String>\r\n<String>\r\n<Name> </Name>\r\n<Val></Val>\r\n</String>\r\n<String>\r\n<Name> </Name>\r\n<Val></Val>\r\n</String>\r\n<String>\r\n<Name> </Name>\r\n<Val></Val>\r\n</String>\r\n<String>\r\n<Name> </Name>\r\n<Val></Val>\r\n</String>\r\n<String>\r\n<Name> </Name>\r\n<Val></Val>\r\n</String>\r\n<String>\r\n<Name> </Name>\r\n<Val></Val>\r\n</String>\r\n<String>\r\n<Name> </Name>\r\n<Val></Val>\r\n</String>\r\n<String>\r\n<Name> </Name>\r\n<Val></Val>\r\n</String>\r\n<String>\r\n<Name> </Name>\r\n<Val></Val>\r\n</String>\r\n<String>\r\n<Name> </Name>\r\n<Val></Val>\r\n</String>\r\n<String>\r\n<Name> </Name>\r\n<Val></Val>\r\n</String>\r\n<String>\r\n<Name> </Name>\r\n<Val></Val>\r\n</String>\r\n<String>\r\n<Name> </Name>\r\n<Val></Val>\r\n</String>\r\n<String>\r\n<Name> </Name>\r\n<Val></Val>\r\n</String>\r\n<String>\r\n<Name> </Name>\r\n<Val></Val>\r\n</String>\r\n<String>\r\n<Name> </Name>\r\n<Val></Val>\r\n</String>\r\n<String>\r\n<Name> </Name>\r\n<Val></Val>\r\n</String>\r\n<String>\r\n<Name> </Name>\r\n<Val></Val>\r\n</String>\r\n<String>\r\n<Name> </Name>\r\n<Val></Val>\r\n</String>\r\n<String>\r\n<Name> </Name>\r\n<Val></Val>\r\n</String>\r\n<String>\r\n<Name> </Name>\r\n<Val></Val>\r\n</String>\r\n<String>\r\n<Name> </Name>\r\n<Val></Val>\r\n</String>\r\n<String>\r\n<Name> </Name>\r\n<Val></Val>\r\n</String>\r\n<String>\r\n<Name> </Name>\r\n<Val></Val>\r\n</String>\r\n<String>\r\n<Name> </Name>\r\n<Val></Val>\r\n</String>\r\n<String>\r\n<Name> </Name>\r\n<Val></Val>\r\n</String>\r\n<String>\r\n<Name> </Name>\r\n<Val></Val>\r\n</String>\r\n<String>\r\n<Name> </Name>\r\n<Val></Val>\r\n</String>\r\n<String>\r\n<Name> </Name>\r\n<Val></Val>\r\n</String>\r\n<String>\r\n<Name> </Name>\r\n<Val></Val>\r\n</String>\r\n<String>\r\n<Name> </Name>\r\n<Val></Val>\r\n</String>\r\n<String>\r\n<Name> </Name>\r\n<Val></Val>\r\n</String>\r\n<String>\r\n<Name> </Name>\r\n<Val></Val>\r\n</String>\r\n<String>\r\n<Name> </Name>\r\n<Val></Val>\r\n</String>\r\n<String>\r\n<Name> </Name>\r\n<Val></Val>\r\n</String>\r\n<String>\r\n<Name> </Name>\r\n<Val></Val>\r\n</String>\r\n<String>\r\n<Name> </Name>\r\n<Val></Val>\r\n</String>\r\n<String>\r\n<Name> </Name>\r\n<Val></Val>\r\n</String>\r\n<String>\r\n<Name> </Name>\r\n<Val></Val>\r\n</String>\r\n<String>\r\n<Name> </Name>\r\n<Val></Val>\r\n</String>\r\n<String>\r\n<Name> </Name>\r\n<Val></Val>\r\n</String>\r\n<String>\r\n<Name> </Name>\r\n<Val></Val>\r\n</String>\r\n<String>\r\n<Name> </Name>\r\n<Val></Val>\r\n</String>\r\n<String>\r\n<Name> </Name>\r\n<Val></Val>\r\n</String>\r\n<String>\r\n<Name> </Name>\r\n<Val></Val>\r\n</String>\r\n<String>\r\n<Name> </Name>\r\n<Val></Val>\r\n</String>\r\n<String>\r\n<Name> </Name>\r\n<Val></Val>\r\n</String>\r\n<String>\r\n<Name> </Name>\r\n<Val></Val>\r\n</String>\r\n<String>\r\n<Name> </Name>\r\n<Val></Val>\r\n</String>\r\n<String>\r\n<Name> </Name>\r\n<Val></Val>\r\n</String>\r\n<String>\r\n<Name> </Name>\r\n<Val></Val>\r\n</String>\r\n<String>\r\n<Name> </Name>\r\n<Val></Val>\r\n</String>\r\n<String>\r\n<Name> </Name>\r\n<Val></Val>\r\n</String>\r\n<String>\r\n<Name> </Name>\r\n<Val></Val>\r\n</String>\r\n<String>\r\n<Name> </Name>\r\n<Val></Val>\r\n</String>\r\n<String>\r\n<Name> </Name>\r\n<Val></Val>\r\n</String>\r\n<String>\r\n<Name> </Name>\r\n<Val></Val>\r\n</String>\r\n<String>\r\n<Name> </Name>\r\n<Val></Val>\r\n</String>\r\n<String>\r\n<Name> </Name>\r\n<Val></Val>\r\n</String>\r\n<String>\r\n<Name> </Name>\r\n<Val></Val>\r\n</String>\r\n<String>\r\n<Name> </Name>\r\n<Val></Val>\r\n</String>\r\n<String>\r\n<Name> </Name>\r\n<Val></Val>\r\n</String>\r\n<String>\r\n<Name> </Name>\r\n<Val></Val>\r\n</String>\r\n<String>\r\n<Name> </Name>\r\n<Val></Val>\r\n</String>\r\n<String>\r\n<Name> </Name>\r\n<Val></Val>\r\n</String>\r\n<String>\r\n<Name> </Name>\r\n<Val></Val>\r\n</String>\r\n<String>\r\n<Name> </Name>\r\n<Val></Val>\r\n</String>\r\n<String>\r\n<Name> </Name>\r\n<Val></Val>\r\n</String>\r\n<String>\r\n<Name> </Name>\r\n<Val></Val>\r\n</String>\r\n<String>\r\n<Name> </Name>\r\n<Val></Val>\r\n</String>\r\n<String>\r\n<Name> </Name>\r\n<Val></Val>\r\n</String>\r\n<String>\r\n<Name> </Name>\r\n<Val></Val>\r\n</String>\r\n<String>\r\n<Name> </Name>\r\n<Val></Val>\r\n</String>\r\n<String>\r\n<Name> </Name>\r\n<Val></Val>\r\n</String>\r\n<String>\r\n<Name> </Name>\r\n<Val></Val>\r\n</String>\r\n<String>\r\n<Name> </Name>\r\n<Val></Val>\r\n</String>\r\n<String>\r\n<Name> </Name>\r\n<Val></Val>\r\n</String>\r\n<String>\r\n<Name> </Name>\r\n<Val></Val>\r\n</String>\r\n<String>\r\n<Name> </Name>\r\n<Val></Val>\r\n</String>\r\n<String>\r\n<Name> </Name>\r\n<Val></Val>\r\n</String>\r\n<String>\r\n<Name> </Name>\r\n<Val></Val>\r\n</String>\r\n<String>\r\n<Name> </Name>\r\n<Val></Val>\r\n</String>\r\n<String>\r\n<Name> </Name>\r\n<Val></Val>\r\n</String>\r\n<String>\r\n<Name> </Name>\r\n<Val></Val>\r\n</String>\r\n<String>\r\n<Name> </Name>\r\n<Val></Val>\r\n</String>\r\n<String>\r\n<Name> </Name>\r\n<Val></Val>\r\n</String>\r\n<String>\r\n<Name> </Name>\r\n<Val></Val>\r\n</String>\r\n<String>\r\n<Name> </Name>\r\n<Val></Val>\r\n</String>\r\n<String>\r\n<Name> </Name>\r\n<Val></Val>\r\n</String>\r\n<String>\r\n<Name> </Name>\r\n<Val></Val>\r\n</String>\r\n<String>\r\n<Name> </Name>\r\n<Val></Val>\r\n</String>\r\n<String>\r\n<Name> </Name>\r\n<Val></Val>\r\n</String>\r\n<String>\r\n<Name> </Name>\r\n<Val></Val>\r\n</String>\r\n<String>\r\n<Name> </Name>\r\n<Val></Val>\r\n</String>\r\n<String>\r\n<Name> </Name>\r\n<Val></Val>\r\n</String>\r\n<String>\r\n<Name> </Name>\r\n<Val></Val>\r\n</String>\r\n<String>\r\n<Name> </Name>\r\n<Val></Val>\r\n</String>\r\n<String>\r\n<Name> </Name>\r\n<Val></Val>\r\n</String>\r\n<String>\r\n<Name> </Name>\r\n<Val></Val>\r\n</String>\r\n<String>\r\n<Name> </Name>\r\n<Val></Val>\r\n</String>\r\n<String>\r\n<Name> </Name>\r\n<Val></Val>\r\n</String>\r\n<String>\r\n<Name> </Name>\r\n<Val></Val>\r\n</String>\r\n<String>\r\n<Name> </Name>\r\n<Val></Val>\r\n</String>\r\n<String>\r\n<Name> </Name>\r\n<Val></Val>\r\n</String>\r\n<String>\r\n<Name> </Name>\r\n<Val></Val>\r\n</String>\r\n<String>\r\n<Name> </Name>\r\n<Val></Val>\r\n</String>\r\n<String>\r\n<Name> </Name>\r\n<Val></Val>\r\n</String>\r\n<String>\r\n<Name> </Name>\r\n<Val></Val>\r\n</String>\r\n<String>\r\n<Name> </Name>\r\n<Val></Val>\r\n</String>\r\n<String>\r\n<Name> </Name>\r\n<Val></Val>\r\n</String>\r\n<String>\r\n<Name> </Name>\r\n<Val></Val>\r\n</String>\r\n<String>\r\n<Name> </Name>\r\n<Val></Val>\r\n</String>\r\n<String>\r\n<Name> </Name>\r\n<Val></Val>\r\n</String>\r\n<String>\r\n<Name> </Name>\r\n<Val></Val>\r\n</String>\r\n<String>\r\n<Name> </Name>\r\n<Val></Val>\r\n</String>\r\n<String>\r\n<Name> </Name>\r\n<Val></Val>\r\n</String>\r\n<String>\r\n<Name> </Name>\r\n<Val></Val>\r\n</String>\r\n<String>\r\n<Name> </Name>\r\n<Val></Val>\r\n</String>\r\n<String>\r\n<Name> </Name>\r\n<Val></Val>\r\n</String>\r\n<String>\r\n<Name> </Name>\r\n<Val></Val>\r\n</String>\r\n<String>\r\n<Name> </Name>\r\n<Val></Val>\r\n</String>\r\n<String>\r\n<Name> </Name>\r\n<Val></Val>\r\n</String>\r\n<String>\r\n<Name> </Name>\r\n<Val></Val>\r\n</String>\r\n<String>\r\n<Name> </Name>\r\n<Val></Val>\r\n</String>\r\n<String>\r\n<Name> </Name>\r\n<Val></Val>\r\n</String>\r\n<String>\r\n<Name> </Name>\r\n<Val></Val>\r\n</String>\r\n<String>\r\n<Name> </Name>\r\n<Val></Val>\r\n</String>\r\n<String>\r\n<Name> </Name>\r\n<Val></Val>\r\n</String>\r\n<String>\r\n<Name> </Name>\r\n<Val></Val>\r\n</String>\r\n<String>\r\n<Name> </Name>\r\n<Val></Val>\r\n</String>\r\n<String>\r\n<Name> </Name>\r\n<Val></Val>\r\n</String>\r\n<String>\r\n<Name> </Name>\r\n<Val></Val>\r\n</String>\r\n<String>\r\n<Name> </Name>\r\n<Val></Val>\r\n</String>\r\n<String>\r\n<Name> </Name>\r\n<Val></Val>\r\n</String>\r\n<String>\r\n<Name> </Name>\r\n<Val></Val>\r\n</String>\r\n<String>\r\n<Name> </Name>\r\n<Val></Val>\r\n</String>\r\n<String>\r\n<Name> </Name>\r\n<Val></Val>\r\n</String>\r\n<String>\r\n<Name> </Name>\r\n<Val></Val>\r\n</String>\r\n<String>\r\n<Name> </Name>\r\n<Val></Val>\r\n</String>\r\n<String>\r\n<Name> </Name>\r\n<Val></Val>\r\n</String>\r\n<String>\r\n<Name> </Name>\r\n<Val></Val>\r\n</String>\r\n<String>\r\n<Name> </Name>\r\n<Val></Val>\r\n</String>\r\n<String>\r\n<Name> </Name>\r\n<Val></Val>\r\n</String>\r\n<String>\r\n<Name> </Name>\r\n<Val></Val>\r\n</String>\r\n<String>\r\n<Name> </Name>\r\n<Val></Val>\r\n</String>\r\n<String>\r\n<Name> </Name>\r\n<Val></Val>\r\n</String>\r\n<String>\r\n<Name> </Name>\r\n<Val></Val>\r\n</String>\r\n<String>\r\n<Name> </Name>\r\n<Val></Val>\r\n</String>\r\n<String>\r\n<Name> </Name>\r\n<Val></Val>\r\n</String>\r\n<String>\r\n<Name> </Name>\r\n<Val></Val>\r\n</String>\r\n<String>\r\n<Name> </Name>\r\n<Val></Val>\r\n</String>\r\n<String>\r\n<Name> </Name>\r\n<Val></Val>\r\n</String>\r\n<String>\r\n<Name> </Name>\r\n<Val></Val>\r\n</String>\r\n<String>\r\n<Name> </Name>\r\n<Val></Val>\r\n</String>\r\n<String>\r\n<Name> </Name>\r\n<Val></Val>\r\n</String>\r\n<String>\r\n<Name> </Name>\r\n<Val></Val>\r\n</String>\r\n<String>\r\n<Name> </Name>\r\n<Val></Val>\r\n</String>\r\n<String>\r\n<Name> </Name>\r\n<Val></Val>\r\n</String>\r\n<String>\r\n<Name> </Name>\r\n<Val></Val>\r\n</String>\r\n<String>\r\n<Name> </Name>\r\n<Val></Val>\r\n</String>\r\n<String>\r\n<Name> </Name>\r\n<Val></Val>\r\n</String>\r\n<String>\r\n<Name> </Name>\r\n<Val></Val>\r\n</String>\r\n<String>\r\n<Name> </Name>\r\n<Val></Val>\r\n</String>\r\n<String>\r\n<Name> </Name>\r\n<Val></Val>\r\n</String>\r\n<String>\r\n<Name> </Name>\r\n<Val></Val>\r\n</String>\r\n<String>\r\n<Name> </Name>\r\n<Val></Val>\r\n</String>\r\n<String>\r\n<Name> </Name>\r\n<Val></Val>\r\n</String>\r\n<String>\r\n<Name> </Name>\r\n<Val></Val>\r\n</String>\r\n<String>\r\n<Name> </Name>\r\n<Val></Val>\r\n</String>\r\n<String>\r\n<Name> </Name>\r\n<Val></Val>\r\n</String>\r\n<String>\r\n<Name> </Name>\r\n<Val></Val>\r\n</String>\r\n<String>\r\n<Name> </Name>\r\n<Val></Val>\r\n</String>\r\n<String>\r\n<Name> </Name>\r\n<Val></Val>\r\n</String>\r\n<String>\r\n<Name> </Name>\r\n<Val></Val>\r\n</String>\r\n<String>\r\n<Name> </Name>\r\n<Val></Val>\r\n</String>\r\n<String>\r\n<Name> </Name>\r\n<Val></Val>\r\n</String>\r\n<String>\r\n<Name> </Name>\r\n<Val></Val>\r\n</String>\r\n<String>\r\n<Name> </Name>\r\n<Val></Val>\r\n</String>\r\n<String>\r\n<Name> </Name>\r\n<Val></Val>\r\n</String>\r\n<String>\r\n<Name> </Name>\r\n<Val></Val>\r\n</String>\r\n<String>\r\n<Name> </Name>\r\n<Val></Val>\r\n</String>\r\n<String>\r\n<Name> </Name>\r\n<Val></Val>\r\n</String>\r\n<String>\r\n<Name> </Name>\r\n<Val></Val>\r\n</String>\r\n<String>\r\n<Name> </Name>\r\n<Val></Val>\r\n</String>\r\n<String>\r\n<Name> </Name>\r\n<Val></Val>\r\n</String>\r\n<String>\r\n<Name> </Name>\r\n<Val></Val>\r\n</String>\r\n<String>\r\n<Name> </Name>\r\n<Val></Val>\r\n</String>\r\n<String>\r\n<Name> </Name>\r\n<Val></Val>\r\n</String>\r\n<String>\r\n<Name> </Name>\r\n<Val></Val>\r\n</String>\r\n<String>\r\n<Name> </Name>\r\n<Val></Val>\r\n</String>\r\n<String>\r\n<Name> </Name>\r\n<Val></Val>\r\n</String>\r\n<String>\r\n<Name> </Name>\r\n<Val></Val>\r\n</String>\r\n<String>\r\n<Name> </Name>\r\n<Val></Val>\r\n</String>\r\n<String>\r\n<Name> </Name>\r\n<Val></Val>\r\n</String>\r\n<String>\r\n<Name> </Name>\r\n<Val></Val>\r\n</String>\r\n<String>\r\n<Name> </Name>\r\n<Val></Val>\r\n</String>\r\n<String>\r\n<Name> </Name>\r\n<Val></Val>\r\n</String>\r\n<String>\r\n<Name> </Name>\r\n<Val></Val>\r\n</String>\r\n<String>\r\n<Name> </Name>\r\n<Val></Val>\r\n</String>\r\n<String>\r\n<Name> </Name>\r\n<Val></Val>\r\n</String>\r\n<String>\r\n<Name> </Name>\r\n<Val></Val>\r\n</String>\r\n<String>\r\n<Name> </Name>\r\n<Val></Val>\r\n</String>\r\n<String>\r\n<Name> </Name>\r\n<Val></Val>\r\n</String>\r\n<String>\r\n<Name> </Name>\r\n<Val></Val>\r\n</String>\r\n<String>\r\n<Name> </Name>\r\n<Val></Val>\r\n</String>\r\n<String>\r\n<Name> </Name>\r\n<Val></Val>\r\n</String>\r\n<String>\r\n<Name> </Name>\r\n<Val></Val>\r\n</String>\r\n<String>\r\n<Name> </Name>\r\n<Val></Val>\r\n</String>\r\n<String>\r\n<Name> </Name>\r\n<Val></Val>\r\n</String>\r\n<String>\r\n<Name> </Name>\r\n<Val></Val>\r\n</String>\r\n<String>\r\n<Name> </Name>\r\n<Val></Val>\r\n</String>\r\n<String>\r\n<Name> </Name>\r\n<Val></Val>\r\n</String>\r\n<String>\r\n<Name> </Name>\r\n<Val></Val>\r\n</String>\r\n<String>\r\n<Name> </Name>\r\n<Val></Val>\r\n</String>\r\n<String>\r\n<Name> </Name>\r\n<Val></Val>\r\n</String>\r\n<String>\r\n<Name> </Name>\r\n<Val></Val>\r\n</String>\r\n<String>\r\n<Name> </Name>\r\n<Val></Val>\r\n</String>\r\n<String>\r\n<Name> </Name>\r\n<Val></Val>\r\n</String>\r\n<String>\r\n<Name> </Name>\r\n<Val></Val>\r\n</String>\r\n<String>\r\n<Name> </Name>\r\n<Val></Val>\r\n</String>\r\n<String>\r\n<Name> </Name>\r\n<Val></Val>\r\n</String>\r\n<String>\r\n<Name> </Name>\r\n<Val></Val>\r\n</String>\r\n<String>\r\n<Name> </Name>\r\n<Val></Val>\r\n</String>\r\n<String>\r\n<Name> </Name>\r\n<Val></Val>\r\n</String>\r\n<String>\r\n<Name> </Name>\r\n<Val></Val>\r\n</String>\r\n<String>\r\n<Name> </Name>\r\n<Val></Val>\r\n</String>\r\n<String>\r\n<Name> </Name>\r\n<Val></Val>\r\n</String>\r\n<String>\r\n<Name> </Name>\r\n<Val></Val>\r\n</String>\r\n<String>\r\n<Name> </Name>\r\n<Val></Val>\r\n</String>\r\n<String>\r\n<Name> </Name>\r\n<Val></Val>\r\n</String>\r\n<String>\r\n<Name> </Name>\r\n<Val></Val>\r\n</String>\r\n<String>\r\n<Name> </Name>\r\n<Val></Val>\r\n</String>\r\n<String>\r\n<Name> </Name>\r\n<Val></Val>\r\n</String>\r\n<String>\r\n<Name> </Name>\r\n<Val></Val>\r\n</String>\r\n<String>\r\n<Name> </Name>\r\n<Val></Val>\r\n</String>\r\n<String>\r\n<Name> </Name>\r\n<Val></Val>\r\n</String>\r\n<String>\r\n<Name> </Name>\r\n<Val></Val>\r\n</String>\r\n<String>\r\n<Name> </Name>\r\n<Val></Val>\r\n</String>\r\n<String>\r\n<Name> </Name>\r\n<Val></Val>\r\n</String>\r\n<String>\r\n<Name> </Name>\r\n<Val></Val>\r\n</String>\r\n<String>\r\n<Name> </Name>\r\n<Val></Val>\r\n</String>\r\n<String>\r\n<Name> </Name>\r\n<Val></Val>\r\n</String>\r\n<String>\r\n<Name> </Name>\r\n<Val></Val>\r\n</String>\r\n<String>\r\n<Name> </Name>\r\n<Val></Val>\r\n</String>\r\n<String>\r\n<Name> </Name>\r\n<Val></Val>\r\n</String>\r\n<String>\r\n<Name> </Name>\r\n<Val></Val>\r\n</String>\r\n<String>\r\n<Name> </Name>\r\n<Val></Val>\r\n</String>\r\n<String>\r\n<Name> </Name>\r\n<Val></Val>\r\n</String>\r\n<String>\r\n<Name> </Name>\r\n<Val></Val>\r\n</String>\r\n<String>\r\n<Name> </Name>\r\n<Val></Val>\r\n</String>\r\n<String>\r\n<Name> </Name>\r\n<Val></Val>\r\n</String>\r\n<String>\r\n<Name> </Name>\r\n<Val></Val>\r\n</String>\r\n<String>\r\n<Name> </Name>\r\n<Val></Val>\r\n</String>\r\n<String>\r\n<Name> </Name>\r\n<Val></Val>\r\n</String>\r\n<String>\r\n<Name> </Name>\r\n<Val></Val>\r\n</String>\r\n<String>\r\n<Name> </Name>\r\n<Val></Val>\r\n</String>\r\n<String>\r\n<Name> </Name>\r\n<Val></Val>\r\n</String>\r\n<String>\r\n<Name> </Name>\r\n<Val></Val>\r\n</String>\r\n<String>\r\n<Name> </Name>\r\n<Val></Val>\r\n</String>\r\n<String>\r\n<Name> </Name>\r\n<Val></Val>\r\n</String>\r\n<String>\r\n<Name> </Name>\r\n<Val></Val>\r\n</String>\r\n<String>\r\n<Name> </Name>\r\n<Val></Val>\r\n</String>\r\n<String>\r\n<Name> </Name>\r\n<Val></Val>\r\n</String>\r\n<String>\r\n<Name> </Name>\r\n<Val></Val>\r\n</String>\r\n<String>\r\n<Name> </Name>\r\n<Val></Val>\r\n</String>\r\n<String>\r\n<Name> </Name>\r\n<Val></Val>\r\n</String>\r\n<String>\r\n<Name> </Name>\r\n<Val></Val>\r\n</String>\r\n<String>\r\n<Name> </Name>\r\n<Val></Val>\r\n</String>\r\n<String>\r\n<Name> </Name>\r\n<Val></Val>\r\n</String>\r\n<String>\r\n<Name> </Name>\r\n<Val></Val>\r\n</String>\r\n<String>\r\n<Name> </Name>\r\n<Val></Val>\r\n</String>\r\n<String>\r\n<Name> </Name>\r\n<Val></Val>\r\n</String>\r\n<String>\r\n<Name> </Name>\r\n<Val></Val>\r\n</String>\r\n<String>\r\n<Name> </Name>\r\n<Val></Val>\r\n</String>\r\n<String>\r\n<Name> </Name>\r\n<Val></Val>\r\n</String>\r\n<String>\r\n<Name> </Name>\r\n<Val></Val>\r\n</String>\r\n<String>\r\n<Name> </Name>\r\n<Val></Val>\r\n</String>\r\n<String>\r\n<Name> </Name>\r\n<Val></Val>\r\n</String>\r\n<String>\r\n<Name> </Name>\r\n<Val></Val>\r\n</String>\r\n<String>\r\n<Name> </Name>\r\n<Val></Val>\r\n</String>\r\n<String>\r\n<Name> </Name>\r\n<Val></Val>\r\n</String>\r\n<String>\r\n<Name> </Name>\r\n<Val></Val>\r\n</String>\r\n<String>\r\n<Name> </Name>\r\n<Val></Val>\r\n</String>\r\n<String>\r\n<Name> </Name>\r\n<Val></Val>\r\n</String>\r\n<String>\r\n<Name> </Name>\r\n<Val></Val>\r\n</String>\r\n<String>\r\n<Name> </Name>\r\n<Val></Val>\r\n</String>\r\n<String>\r\n<Name> </Name>\r\n<Val></Val>\r\n</String>\r\n<String>\r\n<Name> </Name>\r\n<Val></Val>\r\n</String>\r\n<String>\r\n<Name> </Name>\r\n<Val></Val>\r\n</String>\r\n<String>\r\n<Name> </Name>\r\n<Val></Val>\r\n</String>\r\n<String>\r\n<Name> </Name>\r\n<Val></Val>\r\n</String>\r\n<String>\r\n<Name> </Name>\r\n<Val></Val>\r\n</String>\r\n<String>\r\n<Name> </Name>\r\n<Val></Val>\r\n</String>\r\n<String>\r\n<Name> </Name>\r\n<Val></Val>\r\n</String>\r\n<String>\r\n<Name> </Name>\r\n<Val></Val>\r\n</String>\r\n<String>\r\n<Name> </Name>\r\n<Val></Val>\r\n</String>\r\n<String>\r\n<Name> </Name>\r\n<Val></Val>\r\n</String>\r\n<String>\r\n<Name> </Name>\r\n<Val></Val>\r\n</String>\r\n<String>\r\n<Name> </Name>\r\n<Val></Val>\r\n</String>\r\n<String>\r\n<Name> </Name>\r\n<Val></Val>\r\n</String>\r\n<String>\r\n<Name> </Name>\r\n<Val></Val>\r\n</String>\r\n<String>\r\n<Name> </Name>\r\n<Val></Val>\r\n</String>\r\n<String>\r\n<Name> </Name>\r\n<Val></Val>\r\n</String>\r\n<String>\r\n<Name> </Name>\r\n<Val></Val>\r\n</String>\r\n<String>\r\n<Name> </Name>\r\n<Val></Val>\r\n</String>\r\n<String>\r\n<Name> </Name>\r\n<Val></Val>\r\n</String>\r\n<String>\r\n<Name> </Name>\r\n<Val></Val>\r\n</String>\r\n<String>\r\n<Name> </Name>\r\n<Val></Val>\r\n</String>\r\n<String>\r\n<Name> </Name>\r\n<Val></Val>\r\n</String>\r\n<String>\r\n<Name> </Name>\r\n<Val></Val>\r\n</String>\r\n<String>\r\n<Name> </Name>\r\n<Val></Val>\r\n</String>\r\n<String>\r\n<Name> </Name>\r\n<Val></Val>\r\n</String>\r\n<String>\r\n<Name> </Name>\r\n<Val></Val>\r\n</String>\r\n<String>\r\n<Name> </Name>\r\n<Val></Val>\r\n</String>\r\n<String>\r\n<Name> </Name>\r\n<Val></Val>\r\n</String>\r\n<String>\r\n<Name> </Name>\r\n<Val></Val>\r\n</String>\r\n<String>\r\n<Name> </Name>\r\n<Val></Val>\r\n</String>\r\n<String>\r\n<Name> </Name>\r\n<Val></Val>\r\n</String>\r\n<String>\r\n<Name> </Name>\r\n<Val></Val>\r\n</String>\r\n<String>\r\n<Name> </Name>\r\n<Val></Val>\r\n</String>\r\n<String>\r\n<Name> </Name>\r\n<Val></Val>\r\n</String>\r\n<String>\r\n<Name> </Name>\r\n<Val></Val>\r\n</String>\r\n<String>\r\n<Name> </Name>\r\n<Val></Val>\r\n</String>\r\n<String>\r\n<Name> </Name>\r\n<Val></Val>\r\n</String>\r\n<String>\r\n<Name> </Name>\r\n<Val></Val>\r\n</String>\r\n<String>\r\n<Name> </Name>\r\n<Val></Val>\r\n</String>\r\n<String>\r\n<Name> </Name>\r\n<Val></Val>\r\n</String>\r\n<String>\r\n<Name> </Name>\r\n<Val></Val>\r\n</String>\r\n<String>\r\n<Name> </Name>\r\n<Val></Val>\r\n</String>\r\n<String>\r\n<Name> </Name>\r\n<Val></Val>\r\n</String>\r\n<String>\r\n<Name> </Name>\r\n<Val></Val>\r\n</String>\r\n<String>\r\n<Name> </Name>\r\n<Val></Val>\r\n</String>\r\n<String>\r\n<Name> </Name>\r\n<Val></Val>\r\n</String>\r\n<String>\r\n<Name> </Name>\r\n<Val></Val>\r\n</String>\r\n<String>\r\n<Name> </Name>\r\n<Val></Val>\r\n</String>\r\n<String>\r\n<Name> </Name>\r\n<Val></Val>\r\n</String>\r\n<String>\r\n<Name> </Name>\r\n<Val></Val>\r\n</String>\r\n<String>\r\n<Name> </Name>\r\n<Val></Val>\r\n</String>\r\n<String>\r\n<Name> </Name>\r\n<Val></Val>\r\n</String>\r\n<String>\r\n<Name> </Name>\r\n<Val></Val>\r\n</String>\r\n<String>\r\n<Name> </Name>\r\n<Val></Val>\r\n</String>\r\n<String>\r\n<Name> </Name>\r\n<Val></Val>\r\n</String>\r\n<String>\r\n<Name> </Name>\r\n<Val></Val>\r\n</String>\r\n<String>\r\n<Name> </Name>\r\n<Val></Val>\r\n</String>\r\n<String>\r\n<Name> </Name>\r\n<Val></Val>\r\n</String>\r\n<String>\r\n<Name> </Name>\r\n<Val></Val>\r\n</String>\r\n<String>\r\n<Name> </Name>\r\n<Val></Val>\r\n</String>\r\n<String>\r\n<Name> </Name>\r\n<Val></Val>\r\n</String>\r\n<String>\r\n<Name> </Name>\r\n<Val></Val>\r\n</String>\r\n<String>\r\n<Name> </Name>\r\n<Val></Val>\r\n</String>\r\n<String>\r\n<Name> </Name>\r\n<Val></Val>\r\n</String>\r\n<String>\r\n<Name> </Name>\r\n<Val></Val>\r\n</String>\r\n<String>\r\n<Name> </Name>\r\n<Val></Val>\r\n</String>\r\n<String>\r\n<Name> </Name>\r\n<Val></Val>\r\n</String>\r\n<String>\r\n<Name> </Name>\r\n<Val></Val>\r\n</String>\r\n<String>\r\n<Name> </Name>\r\n<Val></Val>\r\n</String>\r\n<String>\r\n<Name> </Name>\r\n<Val></Val>\r\n</String>\r\n<String>\r\n<Name> </Name>\r\n<Val></Val>\r\n</String>\r\n<String>\r\n<Name> </Name>\r\n<Val></Val>\r\n</String>\r\n<String>\r\n<Name> </Name>\r\n<Val></Val>\r\n</String>\r\n<String>\r\n<Name> </Name>\r\n<Val></Val>\r\n</String>\r\n<String>\r\n<Name> </Name>\r\n<Val></Val>\r\n</String>\r\n<String>\r\n<Name> </Name>\r\n<Val></Val>\r\n</String>\r\n<String>\r\n<Name> </Name>\r\n<Val></Val>\r\n</String>\r\n<String>\r\n<Name> </Name>\r\n<Val></Val>\r\n</String>\r\n<String>\r\n<Name> </Name>\r\n<Val></Val>\r\n</String>\r\n<String>\r\n<Name> </Name>\r\n<Val></Val>\r\n</String>\r\n<String>\r\n<Name> </Name>\r\n<Val></Val>\r\n</String>\r\n<String>\r\n<Name> </Name>\r\n<Val></Val>\r\n</String>\r\n<String>\r\n<Name> </Name>\r\n<Val></Val>\r\n</String>\r\n<String>\r\n<Name> </Name>\r\n<Val></Val>\r\n</String>\r\n<String>\r\n<Name> </Name>\r\n<Val></Val>\r\n</String>\r\n<String>\r\n<Name> </Name>\r\n<Val></Val>\r\n</String>\r\n<String>\r\n<Name> </Name>\r\n<Val></Val>\r\n</String>\r\n<String>\r\n<Name> </Name>\r\n<Val></Val>\r\n</String>\r\n<String>\r\n<Name> </Name>\r\n<Val></Val>\r\n</String>\r\n<String>\r\n<Name> </Name>\r\n<Val></Val>\r\n</String>\r\n<String>\r\n<Name> </Name>\r\n<Val></Val>\r\n</String>\r\n<String>\r\n<Name> </Name>\r\n<Val></Val>\r\n</String>\r\n<String>\r\n<Name> </Name>\r\n<Val></Val>\r\n</String>\r\n<String>\r\n<Name> </Name>\r\n<Val></Val>\r\n</String>\r\n<String>\r\n<Name> </Name>\r\n<Val></Val>\r\n</String>\r\n<String>\r\n<Name> </Name>\r\n<Val></Val>\r\n</String>\r\n<String>\r\n<Name> </Name>\r\n<Val></Val>\r\n</String>\r\n<String>\r\n<Name> </Name>\r\n<Val></Val>\r\n</String>\r\n<String>\r\n<Name> </Name>\r\n<Val></Val>\r\n</String>\r\n<String>\r\n<Name> </Name>\r\n<Val></Val>\r\n</String>\r\n<String>\r\n<Name> </Name>\r\n<Val></Val>\r\n</String>\r\n<String>\r\n<Name> </Name>\r\n<Val></Val>\r\n</String>\r\n<String>\r\n<Name> </Name>\r\n<Val></Val>\r\n</String>\r\n<String>\r\n<Name> </Name>\r\n<Val></Val>\r\n</String>\r\n<String>\r\n<Name> </Name>\r\n<Val></Val>\r\n</String>\r\n<String>\r\n<Name> </Name>\r\n<Val></Val>\r\n</String>\r\n<String>\r\n<Name> </Name>\r\n<Val></Val>\r\n</String>\r\n<String>\r\n<Name> </Name>\r\n<Val></Val>\r\n</String>\r\n<String>\r\n<Name> </Name>\r\n<Val></Val>\r\n</String>\r\n<String>\r\n<Name> </Name>\r\n<Val></Val>\r\n</String>\r\n<String>\r\n<Name> </Name>\r\n<Val></Val>\r\n</String>\r\n<String>\r\n<Name> </Name>\r\n<Val></Val>\r\n</String>\r\n<String>\r\n<Name> </Name>\r\n<Val></Val>\r\n</String>\r\n<String>\r\n<Name> </Name>\r\n<Val></Val>\r\n</String>\r\n<String>\r\n<Name> </Name>\r\n<Val></Val>\r\n</String>\r\n<String>\r\n<Name> </Name>\r\n<Val></Val>\r\n</String>\r\n<String>\r\n<Name> </Name>\r\n<Val></Val>\r\n</String>\r\n<String>\r\n<Name> </Name>\r\n<Val></Val>\r\n</String>\r\n<String>\r\n<Name> </Name>\r\n<Val></Val>\r\n</String>\r\n<String>\r\n<Name> </Name>\r\n<Val></Val>\r\n</String>\r\n<String>\r\n<Name> </Name>\r\n<Val></Val>\r\n</String>\r\n<String>\r\n<Name> </Name>\r\n<Val></Val>\r\n</String>\r\n<String>\r\n<Name> </Name>\r\n<Val></Val>\r\n</String>\r\n<String>\r\n<Name> </Name>\r\n<Val></Val>\r\n</String>\r\n<String>\r\n<Name> </Name>\r\n<Val></Val>\r\n</String>\r\n<String>\r\n<Name> </Name>\r\n<Val></Val>\r\n</String>\r\n<String>\r\n<Name> </Name>\r\n<Val></Val>\r\n</String>\r\n<String>\r\n<Name> </Name>\r\n<Val></Val>\r\n</String>\r\n<String>\r\n<Name> </Name>\r\n<Val></Val>\r\n</String>\r\n<String>\r\n<Name> </Name>\r\n<Val></Val>\r\n</String>\r\n<String>\r\n<Name> </Name>\r\n<Val></Val>\r\n</String>\r\n<String>\r\n<Name> </Name>\r\n<Val></Val>\r\n</String>\r\n<String>\r\n<Name> </Name>\r\n<Val></Val>\r\n</String>\r\n<String>\r\n<Name> </Name>\r\n<Val></Val>\r\n</String>\r\n<String>\r\n<Name> </Name>\r\n<Val></Val>\r\n</String>\r\n<String>\r\n<Name> </Name>\r\n<Val></Val>\r\n</String>\r\n<String>\r\n<Name> </Name>\r\n<Val></Val>\r\n</String>\r\n<String>\r\n<Name> </Name>\r\n<Val></Val>\r\n</String>\r\n<String>\r\n<Name> </Name>\r\n<Val></Val>\r\n</String>\r\n<String>\r\n<Name> </Name>\r\n<Val></Val>\r\n</String>\r\n<String>\r\n<Name> </Name>\r\n<Val></Val>\r\n</String>\r\n<String>\r\n<Name> </Name>\r\n<Val></Val>\r\n</String>\r\n<String>\r\n<Name> </Name>\r\n<Val></Val>\r\n</String>\r\n<String>\r\n<Name> </Name>\r\n<Val></Val>\r\n</String>\r\n<String>\r\n<Name> </Name>\r\n<Val></Val>\r\n</String>\r\n<String>\r\n<Name> </Name>\r\n<Val></Val>\r\n</String>\r\n<String>\r\n<Name> </Name>\r\n<Val></Val>\r\n</String>\r\n<String>\r\n<Name> </Name>\r\n<Val></Val>\r\n</String>\r\n<String>\r\n<Name> </Name>\r\n<Val></Val>\r\n</String>\r\n<String>\r\n<Name> </Name>\r\n<Val></Val>\r\n</String>\r\n<String>\r\n<Name> </Name>\r\n<Val></Val>\r\n</String>\r\n<String>\r\n<Name> </Name>\r\n<Val></Val>\r\n</String>\r\n<String>\r\n<Name> </Name>\r\n<Val></Val>\r\n</String>\r\n<String>\r\n<Name> </Name>\r\n<Val></Val>\r\n</String>\r\n<String>\r\n<Name> </Name>\r\n<Val></Val>\r\n</String>\r\n<String>\r\n<Name> </Name>\r\n<Val></Val>\r\n</String>\r\n<String>\r\n<Name> </Name>\r\n<Val></Val>\r\n</String>\r\n<String>\r\n<Name> </Name>\r\n<Val></Val>\r\n</String>\r\n<String>\r\n<Name> </Name>\r\n<Val></Val>\r\n</String>\r\n<String>\r\n<Name> </Name>\r\n<Val></Val>\r\n</String>\r\n<String>\r\n<Name> </Name>\r\n<Val></Val>\r\n</String>\r\n<String>\r\n<Name> </Name>\r\n<Val></Val>\r\n</String>\r\n<String>\r\n<Name> </Name>\r\n<Val></Val>\r\n</String>\r\n<String>\r\n<Name> </Name>\r\n<Val></Val>\r\n</String>\r\n<String>\r\n<Name> </Name>\r\n<Val></Val>\r\n</String>\r\n<String>\r\n<Name> </Name>\r\n<Val></Val>\r\n</String>\r\n<String>\r\n<Name> </Name>\r\n<Val></Val>\r\n</String>\r\n<String>\r\n<Name> </Name>\r\n<Val></Val>\r\n</String>\r\n<String>\r\n<Name> </Name>\r\n<Val></Val>\r\n</String>\r\n<String>\r\n<Name> </Name>\r\n<Val></Val>\r\n</String>\r\n<String>\r\n<Name> </Name>\r\n<Val></Val>\r\n</String>\r\n<String>\r\n<Name> </Name>\r\n<Val></Val>\r\n</String>\r\n<String>\r\n<Name> </Name>\r\n<Val></Val>\r\n</String>\r\n<String>\r\n<Name> </Name>\r\n<Val></Val>\r\n</String>\r\n<String>\r\n<Name> </Name>\r\n<Val></Val>\r\n</String>\r\n<String>\r\n<Name> </Name>\r\n<Val></Val>\r\n</String>\r\n<String>\r\n<Name> </Name>\r\n<Val></Val>\r\n</String>\r\n<String>\r\n<Name> </Name>\r\n<Val></Val>\r\n</String>\r\n<String>\r\n<Name> </Name>\r\n<Val></Val>\r\n</String>\r\n<String>\r\n<Name> </Name>\r\n<Val></Val>\r\n</String>\r\n<String>\r\n<Name> </Name>\r\n<Val></Val>\r\n</String>\r\n<String>\r\n<Name> </Name>\r\n<Val></Val>\r\n</String>\r\n<String>\r\n<Name> </Name>\r\n<Val></Val>\r\n</String>\r\n<String>\r\n<Name> </Name>\r\n<Val></Val>\r\n</String>\r\n<String>\r\n<Name> </Name>\r\n<Val></Val>\r\n</String>\r\n<String>\r\n<Name> </Name>\r\n<Val></Val>\r\n</String>\r\n<String>\r\n<Name> </Name>\r\n<Val></Val>\r\n</String>\r\n<String>\r\n<Name> </Name>\r\n<Val></Val>\r\n</String>\r\n<String>\r\n<Name> </Name>\r\n<Val></Val>\r\n</String>\r\n<String>\r\n<Name> </Name>\r\n<Val></Val>\r\n</String>\r\n<String>\r\n<Name> </Name>\r\n<Val></Val>\r\n</String>\r\n<String>\r\n<Name> </Name>\r\n<Val></Val>\r\n</String>\r\n<String>\r\n<Name> </Name>\r\n<Val></Val>\r\n</String>\r\n<String>\r\n<Name> </Name>\r\n<Val></Val>\r\n</String>\r\n<String>\r\n<Name> </Name>\r\n<Val></Val>\r\n</String>\r\n<String>\r\n<Name> </Name>\r\n<Val></Val>\r\n</String>\r\n<String>\r\n<Name> </Name>\r\n<Val></Val>\r\n</String>\r\n<String>\r\n<Name> </Name>\r\n<Val></Val>\r\n</String>\r\n<String>\r\n<Name> </Name>\r\n<Val></Val>\r\n</String>\r\n<String>\r\n<Name> </Name>\r\n<Val></Val>\r\n</String>\r\n<String>\r\n<Name> </Name>\r\n<Val></Val>\r\n</String>\r\n<String>\r\n<Name> </Name>\r\n<Val></Val>\r\n</String>\r\n<String>\r\n<Name> </Name>\r\n<Val></Val>\r\n</String>\r\n<String>\r\n<Name> </Name>\r\n<Val></Val>\r\n</String>\r\n<String>\r\n<Name> </Name>\r\n<Val></Val>\r\n</String>\r\n<String>\r\n<Name> </Name>\r\n<Val></Val>\r\n</String>\r\n<String>\r\n<Name> </Name>\r\n<Val></Val>\r\n</String>\r\n<String>\r\n<Name> </Name>\r\n<Val></Val>\r\n</String>\r\n<String>\r\n<Name> </Name>\r\n<Val></Val>\r\n</String>\r\n<String>\r\n<Name> </Name>\r\n<Val></Val>\r\n</String>\r\n<String>\r\n<Name> </Name>\r\n<Val></Val>\r\n</String>\r\n<String>\r\n<Name> </Name>\r\n<Val></Val>\r\n</String>\r\n<String>\r\n<Name> </Name>\r\n<Val></Val>\r\n</String>\r\n<String>\r\n<Name> </Name>\r\n<Val></Val>\r\n</String>\r\n<String>\r\n<Name> </Name>\r\n<Val></Val>\r\n</String>\r\n<String>\r\n<Name> </Name>\r\n<Val></Val>\r\n</String>\r\n<String>\r\n<Name> </Name>\r\n<Val></Val>\r\n</String>\r\n<String>\r\n<Name> </Name>\r\n<Val></Val>\r\n</String>\r\n<String>\r\n<Name> </Name>\r\n<Val></Val>\r\n</String>\r\n<String>\r\n<Name> </Name>\r\n<Val></Val>\r\n</String>\r\n<String>\r\n<Name> </Name>\r\n<Val></Val>\r\n</String>\r\n<String>\r\n<Name> </Name>\r\n<Val></Val>\r\n</String>\r\n<String>\r\n<Name> </Name>\r\n<Val></Val>\r\n</String>\r\n<String>\r\n<Name> </Name>\r\n<Val></Val>\r\n</String>\r\n<String>\r\n<Name> </Name>\r\n<Val></Val>\r\n</String>\r\n<String>\r\n<Name> </Name>\r\n<Val></Val>\r\n</String>\r\n<String>\r\n<Name> </Name>\r\n<Val></Val>\r\n</String>\r\n<String>\r\n<Name> </Name>\r\n<Val></Val>\r\n</String>\r\n<String>\r\n<Name> </Name>\r\n<Val></Val>\r\n</String>\r\n<String>\r\n<Name> </Name>\r\n<Val></Val>\r\n</String>\r\n<String>\r\n<Name> </Name>\r\n<Val></Val>\r\n</String>\r\n<String>\r\n<Name> </Name>\r\n<Val></Val>\r\n</String>\r\n<String>\r\n<Name> </Name>\r\n<Val></Val>\r\n</String>\r\n<String>\r\n<Name> </Name>\r\n<Val></Val>\r\n</String>\r\n<String>\r\n<Name> </Name>\r\n<Val></Val>\r\n</String>\r\n<String>\r\n<Name> </Name>\r\n<Val></Val>\r\n</String>\r\n<String>\r\n<Name> </Name>\r\n<Val></Val>\r\n</String>\r\n<String>\r\n<Name> </Name>\r\n<Val></Val>\r\n</String>\r\n<String>\r\n<Name> </Name>\r\n<Val></Val>\r\n</String>\r\n<String>\r\n<Name> </Name>\r\n<Val></Val>\r\n</String>\r\n<String>\r\n<Name> </Name>\r\n<Val></Val>\r\n</String>\r\n<String>\r\n<Name> </Name>\r\n<Val></Val>\r\n</String>\r\n<String>\r\n<Name> </Name>\r\n<Val></Val>\r\n</String>\r\n<String>\r\n<Name> </Name>\r\n<Val></Val>\r\n</String>\r\n<String>\r\n<Name> </Name>\r\n<Val></Val>\r\n</String>\r\n<String>\r\n<Name> </Name>\r\n<Val></Val>\r\n</String>\r\n<String>\r\n<Name> </Name>\r\n<Val></Val>\r\n</String>\r\n<String>\r\n<Name> </Name>\r\n<Val></Val>\r\n</String>\r\n<String>\r\n<Name> </Name>\r\n<Val></Val>\r\n</String>\r\n<String>\r\n<Name> </Name>\r\n<Val></Val>\r\n</String>\r\n<String>\r\n<Name> </Name>\r\n<Val></Val>\r\n</String>\r\n<String>\r\n<Name> </Name>\r\n<Val></Val>\r\n</String>\r\n<String>\r\n<Name> </Name>\r\n<Val></Val>\r\n</String>\r\n<String>\r\n<Name> </Name>\r\n<Val></Val>\r\n</String>\r\n<String>\r\n<Name> </Name>\r\n<Val></Val>\r\n</String>\r\n<String>\r\n<Name> </Name>\r\n<Val></Val>\r\n</String>\r\n<String>\r\n<Name> </Name>\r\n<Val></Val>\r\n</String>\r\n<String>\r\n<Name> </Name>\r\n<Val></Val>\r\n</String>\r\n<String>\r\n<Name> </Name>\r\n<Val></Val>\r\n</String>\r\n<String>\r\n<Name> </Name>\r\n<Val></Val>\r\n</String>\r\n<String>\r\n<Name> </Name>\r\n<Val></Val>\r\n</String>\r\n<String>\r\n<Name> </Name>\r\n<Val></Val>\r\n</String>\r\n<String>\r\n<Name> </Name>\r\n<Val></Val>\r\n</String>\r\n<String>\r\n<Name> </Name>\r\n<Val></Val>\r\n</String>\r\n<String>\r\n<Name> </Name>\r\n<Val></Val>\r\n</String>\r\n<String>\r\n<Name> </Name>\r\n<Val></Val>\r\n</String>\r\n<String>\r\n<Name> </Name>\r\n<Val></Val>\r\n</String>\r\n<String>\r\n<Name> </Name>\r\n<Val></Val>\r\n</String>\r\n<String>\r\n<Name> </Name>\r\n<Val></Val>\r\n</String>\r\n<String>\r\n<Name> </Name>\r\n<Val></Val>\r\n</String>\r\n<String>\r\n<Name> </Name>\r\n<Val></Val>\r\n</String>\r\n<String>\r\n<Name> </Name>\r\n<Val></Val>\r\n</String>\r\n<String>\r\n<Name> </Name>\r\n<Val></Val>\r\n</String>\r\n<String>\r\n<Name> </Name>\r\n<Val></Val>\r\n</String>\r\n<String>\r\n<Name> </Name>\r\n<Val></Val>\r\n</String>\r\n<String>\r\n<Name> </Name>\r\n<Val></Val>\r\n</String>\r\n<String>\r\n<Name> </Name>\r\n<Val></Val>\r\n</String>\r\n<String>\r\n<Name> </Name>\r\n<Val></Val>\r\n</String>\r\n<String>\r\n<Name> </Name>\r\n<Val></Val>\r\n</String>\r\n<String>\r\n<Name> </Name>\r\n<Val></Val>\r\n</String>\r\n<String>\r\n<Name> </Name>\r\n<Val></Val>\r\n</String>\r\n<String>\r\n<Name> </Name>\r\n<Val></Val>\r\n</String>\r\n<String>\r\n<Name> </Name>\r\n<Val></Val>\r\n</String>\r\n<String>\r\n<Name> </Name>\r\n<Val></Val>\r\n</String>\r\n<String>\r\n<Name> </Name>\r\n<Val></Val>\r\n</String>\r\n<String>\r\n<Name> </Name>\r\n<Val></Val>\r\n</String>\r\n<String>\r\n<Name> </Name>\r\n<Val></Val>\r\n</String>\r\n<String>\r\n<Name> </Name>\r\n<Val></Val>\r\n</String>\r\n<String>\r\n<Name> </Name>\r\n<Val></Val>\r\n</String>\r\n<String>\r\n<Name> </Name>\r\n<Val></Val>\r\n</String>\r\n<String>\r\n<Name> </Name>\r\n<Val></Val>\r\n</String>\r\n<String>\r\n<Name> </Name>\r\n<Val></Val>\r\n</String>\r\n<String>\r\n<Name> </Name>\r\n<Val></Val>\r\n</String>\r\n<String>\r\n<Name> </Name>\r\n<Val></Val>\r\n</String>\r\n<String>\r\n<Name> </Name>\r\n<Val></Val>\r\n</String>\r\n<String>\r\n<Name> </Name>\r\n<Val></Val>\r\n</String>\r\n<String>\r\n<Name> </Name>\r\n<Val></Val>\r\n</String>\r\n<String>\r\n<Name> </Name>\r\n<Val></Val>\r\n</String>\r\n<String>\r\n<Name> </Name>\r\n<Val></Val>\r\n</String>\r\n<String>\r\n<Name> </Name>\r\n<Val></Val>\r\n</String>\r\n<String>\r\n<Name> </Name>\r\n<Val></Val>\r\n</String>\r\n<String>\r\n<Name> </Name>\r\n<Val></Val>\r\n</String>\r\n<String>\r\n<Name> </Name>\r\n<Val></Val>\r\n</String>\r\n<String>\r\n<Name> </Name>\r\n<Val></Val>\r\n</String>\r\n<String>\r\n<Name> </Name>\r\n<Val></Val>\r\n</String>\r\n<String>\r\n<Name> </Name>\r\n<Val></Val>\r\n</String>\r\n<String>\r\n<Name> </Name>\r\n<Val></Val>\r\n</String>\r\n<String>\r\n<Name> </Name>\r\n<Val></Val>\r\n</String>\r\n<String>\r\n<Name> </Name>\r\n<Val></Val>\r\n</String>\r\n<String>\r\n<Name> </Name>\r\n<Val></Val>\r\n</String>\r\n<String>\r\n<Name> </Name>\r\n<Val></Val>\r\n</String>\r\n<String>\r\n<Name> </Name>\r\n<Val></Val>\r\n</String>\r\n<String>\r\n<Name> </Name>\r\n<Val></Val>\r\n</String>\r\n<String>\r\n<Name> </Name>\r\n<Val></Val>\r\n</String>\r\n<String>\r\n<Name> </Name>\r\n<Val></Val>\r\n</String>\r\n<String>\r\n<Name> </Name>\r\n<Val></Val>\r\n</String>\r\n<String>\r\n<Name> </Name>\r\n<Val></Val>\r\n</String>\r\n<String>\r\n<Name> </Name>\r\n<Val></Val>\r\n</String>\r\n<String>\r\n<Name> </Name>\r\n<Val></Val>\r\n</String>\r\n<String>\r\n<Name> </Name>\r\n<Val></Val>\r\n</String>\r\n<String>\r\n<Name> </Name>\r\n<Val></Val>\r\n</String>\r\n<String>\r\n<Name> </Name>\r\n<Val></Val>\r\n</String>\r\n<String>\r\n<Name> </Name>\r\n<Val></Val>\r\n</String>\r\n<String>\r\n<Name> </Name>\r\n<Val></Val>\r\n</String>\r\n<String>\r\n<Name> </Name>\r\n<Val></Val>\r\n</String>\r\n<String>\r\n<Name> </Name>\r\n<Val></Val>\r\n</String>\r\n<String>\r\n<Name> </Name>\r\n<Val></Val>\r\n</String>\r\n<String>\r\n<Name> </Name>\r\n<Val></Val>\r\n</String>\r\n<String>\r\n<Name> </Name>\r\n<Val></Val>\r\n</String>\r\n<String>\r\n<Name> </Name>\r\n<Val></Val>\r\n</String>\r\n<String>\r\n<Name> </Name>\r\n<Val></Val>\r\n</String>\r\n<String>\r\n<Name> </Name>\r\n<Val></Val>\r\n</String>\r\n<String>\r\n<Name> </Name>\r\n<Val></Val>\r\n</String>\r\n<String>\r\n<Name> </Name>\r\n<Val></Val>\r\n</String>\r\n<String>\r\n<Name> </Name>\r\n<Val></Val>\r\n</String>\r\n<String>\r\n<Name> </Name>\r\n<Val></Val>\r\n</String>\r\n<String>\r\n<Name> </Name>\r\n<Val></Val>\r\n</String>\r\n<String>\r\n<Name> </Name>\r\n<Val></Val>\r\n</String>\r\n<String>\r\n<Name> </Name>\r\n<Val></Val>\r\n</String>\r\n<String>\r\n<Name> </Name>\r\n<Val></Val>\r\n</String>\r\n<String>\r\n<Name> </Name>\r\n<Val></Val>\r\n</String>\r\n<String>\r\n<Name> </Name>\r\n<Val></Val>\r\n</String>\r\n<String>\r\n<Name> </Name>\r\n<Val></Val>\r\n</String>\r\n<String>\r\n<Name> </Name>\r\n<Val></Val>\r\n</String>\r\n<String>\r\n<Name> </Name>\r\n<Val></Val>\r\n</String>\r\n<String>\r\n<Name> </Name>\r\n<Val></Val>\r\n</String>\r\n<String>\r\n<Name> </Name>\r\n<Val></Val>\r\n</String>\r\n<String>\r\n<Name> </Name>\r\n<Val></Val>\r\n</String>\r\n<String>\r\n<Name> </Name>\r\n<Val></Val>\r\n</String>\r\n<String>\r\n<Name> </Name>\r\n<Val></Val>\r\n</String>\r\n</Array>\r\n</Cluster>\r\n") -> (0 "error out":errorcluster, 3 "GZIP compressed string":string, 5 "Compression Ratio":dbl)   [LabVIEW 2010]
doc: "Compresses the input string using the gzip standard. \n\nOutput is astring that can be written to a binary file, or converted to a string and transferred via a connection (e.g. TCP/IP, DataSocket or RS-232). \n\nUses: reduce load on transport of data between LabVIEW nodes, saved to save storage space on disk or in a database, obfuscate the contents of a message or file (cheesey encryption).\n\nThis VI makes use of the .NET 2.0 framework.\n\nREV 1.0.1 02/15/2012 P.Brooks\n Compression Ratio fixed to report Compressed Size / Uncompressed Size.\n\nREV 1.0.0 10/02/2009 P.Brooks\n Originated."
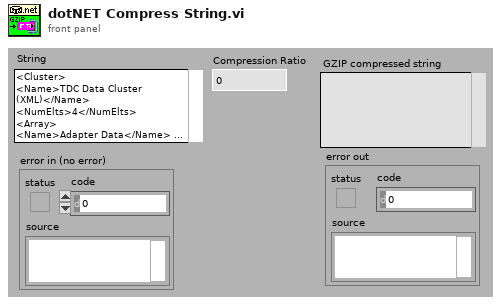
[diagram p1: front panel]
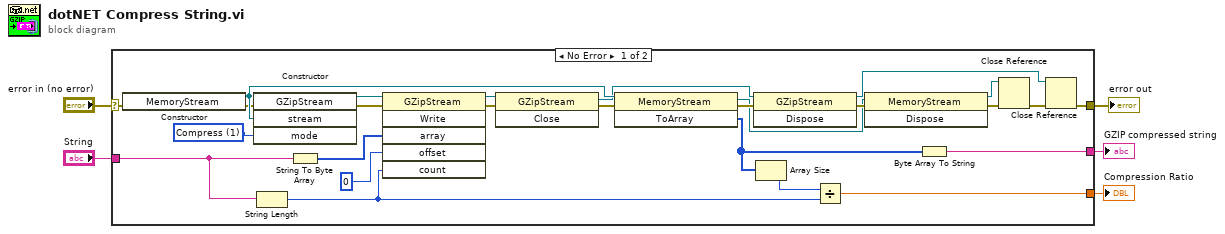
[diagram p0: block diagram]
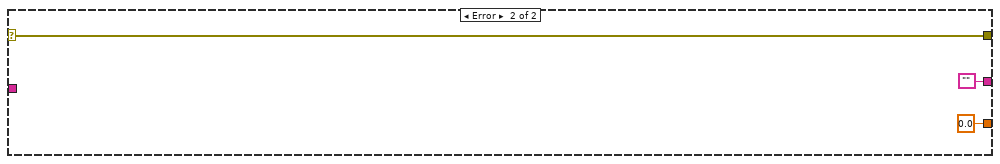
[diagram p2: hidden frame]
diagram:
  n1 = case shown="No Error" "error in (no error)" {
    selector: "error in (no error)" -> [w18 w34]
    tunnel: "String" -> [w28 _]
    tunnel: [w13 w34] -> w4
    tunnel: [w7 0.0] -> w2
    tunnel: [w6 "" ("string")] -> w1
    frame No Error {
      w21 = 1 items=["Decompress", "Compress"] ("mode")
      n2 = constructor class="MemoryStream"(error in=w18) -> (reference out=w24:refnum<k24>, error out=w20:errorcluster)  [unwired: 2 in, 1 out]
      n3 = constructor class="GZipStream"(error in=w20, "stream"=w24, "mode"=w21) -> (reference out=w22:refnum<k24>, error out=w23:errorcluster)  [unwired: 2 in, 3 out]
      n4 = String Length(string=w28) -> (length=w8:i32)
      n5 = String To Byte Array(string=w28) -> (unsigned byte array=w19:u8[])
      n6 = invoke class="GZipStream" method="Write"(reference=w22, error in=w23, "array"=w19, "offset"=0, "count"=w8) -> (reference out=w30:refnum<k24>, error out=w25:errorcluster)  [unwired: 1 in, 4 out]
      n7 = invoke class="GZipStream" method="Close"(reference=w30, error in=w25) -> (reference out=w12:refnum<k24>, error out=w26:errorcluster)  [unwired: 1 in, 1 out]
      n8 = invoke class="MemoryStream" method="ToArray"(reference=w24, error in=w26) -> (reference out=w11:refnum<k24>, error out=w31:errorcluster, "ToArray"=w10:u8[])  [unwired: 1 in]
      n9 = invoke class="GZipStream" method="Dispose"(reference=w12, error in=w31) -> (reference out=w14:refnum<k24>, error out=w29:errorcluster)  [unwired: 1 in, 1 out]
      n10 = Array Size(array=w10) -> (size(s)=w9:i32)
      n11 = Divide(x=w9, y=w8) -> (x/y=w7:dbl)
      n12 = invoke class="MemoryStream" method="Dispose"(reference=w11, error in=w29) -> (reference out=w16:refnum<k24>, error out=w17:errorcluster)  [unwired: 1 in, 1 out]
      n13 = Byte Array To String(unsigned byte array=w10) -> (string=w6:string)
      n14 = Close Reference(reference=w16, error in (no error)=w17) -> (error out=w15:errorcluster)
      n15 = Close Reference(reference=w14, error in (no error)=w15) -> (error out=w13:errorcluster)
    }
    frame Error {
    }
  }
  "error out" <- w4
  "Compression Ratio" <- w2
  "GZIP compressed string" <- w1
